vi "StreamEye_client_winX_v4.vi"() -> ()   [LabVIEW 2017]
uses:
  <vilib>/Analysis/NI_AALPro.lvlib
panel:
  in  "Start Scan":bool
  in  "Wavelength Step (nm)":dbl=100.0 min=0.0 max=100.0 step=0.01
  in  "Wavelength End (nm)":dbl=400.0 min=0.0 max=2000.0 step=0.01
  in  "Wavelength Start (nm)":dbl=400.0 min=0.0 max=2000.0 step=0.01
  in  "Fast continuous":bool caption="Focus mode"
  in  "standby stream":bool caption="Standby"
  out "time elapsed (s)":dbl caption="Time per scan (s)"
  out "Time Trace":dbl(graph)
  out "Intensity Sum":dbl
  in  "Stop measurement":bool
  out "XY Graph Spectrum":T1(graph)
  in  "Spectro Correct background":bool
  in  "Get Temp":bool
  in  "Misc Info/Variables":enum32{"Streaming", "OVA V"}(tab)
  out "reader endpoint":refnum<k21>
  out "error reader":errorcluster
  out "writer endpoint":refnum<k21>
  out "error writer":errorcluster
  out "MonoRef":refnum<k7>
  out "notifier out WinX Abort":refnum<notifier>
  out "notifier out WinX Start":refnum<notifier>
  in  "spectroObject reference":refnum<k7>
  in  "experiment reference_raw":refnum<k7>
  in  "file reference":refnum<k7>
  out "Wavelength Scale":dbl[](array[numeric])=[468.44882318557495, 468.4966768628263, 468.54452836446194, 468.59237769048184, 468.640224840886, 468.6880698156744, 468.73591261484705, 468.783753238404, 468.83159168634523, 468.8794279586707, 468.9272620553804, 468.9750939764744, 469.0229237219527, 469.07075129181516, 469.11857668606194, 469.16639990469304, 469.2142209477083, 469.2620398151079, 469.3098565068918, 469.3576710230599, 469.40548336361223, 469.45329352854884, 469.50110151786976, 469.5489073315749, 469.59671096966434, 469.644512432138, 469.69231171899594, 469.74010883023817, 469.78790376586466, 469.8356965258754, 469.8834871102704, 469.9312755190497, 469.97906175221317, 470.02684580976097, 470.074627691693, 470.12240739800933, 470.17018492870994, 470.2179602837948, 470.26573346326387, 470.31350446711724, 470.3612732953549, 470.4090399479768, 470.456804424983, 470.5045667263734, 470.5523268521481, 470.60008480230704, 470.6478405768503, 470.6955941757777, 470.7433455990895, 470.7910948467854, 470.83884191886574, 470.88658681533025, 470.93432953617906, 470.98207008141213, 471.02980845102945, 471.077544645031, 471.1252786634169, 471.17301050618704, 471.2207401733414, 471.26846766488006, 471.31619298080295, 471.36391612111015, 471.41163708580154, 471.45935587487725, 471.5070724883372, 471.55478692618146, 471.6024991884099, 471.6502092750227, 471.6979171860197, 471.745622921401, 471.79332648116656, 471.84102786531633, 471.8887270738504, 471.93642410676875, 471.98411896407134, 472.03181164575824, 472.07950215182933, 472.12719048228473, 472.1748766371244, 472.2225606163483, 472.27024241995645, 472.3179220479489, 472.36559950032563, 472.4132747770866, 472.4609478782318, 472.50861880376135, 472.5562875536751, 472.6039541279731, 472.6516185266554, 472.69928074972194, 472.7469407971728, 472.7945986690078, 472.8422543652272, 472.8899078858308, 472.93755923081864, 472.9852084001908, 473.0328553939472, 473.0805002120878, 473.1281428546128, 473.175783321522, 473.2234216128154, 473.27105772849313, 473.3186916685551, 473.36632343300136, 473.41395302183184, 473.46158043504664, 473.50920567264563, 473.55682873462894, 473.6044496209965, 473.65206833174835, 473.6996848668844, 473.7472992264048, 473.7949114103094, 473.84252141859827, 473.8901292512714, 473.9377349083288, 473.98533838977045, 474.0329396955964, 474.08053882580657, 474.12813578040107, 474.17573055937976, 474.22332316274276, 474.27091359049, 474.3185018426215, 474.36608791913727, 474.41367182003734, 474.46125354532165, 474.5088330949902, 474.55641046904304, 474.6039856674801, 474.6515586903015, 474.6991295375071, 474.74669820909696, 474.79426470507116, 474.84182902542955, 474.88939117017225, 474.93695113929914, 474.98450893281034, 475.0320645507058, 475.07961799298556, 475.1271692596495, 475.1747183506978, 475.2222652661303, 475.269810005947, 475.3173525701481, 475.3648929587334, 475.41243117170296, 475.4599672090568, 475.50750107079494, 475.5550327569173, 475.60256226742393, 475.6500896023148, 475.69761476158993, 475.7451377452494, 475.79265855329305, 475.840177185721, 475.88769364253324, 475.9352079237297, 475.9827200293104, 476.0302299592754, 476.0777377136247, 476.1252432923582, 476.172746695476, 476.22024792297805, 476.2677469748644, 476.31524385113494, 476.3627385517898, 476.4102310768289, 476.45772142625225, 476.5052096000599, 476.55269559825183, 476.600179420828, 476.6476610677884, 476.6951405391331, 476.742617834862, 476.79009295497525, 476.83756589947274, 476.8850366683545, 476.93250526162046, 476.97997167927076, 477.0274359213053, 477.0748979877241, 477.12235787852717, 477.1698155937145, 477.2172711332861, 477.2647244972419, 477.312175685582, 477.3596246983064, 477.40707153541507, 477.45451619690795, 477.50195868278513, 477.54939899304657, 477.59683712769225, 477.6442730867222, 477.69170687013644, 477.73913847793494, 477.7865679101177, 477.8339951666847, 477.88142024763596, 477.9288431529715, 477.97626388269134, 478.0236824367954, 478.07109881528373, 478.1185130181563, 478.1659250454132, 478.2133348970543, 478.2607425730797, 478.30814807348935, 478.35555139828324, 478.40295254746144, 478.4503515210239, 478.4977483189706, 478.54514294130155, 478.59253538801676, 478.6399256591163, 478.68731375460004, 478.73469967446806, 478.78208341872033, 478.82946498735686, 478.8768443803777, 478.9242215977828, 478.9715966395721, 479.0189695057457, 479.0663401963036, 479.1137087112457, 479.1610750505721, 479.20843921428275, 479.25580120237765, 479.30316101485687, 479.35051865172034, 479.397874112968, 479.4452273986, 479.49257850861625, 479.5399274430167, 479.5872742018015, 479.63461878497054, 479.68196119252383, 479.72930142446137, 479.7766394807832, 479.82397536148926, 479.8713090665796, 479.91864059605416, 479.9659699499131, 480.0132971281562, 480.0606221307836, 480.10794495779527, 480.1552656091912, 480.20258408497136, 480.24990038513585, 480.2972145096846, 480.34452645861757, 480.3918362319348, 480.4391438296363, 480.4864492517221, 480.5337524981921, 480.5810535690464, 480.62835246428494, 480.6756491839078, 480.72294372791487, 480.77023609630623, 480.81752628908185, 480.8648143062417, 480.9121001477859, 480.9593838137143, 481.00666530402697, 481.0539446187239, 481.1012217578051, 481.1484967212706, 481.1957695091203, 481.2430401213543, 481.29030855797254, 481.33757481897504, 481.3848389043618, 481.43210081413287, 481.4793605482882, 481.52661810682775, 481.5738734897516, 481.6211266970597, 481.66837772875203, 481.71562658482867, 481.76287326528956, 481.8101177701347, 481.85736009936414, 481.9046002529778, 481.95183823097574, 481.99907403335794, 482.0463076601244, 482.09353911127516, 482.1407683868102, 482.1879954867294, 482.2352204110329, 482.28244315972074, 482.32966373279277, 482.3768821302491, 482.4240983520897, 482.4713123983145, 482.5185242689236, 482.565733963917, 482.6129414832946, 482.6601468270565, 482.70734999520266, 482.7545509877331, 482.8017498046478, 482.84894644594675, 482.89614091162997, 482.94333320169744, 482.99052331614917, 483.0377112549852, 483.0848970182054, 483.13208060580996, 483.17926201779875, 483.22644125417185, 483.27361831492914, 483.32079320007074, 483.3679659095966, 483.4151364435067, 483.46230480180105, 483.5094709844797, 483.55663499154264, 483.6037968229898, 483.65095647882123, 483.6981139590369, 483.7452692636369, 483.79242239262106, 483.83957334598955, 483.8867221237423, 483.93386872587934, 483.9810131524006, 484.02815540330613, 484.07529547859593, 484.12243337827, 484.16956910232835, 484.2167026507709, 484.2638340235978, 484.31096322080884, 484.3580902424042, 484.4052150883839, 484.4523377587478, 484.49945825349596, 484.5465765726284, 484.5936927161451, 484.6408066840461, 484.6879184763313, 484.7350280930008, 484.78213553405453, 484.8292407994926, 484.87634388931485, 484.9234448035214, 484.9705435421122, 485.01764010508725, 485.06473449244663, 485.1118267041902, 485.1589167403181, 485.2060046008302, 485.2530902857266, 485.30017379500725, 485.34725512867215, 485.39433428672135, 485.4414112691548, 485.4884860759725, 485.53555870717446, 485.5826291627607, 485.62969744273124, 485.67676354708595, 485.723827475825, 485.7708892289483, 485.81794880645583, 485.86500620834767, 485.91206143462375, 485.9591144852841, 486.0061653603287, 486.0532140597576, 486.10026058357073, 486.1473049317681, 486.1943471043498, 486.2413871013157, 486.28842492266585, 486.3354605684003, 486.38249403851904, 486.429525333022, 486.4765544519093, 486.52358139518077, 486.57060616283655, 486.6176287548766, 486.6646491713009, 486.7116674121094, 486.75868347730227, 486.8056973668794, 486.8527090808407, 486.89971861918633, 486.9467259819162, 486.99373116903035, 487.0407341805287, 487.0877350164114, 487.13473367667837, 487.18173016132954, 487.228724470365, 487.2757166037847, 487.3227065615887, 487.369694343777, 487.4166799503495, 487.4636633813063, 487.51064463664727, 487.5576237163726, 487.6046006204822, 487.651575348976, 487.6985479018541, 487.7455182791164, 487.7924864807631, 487.839452506794, 487.8864163572091, 487.93337803200853, 487.9803375311922, 488.02729485476016, 488.07425000271235, 488.1212029750488, 488.16815377176954, 488.21510239287454, 488.2620488383638, 488.3089931082373, 488.3559352024951, 488.40287512113713, 488.44981286416345, 488.496748431574, 488.5436818233689, 488.590613039548, 488.63754208011136, 488.684468945059, 488.7313936343909, 488.778316148107, 488.8252364862074, 488.8721546486921, 488.919070635561, 488.9659844468142, 489.0128960824517, 489.05980554247344, 489.10671282687946, 489.15361793566973, 489.20052086884425, 489.247421626403, 489.2943202083461, 489.3412166146734, 489.388110845385, 489.4350029004808, 489.48189277996096, 489.5287804838253, 489.57566601207395, 489.62254936470686, 489.669430541724, 489.7163095431254, 489.76318636891114, 489.8100610190811, 489.8569334936353, 489.9038037925738, 489.9506719158965, 489.99753786360355, 490.04440163569484, 490.0912632321704, 490.13812265303017, 490.1849798982742, 490.23183496790256, 490.27868786191516, 490.325538580312, 490.3723871230931, 490.4192334902585, 490.46607768180814, 490.51291969774206, 490.55975953806023, 490.60659720276266, 490.65343269184933, 490.7002660053203, 490.74709714317555, 490.79392610541504, 490.8407528920388, 490.88757750304677, 490.93439993843907, 490.9812201982156, 491.02803828237643, 491.0748541909215, 491.12166792385085, 491.1684794811644, 491.2152888628623, 491.2620960689444, 491.3089010994108, 491.35570395426146, 491.4025046334964, 491.4493031371155, 491.49609946511896, 491.5428936175067, 491.58968559427865, 491.6364753954349, 491.6832630209754, 491.73004847090016, 491.77683174520917, 491.8236128439025, 491.87039176698, 491.9171685144418, 491.9639430862879, 492.01071548251826, 492.05748570313284, 492.1042537481317, 492.15101961751486, 492.19778331128225, 492.2445448294339, 492.29130417196984, 492.33806133889004, 492.38481633019444, 492.4315691458832, 492.47831978595616, 492.52506825041337, 492.5718145392549, 492.61855865248066, 492.6653005900907, 492.712040352085, 492.75877793846354, 492.8055133492264, 492.85224658437346, 492.8989776439048, 492.9457065278204, 492.9924332361203, 493.03915776880444, 493.08588012587285, 493.1326003073255, 493.1793183131624, 493.22603414338363, 493.2727477979891, 493.31945927697876, 493.36616858035273, 493.41287570811096, 493.4595806602535, 493.5062834367803, 493.5529840376913, 493.5996824629866, 493.64637871266615, 493.69307278673, 493.7397646851781, 493.78645440801046, 493.83314195522706, 493.879827326828, 493.9265105228131, 493.9731915431825, 494.0198703879362, 494.0665470570741, 494.11322155059634, 494.15989386850276, 494.2065640107935, 494.2532319774685, 494.2998977685278, 494.3465613839713, 494.3932228237991, 494.43988208801113, 494.48653917660744, 494.533194089588, 494.5798468269528, 494.6264973887019, 494.6731457748353, 494.7197919853529, 494.7664360202548, 494.81307787954097, 494.8597175632114, 494.90635507126603, 494.95299040370503, 494.9996235605282, 495.04625454173566, 495.0928833473274, 495.1395099773034, 495.1861344316637, 495.2327567104082, 495.279376813537, 495.32599474105007, 495.3726104929474, 495.41922406922896, 495.4658354698948, 495.5124446949449, 495.55905174437925, 495.6056566181979, 495.6522593164008, 495.69885983898797, 495.74545818595936, 495.79205435731507, 495.838648353055, 495.8852401731792, 495.93182981768774, 495.97841728658045, 496.02500257985747, 496.07158569751874, 496.11816663956427, 496.1647454059941, 496.2113219968081, 496.25789641200646, 496.30446865158905, 496.3510387155559, 496.397606603907, 496.4441723166424, 496.49073585376203, 496.53729721526594, 496.5838564011541, 496.63041341142656, 496.6769682460832, 496.7235209051242, 496.7700713885494, 496.8166196963589, 496.86316582855267, 496.90970978513064, 496.95625156609293, 497.00279117143947, 497.04932860117026, 497.09586385528536, 497.1423969337847, 497.18892783666826, 497.2354565639361, 497.2819831155883, 497.32850749162463, 497.3750296920453, 497.4215497168502, 497.4680675660394, 497.5145832396128, 497.56109673757055, 497.6076080599125, 497.6541172066387, 497.7006241777492, 497.74712897324395, 497.793631593123, 497.84013203738624, 497.8866303060338, 497.9331263990656, 497.97962031648166, 498.02611205828197, 498.0726016244666, 498.11908901503546, 498.1655742299886, 498.212057269326, 498.25853813304764, 498.3050168211536, 498.35149333364376, 498.3979676705182, 498.4444398317769, 498.4909098174199, 498.5373776274471, 498.5838432618586, 498.6303067206544, 498.6767680038344, 498.72322711139867, 498.76968404334724, 498.81613879968006, 498.86259138039713, 498.9090417854985, 498.9554900149841, 499.001936068854, 499.0483799471081, 499.0948216497465, 499.1412611767692, 499.1876985281761, 499.2341337039673, 499.28056670414276, 499.32699752870246, 499.3734261776465, 499.4198526509747, 499.4662769486872, 499.512699070784, 499.559119017265, 499.60553678813034, 499.65195238337986, 499.6983658030137, 499.7447770470318, 499.79118611543413, 499.8375930082208, 499.8839977253916, 499.9304002669468, 499.9768006328862, 500.0231988232099, 500.0695948379178, 500.11598867701, 500.16238034048644, 500.2087698283472, 500.2551571405922, 500.3015422772214, 500.34792523823495, 500.39430602363274, 500.4406846334148, 500.48706106758107, 500.53343532613167, 500.57980740906646, 500.62617731638557, 500.6725450480889, 500.7189106041766, 500.76527398464845, 500.8116351895046, 500.85799421874503, 500.9043510723697, 500.95070575037863, 500.99705825277186, 501.0434085795493, 501.08975673071103, 501.136102706257, 501.1824465061873, 501.2287881305018, 501.2751275792006, 501.32146485228367, 501.367799949751, 501.41413287160253, 501.4604636178384, 501.5067921884585, 501.5531185834629, 501.5994428028515, 501.6457648466244, 501.6920847147816, 501.73840240732295, 501.78471792424864, 501.8310312655586, 501.8773424312528, 501.9236514213313, 501.969958235794, 502.01626287464103, 502.0625653378723, 502.10886562548785, 502.1551637374876, 502.2014596738716, 502.24775343463995, 502.2940450197925, 502.3403344293294, 502.3866216632505, 502.43290672155587, 502.4791896042455, 502.5254703113194, 502.5717488427776, 502.61802519862, 502.6642993788467, 502.71057138345765, 502.75684121245285, 502.80310886583237, 502.8493743435961, 502.8956376457441, 502.9418987722764, 502.98815772319296, 503.03441449849373, 503.0806690981788, 503.12692152224815, 503.17317177070174, 503.2194198435396, 503.2656657407617, 503.3119094623681, 503.35815100835873, 503.40439037873364, 503.4506275734928, 503.49686259263626, 503.5430954361639, 503.5893261040759, 503.6355545963721, 503.68178091305265, 503.7280050541174, 503.7742270195664, 503.8204468093997, 503.86666442361724, 503.91287986221903, 503.95909312520513, 504.0053042125754, 504.05151312433003, 504.0977198604689, 504.14392442099205, 504.1901268058994, 504.2363270151911, 504.282525048867, 504.3287209069272, 504.3749145893716, 504.42110609620033, 504.4672954274133, 504.51348258301056, 504.55966756299205, 504.6058503673578, 504.65203099610784, 504.6982094492421, 504.74438572676064, 504.79055982866345, 504.83673175495056, 504.8829015056219, 504.9290690806775, 504.97523448011736, 505.0213977039415, 505.0675587521499, 505.11371762474255, 505.1598743217195, 505.2060288430807, 505.2521811888261, 505.29833135895586, 505.3444793534698, 505.39062517236806, 505.43676881565057, 505.4829102833173, 505.5290495753684, 505.57518669180365, 505.6213216326232, 505.66745439782704, 505.7135849874151, 505.7597134013875, 505.80583963974414, 505.85196370248497, 505.8980855896101, 505.94420530111955, 505.9903228370132, 506.03643819729115, 506.08255138195335, 506.1286623909998, 506.1747712244305, 506.2208778822455, 506.26698236444474, 506.31308467102826, 506.35918480199604, 506.40528275734806, 506.4513785370844, 506.4974721412049, 506.54356356970976, 506.58965282259885, 506.63573989987225, 506.6818248015298, 506.7279075275717, 506.77398807799784, 506.82006645280825, 506.8661426520029, 506.9122166755819, 506.95828852354504, 507.0043581958925, 507.05042569262423, 507.09649101374026, 507.1425541592405, 507.188615129125, 507.2346739233938, 507.28073054204685, 507.32678498508415, 507.37283725250575, 507.4188873443116, 507.4649352605017, 507.51098100107606, 507.55702456603467, 507.6030659553776, 507.6491051691047, 507.6951422072161, 507.74117706971185, 507.7872097565918, 507.83324026785596, 507.87926860350444, 507.9252947635372, 507.9713187479542, 508.01734055675547, 508.06336018994097, 508.10937764751077, 508.1553929294648, 508.20140603580313, 508.24741696652575, 508.29342572163256, 508.3394323011237, 508.38543670499905, 508.4314389332587, 508.4774389859026, 508.52343686293074, 508.5694325643432, 508.61542609013986, 508.6614174403208, 508.70740661488605, 508.7533936138355, 508.79937843716925, 508.84536108488726, 508.8913415569896, 508.9373198534761, 508.9832959743469, 509.029269919602, 509.0752416892413, 509.12121128326487, 509.1671787016727, 509.21314394446483, 509.2591070116412, 509.30506790320186, 509.35102661914675, 509.39698315947595, 509.44293752418935, 509.48888971328705, 509.534839726769, 509.5807875646353, 509.62673322688573, 509.6726767135205, 509.7186180245395, 509.7645571599428, 509.8104941197303, 509.85642890390216, 509.9023615124582, 509.9482919453985, 509.9942202027231, 510.040146284432, 510.0860701905251, 510.1319919210025, 510.17791147586416, 510.22382885511007, 510.26974405874023, 510.3156570867547, 510.3615679391534, 510.4074766159364, 510.4533831171036, 510.4992874426551, 510.5451895925909, 510.59108956691085, 510.63698736561514, 510.6828829887037, 510.72877643617653, 510.7746677080336, 510.82055680427493, 510.86644372490053, 510.9123284699104, 510.95821103930456, 511.00409143308286, 511.04996965124553, 511.09584569379246, 511.14171956072363, 511.1875912520391, 511.2334607677388, 511.2793281078228, 511.325193272291, 511.3710562611435, 511.4169170743803, 511.4627757120013, 511.5086321740066, 511.55448646039616, 511.60033857116997, 511.6461885063281, 511.6920362658704, 511.737881849797, 511.7837252581079, 511.8295664908031, 511.87540554788245, 511.92124242934614, 511.9670771351941, 512.0129096654263, 512.0587400200427, 512.1045681990435, 512.1503942024284, 512.1962180301977, 512.2420396823511, 512.287859158889, 512.3336764598109, 512.3794915851173, 512.4253045348079, 512.4711153088826, 512.5169239073417, 512.5627303301851, 512.6085345774127, 512.6543366490246, 512.7001365450208, 512.7459342654012, 512.7917298101659, 512.8375231793148, 512.883314372848, 512.9291033907655, 512.9748902330672, 513.0206748997532, 513.0664573908234, 513.1122377062779, 513.1580158461167, 513.2037918103398, 513.249565598947, 513.2953372119387, 513.3411066493145, 513.3868739110745, 513.432638997219, 513.4784019077475, 513.5241626426605, 513.5699212019576, 513.615677585639, 513.6614317937047, 513.7071838261546, 513.7529336829889, 513.7986813642074, 513.84442686981, 513.890170199797, 513.9359113541683, 513.9816503329239, 514.0273871360637, 514.0731217635877, 514.118854215496, 514.1645844917886, 514.2103125924655, 514.2560385175266, 514.3017622669719, 514.3474838408015, 514.3932032390154, 514.4389204616136, 514.484635508596, 514.5303483799627, 514.5760590757136, 514.6217675958488, 514.6674739403684, 514.7131781092721, 514.75888010256, 514.8045799202323, 514.8502775622889, 514.8959730287297, 514.9416663195548, 514.987357434764, 515.0330463743577, 515.0787331383355, 515.1244177266976, 515.170100139444, 515.2157803765747, 515.2614584380896, 515.3071343239887, 515.3528080342721, 515.3984795689398, 515.4441489279917, 515.489816111428, 515.5354811192485, 515.5811439514532, 515.6268046080422, 515.6724630890155, 515.718119394373, 515.7637735241149, 515.8094254782409, 515.8550752567513, 515.9007228596458, 515.9463682869247, 515.9920115385878, 516.0376526146352, 516.0832915150669, 516.1289282398827, 516.1745627890829, 516.2201951626673, 516.2658253606361, 516.311453382989, 516.3570792297262, 516.4027029008477, 516.4483243963535, 516.4939437162435, 516.5395608605178, 516.5851758291764, 516.6307886222193, 516.6763992396462, 516.7220076814576, 516.7676139476531, 516.8132180382331, 516.8588199531972, 516.9044196925456, 516.9500172562782, 516.9956126443952, 517.0412058568963, 517.0867968937818, 517.1323857550515, 517.1779724407054, 517.2235569507437, 517.2691392851661, 517.3147194439729, 517.3602974271639, 517.4058732347393, 517.4514468666988, 517.4970183230427, 517.5425876037707, 517.588154708883, 517.6337196383797, 517.6792823922606, 517.7248429705256, 517.7704013731751, 517.8159576002088, 517.8615116516266, 517.9070635274288, 517.9526132276153, 517.9981607521861, 518.043706101141, 518.0892492744803, 518.1347902722036, 518.1803290943116, 518.2258657408036, 518.2714002116799, 518.3169325069404, 518.3624626265853, 518.4079905706143, 518.4535163390277, 518.4990399318252, 518.5445613490073, 518.5900805905733, 518.6355976565237, 518.6811125468583, 518.7266252615774, 518.7721358006805, 518.817644164168, 518.8631503520397, 518.9086543642958, 518.9541562009359, 518.9996558619605, 519.0451533473693, 519.0906486571622, 519.1361417913396, 519.1816327499012, 519.2271215328469, 519.272608140177, 519.3180925718915, 519.3635748279901, 519.409054908473, 519.45453281334, 519.5000085425916, 519.5454820962271, 519.5909534742472, 519.6364226766513, 519.6818897034399, 519.7273545546126, 519.7728172301695, 519.8182777301107, 519.8637360544363, 519.9091922031461, 519.9546461762401, 520.0000979737184, 520.045547595581, 520.0909950418279, 520.136440312459, 520.1818834074743, 520.2273243268739, 520.2727630706579, 520.3181996388261, 520.3636340313784, 520.4090662483151, 520.4544962896362, 520.4999241553413, 520.5453498454308, 520.5907733599045, 520.6361946987626, 520.6816138620048, 520.7270308496313, 520.772445661642, 520.8178582980372, 520.8632687588165, 520.90867704398, 520.9540831535279, 520.99948708746, 521.0448888457764, 521.090288428477, 521.1356858355618, 521.1810810670311, 521.2264741228845, 521.2718650031222, 521.3172537077442, 521.3626402367503, 521.4080245901409, 521.4534067679156, 521.4987867700746, 521.5441645966179, 521.5895402475454, 521.6349137228573, 521.6802850225532, 521.7256541466336, 521.7710210950983, 521.8163858679471, 521.8617484651802, 521.9071088867976, 521.9524671327993, 521.9978232031851, 522.0431770979553, 522.0885288171097, 522.1338783606484, 522.1792257285714, 522.2245709208786, 522.2699139375701, 522.3152547786458, 522.3605934441059, 522.4059299339501, 522.4512642481786, 522.4965963867915, 522.5419263497886, 522.5872541371699, 522.6325797489355, 522.6779031850854, 522.7232244456195, 522.7685435305378, 522.8138604398405, 522.8591751735274, 522.9044877315987, 522.949798114054, 522.9951063208938, 523.0404123521178, 523.0857162077259, 523.1310178877185, 523.1763173920953, 523.2216147208562, 523.2669098740015, 523.3122028515311, 523.3574936534449, 523.402782279743, 523.4480687304252, 523.4933530054919, 523.5386351049428, 523.5839150287779, 523.6291927769973, 523.674468349601, 523.719741746589, 523.7650129679611, 523.8102820137175, 523.8555488838583, 523.9008135783832, 523.9460760972925, 523.991336440586, 524.0365946082637, 524.0818506003258, 524.1271044167721, 524.1723560576027, 524.2176055228174, 524.2628528124166, 524.3080979263999, 524.3533408647675, 524.3985816275193, 524.4438202146556, 524.489056626176, 524.5342908620805, 524.5795229223695, 524.6247528070428, 524.6699805161002, 524.7152060495418, 524.7604294073678, 524.8056505895781, 524.8508695961726, 524.8960864271514, 524.9413010825144, 524.9865135622617, 525.0317238663933, 525.0769319949092, 525.1221379478092, 525.1673417250936, 525.2125433267622, 525.2577427528151, 525.3029400032523, 525.3481350780736, 525.3933279772793, 525.4385187008693, 525.4837072488434, 525.5288936212019, 525.5740778179447, 525.6192598390717, 525.6644396845829, 525.7096173544784, 525.7547928487583, 525.7999661674223, 525.8451373104706, 525.8903062779032, 525.9354730697199, 525.9806376859211, 526.0258001265064, 526.0709603914761, 526.1161184808299, 526.1612743945682, 526.2064281326906, 526.2515796951972, 526.2967290820881, 526.3418762933634, 526.3870213290229, 526.4321641890666, 526.4773048734945, 526.5224433823068, 526.5675797155034, 526.6127138730842, 526.6578458550492, 526.7029756613986, 526.7481032921321, 526.7932287472499, 526.838352026752, 526.8834731306383, 526.9285920589091, 526.9737088115639, 527.0188233886031, 527.0639357900264, 527.1090460158342, 527.1541540660262, 527.1992599406024, 527.2443636395628, 527.2894651629076, 527.3345645106366, 527.3796616827499, 527.4247566792474, 527.4698495001293, 527.5149401453954, 527.5600286150457, 527.6051149090802, 527.6501990274991, 527.6952809703022, 527.7403607374896, 527.7854383290612, 527.830513745017, 527.8755869853574, 527.9206580500817, 527.9657269391904, 528.0107936526833, 528.0558581905606, 528.1009205528221, 528.1459807394677, 528.1910387504978, 528.2360945859122, 528.2811482457107, 528.3261997298935, 528.3712490384605, 528.4162961714119, 528.4613411287474, 528.5063839104673, 528.5514245165714, 528.5964629470599, 528.6414992019324, 528.6865332811893, 528.7315651848305, 528.7765949128559, 528.8216224652657, 528.8666478420597, 528.9116710432379, 528.9566920688003, 529.0017109187472, 529.0467275930782, 529.0917420917934, 529.136754414893, 529.1817645623769, 529.2267725342449, 529.2717783304972, 529.3167819511337, 529.3617833961547, 529.4067826655598, 529.4517797593492, 529.4967746775228, 529.5417674200809, 529.586757987023, 529.6317463783495, 529.6767325940601, 529.7217166341551, 529.7666984986344, 529.8116781874978, 529.8566557007456, 529.9016310383776, 529.946604200394, 529.9915751867945, 530.0365439975793, 530.0815106327484, 530.1264750923018, 530.1714373762394, 530.2163974845612, 530.2613554172673, 530.3063111743578, 530.3512647558324, 530.3962161616913, 530.4411653919345, 530.4861124465621, 530.5310573255738, 530.5760000289697]
  in  "FrameVariant":variant
  out "experiment reference":refnum<k7>
  out "frame array":i32[][](array[numeric])
  out "time start (ms)":i32
  in  "Set Temperature (°C)":i8 min=-125 max=25 step=1
  in  "Start Continuous":bool
  in  "Start Background":bool
  in  "Start Single Spectrum":bool
  in  "Start Stream":bool
  out "busy":bool
  out "Hosts Synchronized":bool
  in  "Synchronize Hosts":bool
  in  "Init Spectro":bool
  in  "Exit":bool
  out "OMA V temp":dbl(slide) caption="Sensor Temperature" scale=-125.0..25.0
  in  "OMA V exposure time":dbl=0.001 caption="Integration time (s)" min=0.001 max=3000.0 step=0.001
  in  "OMA V gain":u32(ring) caption="Gain" items=["low"=2, "high"=3]
  in  "Grating Number":i16(ring) items=["600g/mm, blz=1.6um"=1, "300g/mm, blz=1.0um"=2, "150g/mm, blz=3.0um"=3]
  in  "Output Port":bool
  in  "Wavelength (nm)":dbl=400.0 min=-100.0 max=2000.0 step=0.01
  out "Spectro ON":bool
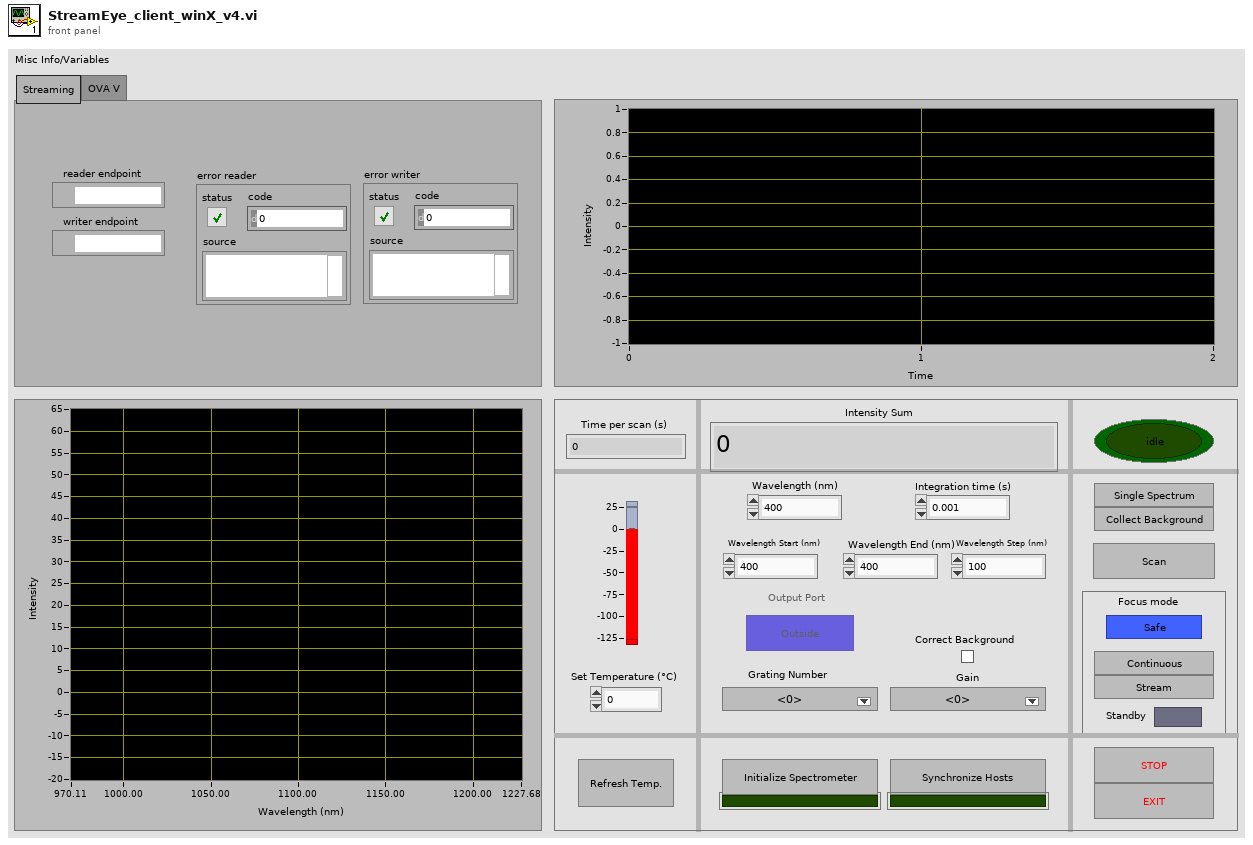
[diagram p1: front panel]
types:
  T1 = cluster{"Calibrated Array":dbl[], "Array F32":sgl[]}
  T2 = enum8{"Enabled", "Disabled", "Disabled and Grayed Out"}
  T3 = cluster{"Wavelength Scale":dbl[], "frame array":i32[]}
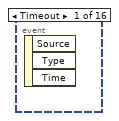
[diagram p2: hidden frame]
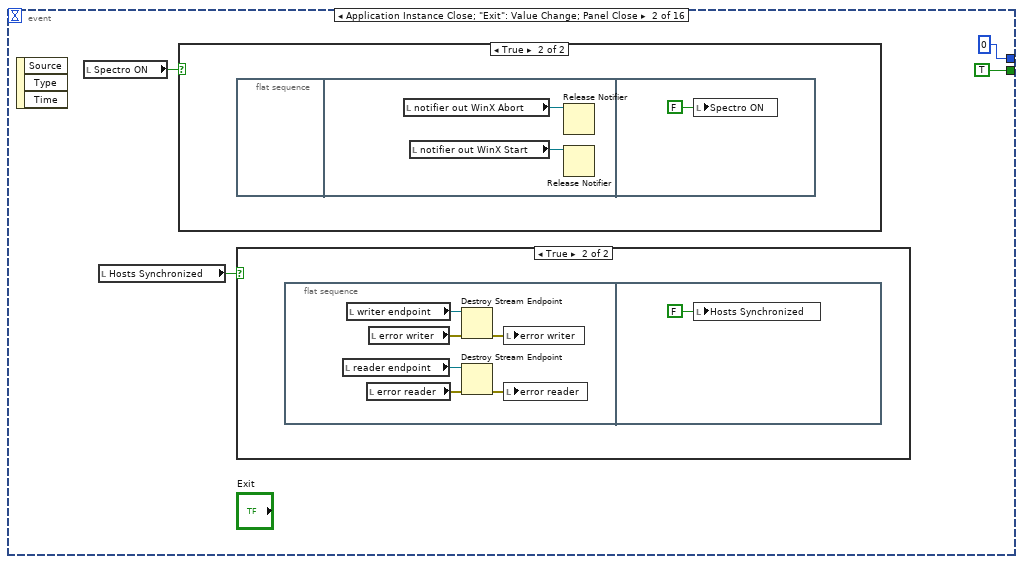
[diagram p3: hidden frame]
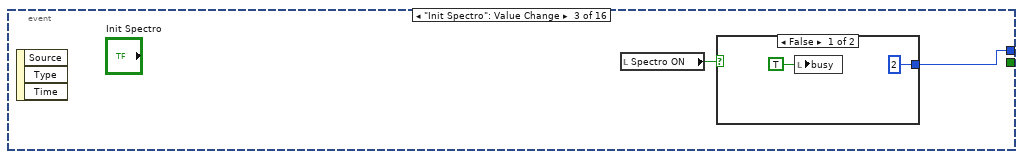
[diagram p6: hidden frame]
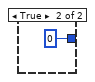
[diagram p7: hidden frame]
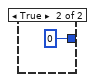
[diagram p8: hidden frame]
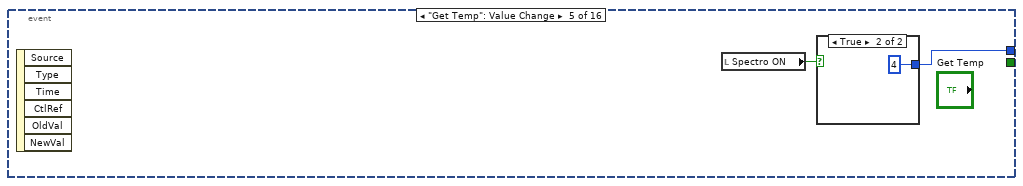
[diagram p9: hidden frame]
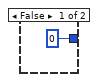
[diagram p10: hidden frame]
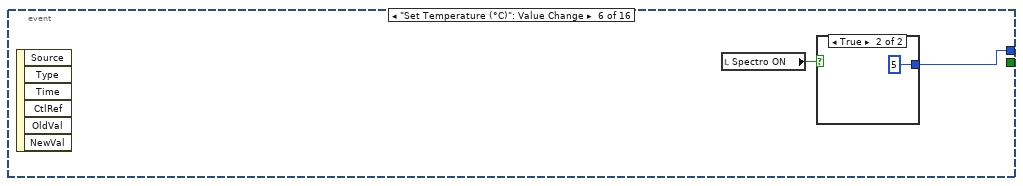
[diagram p11: hidden frame]
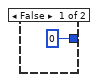
[diagram p12: hidden frame]
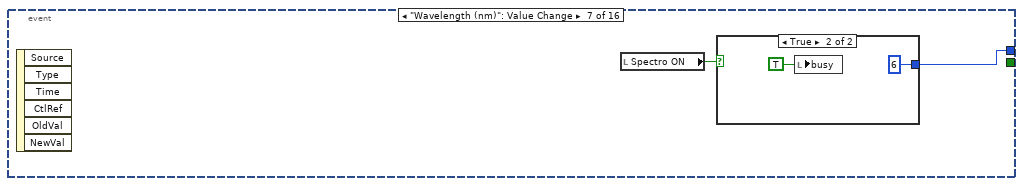
[diagram p13: hidden frame]
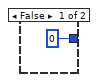
[diagram p14: hidden frame]
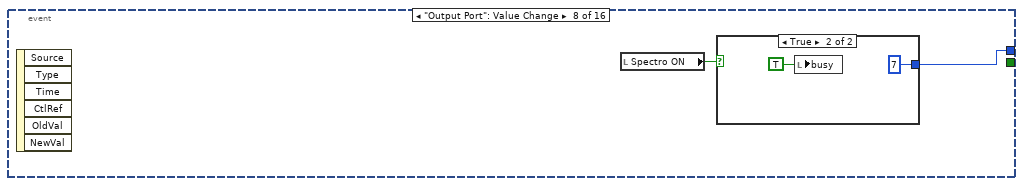
[diagram p15: hidden frame]
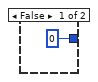
[diagram p16: hidden frame]
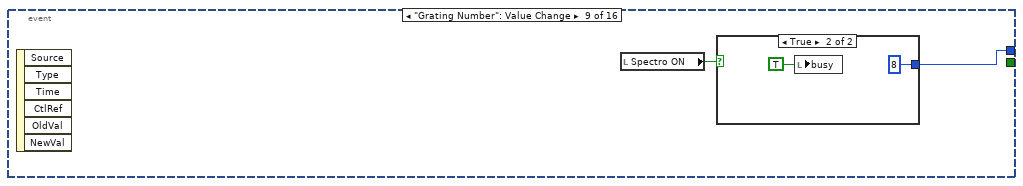
[diagram p17: hidden frame]
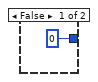
[diagram p18: hidden frame]
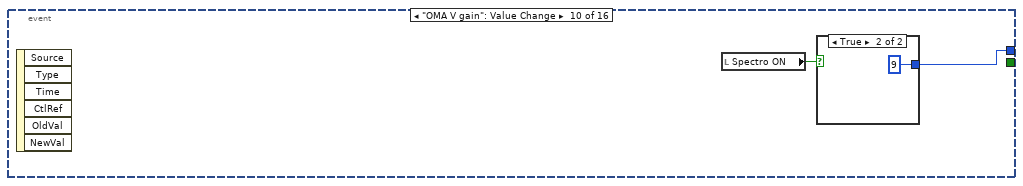
[diagram p19: hidden frame]
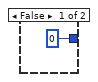
[diagram p20: hidden frame]
diagram:
  w8 = u32 2 items=["", "low", "high"] ("OMA V gain")
  w7 = FALSE ("Hosts Synchronized")
  n1 = while {
    stop <- w14 stop-if-true
    n2 = flat-sequence {
      tunnel: [w16] -> w14
      tunnel: [w15] -> w13
      tunnel: w13 -> [w108]
      frame #0 {
        # "Even catcher"
        n3 = event shown="[3] \"Synchronize Hosts\": Value Change" {
          selector: _ -> [_ _ _ _ _ _ _ _ _ _ _ _ _ _ _ _]
          dyn-events: _ -> [_ _ _ _ _ _ _ _ _ _ _ _ _ _ _ _]
          timeout: 1000 -> [_ _ _ _ _ _ _ _ _ _ _ _ _ _ _ _]
          tunnel: [_ TRUE _ _ _ _ _ _ _ _ _ _ _ _ _ _] -> w16
          tunnel: [_ 0 w33 w37 w42 w46 w50 w55 w61 w66 w69 w74 w79 w90 0 w103] -> w15
          event Timeout {
            n4 = event-data() -> ()  [unwired: 1 in, 3 out]
          }
          event Application Instance Close; "Exit": Value Change; Panel Close {
            n5 = event-data() -> ()  [unwired: 1 in, 3 out]
            n6 = local read "Spectro ON"() -> (w18:bool)
            n7 = local read "Hosts Synchronized"() -> (w19:bool)
            n8 = case shown="True" w18 {
              frame False {
              }
              frame True {
                n9 = flat-sequence {
                  frame #0 {
                  }
                  frame #1 {
                    n10 = local read "notifier out WinX Abort"() -> (w29:refnum<notifier>)
                    n11 = local read "notifier out WinX Start"() -> (w30:refnum<notifier>)
                    n12 = Release Notifier(notifier=w29) -> ()  [unwired: 2 in, 3 out]
                    n13 = Release Notifier(notifier=w30) -> ()  [unwired: 2 in, 3 out]
                  }
                  frame #2 {
                    n14 = local write "Spectro ON"(FALSE ("Spectro ON")) -> ()
                  }
                }
              }
            }
            n15 = case shown="True" w19 {
              frame False {
              }
              frame True {
                n16 = flat-sequence {
                  frame #0 {
                    n17 = local read "reader endpoint"() -> (w22:refnum<k21>)
                    n18 = local read "writer endpoint"() -> (w23:refnum<k21>)
                    n19 = local read "error reader"() -> (w27:errorcluster)
                    n20 = local read "error writer"() -> (w24:errorcluster)
                    n21 = Destroy Stream Endpoint(8:w24, 11:w23) -> (0:w25:errorcluster)
                    n22 = Destroy Stream Endpoint(8:w27, 11:w22) -> (0:w26:errorcluster)
                    n23 = local write "error writer"(w25) -> ()
                    n24 = local write "error reader"(w26) -> ()
                  }
                  frame #1 {
                    n25 = local write "Hosts Synchronized"(FALSE ("Hosts Synchronized")) -> ()
                  }
                }
              }
            }
          }
          event "Init Spectro": Value Change {
            n26 = event-data() -> ()  [unwired: 1 in, 3 out]
            n27 = local read "Spectro ON"() -> (w32:bool)
            n28 = case shown="False" w32 {
              tunnel: [2 0] -> w33
              frame False {
                n29 = local write "busy"(TRUE ("busy")) -> ()
              }
              frame True {
              }
            }
          }
          event "Synchronize Hosts": Value Change {
            n30 = event-data() -> ()  [unwired: 1 in, 3 out]
            n31 = local read "Hosts Synchronized"() -> (w38:bool)
            n32 = case shown="False" w38 {
              tunnel: [3 0] -> w37
              frame False {
                n33 = local write "busy"(TRUE ("busy")) -> ()
              }
              frame True {
              }
            }
          }
          event "Get Temp": Value Change {
            n34 = event-data() -> ()  [unwired: 1 in, 6 out]
            n35 = local read "Spectro ON"() -> (w43:bool)
            n36 = case shown="True" w43 {
              tunnel: [0 4] -> w42
              frame False {
              }
              frame True {
              }
            }
          }
          event "Set Temperature (°C)": Value Change {
            n37 = event-data() -> ()  [unwired: 1 in, 6 out]
            n38 = local read "Spectro ON"() -> (w47:bool)
            n39 = case shown="True" w47 {
              tunnel: [0 5] -> w46
              frame False {
              }
              frame True {
              }
            }
          }
          event "Wavelength (nm)": Value Change {
            n40 = event-data() -> ()  [unwired: 1 in, 6 out]
            n41 = local read "Spectro ON"() -> (w51:bool)
            n42 = case shown="True" w51 {
              tunnel: [0 6] -> w50
              frame False {
              }
              frame True {
                n43 = local write "busy"(TRUE ("busy")) -> ()
              }
            }
          }
          event "Output Port": Value Change {
            n44 = event-data() -> ()  [unwired: 1 in, 6 out]
            n45 = local read "Spectro ON"() -> (w56:bool)
            n46 = case shown="True" w56 {
              tunnel: [0 7] -> w55
              frame False {
              }
              frame True {
                n47 = local write "busy"(TRUE ("busy")) -> ()
              }
            }
          }
          event "Grating Number": Value Change {
            n48 = event-data() -> ()  [unwired: 1 in, 6 out]
            n49 = local read "Spectro ON"() -> (w60:bool)
            n50 = case shown="True" w60 {
              tunnel: [0 8] -> w61
              frame False {
              }
              frame True {
                n51 = local write "busy"(TRUE ("busy")) -> ()
              }
            }
          }
          event "OMA V gain": Value Change {
            n52 = event-data() -> ()  [unwired: 1 in, 6 out]
            n53 = local read "Spectro ON"() -> (w65:bool)
            n54 = case shown="True" w65 {
              tunnel: [0 9] -> w66
              frame False {
              }
              frame True {
              }
            }
          }
          event "Start Single Spectrum": Value Change {
            n55 = event-data() -> ()  [unwired: 1 in, 6 out]
            n56 = local read "Spectro ON"() -> (w70:bool)
            n57 = case shown="True" w70 {
              tunnel: [0 10] -> w69
              frame False {
              }
              frame True {
                n58 = local write "busy"(TRUE ("busy")) -> ()
              }
            }
          }
          event "Start Background": Value Change {
            n59 = event-data() -> ()  [unwired: 1 in, 6 out]
            n60 = local read "Spectro ON"() -> (w75:bool)
            n61 = case shown="True" w75 {
              tunnel: [0 11] -> w74
              frame False {
              }
              frame True {
                n62 = local write "busy"(TRUE) -> ()
              }
            }
          }
          event "Start Continuous": Value Change {
            n63 = event-data() -> ()  [unwired: 1 in, 6 out]
            n64 = local read "Spectro ON"() -> (w80:bool)
            n65 = case shown="True" w80 {
              tunnel: [0 w84] -> w79
              frame False {
              }
              frame True {
                n66 = local write "busy"(TRUE) -> ()
                n67 = local read "Fast continuous"() -> (w82:bool)
                n68 = Select(t=14, s=w82, f=12) -> (s? t:f=w84:i32)
              }
            }
          }
          event "Start Stream": Value Change {
            n69 = event-data() -> ()  [unwired: 1 in, 6 out]
            n70 = local read "Hosts Synchronized"() -> (w89:bool)
            n71 = local read "Spectro ON"() -> (w88:bool)
            n72 = And(x=w88, y=w89) -> (x .and. y?=w87:bool)
            n73 = case shown="True" w87 {
              tunnel: [0 w92] -> w90
              frame False {
              }
              frame True {
                n74 = local write "busy"(TRUE) -> ()
                n75 = local read "Fast continuous"() -> (w94:bool)
                n76 = Select(t=15, s=w94, f=13) -> (s? t:f=w92:i32)
              }
            }
          }
          event "Spectro Correct background": Value Change {
            n77 = event-data() -> ()  [unwired: 1 in, 6 out]
            n78 = local read "Spectro ON"() -> (w98:bool)
            n79 = case shown="True" w98 {
              frame False {
              }
              frame True {
                w102 = 828 items=["EXP_ETACTUAL"=1, "EXP_SEQUENTS"=2, "EXP_ERROR"=3, "EXP_GETCAPS"=4, "EXP_GETPLSR"=5, "EXP_DETECTOR_BIT"=16, "EXP_RUNNING_APP"=23, "EXP_VIDEO_TYPE"=24, "EXP_CUSTOM_VIDEO_X"=25, "EXP_CUSTOM_VIDEO_Y"=26, "EXP_CUSTOM_VIDEO_FSTWIDTH"=27, "EXP_CUSTOM_VIDEO_LSTWIDTH"=28, "EXP_VIDEO_XDIM"=29, "EXP_VIDEO_YDIM"=30, "EXP_VIDEO_MAX_ZOOM"=31, "EXP_VIDEO_HORZ_PAN"=32, "EXP_VIDEO_VERT_PAN"=33, "EXP_WORD_MULTIPLIER"=34, "EXP_TARGET_ID"=35, "EXP_ADAPTER_ID"=36, "EXP_NUMADAPTORS"=37, "EXP_FORCE_PP_INIT"=38, "EXP_NOP_ADC"=39, "EXP_ACTUAL_TEMP"=40, "EXP_FORCE_AUTOSTOP"=41, "EXP_DEFAULT_VTCLK"=42, "EXP_MIN_VTCLK"=43, "EXP_MAX_VTCLK"=44, "EXP_DEFAULT_HTCLK"=45, "EXP_MIN_HTCLK"=46, "EXP_MAX_HTCLK"=47, "EXP_TIMING_STYLE"=48, "EXP_HEADSELECT"=49, "EXP_HORZPHASE"=50, "EXP_VERTPHASE"=51, "EXP_SPECIAL_SPEED"=52, "EXP_PRE_STRIPS"=53, "EXP_POST_STRIPS"=54, "EXP_PRE_LINES"=55, "EXP_POST_LINES"=56, "EXP_ACTIVE_LINES"=57, "EXP_ACTIVE_STRIPS"=58, "EXP_XFER_EXTRA"=59, "EXP_MIN_BLOCK"=60, "EXP_NUM_MIN_BLOCK"=61, "EXP_LOGIC_OUTPUT"=66, "EXP_VIDEO_BLANK"=67, "EXP_ZOOM_MODE_VIDEO"=68, "EXP_LEVEL_SYNC"=69, "EXP_DISABLE_LASER"=70, "EXP_ACQBACK_SHUTTER"=71, "EXP_ACQFLAT_SHUTTER"=72, "EXP_SMALL_CCD_MINEXP"=73, "EXP_LARGE_CCD_MINEXP"=74, "EXP_GATING_MODE"=75, "EXP_ILME_B1X"=76, "EXP_ILME_B2X"=77, "EXP_ILME_D1X"=78, "EXP_ILME_D2X"=79, "EXP_ILME_D4X"=80, "EXP_INIT_HW_ACCUM"=81, "EXP_5X_GAIN_ENABLE"=82, "EXP_RET_SRCCMP"=83, "EXP_EVENT_HANDLE"=84, "EXP_READOUT_MODE"=85, "EXP_SHUTTER_TYPE"=86, "EXP_USER_DEFINED_CHIP"=87, "EXP_USER_DEFINED_TIMING"=88, "EXP_CONTROLLER_VERSION"=89, "EXP_GET_CONTROLLER_VER"=90, "EXP_TTL_LINES"=91, "EXP_BIT_ADJUST"=92, "EXP_RESOLUTION"=93, "EXP_GAIN"=94, "EXP_ADC_RATE"=95, "EXP_ADC_TYPE"=96, "EXP_NUMBER_OF_CLEANS"=97, "EXP_NUM_OF_STRIPS_PER_CLN"=98, "EXP_INTERFACE_CARD"=99, "EXP_INTERRUPT"=100, "EXP_IO_ADDRESS1"=101, "EXP_IO_ADDRESS2"=102, "EXP_IO_ADDRESS3"=103, "EXP_HW_ROI"=104, "EXP_HW_BINNING"=105, "EXP_EDGE_TRIGGER"=106, "EXP_SHUTTER_CONTROL"=107, "EXP_RS170"=108, "EXP_RS170_COMPLEX"=109, "EXP_HW_RS170_LUT"=110, "EXP_RS170_INTENSITY_SCALING"=111, "EXP_RS170_OFFSET"=112, "EXP_RS170_PAN"=113, "EXP_RS170_ZOOM2X"=114, "EXP_RS170_ZOOM4X"=115, "EXP_RS170_BINNING"=116, "EXP_RS170_DECIMATION"=117, "EXP_HW_ACCUM"=118, "EXP_SHT_PREOPEN"=119, "EXP_STORE_STROBE"=120, "EXP_CONT_CLNS"=121, "EXP_TIMING_MODE"=122, "EXP_EXT_TRIGGER"=123, "EXP_EVENT_COUNTER"=124, "EXP_SW_TRIGGER"=125, "EXP_KINETICS_WINDOWSIZE"=126, "EXP_EXPOSURE"=127, "EXP_CONTROLLER_NAME"=128, "EXP_CCD_CHIP_NAME"=129, "EXP_BSWBINNING"=297, "EXP_EDGEENHANCE"=130, "EXP_BOXVIDEOGAIN"=131, "EXP_HSHADING_VALUE"=132, "EXP_VSHADING_VALUE"=133, "EXP_EDGEENHANCE_FLAG"=134, "EXP_SHADING_FLAG"=135, "EXP_GRAYSCALE"=136, "EXP_OFFSET"=137, "EXP_CCDGAIN"=138, "EXP_TEMPERATURE"=139, "EXP_MCPVOLTAGE"=140, "EXP_BOXEXPOSURE"=141, "EXP_ABC_FLAG"=142, "EXP_GAMMA_FLAG"=143, "EXP_AUTOBLACK_FLAG"=144, "EXP_AGC_FLAG"=145, "EXP_ODD_FIELD"=146, "EXP_FIELD_SELECT"=147, "EXP_RESET"=148, "EXP_EXTERN_ENABLE"=149, "EXP_CONTROLLERS_SUPPORTED"=150, "EXP_VTCLK"=151, "EXP_HTCLK"=152, "EXP_GATE_VS_CW"=153, "EXP_COM_PORT"=154, "EXP_US_UNITS"=156, "EXP_MS_UNITS"=157, "EXP_SEC_UNITS"=158, "EXP_MIN_UNITS"=159, "EXP_HRS_UNITS"=160, "EXP_FRAME_UNITS"=161, "EXP_SYNC_ASYNC"=162, "EXP_FOCUS_NFRAME"=163, "EXP_TIMEOUT"=164, "EXP_TIMEOUT_DEFAULT"=165, "EXP_HW_AUTOSTOP"=166, "EXP_RS170_INTEN_OFFSET"=167, "EXP_CONTROLLER_ALIVE"=168, "EXP_FOCUS_TYPE"=169, "EXP_FOCUS_ZOOM"=170, "EXP_FOCUS_PAN"=171, "EXP_MULTI_TAP_ROI"=172, "EXP_USE_INTERUPTS"=173, "EXP_DATA_ACQ_STATE"=174, "EXP_VERIFY_GOOD_VALUES"=175, "EXP_WHITE_CLAMP"=176, "EXP_BLACK_CLAMP"=177, "EXP_DELAY_TIME"=178, "EXP_READOUT_TIME"=179, "EXP_SW_DIAG"=180, "EXP_DIAG1"=181, "EXP_DIAG2"=182, "EXP_DIAG3"=183, "EXP_DIAG4"=184, "EXP_DIAG5"=185, "EXP_AorB_GROUP"=186, "EXP_ABSORBANCE_FLAG"=187, "EXP_ABSORBANCE_METHOD"=188, "EXP_ABSORBANCE_STRIPNUM"=189, "EXP_DMASIZE_VIA_DRIVER"=190, "EXP_DRIVERVERSION"=191, "EXP_NUM_DEVICES"=192, "EXP_ECPDMA_CHANNEL"=193, "EXP_CUSTOM_SHUTTER"=194, "EXP_ADC_OFFSET"=195, "EXP_CURRENT_READOUT_MODE"=196, "EXP_BANK_ADD"=197, "EXP_LUT_BANK"=198, "EXP_SETUP_STATUS"=201, "EXP_XY_GROUPING"=239, "EXP_MESSAGES_FLAG"=240, "EXP_TTL_LINE_TO_WAIT"=253, "EXP_DATA_COLLECTION_MODE"=258, "EXP_DATA_COLLECTION_TYPE"=262, "EXP_SKIPFRAMES"=274, "EXP_CLR_INT_CNTR"=276, "EXP_ENABLE_INT_CNTR"=277, "EXP_INT_CNTR"=278, "EXP_INTERNAL_SYNC_SRC"=279, "EXP_SW_EXTSYNC"=280, "EXP_PTG_PRESENT"=281, "EXP_ELEC_SHT"=282, "EXP_BOARDS_WITH_NVRAM"=283, "EXP_ANLGMASTER_ST143"=284, "EXP_ANLGSLAVE_ST143"=285, "EXP_DISPLAY_ST143"=286, "EXP_INTRFACE_ST143"=287, "EXP_SCANCONTROL_ST143"=288, "EXP_NUMBERFRAMES_IRQ"=204, "EXP_COOL_TYPE"=214, "EXP_HD_TYPE"=215, "EXP_INTENSIFER_GAIN"=216, "EXP_SHT_GATE_MODE"=217, "EXP_HD_CHECK"=218, "EXP_AMP_MODE"=219, "EXP_AMP_DIALOG"=247, "EXP_ANALOG_GAIN"=220, "EXP_HW_FIXES"=221, "EXP_PCI_CARDS"=222, "EXP_NOT_REVERSE"=223, "EXP_LOAD_NVRAM_DEFAULTS"=234, "EXP_CNTR_BRD"=235, "EXP_XDIMHW"=237, "EXP_YDIMHW"=238, "EXP_SPECIAL_FAST_RDOUT"=254, "EXP_SPCL_FAST_Y_DIM"=255, "EXP_SPCL_FAST_X_DIM"=256, "EXP_SPCL_FAST_Y_INDEX"=257, "EXP_SHUTTER_COMP_TIME_MS"=266, "EXP_NVRAM_AVAIL"=267, "EXP_NUMBER_AGAIN_AVAIL"=269, "EXP_SENSOR_TYPE"=270, "EXP_EVENT_TYPE"=292, "EXP_ANTI_BLOOMING"=293, "EXP_FAST_PULSE_ENABLE"=233, "EXP_USE_HEADCALIB"=296, "EXP_TEMP_STATUS"=301, "EXP_MULTIPLE_READMODES_LIVE"=302, "EXP_FIRST_ACQUIRE_FLAG"=303, "EXP_ANTI_BLOOMING_CONTROL"=304, "EXP_PRE_HORZ_DELAY"=305, "EXP_NVRAM_TRIES"=306, "EXP_XASCEND"=307, "EXP_YASCEND"=308, "EXP_ALT_TIMING"=309, "EXP_SHUTTER_PRE_COMP"=310, "EXP_PVCAM_POSSIBLE"=311, "EXP_ADC_IN_NVRAM"=312, "EXP_PASSTHRU_MODE"=313, "EXP_FIRMWAREVERSION"=314, "EXP_IMMEDIATE_SHUTTER"=315, "EXP_STAGE2_TEMP"=316, "EXP_AVGAIN_ENABLED"=317, "EXP_AVGAIN_SETPOINT"=318, "EXP_AVGAIN"=319, "EXP_AVGAIN_CALIB_TEMP"=320, "EXP_AVGAIN_CALIB_COEFF1"=321, "EXP_AVGAIN_CALIB_COEFF2"=322, "EXP_AVGAIN_CALIB_COEFF3"=323, "EXP_AVGAIN_CALIB_COEFF4"=324, "EXP_AVGAIN_CALIB_COEFF5"=325, "EXP_FORCE_READOUT_MODE"=326, "EXP_RESET_DATACOLLECTION"=327, "EXP_ACTIVE_SUBFRAME"=328, "EXP_PV_READOUT_PORT"=514, "EXP_CLASSNAME"=775, "EXP_FLATFLDNAME"=776, "EXP_DARKNAME"=777, "EXP_SETUPNAME"=778, "EXP_ACCESSNAME"=779, "EXP_DATFILENAME"=780, "EXP_ABSORBFILENAME"=781, "EXP_BLEMISHFILENAME"=782, "EXP_COSMICFILENAME"=783, "EXP_FILEINCBASENAME"=784, "EXP_YTNAME"=785, "EXP_DEVNAME"=786, "EXP_USEROI"=787, "EXP_DOBLEMISH"=788, "EXP_DOABSORB"=789, "EXP_DOCOSMIC"=790, "EXP_COSMICSENS"=791, "EXP_ABSORBSTRIP"=792, "EXP_DATATYPE"=793, "EXP_OVERWRITECONFIRM"=794, "EXP_FILEINCENABLE"=795, "EXP_FILEINCCOUNT"=796, "EXP_RUNNING"=797, "EXP_SAVEROPT"=798, "EXP_TIME_UNITS"=799, "EXP_FILEACCESS"=800, "EXP_AUTOSAVE"=801, "EXP_NEWWINDOW"=802, "EXP_XDIM"=803, "EXP_YDIM"=804, "EXP_XDIMDET"=805, "EXP_YDIMDET"=806, "EXP_ROIMODE"=807, "EXP_NUMREPEATSEXP"=808, "EXP_NUMACCUMSEXP"=809, "EXP_THREADSTATE"=810, "EXP_USEMINTHRESHOLDING"=811, "EXP_MINTHRESHOLDVALUE"=812, "EXP_USEMAXTHRESHOLDING"=813, "EXP_MAXTHRESHOLDVALUE"=814, "EXP_RUNNING_EXPERIMENT"=815, "EXP_THRESHOLD_DEMAND_UPDATE"=816, "EXP_ROICOUNT"=817, "EXP_ACCUMS"=818, "EXP_CACCUMS"=819, "EXP_CSEQUENTS"=820, "EXP_PHOTON_ESTIMATION_ENABLE"=821, "EXP_PHOTON_MAXTIME"=822, "EXP_PHOTON_MAXTIMEUNIT"=823, "EXP_CUSTOMFILTER_ENABLE"=824, "EXP_CUSTOMFILTER_SIZE"=825, "EXP_LOOKUPTABLE_ENABLE"=826, "EXP_BSHOWWINDOW"=827, "EXP_BBACKSUBTRACT"=828, "EXP_BDOFLATFIELD"=829, "EXP_ASCIIOUTPUTFILE"=830, "EXP_ASCIIOUTPUT_DELIMITER"=831, "EXP_ASCIIOUTPUT_TERMINATOR"=832, "EXP_FFTYPE"=833, "EXP_BGTYPE"=834, "EXP_COSGRASS"=835, "EXP_RUNASCONFIRM"=836, "EXP_RUNASRUNACCESS"=837, "EXP_DATAFILETYPE"=838, "EXP_ROTATE"=839, "EXP_FLIP"=840, "EXP_REVERSE"=841, "EXP_SWBINNING"=842, "EXP_AUTOSTORE"=843, "EXP_XBINNED"=844, "EXP_YBINNED"=845, "EXP_NUMPATTERNS"=846, "EXP_EXPERIMENTTIME"=847, "EXP_ASYNCSEQUENTIALS"=848, "EXP_SEQUENTIALS"=849, "EXP_CSEQUENTIALS"=850, "EXP_AUTOD"=851, "EXP_EXPOSURETIME"=852, "EXP_EXPOSURETIME_UNITS"=853, "EXP_ACQMODE"=854, "EXP_DMASIZE_PVCAM"=855, "EXP_INITIALIZE"=856, "EXP_CELL_X_SIZE"=857, "EXP_CELL_Y_SIZE"=858, "EXP_X_GAP_SIZE"=859, "EXP_Y_GAP_SIZE"=860] ("Param")
                n80 = local read "experiment reference"() -> (w100:refnum<k7>)
                n81 = property on="Spectro Correct background" class="Bool (strict)"("DisabledEnum"=T2."Disabled" ("Disabled")) -> ()  [unwired: 2 in, 2 out]
                n82 = invoke class="IExpSetup2" method="SetParam"(reference=w100, "Param"=w102, "pSetVal"=0) -> ()  [unwired: 2 in, 5 out]
              }
            }
          }
          event "Start Scan": Value Change {
            n83 = event-data() -> ()  [unwired: 1 in, 6 out]
            n84 = local read "Spectro ON"() -> (w104:bool)
            n85 = case shown="True" w104 {
              tunnel: [0 16] -> w103
              frame False {
              }
              frame True {
                n86 = local write "busy"(TRUE ("busy")) -> ()
              }
            }
          }
        }
      }
      frame #1 {
        # "Event handler"
        n87 = case shown="16" w108 {
          frame 0, Default {
            # "idle"
          }
          frame 2 {
            # "InitSpectro"
            n88 = Obtain Notifier(name (unnamed)="Winx_Abort", notification data type=FALSE) -> (notifier out=→"notifier out WinX Abort":refnum<notifier>)  [unwired: 2 in, 2 out]
            n89 = Obtain Notifier(name (unnamed)="Winx_Start", notification data type=TRUE) -> (notifier out=→"notifier out WinX Start":refnum<notifier>)  [unwired: 2 in, 2 out]
            n90 = flat-sequence {
              tunnel: w111 -> [w156]
              frame #0 {
                # "monochromator"
                n91 = Automation Open(Automation Refnum="spectroObject reference") -> (Automation Refnum=w120:refnum<k7>)  [unwired: 3 in, 1 out]
                n92 = property class="ISpectroObjMgr"(reference=w120) -> ("Count"=w122:i16)  [unwired: 1 in, 2 out]
                n93 = property class="ISpectroObjMgr"(reference=w120) -> ("Current"=w118:refnum<k7>)  [unwired: 1 in, 2 out]
                "MonoRef" <- w118
                n94 = Greater Than 0?(x=w122) -> (x > 0?=w119:bool)
                n95 = case shown="True" w119 {
                  tunnel: w118 -> [_ w123]
                  frame False {
                  }
                  frame True {
                    w127 = 88 items=["SPT_NOCMD", "SPT_SPECTS_SUPPORTED", "SPT_TYPE", "SPT_CALIBUPDATE", "SPT_GRATINGWARNING", "SPT_LASERWARNING", "SPT_FORCEMOVE", "SPT_INSTNAME", "SPT_USERNAME", "SPT_INSTUSERNAME", "SPT_INSTCOMMNAME", "SPT_WAVE_ORIENTED", "SPT_NUMSTAGES", "SPT_GRATINGSPERTURRET", "SPT_CURRGRATING", "SPT_GRAT_BACKLASH_REQ", "SPT_GRATINGBACKLASHSTEPS", "SPT_NEEDINIT", "SPT_NEED_HWINIT", "SPT_MOTOR", "SPT_ARRAYSIZE", "SPT_ROI_CENTER", "SPT_ORDER", "SPT_CUR_GRATING", "SPT_NEW_GRATING", "SPT_SEQUENCER_STATE", "SPT_NUMTURRETS", "SPT_CURRTURRET", "SPT_DO_RESET", "SPT_SLAVE_CNT", "SPT_NUM_STEPS", "SPT_PIXEL_WIDTH", "SPT_GRAT_USERNAME", "SPT_GRAT_GROOVES", "SPT_GRAT_CENTERADJ", "SPT_GRAT_LINEAR_ADJ", "SPT_GRAT_SLOPE_ADJ", "SPT_GRAT_FOCAL_LEN", "SPT_GRAT_INCL_ANGLE", "SPT_GRAT_DETECT_ANGLE", "SPT_GRAT_MAG", "SPT_ACCESS_ALL_GRAT_SPEEDS", "SPT_SPEED_FOR_EACH_GRATING", "SPT_NUM_SETABLE_GRAT_SPEEDS", "SPT_GRATING_SPEED", "SPT_GRATING_SPEED_MIN", "SPT_GRATING_SPEED_MAX", "SPT_GRAT_REF_GRATING", "SPT_GRAT_STEPSPUNIT", "SPT_GRAT_OFFSET", "SPT_GRAT_ADJUST", "SPT_GRAT_LO_CAL_WAVE", "SPT_GRAT_HI_CAL_WAVE", "SPT_GRAT_LO_POS_WAVE", "SPT_GRAT_HI_POS_WAVE", "SPT_GRAT_REF_WAVE", "SPT_NUM_SLITS", "SPT_SLIT_ENABLED", "SPT_SLIT_LOCATION", "SPT_SLIT_CURPOSITION", "SPT_SLIT_NEWPOSITION", "SPT_SPEED_FOR_EACH_SLIT", "SPT_NUM_SETABLE_SLIT_SPEEDS", "SPT_SLIT_SPEED", "SPT_SLIT_SPEED_MIN", "SPT_SLIT_SPEED_MAX", "SPT_SLIT_STEPSPUNIT", "SPT_SLIT_BACKLASH_REQ", "SPT_SLIT_BACKLASH", "SPT_NUMMIRRORS", "SPT_MIRROR_ENABLED", "SPT_MIRROR_LOCATION", "SPT_MIRROR_CURPOSITION", "SPT_MIRROR_NEWPOSITION", "SPT_OFFSET_AVAIL", "SPT_ADJUST_AVAIL", "SPT_COUNTERSUPPORTED", "SPT_POSITIONSUPPORTED", "SPT_AUTOCALIBSUPPORTED", "SPT_POSITIONMEMORY", "SPT_NUMCOEFFS", "SPT_COEFF", "SPT_SERIAL_IO_SUPPORTED", "SPT_GPIB_IO_SUPPORTED", "SPT_OFFSETADJUSTSUPPORTED", "SPT_LINEARADJUSTSUPPORTED", "SPT_WL_PRECISION", "SPT_NEW_POSITION", "SPT_CUR_POSITION", "SPT_ROI_OFFSET", "SPT_MARK_EXCITATION", "SPT_EXCITATION", "SPT_STEP_SIZE", "SPT_STARTING_WAVELENGTH", "SPT_ENDING_WAVELENGTH", "SPT_MIN_OVERLAP", "SPT_GLUE_BIN_SIZE", "SPT_STARTING_CENTER_WAVE", "SPT_DFLT_BIN_FLAG", "SPT_REPOSITION_FLAG", "SPT_PORT_TYPE", "SPT_PORT_NAME", "SPT_PORT_ADDRESS", "SPT_CUSTOM_NAME", "SPT_GLUE_FILE_NAME", "SPT_DEF_GRATINGSPERTURRET", "SPT_DEF_FOCALLENGTH", "SPT_DEF_INCLUSIONANGLE", "SPT_DEF_DETECTORANGLE", "SPT_DEF_MAGNIFICATION", "SPT_DEF_PIXELWIDTH", "SPT_DEF_REFGRATING", "SPT_DEF_GROOVES", "SPT_DEF_GRAT_USERNAME", "SPT_DEF_GRAT_STEPSPERUNIT", "SPT_DEF_GRAT_SPEED", "SPT_DEF_GRAT_MAX_SPEED", "SPT_DEF_GRAT_MIN_SPEED", "SPT_DEF_GRAT_BACKLASH_REQ", "SPT_DEF_GRAT_BACKLASHSTEPS", "SPT_DEF_SLIT_STEPSPERUNIT", "SPT_DEF_SLIT_SPEED", "SPT_DEF_SLIT_MAX_SPEED", "SPT_DEF_SLIT_MIN_SPEED", "SPT_DEF_SLIT_BACKLASH_REQ", "SPT_DEF_SLIT_BACKLASHSTEPS", "SPT_MIN_SLIT_POS", "SPT_MAX_SLIT_POS", "SPT_SLIT_POS_UNITS", "SPT_DEF_PORTADDRESS", "SPT_DEF_PORTNAME", "SPT_DEF_PORTTYPE", "SPT_SETTINGSLOADED", "SPT_BAUDRATE", "SPT_DATABITS", "SPT_STOPBITS", "SPT_PARITY", "SPT_CTSFLOW", "SPT_MODELNAME", "SPT_SERIALNUMBER", "SPT_VALIDITYFLAG", "SPT_EXISTS", "SPT_CHANGED", "SPT_MANUFACTURE_NAME", "SPT_TRIMTOPRECISION", "SPT_GRAT_TYPE", "SPT_COMM_PORT", "SPT_RESET_WAIT_FLAG", "SPT_DEMOPORT_FLAG", "SPT_INST_NUMTURRETS", "SPT_INST_CURR_TURRET", "SPT_INST_GRAT_GROOVES", "SPT_INST_CUR_GRAT_NUM", "SPT_INST_GRAT_USERNAME", "SPT_INST_CUR_GRAT_POS", "SPT_INST_GRAT_SPEED", "SPT_INST_MODELNAME", "SPT_INST_SERIALNUMBER", "SPT_INST_NUM_SLITS", "SPT_INST_SLIT_LOCATION", "SPT_INST_SLIT_POSITION", "SPT_INST_SLIT_SPEED", "SPT_INST_NUM_MIRRORS", "SPT_INST_MIRROR_LOCATION", "SPT_INST_MIRROR_POSITION", "SPT_ACTIVE_MIRROR_LOC", "SPT_ACTIVE_MIRROR_POS", "SPT_GRAT_MOVE_MODE", "SPT_ACTIVE_GRAT_POS", "SPT_ACTIVE_GRATING_NUM", "SPT_ACTIVE_SLIT_LOC", "SPT_ACTIVE_SLIT_POS", "SPT_STEP_ERROR_CODE", "SPT_ERROR_CODE", "SPT_ACTIVE_TURRET_NUM", "SPT_DLL_INDEX", "SPT_NMTOSTEPS_WL", "SPT_NMTOSTEPS_STEPS", "SPT_NUM_SPECT_DLLS", "SPT_NUM_SPECT_AVAIL", "SPT_MESSAGE_WND_HNDL", "SPT_MUTEX", "SPT_CALC_WL_INCENTERWL", "SPT_CALC_WL_INDIST", "SPT_CALC_WL_OUTWL", "SPT_ARRAY_CENTER", "SPT_CURR_CALIB_PTR", "SPT_DLL_TYPE", "SPT_NEW_SLIT_INDEX", "SPT_NEW_MIRROR_INDEX", "SPT_CALCSLOPEADJ_WL", "SPT_CALCSLOPEADJ_SLOPE", "SPT_MAX_GRATINGS_PER_TURRET", "SPT_MAX_NUM_TURRETS", "SPT_MAX_NUM_MIRRORS", "SPT_MAX_NUM_SLITS", "SPT_GRATING_SPEED_INDEX", "SPT_SLIT_SPEED_INDEX", "SPT_GRATING_SPEED_UNITS", "SPT_GRATING_SPEED_NAME", "SPT_SLIT_SPEED_UNITS", "SPT_SLIT_SPEED_NAME", "SPT_NEED_GRATING_SPEED_SET", "SPT_NEED_SLIT_SPEED_SET", "SPT_GRAT_STEPSUNIT_UNIT", "SPT_SLIT_STEPSUNIT_UNIT", "SPT_PROCESS_MOVE_STATUS", "SPT_RESET", "SPT_RESET_TIMEOUT_MS", "SPT_GENERIC_DLG_MAIN_TITLE", "SPT_GENERIC_DLG_INDEX", "SPT_GENERIC_EDITBOX_TXT", "SPT_GENERIC_EDITBOX", "SPT_GENERIC_SPINBUTTON", "SPT_GENERIC_CHECKBOX_TXT", "SPT_GENERIC_CHECKBOX", "SPT_GENERIC_COMBOBOX_TXT", "SPT_GENERIC_COMBOBOX", "SPT_GENERIC_RADIOBUTTON_GRP", "SPT_GENERIC_RADIOBUTTON_TXT", "SPT_GENERIC_RADIOBUTTON", "SPT_DLL_PRODUCT_VERSION", "SPT_DLL_FILE_VERSION", "SPT_END_OF_LIST"] ("Param")
                    w132 = 23 items=["SPT_NOCMD", "SPT_SPECTS_SUPPORTED", "SPT_TYPE", "SPT_CALIBUPDATE", "SPT_GRATINGWARNING", "SPT_LASERWARNING", "SPT_FORCEMOVE", "SPT_INSTNAME", "SPT_USERNAME", "SPT_INSTUSERNAME", "SPT_INSTCOMMNAME", "SPT_WAVE_ORIENTED", "SPT_NUMSTAGES", "SPT_GRATINGSPERTURRET", "SPT_CURRGRATING", "SPT_GRAT_BACKLASH_REQ", "SPT_GRATINGBACKLASHSTEPS", "SPT_NEEDINIT", "SPT_NEED_HWINIT", "SPT_MOTOR", "SPT_ARRAYSIZE", "SPT_ROI_CENTER", "SPT_ORDER", "SPT_CUR_GRATING", "SPT_NEW_GRATING", "SPT_SEQUENCER_STATE", "SPT_NUMTURRETS", "SPT_CURRTURRET", "SPT_DO_RESET", "SPT_SLAVE_CNT", "SPT_NUM_STEPS", "SPT_PIXEL_WIDTH", "SPT_GRAT_USERNAME", "SPT_GRAT_GROOVES", "SPT_GRAT_CENTERADJ", "SPT_GRAT_LINEAR_ADJ", "SPT_GRAT_SLOPE_ADJ", "SPT_GRAT_FOCAL_LEN", "SPT_GRAT_INCL_ANGLE", "SPT_GRAT_DETECT_ANGLE", "SPT_GRAT_MAG", "SPT_ACCESS_ALL_GRAT_SPEEDS", "SPT_SPEED_FOR_EACH_GRATING", "SPT_NUM_SETABLE_GRAT_SPEEDS", "SPT_GRATING_SPEED", "SPT_GRATING_SPEED_MIN", "SPT_GRATING_SPEED_MAX", "SPT_GRAT_REF_GRATING", "SPT_GRAT_STEPSPUNIT", "SPT_GRAT_OFFSET", "SPT_GRAT_ADJUST", "SPT_GRAT_LO_CAL_WAVE", "SPT_GRAT_HI_CAL_WAVE", "SPT_GRAT_LO_POS_WAVE", "SPT_GRAT_HI_POS_WAVE", "SPT_GRAT_REF_WAVE", "SPT_NUM_SLITS", "SPT_SLIT_ENABLED", "SPT_SLIT_LOCATION", "SPT_SLIT_CURPOSITION", "SPT_SLIT_NEWPOSITION", "SPT_SPEED_FOR_EACH_SLIT", "SPT_NUM_SETABLE_SLIT_SPEEDS", "SPT_SLIT_SPEED", "SPT_SLIT_SPEED_MIN", "SPT_SLIT_SPEED_MAX", "SPT_SLIT_STEPSPUNIT", "SPT_SLIT_BACKLASH_REQ", "SPT_SLIT_BACKLASH", "SPT_NUMMIRRORS", "SPT_MIRROR_ENABLED", "SPT_MIRROR_LOCATION", "SPT_MIRROR_CURPOSITION", "SPT_MIRROR_NEWPOSITION", "SPT_OFFSET_AVAIL", "SPT_ADJUST_AVAIL", "SPT_COUNTERSUPPORTED", "SPT_POSITIONSUPPORTED", "SPT_AUTOCALIBSUPPORTED", "SPT_POSITIONMEMORY", "SPT_NUMCOEFFS", "SPT_COEFF", "SPT_SERIAL_IO_SUPPORTED", "SPT_GPIB_IO_SUPPORTED", "SPT_OFFSETADJUSTSUPPORTED", "SPT_LINEARADJUSTSUPPORTED", "SPT_WL_PRECISION", "SPT_NEW_POSITION", "SPT_CUR_POSITION", "SPT_ROI_OFFSET", "SPT_MARK_EXCITATION", "SPT_EXCITATION", "SPT_STEP_SIZE", "SPT_STARTING_WAVELENGTH", "SPT_ENDING_WAVELENGTH", "SPT_MIN_OVERLAP", "SPT_GLUE_BIN_SIZE", "SPT_STARTING_CENTER_WAVE", "SPT_DFLT_BIN_FLAG", "SPT_REPOSITION_FLAG", "SPT_PORT_TYPE", "SPT_PORT_NAME", "SPT_PORT_ADDRESS", "SPT_CUSTOM_NAME", "SPT_GLUE_FILE_NAME", "SPT_DEF_GRATINGSPERTURRET", "SPT_DEF_FOCALLENGTH", "SPT_DEF_INCLUSIONANGLE", "SPT_DEF_DETECTORANGLE", "SPT_DEF_MAGNIFICATION", "SPT_DEF_PIXELWIDTH", "SPT_DEF_REFGRATING", "SPT_DEF_GROOVES", "SPT_DEF_GRAT_USERNAME", "SPT_DEF_GRAT_STEPSPERUNIT", "SPT_DEF_GRAT_SPEED", "SPT_DEF_GRAT_MAX_SPEED", "SPT_DEF_GRAT_MIN_SPEED", "SPT_DEF_GRAT_BACKLASH_REQ", "SPT_DEF_GRAT_BACKLASHSTEPS", "SPT_DEF_SLIT_STEPSPERUNIT", "SPT_DEF_SLIT_SPEED", "SPT_DEF_SLIT_MAX_SPEED", "SPT_DEF_SLIT_MIN_SPEED", "SPT_DEF_SLIT_BACKLASH_REQ", "SPT_DEF_SLIT_BACKLASHSTEPS", "SPT_MIN_SLIT_POS", "SPT_MAX_SLIT_POS", "SPT_SLIT_POS_UNITS", "SPT_DEF_PORTADDRESS", "SPT_DEF_PORTNAME", "SPT_DEF_PORTTYPE", "SPT_SETTINGSLOADED", "SPT_BAUDRATE", "SPT_DATABITS", "SPT_STOPBITS", "SPT_PARITY", "SPT_CTSFLOW", "SPT_MODELNAME", "SPT_SERIALNUMBER", "SPT_VALIDITYFLAG", "SPT_EXISTS", "SPT_CHANGED", "SPT_MANUFACTURE_NAME", "SPT_TRIMTOPRECISION", "SPT_GRAT_TYPE", "SPT_COMM_PORT", "SPT_RESET_WAIT_FLAG", "SPT_DEMOPORT_FLAG", "SPT_INST_NUMTURRETS", "SPT_INST_CURR_TURRET", "SPT_INST_GRAT_GROOVES", "SPT_INST_CUR_GRAT_NUM", "SPT_INST_GRAT_USERNAME", "SPT_INST_CUR_GRAT_POS", "SPT_INST_GRAT_SPEED", "SPT_INST_MODELNAME", "SPT_INST_SERIALNUMBER", "SPT_INST_NUM_SLITS", "SPT_INST_SLIT_LOCATION", "SPT_INST_SLIT_POSITION", "SPT_INST_SLIT_SPEED", "SPT_INST_NUM_MIRRORS", "SPT_INST_MIRROR_LOCATION", "SPT_INST_MIRROR_POSITION", "SPT_ACTIVE_MIRROR_LOC", "SPT_ACTIVE_MIRROR_POS", "SPT_GRAT_MOVE_MODE", "SPT_ACTIVE_GRAT_POS", "SPT_ACTIVE_GRATING_NUM", "SPT_ACTIVE_SLIT_LOC", "SPT_ACTIVE_SLIT_POS", "SPT_STEP_ERROR_CODE", "SPT_ERROR_CODE", "SPT_ACTIVE_TURRET_NUM", "SPT_DLL_INDEX", "SPT_NMTOSTEPS_WL", "SPT_NMTOSTEPS_STEPS", "SPT_NUM_SPECT_DLLS", "SPT_NUM_SPECT_AVAIL", "SPT_MESSAGE_WND_HNDL", "SPT_MUTEX", "SPT_CALC_WL_INCENTERWL", "SPT_CALC_WL_INDIST", "SPT_CALC_WL_OUTWL", "SPT_ARRAY_CENTER", "SPT_CURR_CALIB_PTR", "SPT_DLL_TYPE", "SPT_NEW_SLIT_INDEX", "SPT_NEW_MIRROR_INDEX", "SPT_CALCSLOPEADJ_WL", "SPT_CALCSLOPEADJ_SLOPE", "SPT_MAX_GRATINGS_PER_TURRET", "SPT_MAX_NUM_TURRETS", "SPT_MAX_NUM_MIRRORS", "SPT_MAX_NUM_SLITS", "SPT_GRATING_SPEED_INDEX", "SPT_SLIT_SPEED_INDEX", "SPT_GRATING_SPEED_UNITS", "SPT_GRATING_SPEED_NAME", "SPT_SLIT_SPEED_UNITS", "SPT_SLIT_SPEED_NAME", "SPT_NEED_GRATING_SPEED_SET", "SPT_NEED_SLIT_SPEED_SET", "SPT_GRAT_STEPSUNIT_UNIT", "SPT_SLIT_STEPSUNIT_UNIT", "SPT_PROCESS_MOVE_STATUS", "SPT_RESET", "SPT_RESET_TIMEOUT_MS", "SPT_GENERIC_DLG_MAIN_TITLE", "SPT_GENERIC_DLG_INDEX", "SPT_GENERIC_EDITBOX_TXT", "SPT_GENERIC_EDITBOX", "SPT_GENERIC_SPINBUTTON", "SPT_GENERIC_CHECKBOX_TXT", "SPT_GENERIC_CHECKBOX", "SPT_GENERIC_COMBOBOX_TXT", "SPT_GENERIC_COMBOBOX", "SPT_GENERIC_RADIOBUTTON_GRP", "SPT_GENERIC_RADIOBUTTON_TXT", "SPT_GENERIC_RADIOBUTTON", "SPT_DLL_PRODUCT_VERSION", "SPT_DLL_FILE_VERSION", "SPT_END_OF_LIST"] ("Param")
                    n96 = invoke class="ISpectroObj" method="GetParam"(reference=w123, "Param"=w132) -> (reference out=w128:refnum<k7>, "GetParam"=w130:variant)  [unwired: 4 in, 4 out]
                    n97 = invoke class="ISpectroObj" method="GetParam"(reference=w128, "Param"=w127) -> ("GetParam"=w126:variant)  [unwired: 4 in, 5 out]
                    n98 = Variant To Data(type=0, Variant=w130) -> (data=w129:i32)  [unwired: 1 in, 1 out]
                    n99 = local write "Grating Number"(w129) -> ()
                    n100 = Variant To Data(type=0.0, Variant=w126) -> (data=w124:dbl)  [unwired: 1 in, 1 out]
                    n101 = local write "Wavelength (nm)"(w124) -> ()
                  }
                }
              }
              frame #1 {
                w138 = 828 items=["EXP_ETACTUAL"=1, "EXP_SEQUENTS"=2, "EXP_ERROR"=3, "EXP_GETCAPS"=4, "EXP_GETPLSR"=5, "EXP_DETECTOR_BIT"=16, "EXP_RUNNING_APP"=23, "EXP_VIDEO_TYPE"=24, "EXP_CUSTOM_VIDEO_X"=25, "EXP_CUSTOM_VIDEO_Y"=26, "EXP_CUSTOM_VIDEO_FSTWIDTH"=27, "EXP_CUSTOM_VIDEO_LSTWIDTH"=28, "EXP_VIDEO_XDIM"=29, "EXP_VIDEO_YDIM"=30, "EXP_VIDEO_MAX_ZOOM"=31, "EXP_VIDEO_HORZ_PAN"=32, "EXP_VIDEO_VERT_PAN"=33, "EXP_WORD_MULTIPLIER"=34, "EXP_TARGET_ID"=35, "EXP_ADAPTER_ID"=36, "EXP_NUMADAPTORS"=37, "EXP_FORCE_PP_INIT"=38, "EXP_NOP_ADC"=39, "EXP_ACTUAL_TEMP"=40, "EXP_FORCE_AUTOSTOP"=41, "EXP_DEFAULT_VTCLK"=42, "EXP_MIN_VTCLK"=43, "EXP_MAX_VTCLK"=44, "EXP_DEFAULT_HTCLK"=45, "EXP_MIN_HTCLK"=46, "EXP_MAX_HTCLK"=47, "EXP_TIMING_STYLE"=48, "EXP_HEADSELECT"=49, "EXP_HORZPHASE"=50, "EXP_VERTPHASE"=51, "EXP_SPECIAL_SPEED"=52, "EXP_PRE_STRIPS"=53, "EXP_POST_STRIPS"=54, "EXP_PRE_LINES"=55, "EXP_POST_LINES"=56, "EXP_ACTIVE_LINES"=57, "EXP_ACTIVE_STRIPS"=58, "EXP_XFER_EXTRA"=59, "EXP_MIN_BLOCK"=60, "EXP_NUM_MIN_BLOCK"=61, "EXP_LOGIC_OUTPUT"=66, "EXP_VIDEO_BLANK"=67, "EXP_ZOOM_MODE_VIDEO"=68, "EXP_LEVEL_SYNC"=69, "EXP_DISABLE_LASER"=70, "EXP_ACQBACK_SHUTTER"=71, "EXP_ACQFLAT_SHUTTER"=72, "EXP_SMALL_CCD_MINEXP"=73, "EXP_LARGE_CCD_MINEXP"=74, "EXP_GATING_MODE"=75, "EXP_ILME_B1X"=76, "EXP_ILME_B2X"=77, "EXP_ILME_D1X"=78, "EXP_ILME_D2X"=79, "EXP_ILME_D4X"=80, "EXP_INIT_HW_ACCUM"=81, "EXP_5X_GAIN_ENABLE"=82, "EXP_RET_SRCCMP"=83, "EXP_EVENT_HANDLE"=84, "EXP_READOUT_MODE"=85, "EXP_SHUTTER_TYPE"=86, "EXP_USER_DEFINED_CHIP"=87, "EXP_USER_DEFINED_TIMING"=88, "EXP_CONTROLLER_VERSION"=89, "EXP_GET_CONTROLLER_VER"=90, "EXP_TTL_LINES"=91, "EXP_BIT_ADJUST"=92, "EXP_RESOLUTION"=93, "EXP_GAIN"=94, "EXP_ADC_RATE"=95, "EXP_ADC_TYPE"=96, "EXP_NUMBER_OF_CLEANS"=97, "EXP_NUM_OF_STRIPS_PER_CLN"=98, "EXP_INTERFACE_CARD"=99, "EXP_INTERRUPT"=100, "EXP_IO_ADDRESS1"=101, "EXP_IO_ADDRESS2"=102, "EXP_IO_ADDRESS3"=103, "EXP_HW_ROI"=104, "EXP_HW_BINNING"=105, "EXP_EDGE_TRIGGER"=106, "EXP_SHUTTER_CONTROL"=107, "EXP_RS170"=108, "EXP_RS170_COMPLEX"=109, "EXP_HW_RS170_LUT"=110, "EXP_RS170_INTENSITY_SCALING"=111, "EXP_RS170_OFFSET"=112, "EXP_RS170_PAN"=113, "EXP_RS170_ZOOM2X"=114, "EXP_RS170_ZOOM4X"=115, "EXP_RS170_BINNING"=116, "EXP_RS170_DECIMATION"=117, "EXP_HW_ACCUM"=118, "EXP_SHT_PREOPEN"=119, "EXP_STORE_STROBE"=120, "EXP_CONT_CLNS"=121, "EXP_TIMING_MODE"=122, "EXP_EXT_TRIGGER"=123, "EXP_EVENT_COUNTER"=124, "EXP_SW_TRIGGER"=125, "EXP_KINETICS_WINDOWSIZE"=126, "EXP_EXPOSURE"=127, "EXP_CONTROLLER_NAME"=128, "EXP_CCD_CHIP_NAME"=129, "EXP_BSWBINNING"=297, "EXP_EDGEENHANCE"=130, "EXP_BOXVIDEOGAIN"=131, "EXP_HSHADING_VALUE"=132, "EXP_VSHADING_VALUE"=133, "EXP_EDGEENHANCE_FLAG"=134, "EXP_SHADING_FLAG"=135, "EXP_GRAYSCALE"=136, "EXP_OFFSET"=137, "EXP_CCDGAIN"=138, "EXP_TEMPERATURE"=139, "EXP_MCPVOLTAGE"=140, "EXP_BOXEXPOSURE"=141, "EXP_ABC_FLAG"=142, "EXP_GAMMA_FLAG"=143, "EXP_AUTOBLACK_FLAG"=144, "EXP_AGC_FLAG"=145, "EXP_ODD_FIELD"=146, "EXP_FIELD_SELECT"=147, "EXP_RESET"=148, "EXP_EXTERN_ENABLE"=149, "EXP_CONTROLLERS_SUPPORTED"=150, "EXP_VTCLK"=151, "EXP_HTCLK"=152, "EXP_GATE_VS_CW"=153, "EXP_COM_PORT"=154, "EXP_US_UNITS"=156, "EXP_MS_UNITS"=157, "EXP_SEC_UNITS"=158, "EXP_MIN_UNITS"=159, "EXP_HRS_UNITS"=160, "EXP_FRAME_UNITS"=161, "EXP_SYNC_ASYNC"=162, "EXP_FOCUS_NFRAME"=163, "EXP_TIMEOUT"=164, "EXP_TIMEOUT_DEFAULT"=165, "EXP_HW_AUTOSTOP"=166, "EXP_RS170_INTEN_OFFSET"=167, "EXP_CONTROLLER_ALIVE"=168, "EXP_FOCUS_TYPE"=169, "EXP_FOCUS_ZOOM"=170, "EXP_FOCUS_PAN"=171, "EXP_MULTI_TAP_ROI"=172, "EXP_USE_INTERUPTS"=173, "EXP_DATA_ACQ_STATE"=174, "EXP_VERIFY_GOOD_VALUES"=175, "EXP_WHITE_CLAMP"=176, "EXP_BLACK_CLAMP"=177, "EXP_DELAY_TIME"=178, "EXP_READOUT_TIME"=179, "EXP_SW_DIAG"=180, "EXP_DIAG1"=181, "EXP_DIAG2"=182, "EXP_DIAG3"=183, "EXP_DIAG4"=184, "EXP_DIAG5"=185, "EXP_AorB_GROUP"=186, "EXP_ABSORBANCE_FLAG"=187, "EXP_ABSORBANCE_METHOD"=188, "EXP_ABSORBANCE_STRIPNUM"=189, "EXP_DMASIZE_VIA_DRIVER"=190, "EXP_DRIVERVERSION"=191, "EXP_NUM_DEVICES"=192, "EXP_ECPDMA_CHANNEL"=193, "EXP_CUSTOM_SHUTTER"=194, "EXP_ADC_OFFSET"=195, "EXP_CURRENT_READOUT_MODE"=196, "EXP_BANK_ADD"=197, "EXP_LUT_BANK"=198, "EXP_SETUP_STATUS"=201, "EXP_XY_GROUPING"=239, "EXP_MESSAGES_FLAG"=240, "EXP_TTL_LINE_TO_WAIT"=253, "EXP_DATA_COLLECTION_MODE"=258, "EXP_DATA_COLLECTION_TYPE"=262, "EXP_SKIPFRAMES"=274, "EXP_CLR_INT_CNTR"=276, "EXP_ENABLE_INT_CNTR"=277, "EXP_INT_CNTR"=278, "EXP_INTERNAL_SYNC_SRC"=279, "EXP_SW_EXTSYNC"=280, "EXP_PTG_PRESENT"=281, "EXP_ELEC_SHT"=282, "EXP_BOARDS_WITH_NVRAM"=283, "EXP_ANLGMASTER_ST143"=284, "EXP_ANLGSLAVE_ST143"=285, "EXP_DISPLAY_ST143"=286, "EXP_INTRFACE_ST143"=287, "EXP_SCANCONTROL_ST143"=288, "EXP_NUMBERFRAMES_IRQ"=204, "EXP_COOL_TYPE"=214, "EXP_HD_TYPE"=215, "EXP_INTENSIFER_GAIN"=216, "EXP_SHT_GATE_MODE"=217, "EXP_HD_CHECK"=218, "EXP_AMP_MODE"=219, "EXP_AMP_DIALOG"=247, "EXP_ANALOG_GAIN"=220, "EXP_HW_FIXES"=221, "EXP_PCI_CARDS"=222, "EXP_NOT_REVERSE"=223, "EXP_LOAD_NVRAM_DEFAULTS"=234, "EXP_CNTR_BRD"=235, "EXP_XDIMHW"=237, "EXP_YDIMHW"=238, "EXP_SPECIAL_FAST_RDOUT"=254, "EXP_SPCL_FAST_Y_DIM"=255, "EXP_SPCL_FAST_X_DIM"=256, "EXP_SPCL_FAST_Y_INDEX"=257, "EXP_SHUTTER_COMP_TIME_MS"=266, "EXP_NVRAM_AVAIL"=267, "EXP_NUMBER_AGAIN_AVAIL"=269, "EXP_SENSOR_TYPE"=270, "EXP_EVENT_TYPE"=292, "EXP_ANTI_BLOOMING"=293, "EXP_FAST_PULSE_ENABLE"=233, "EXP_USE_HEADCALIB"=296, "EXP_TEMP_STATUS"=301, "EXP_MULTIPLE_READMODES_LIVE"=302, "EXP_FIRST_ACQUIRE_FLAG"=303, "EXP_ANTI_BLOOMING_CONTROL"=304, "EXP_PRE_HORZ_DELAY"=305, "EXP_NVRAM_TRIES"=306, "EXP_XASCEND"=307, "EXP_YASCEND"=308, "EXP_ALT_TIMING"=309, "EXP_SHUTTER_PRE_COMP"=310, "EXP_PVCAM_POSSIBLE"=311, "EXP_ADC_IN_NVRAM"=312, "EXP_PASSTHRU_MODE"=313, "EXP_FIRMWAREVERSION"=314, "EXP_IMMEDIATE_SHUTTER"=315, "EXP_STAGE2_TEMP"=316, "EXP_AVGAIN_ENABLED"=317, "EXP_AVGAIN_SETPOINT"=318, "EXP_AVGAIN"=319, "EXP_AVGAIN_CALIB_TEMP"=320, "EXP_AVGAIN_CALIB_COEFF1"=321, "EXP_AVGAIN_CALIB_COEFF2"=322, "EXP_AVGAIN_CALIB_COEFF3"=323, "EXP_AVGAIN_CALIB_COEFF4"=324, "EXP_AVGAIN_CALIB_COEFF5"=325, "EXP_FORCE_READOUT_MODE"=326, "EXP_RESET_DATACOLLECTION"=327, "EXP_ACTIVE_SUBFRAME"=328, "EXP_PV_READOUT_PORT"=514, "EXP_CLASSNAME"=775, "EXP_FLATFLDNAME"=776, "EXP_DARKNAME"=777, "EXP_SETUPNAME"=778, "EXP_ACCESSNAME"=779, "EXP_DATFILENAME"=780, "EXP_ABSORBFILENAME"=781, "EXP_BLEMISHFILENAME"=782, "EXP_COSMICFILENAME"=783, "EXP_FILEINCBASENAME"=784, "EXP_YTNAME"=785, "EXP_DEVNAME"=786, "EXP_USEROI"=787, "EXP_DOBLEMISH"=788, "EXP_DOABSORB"=789, "EXP_DOCOSMIC"=790, "EXP_COSMICSENS"=791, "EXP_ABSORBSTRIP"=792, "EXP_DATATYPE"=793, "EXP_OVERWRITECONFIRM"=794, "EXP_FILEINCENABLE"=795, "EXP_FILEINCCOUNT"=796, "EXP_RUNNING"=797, "EXP_SAVEROPT"=798, "EXP_TIME_UNITS"=799, "EXP_FILEACCESS"=800, "EXP_AUTOSAVE"=801, "EXP_NEWWINDOW"=802, "EXP_XDIM"=803, "EXP_YDIM"=804, "EXP_XDIMDET"=805, "EXP_YDIMDET"=806, "EXP_ROIMODE"=807, "EXP_NUMREPEATSEXP"=808, "EXP_NUMACCUMSEXP"=809, "EXP_THREADSTATE"=810, "EXP_USEMINTHRESHOLDING"=811, "EXP_MINTHRESHOLDVALUE"=812, "EXP_USEMAXTHRESHOLDING"=813, "EXP_MAXTHRESHOLDVALUE"=814, "EXP_RUNNING_EXPERIMENT"=815, "EXP_THRESHOLD_DEMAND_UPDATE"=816, "EXP_ROICOUNT"=817, "EXP_ACCUMS"=818, "EXP_CACCUMS"=819, "EXP_CSEQUENTS"=820, "EXP_PHOTON_ESTIMATION_ENABLE"=821, "EXP_PHOTON_MAXTIME"=822, "EXP_PHOTON_MAXTIMEUNIT"=823, "EXP_CUSTOMFILTER_ENABLE"=824, "EXP_CUSTOMFILTER_SIZE"=825, "EXP_LOOKUPTABLE_ENABLE"=826, "EXP_BSHOWWINDOW"=827, "EXP_BBACKSUBTRACT"=828, "EXP_BDOFLATFIELD"=829, "EXP_ASCIIOUTPUTFILE"=830, "EXP_ASCIIOUTPUT_DELIMITER"=831, "EXP_ASCIIOUTPUT_TERMINATOR"=832, "EXP_FFTYPE"=833, "EXP_BGTYPE"=834, "EXP_COSGRASS"=835, "EXP_RUNASCONFIRM"=836, "EXP_RUNASRUNACCESS"=837, "EXP_DATAFILETYPE"=838, "EXP_ROTATE"=839, "EXP_FLIP"=840, "EXP_REVERSE"=841, "EXP_SWBINNING"=842, "EXP_AUTOSTORE"=843, "EXP_XBINNED"=844, "EXP_YBINNED"=845, "EXP_NUMPATTERNS"=846, "EXP_EXPERIMENTTIME"=847, "EXP_ASYNCSEQUENTIALS"=848, "EXP_SEQUENTIALS"=849, "EXP_CSEQUENTIALS"=850, "EXP_AUTOD"=851, "EXP_EXPOSURETIME"=852, "EXP_EXPOSURETIME_UNITS"=853, "EXP_ACQMODE"=854, "EXP_DMASIZE_PVCAM"=855, "EXP_INITIALIZE"=856, "EXP_CELL_X_SIZE"=857, "EXP_CELL_Y_SIZE"=858, "EXP_X_GAP_SIZE"=859, "EXP_Y_GAP_SIZE"=860] ("Param")
                w141 = 795 items=["EXP_ETACTUAL"=1, "EXP_SEQUENTS"=2, "EXP_ERROR"=3, "EXP_GETCAPS"=4, "EXP_GETPLSR"=5, "EXP_DETECTOR_BIT"=16, "EXP_RUNNING_APP"=23, "EXP_VIDEO_TYPE"=24, "EXP_CUSTOM_VIDEO_X"=25, "EXP_CUSTOM_VIDEO_Y"=26, "EXP_CUSTOM_VIDEO_FSTWIDTH"=27, "EXP_CUSTOM_VIDEO_LSTWIDTH"=28, "EXP_VIDEO_XDIM"=29, "EXP_VIDEO_YDIM"=30, "EXP_VIDEO_MAX_ZOOM"=31, "EXP_VIDEO_HORZ_PAN"=32, "EXP_VIDEO_VERT_PAN"=33, "EXP_WORD_MULTIPLIER"=34, "EXP_TARGET_ID"=35, "EXP_ADAPTER_ID"=36, "EXP_NUMADAPTORS"=37, "EXP_FORCE_PP_INIT"=38, "EXP_NOP_ADC"=39, "EXP_ACTUAL_TEMP"=40, "EXP_FORCE_AUTOSTOP"=41, "EXP_DEFAULT_VTCLK"=42, "EXP_MIN_VTCLK"=43, "EXP_MAX_VTCLK"=44, "EXP_DEFAULT_HTCLK"=45, "EXP_MIN_HTCLK"=46, "EXP_MAX_HTCLK"=47, "EXP_TIMING_STYLE"=48, "EXP_HEADSELECT"=49, "EXP_HORZPHASE"=50, "EXP_VERTPHASE"=51, "EXP_SPECIAL_SPEED"=52, "EXP_PRE_STRIPS"=53, "EXP_POST_STRIPS"=54, "EXP_PRE_LINES"=55, "EXP_POST_LINES"=56, "EXP_ACTIVE_LINES"=57, "EXP_ACTIVE_STRIPS"=58, "EXP_XFER_EXTRA"=59, "EXP_MIN_BLOCK"=60, "EXP_NUM_MIN_BLOCK"=61, "EXP_LOGIC_OUTPUT"=66, "EXP_VIDEO_BLANK"=67, "EXP_ZOOM_MODE_VIDEO"=68, "EXP_LEVEL_SYNC"=69, "EXP_DISABLE_LASER"=70, "EXP_ACQBACK_SHUTTER"=71, "EXP_ACQFLAT_SHUTTER"=72, "EXP_SMALL_CCD_MINEXP"=73, "EXP_LARGE_CCD_MINEXP"=74, "EXP_GATING_MODE"=75, "EXP_ILME_B1X"=76, "EXP_ILME_B2X"=77, "EXP_ILME_D1X"=78, "EXP_ILME_D2X"=79, "EXP_ILME_D4X"=80, "EXP_INIT_HW_ACCUM"=81, "EXP_5X_GAIN_ENABLE"=82, "EXP_RET_SRCCMP"=83, "EXP_EVENT_HANDLE"=84, "EXP_READOUT_MODE"=85, "EXP_SHUTTER_TYPE"=86, "EXP_USER_DEFINED_CHIP"=87, "EXP_USER_DEFINED_TIMING"=88, "EXP_CONTROLLER_VERSION"=89, "EXP_GET_CONTROLLER_VER"=90, "EXP_TTL_LINES"=91, "EXP_BIT_ADJUST"=92, "EXP_RESOLUTION"=93, "EXP_GAIN"=94, "EXP_ADC_RATE"=95, "EXP_ADC_TYPE"=96, "EXP_NUMBER_OF_CLEANS"=97, "EXP_NUM_OF_STRIPS_PER_CLN"=98, "EXP_INTERFACE_CARD"=99, "EXP_INTERRUPT"=100, "EXP_IO_ADDRESS1"=101, "EXP_IO_ADDRESS2"=102, "EXP_IO_ADDRESS3"=103, "EXP_HW_ROI"=104, "EXP_HW_BINNING"=105, "EXP_EDGE_TRIGGER"=106, "EXP_SHUTTER_CONTROL"=107, "EXP_RS170"=108, "EXP_RS170_COMPLEX"=109, "EXP_HW_RS170_LUT"=110, "EXP_RS170_INTENSITY_SCALING"=111, "EXP_RS170_OFFSET"=112, "EXP_RS170_PAN"=113, "EXP_RS170_ZOOM2X"=114, "EXP_RS170_ZOOM4X"=115, "EXP_RS170_BINNING"=116, "EXP_RS170_DECIMATION"=117, "EXP_HW_ACCUM"=118, "EXP_SHT_PREOPEN"=119, "EXP_STORE_STROBE"=120, "EXP_CONT_CLNS"=121, "EXP_TIMING_MODE"=122, "EXP_EXT_TRIGGER"=123, "EXP_EVENT_COUNTER"=124, "EXP_SW_TRIGGER"=125, "EXP_KINETICS_WINDOWSIZE"=126, "EXP_EXPOSURE"=127, "EXP_CONTROLLER_NAME"=128, "EXP_CCD_CHIP_NAME"=129, "EXP_BSWBINNING"=297, "EXP_EDGEENHANCE"=130, "EXP_BOXVIDEOGAIN"=131, "EXP_HSHADING_VALUE"=132, "EXP_VSHADING_VALUE"=133, "EXP_EDGEENHANCE_FLAG"=134, "EXP_SHADING_FLAG"=135, "EXP_GRAYSCALE"=136, "EXP_OFFSET"=137, "EXP_CCDGAIN"=138, "EXP_TEMPERATURE"=139, "EXP_MCPVOLTAGE"=140, "EXP_BOXEXPOSURE"=141, "EXP_ABC_FLAG"=142, "EXP_GAMMA_FLAG"=143, "EXP_AUTOBLACK_FLAG"=144, "EXP_AGC_FLAG"=145, "EXP_ODD_FIELD"=146, "EXP_FIELD_SELECT"=147, "EXP_RESET"=148, "EXP_EXTERN_ENABLE"=149, "EXP_CONTROLLERS_SUPPORTED"=150, "EXP_VTCLK"=151, "EXP_HTCLK"=152, "EXP_GATE_VS_CW"=153, "EXP_COM_PORT"=154, "EXP_US_UNITS"=156, "EXP_MS_UNITS"=157, "EXP_SEC_UNITS"=158, "EXP_MIN_UNITS"=159, "EXP_HRS_UNITS"=160, "EXP_FRAME_UNITS"=161, "EXP_SYNC_ASYNC"=162, "EXP_FOCUS_NFRAME"=163, "EXP_TIMEOUT"=164, "EXP_TIMEOUT_DEFAULT"=165, "EXP_HW_AUTOSTOP"=166, "EXP_RS170_INTEN_OFFSET"=167, "EXP_CONTROLLER_ALIVE"=168, "EXP_FOCUS_TYPE"=169, "EXP_FOCUS_ZOOM"=170, "EXP_FOCUS_PAN"=171, "EXP_MULTI_TAP_ROI"=172, "EXP_USE_INTERUPTS"=173, "EXP_DATA_ACQ_STATE"=174, "EXP_VERIFY_GOOD_VALUES"=175, "EXP_WHITE_CLAMP"=176, "EXP_BLACK_CLAMP"=177, "EXP_DELAY_TIME"=178, "EXP_READOUT_TIME"=179, "EXP_SW_DIAG"=180, "EXP_DIAG1"=181, "EXP_DIAG2"=182, "EXP_DIAG3"=183, "EXP_DIAG4"=184, "EXP_DIAG5"=185, "EXP_AorB_GROUP"=186, "EXP_ABSORBANCE_FLAG"=187, "EXP_ABSORBANCE_METHOD"=188, "EXP_ABSORBANCE_STRIPNUM"=189, "EXP_DMASIZE_VIA_DRIVER"=190, "EXP_DRIVERVERSION"=191, "EXP_NUM_DEVICES"=192, "EXP_ECPDMA_CHANNEL"=193, "EXP_CUSTOM_SHUTTER"=194, "EXP_ADC_OFFSET"=195, "EXP_CURRENT_READOUT_MODE"=196, "EXP_BANK_ADD"=197, "EXP_LUT_BANK"=198, "EXP_SETUP_STATUS"=201, "EXP_XY_GROUPING"=239, "EXP_MESSAGES_FLAG"=240, "EXP_TTL_LINE_TO_WAIT"=253, "EXP_DATA_COLLECTION_MODE"=258, "EXP_DATA_COLLECTION_TYPE"=262, "EXP_SKIPFRAMES"=274, "EXP_CLR_INT_CNTR"=276, "EXP_ENABLE_INT_CNTR"=277, "EXP_INT_CNTR"=278, "EXP_INTERNAL_SYNC_SRC"=279, "EXP_SW_EXTSYNC"=280, "EXP_PTG_PRESENT"=281, "EXP_ELEC_SHT"=282, "EXP_BOARDS_WITH_NVRAM"=283, "EXP_ANLGMASTER_ST143"=284, "EXP_ANLGSLAVE_ST143"=285, "EXP_DISPLAY_ST143"=286, "EXP_INTRFACE_ST143"=287, "EXP_SCANCONTROL_ST143"=288, "EXP_NUMBERFRAMES_IRQ"=204, "EXP_COOL_TYPE"=214, "EXP_HD_TYPE"=215, "EXP_INTENSIFER_GAIN"=216, "EXP_SHT_GATE_MODE"=217, "EXP_HD_CHECK"=218, "EXP_AMP_MODE"=219, "EXP_AMP_DIALOG"=247, "EXP_ANALOG_GAIN"=220, "EXP_HW_FIXES"=221, "EXP_PCI_CARDS"=222, "EXP_NOT_REVERSE"=223, "EXP_LOAD_NVRAM_DEFAULTS"=234, "EXP_CNTR_BRD"=235, "EXP_XDIMHW"=237, "EXP_YDIMHW"=238, "EXP_SPECIAL_FAST_RDOUT"=254, "EXP_SPCL_FAST_Y_DIM"=255, "EXP_SPCL_FAST_X_DIM"=256, "EXP_SPCL_FAST_Y_INDEX"=257, "EXP_SHUTTER_COMP_TIME_MS"=266, "EXP_NVRAM_AVAIL"=267, "EXP_NUMBER_AGAIN_AVAIL"=269, "EXP_SENSOR_TYPE"=270, "EXP_EVENT_TYPE"=292, "EXP_ANTI_BLOOMING"=293, "EXP_FAST_PULSE_ENABLE"=233, "EXP_USE_HEADCALIB"=296, "EXP_TEMP_STATUS"=301, "EXP_MULTIPLE_READMODES_LIVE"=302, "EXP_FIRST_ACQUIRE_FLAG"=303, "EXP_ANTI_BLOOMING_CONTROL"=304, "EXP_PRE_HORZ_DELAY"=305, "EXP_NVRAM_TRIES"=306, "EXP_XASCEND"=307, "EXP_YASCEND"=308, "EXP_ALT_TIMING"=309, "EXP_SHUTTER_PRE_COMP"=310, "EXP_PVCAM_POSSIBLE"=311, "EXP_ADC_IN_NVRAM"=312, "EXP_PASSTHRU_MODE"=313, "EXP_FIRMWAREVERSION"=314, "EXP_IMMEDIATE_SHUTTER"=315, "EXP_STAGE2_TEMP"=316, "EXP_AVGAIN_ENABLED"=317, "EXP_AVGAIN_SETPOINT"=318, "EXP_AVGAIN"=319, "EXP_AVGAIN_CALIB_TEMP"=320, "EXP_AVGAIN_CALIB_COEFF1"=321, "EXP_AVGAIN_CALIB_COEFF2"=322, "EXP_AVGAIN_CALIB_COEFF3"=323, "EXP_AVGAIN_CALIB_COEFF4"=324, "EXP_AVGAIN_CALIB_COEFF5"=325, "EXP_FORCE_READOUT_MODE"=326, "EXP_RESET_DATACOLLECTION"=327, "EXP_ACTIVE_SUBFRAME"=328, "EXP_PV_READOUT_PORT"=514, "EXP_COOLING_FAN_CTRL"=339, "EXP_SHTR_RES"=343, "EXP_PBC"=351, "EXP_PREEXP_CLEANS"=354, "EXP_TTL_CTRL"=355, "EXP_PAR_SHIFT_INDEX"=547, "EXP_LOGIC_OUTPUT_INVERT"=548, "EXP_CLASSNAME"=775, "EXP_FLATFLDNAME"=776, "EXP_DARKNAME"=777, "EXP_SETUPNAME"=778, "EXP_ACCESSNAME"=779, "EXP_DATFILENAME"=780, "EXP_ABSORBFILENAME"=781, "EXP_BLEMISHFILENAME"=782, "EXP_COSMICFILENAME"=783, "EXP_FILEINCBASENAME"=784, "EXP_YTNAME"=785, "EXP_DEVNAME"=786, "EXP_USEROI"=787, "EXP_DOBLEMISH"=788, "EXP_DOABSORB"=789, "EXP_DOCOSMIC"=790, "EXP_COSMICSENS"=791, "EXP_ABSORBSTRIP"=792, "EXP_DATATYPE"=793, "EXP_OVERWRITECONFIRM"=794, "EXP_FILEINCENABLE"=795, "EXP_FILEINCCOUNT"=796, "EXP_RUNNING"=797, "EXP_SAVEROPT"=798, "EXP_TIME_UNITS"=799, "EXP_FILEACCESS"=800, "EXP_AUTOSAVE"=801, "EXP_NEWWINDOW"=802, "EXP_XDIM"=803, "EXP_YDIM"=804, "EXP_XDIMDET"=805, "EXP_YDIMDET"=806, "EXP_ROIMODE"=807, "EXP_NUMREPEATSEXP"=808, "EXP_NUMACCUMSEXP"=809, "EXP_THREADSTATE"=810, "EXP_USEMINTHRESHOLDING"=811, "EXP_MINTHRESHOLDVALUE"=812, "EXP_USEMAXTHRESHOLDING"=813, "EXP_MAXTHRESHOLDVALUE"=814, "EXP_RUNNING_EXPERIMENT"=815, "EXP_THRESHOLD_DEMAND_UPDATE"=816, "EXP_ROICOUNT"=817, "EXP_ACCUMS"=818, "EXP_CACCUMS"=819, "EXP_CSEQUENTS"=820, "EXP_PHOTON_ESTIMATION_ENABLE"=821, "EXP_PHOTON_MAXTIME"=822, "EXP_PHOTON_MAXTIMEUNIT"=823, "EXP_CUSTOMFILTER_ENABLE"=824, "EXP_CUSTOMFILTER_SIZE"=825, "EXP_LOOKUPTABLE_ENABLE"=826, "EXP_BSHOWWINDOW"=827, "EXP_BBACKSUBTRACT"=828, "EXP_BDOFLATFIELD"=829, "EXP_ASCIIOUTPUTFILE"=830, "EXP_ASCIIOUTPUT_DELIMITER"=831, "EXP_ASCIIOUTPUT_TERMINATOR"=832, "EXP_FFTYPE"=833, "EXP_BGTYPE"=834, "EXP_COSGRASS"=835, "EXP_RUNASCONFIRM"=836, "EXP_RUNASRUNACCESS"=837, "EXP_DATAFILETYPE"=838, "EXP_ROTATE"=839, "EXP_FLIP"=840, "EXP_REVERSE"=841, "EXP_SWBINNING"=842, "EXP_AUTOSTORE"=843, "EXP_XBINNED"=844, "EXP_YBINNED"=845, "EXP_NUMPATTERNS"=846, "EXP_EXPERIMENTTIME"=847, "EXP_ASYNCSEQUENTIALS"=848, "EXP_SEQUENTIALS"=849, "EXP_CSEQUENTIALS"=850, "EXP_AUTOD"=851, "EXP_EXPOSURETIME"=852, "EXP_EXPOSURETIME_UNITS"=853, "EXP_ACQMODE"=854, "EXP_DMASIZE_PVCAM"=855, "EXP_INITIALIZE"=856, "EXP_CELL_X_SIZE"=857, "EXP_CELL_Y_SIZE"=858, "EXP_X_GAP_SIZE"=859, "EXP_Y_GAP_SIZE"=860] ("Param")
                w147 = 40 items=["EXP_ETACTUAL"=1, "EXP_SEQUENTS"=2, "EXP_ERROR"=3, "EXP_GETCAPS"=4, "EXP_GETPLSR"=5, "EXP_DETECTOR_BIT"=16, "EXP_RUNNING_APP"=23, "EXP_VIDEO_TYPE"=24, "EXP_CUSTOM_VIDEO_X"=25, "EXP_CUSTOM_VIDEO_Y"=26, "EXP_CUSTOM_VIDEO_FSTWIDTH"=27, "EXP_CUSTOM_VIDEO_LSTWIDTH"=28, "EXP_VIDEO_XDIM"=29, "EXP_VIDEO_YDIM"=30, "EXP_VIDEO_MAX_ZOOM"=31, "EXP_VIDEO_HORZ_PAN"=32, "EXP_VIDEO_VERT_PAN"=33, "EXP_WORD_MULTIPLIER"=34, "EXP_TARGET_ID"=35, "EXP_ADAPTER_ID"=36, "EXP_NUMADAPTORS"=37, "EXP_FORCE_PP_INIT"=38, "EXP_NOP_ADC"=39, "EXP_ACTUAL_TEMP"=40, "EXP_FORCE_AUTOSTOP"=41, "EXP_DEFAULT_VTCLK"=42, "EXP_MIN_VTCLK"=43, "EXP_MAX_VTCLK"=44, "EXP_DEFAULT_HTCLK"=45, "EXP_MIN_HTCLK"=46, "EXP_MAX_HTCLK"=47, "EXP_TIMING_STYLE"=48, "EXP_HEADSELECT"=49, "EXP_HORZPHASE"=50, "EXP_VERTPHASE"=51, "EXP_SPECIAL_SPEED"=52, "EXP_PRE_STRIPS"=53, "EXP_POST_STRIPS"=54, "EXP_PRE_LINES"=55, "EXP_POST_LINES"=56, "EXP_ACTIVE_LINES"=57, "EXP_ACTIVE_STRIPS"=58, "EXP_XFER_EXTRA"=59, "EXP_MIN_BLOCK"=60, "EXP_NUM_MIN_BLOCK"=61, "EXP_LOGIC_OUTPUT"=66, "EXP_VIDEO_BLANK"=67, "EXP_ZOOM_MODE_VIDEO"=68, "EXP_LEVEL_SYNC"=69, "EXP_DISABLE_LASER"=70, "EXP_ACQBACK_SHUTTER"=71, "EXP_ACQFLAT_SHUTTER"=72, "EXP_SMALL_CCD_MINEXP"=73, "EXP_LARGE_CCD_MINEXP"=74, "EXP_GATING_MODE"=75, "EXP_ILME_B1X"=76, "EXP_ILME_B2X"=77, "EXP_ILME_D1X"=78, "EXP_ILME_D2X"=79, "EXP_ILME_D4X"=80, "EXP_INIT_HW_ACCUM"=81, "EXP_5X_GAIN_ENABLE"=82, "EXP_RET_SRCCMP"=83, "EXP_EVENT_HANDLE"=84, "EXP_READOUT_MODE"=85, "EXP_SHUTTER_TYPE"=86, "EXP_USER_DEFINED_CHIP"=87, "EXP_USER_DEFINED_TIMING"=88, "EXP_CONTROLLER_VERSION"=89, "EXP_GET_CONTROLLER_VER"=90, "EXP_TTL_LINES"=91, "EXP_BIT_ADJUST"=92, "EXP_RESOLUTION"=93, "EXP_GAIN"=94, "EXP_ADC_RATE"=95, "EXP_ADC_TYPE"=96, "EXP_NUMBER_OF_CLEANS"=97, "EXP_NUM_OF_STRIPS_PER_CLN"=98, "EXP_INTERFACE_CARD"=99, "EXP_INTERRUPT"=100, "EXP_IO_ADDRESS1"=101, "EXP_IO_ADDRESS2"=102, "EXP_IO_ADDRESS3"=103, "EXP_HW_ROI"=104, "EXP_HW_BINNING"=105, "EXP_EDGE_TRIGGER"=106, "EXP_SHUTTER_CONTROL"=107, "EXP_RS170"=108, "EXP_RS170_COMPLEX"=109, "EXP_HW_RS170_LUT"=110, "EXP_RS170_INTENSITY_SCALING"=111, "EXP_RS170_OFFSET"=112, "EXP_RS170_PAN"=113, "EXP_RS170_ZOOM2X"=114, "EXP_RS170_ZOOM4X"=115, "EXP_RS170_BINNING"=116, "EXP_RS170_DECIMATION"=117, "EXP_HW_ACCUM"=118, "EXP_SHT_PREOPEN"=119, "EXP_STORE_STROBE"=120, "EXP_CONT_CLNS"=121, "EXP_TIMING_MODE"=122, "EXP_EXT_TRIGGER"=123, "EXP_EVENT_COUNTER"=124, "EXP_SW_TRIGGER"=125, "EXP_KINETICS_WINDOWSIZE"=126, "EXP_EXPOSURE"=127, "EXP_CONTROLLER_NAME"=128, "EXP_CCD_CHIP_NAME"=129, "EXP_BSWBINNING"=297, "EXP_EDGEENHANCE"=130, "EXP_BOXVIDEOGAIN"=131, "EXP_HSHADING_VALUE"=132, "EXP_VSHADING_VALUE"=133, "EXP_EDGEENHANCE_FLAG"=134, "EXP_SHADING_FLAG"=135, "EXP_GRAYSCALE"=136, "EXP_OFFSET"=137, "EXP_CCDGAIN"=138, "EXP_TEMPERATURE"=139, "EXP_MCPVOLTAGE"=140, "EXP_BOXEXPOSURE"=141, "EXP_ABC_FLAG"=142, "EXP_GAMMA_FLAG"=143, "EXP_AUTOBLACK_FLAG"=144, "EXP_AGC_FLAG"=145, "EXP_ODD_FIELD"=146, "EXP_FIELD_SELECT"=147, "EXP_RESET"=148, "EXP_EXTERN_ENABLE"=149, "EXP_CONTROLLERS_SUPPORTED"=150, "EXP_VTCLK"=151, "EXP_HTCLK"=152, "EXP_GATE_VS_CW"=153, "EXP_COM_PORT"=154, "EXP_US_UNITS"=156, "EXP_MS_UNITS"=157, "EXP_SEC_UNITS"=158, "EXP_MIN_UNITS"=159, "EXP_HRS_UNITS"=160, "EXP_FRAME_UNITS"=161, "EXP_SYNC_ASYNC"=162, "EXP_FOCUS_NFRAME"=163, "EXP_TIMEOUT"=164, "EXP_TIMEOUT_DEFAULT"=165, "EXP_HW_AUTOSTOP"=166, "EXP_RS170_INTEN_OFFSET"=167, "EXP_CONTROLLER_ALIVE"=168, "EXP_FOCUS_TYPE"=169, "EXP_FOCUS_ZOOM"=170, "EXP_FOCUS_PAN"=171, "EXP_MULTI_TAP_ROI"=172, "EXP_USE_INTERUPTS"=173, "EXP_DATA_ACQ_STATE"=174, "EXP_VERIFY_GOOD_VALUES"=175, "EXP_WHITE_CLAMP"=176, "EXP_BLACK_CLAMP"=177, "EXP_DELAY_TIME"=178, "EXP_READOUT_TIME"=179, "EXP_SW_DIAG"=180, "EXP_DIAG1"=181, "EXP_DIAG2"=182, "EXP_DIAG3"=183, "EXP_DIAG4"=184, "EXP_DIAG5"=185, "EXP_AorB_GROUP"=186, "EXP_ABSORBANCE_FLAG"=187, "EXP_ABSORBANCE_METHOD"=188, "EXP_ABSORBANCE_STRIPNUM"=189, "EXP_DMASIZE_VIA_DRIVER"=190, "EXP_DRIVERVERSION"=191, "EXP_NUM_DEVICES"=192, "EXP_ECPDMA_CHANNEL"=193, "EXP_CUSTOM_SHUTTER"=194, "EXP_ADC_OFFSET"=195, "EXP_CURRENT_READOUT_MODE"=196, "EXP_BANK_ADD"=197, "EXP_LUT_BANK"=198, "EXP_SETUP_STATUS"=201, "EXP_XY_GROUPING"=239, "EXP_MESSAGES_FLAG"=240, "EXP_TTL_LINE_TO_WAIT"=253, "EXP_DATA_COLLECTION_MODE"=258, "EXP_DATA_COLLECTION_TYPE"=262, "EXP_SKIPFRAMES"=274, "EXP_CLR_INT_CNTR"=276, "EXP_ENABLE_INT_CNTR"=277, "EXP_INT_CNTR"=278, "EXP_INTERNAL_SYNC_SRC"=279, "EXP_SW_EXTSYNC"=280, "EXP_PTG_PRESENT"=281, "EXP_ELEC_SHT"=282, "EXP_BOARDS_WITH_NVRAM"=283, "EXP_ANLGMASTER_ST143"=284, "EXP_ANLGSLAVE_ST143"=285, "EXP_DISPLAY_ST143"=286, "EXP_INTRFACE_ST143"=287, "EXP_SCANCONTROL_ST143"=288, "EXP_NUMBERFRAMES_IRQ"=204, "EXP_COOL_TYPE"=214, "EXP_HD_TYPE"=215, "EXP_INTENSIFER_GAIN"=216, "EXP_SHT_GATE_MODE"=217, "EXP_HD_CHECK"=218, "EXP_AMP_MODE"=219, "EXP_AMP_DIALOG"=247, "EXP_ANALOG_GAIN"=220, "EXP_HW_FIXES"=221, "EXP_PCI_CARDS"=222, "EXP_NOT_REVERSE"=223, "EXP_LOAD_NVRAM_DEFAULTS"=234, "EXP_CNTR_BRD"=235, "EXP_XDIMHW"=237, "EXP_YDIMHW"=238, "EXP_SPECIAL_FAST_RDOUT"=254, "EXP_SPCL_FAST_Y_DIM"=255, "EXP_SPCL_FAST_X_DIM"=256, "EXP_SPCL_FAST_Y_INDEX"=257, "EXP_SHUTTER_COMP_TIME_MS"=266, "EXP_NVRAM_AVAIL"=267, "EXP_NUMBER_AGAIN_AVAIL"=269, "EXP_SENSOR_TYPE"=270, "EXP_EVENT_TYPE"=292, "EXP_ANTI_BLOOMING"=293, "EXP_FAST_PULSE_ENABLE"=233, "EXP_USE_HEADCALIB"=296, "EXP_TEMP_STATUS"=301, "EXP_MULTIPLE_READMODES_LIVE"=302, "EXP_FIRST_ACQUIRE_FLAG"=303, "EXP_ANTI_BLOOMING_CONTROL"=304, "EXP_PRE_HORZ_DELAY"=305, "EXP_NVRAM_TRIES"=306, "EXP_XASCEND"=307, "EXP_YASCEND"=308, "EXP_ALT_TIMING"=309, "EXP_SHUTTER_PRE_COMP"=310, "EXP_PVCAM_POSSIBLE"=311, "EXP_ADC_IN_NVRAM"=312, "EXP_PASSTHRU_MODE"=313, "EXP_FIRMWAREVERSION"=314, "EXP_IMMEDIATE_SHUTTER"=315, "EXP_STAGE2_TEMP"=316, "EXP_AVGAIN_ENABLED"=317, "EXP_AVGAIN_SETPOINT"=318, "EXP_AVGAIN"=319, "EXP_AVGAIN_CALIB_TEMP"=320, "EXP_AVGAIN_CALIB_COEFF1"=321, "EXP_AVGAIN_CALIB_COEFF2"=322, "EXP_AVGAIN_CALIB_COEFF3"=323, "EXP_AVGAIN_CALIB_COEFF4"=324, "EXP_AVGAIN_CALIB_COEFF5"=325, "EXP_FORCE_READOUT_MODE"=326, "EXP_RESET_DATACOLLECTION"=327, "EXP_ACTIVE_SUBFRAME"=328, "EXP_PV_READOUT_PORT"=514, "EXP_COOLING_FAN_CTRL"=339, "EXP_SHTR_RES"=343, "EXP_PBC"=351, "EXP_PREEXP_CLEANS"=354, "EXP_TTL_CTRL"=355, "EXP_PAR_SHIFT_INDEX"=547, "EXP_LOGIC_OUTPUT_INVERT"=548, "EXP_CLASSNAME"=775, "EXP_FLATFLDNAME"=776, "EXP_DARKNAME"=777, "EXP_SETUPNAME"=778, "EXP_ACCESSNAME"=779, "EXP_DATFILENAME"=780, "EXP_ABSORBFILENAME"=781, "EXP_BLEMISHFILENAME"=782, "EXP_COSMICFILENAME"=783, "EXP_FILEINCBASENAME"=784, "EXP_YTNAME"=785, "EXP_DEVNAME"=786, "EXP_USEROI"=787, "EXP_DOBLEMISH"=788, "EXP_DOABSORB"=789, "EXP_DOCOSMIC"=790, "EXP_COSMICSENS"=791, "EXP_ABSORBSTRIP"=792, "EXP_DATATYPE"=793, "EXP_OVERWRITECONFIRM"=794, "EXP_FILEINCENABLE"=795, "EXP_FILEINCCOUNT"=796, "EXP_RUNNING"=797, "EXP_SAVEROPT"=798, "EXP_TIME_UNITS"=799, "EXP_FILEACCESS"=800, "EXP_AUTOSAVE"=801, "EXP_NEWWINDOW"=802, "EXP_XDIM"=803, "EXP_YDIM"=804, "EXP_XDIMDET"=805, "EXP_YDIMDET"=806, "EXP_ROIMODE"=807, "EXP_NUMREPEATSEXP"=808, "EXP_NUMACCUMSEXP"=809, "EXP_THREADSTATE"=810, "EXP_USEMINTHRESHOLDING"=811, "EXP_MINTHRESHOLDVALUE"=812, "EXP_USEMAXTHRESHOLDING"=813, "EXP_MAXTHRESHOLDVALUE"=814, "EXP_RUNNING_EXPERIMENT"=815, "EXP_THRESHOLD_DEMAND_UPDATE"=816, "EXP_ROICOUNT"=817, "EXP_ACCUMS"=818, "EXP_CACCUMS"=819, "EXP_CSEQUENTS"=820, "EXP_PHOTON_ESTIMATION_ENABLE"=821, "EXP_PHOTON_MAXTIME"=822, "EXP_PHOTON_MAXTIMEUNIT"=823, "EXP_CUSTOMFILTER_ENABLE"=824, "EXP_CUSTOMFILTER_SIZE"=825, "EXP_LOOKUPTABLE_ENABLE"=826, "EXP_BSHOWWINDOW"=827, "EXP_BBACKSUBTRACT"=828, "EXP_BDOFLATFIELD"=829, "EXP_ASCIIOUTPUTFILE"=830, "EXP_ASCIIOUTPUT_DELIMITER"=831, "EXP_ASCIIOUTPUT_TERMINATOR"=832, "EXP_FFTYPE"=833, "EXP_BGTYPE"=834, "EXP_COSGRASS"=835, "EXP_RUNASCONFIRM"=836, "EXP_RUNASRUNACCESS"=837, "EXP_DATAFILETYPE"=838, "EXP_ROTATE"=839, "EXP_FLIP"=840, "EXP_REVERSE"=841, "EXP_SWBINNING"=842, "EXP_AUTOSTORE"=843, "EXP_XBINNED"=844, "EXP_YBINNED"=845, "EXP_NUMPATTERNS"=846, "EXP_EXPERIMENTTIME"=847, "EXP_ASYNCSEQUENTIALS"=848, "EXP_SEQUENTIALS"=849, "EXP_CSEQUENTIALS"=850, "EXP_AUTOD"=851, "EXP_EXPOSURETIME"=852, "EXP_EXPOSURETIME_UNITS"=853, "EXP_ACQMODE"=854, "EXP_DMASIZE_PVCAM"=855, "EXP_INITIALIZE"=856, "EXP_CELL_X_SIZE"=857, "EXP_CELL_Y_SIZE"=858, "EXP_X_GAP_SIZE"=859, "EXP_Y_GAP_SIZE"=860] ("Param")
                w149 = 139 items=["EXP_ETACTUAL"=1, "EXP_SEQUENTS"=2, "EXP_ERROR"=3, "EXP_GETCAPS"=4, "EXP_GETPLSR"=5, "EXP_DETECTOR_BIT"=16, "EXP_RUNNING_APP"=23, "EXP_VIDEO_TYPE"=24, "EXP_CUSTOM_VIDEO_X"=25, "EXP_CUSTOM_VIDEO_Y"=26, "EXP_CUSTOM_VIDEO_FSTWIDTH"=27, "EXP_CUSTOM_VIDEO_LSTWIDTH"=28, "EXP_VIDEO_XDIM"=29, "EXP_VIDEO_YDIM"=30, "EXP_VIDEO_MAX_ZOOM"=31, "EXP_VIDEO_HORZ_PAN"=32, "EXP_VIDEO_VERT_PAN"=33, "EXP_WORD_MULTIPLIER"=34, "EXP_TARGET_ID"=35, "EXP_ADAPTER_ID"=36, "EXP_NUMADAPTORS"=37, "EXP_FORCE_PP_INIT"=38, "EXP_NOP_ADC"=39, "EXP_ACTUAL_TEMP"=40, "EXP_FORCE_AUTOSTOP"=41, "EXP_DEFAULT_VTCLK"=42, "EXP_MIN_VTCLK"=43, "EXP_MAX_VTCLK"=44, "EXP_DEFAULT_HTCLK"=45, "EXP_MIN_HTCLK"=46, "EXP_MAX_HTCLK"=47, "EXP_TIMING_STYLE"=48, "EXP_HEADSELECT"=49, "EXP_HORZPHASE"=50, "EXP_VERTPHASE"=51, "EXP_SPECIAL_SPEED"=52, "EXP_PRE_STRIPS"=53, "EXP_POST_STRIPS"=54, "EXP_PRE_LINES"=55, "EXP_POST_LINES"=56, "EXP_ACTIVE_LINES"=57, "EXP_ACTIVE_STRIPS"=58, "EXP_XFER_EXTRA"=59, "EXP_MIN_BLOCK"=60, "EXP_NUM_MIN_BLOCK"=61, "EXP_LOGIC_OUTPUT"=66, "EXP_VIDEO_BLANK"=67, "EXP_ZOOM_MODE_VIDEO"=68, "EXP_LEVEL_SYNC"=69, "EXP_DISABLE_LASER"=70, "EXP_ACQBACK_SHUTTER"=71, "EXP_ACQFLAT_SHUTTER"=72, "EXP_SMALL_CCD_MINEXP"=73, "EXP_LARGE_CCD_MINEXP"=74, "EXP_GATING_MODE"=75, "EXP_ILME_B1X"=76, "EXP_ILME_B2X"=77, "EXP_ILME_D1X"=78, "EXP_ILME_D2X"=79, "EXP_ILME_D4X"=80, "EXP_INIT_HW_ACCUM"=81, "EXP_5X_GAIN_ENABLE"=82, "EXP_RET_SRCCMP"=83, "EXP_EVENT_HANDLE"=84, "EXP_READOUT_MODE"=85, "EXP_SHUTTER_TYPE"=86, "EXP_USER_DEFINED_CHIP"=87, "EXP_USER_DEFINED_TIMING"=88, "EXP_CONTROLLER_VERSION"=89, "EXP_GET_CONTROLLER_VER"=90, "EXP_TTL_LINES"=91, "EXP_BIT_ADJUST"=92, "EXP_RESOLUTION"=93, "EXP_GAIN"=94, "EXP_ADC_RATE"=95, "EXP_ADC_TYPE"=96, "EXP_NUMBER_OF_CLEANS"=97, "EXP_NUM_OF_STRIPS_PER_CLN"=98, "EXP_INTERFACE_CARD"=99, "EXP_INTERRUPT"=100, "EXP_IO_ADDRESS1"=101, "EXP_IO_ADDRESS2"=102, "EXP_IO_ADDRESS3"=103, "EXP_HW_ROI"=104, "EXP_HW_BINNING"=105, "EXP_EDGE_TRIGGER"=106, "EXP_SHUTTER_CONTROL"=107, "EXP_RS170"=108, "EXP_RS170_COMPLEX"=109, "EXP_HW_RS170_LUT"=110, "EXP_RS170_INTENSITY_SCALING"=111, "EXP_RS170_OFFSET"=112, "EXP_RS170_PAN"=113, "EXP_RS170_ZOOM2X"=114, "EXP_RS170_ZOOM4X"=115, "EXP_RS170_BINNING"=116, "EXP_RS170_DECIMATION"=117, "EXP_HW_ACCUM"=118, "EXP_SHT_PREOPEN"=119, "EXP_STORE_STROBE"=120, "EXP_CONT_CLNS"=121, "EXP_TIMING_MODE"=122, "EXP_EXT_TRIGGER"=123, "EXP_EVENT_COUNTER"=124, "EXP_SW_TRIGGER"=125, "EXP_KINETICS_WINDOWSIZE"=126, "EXP_EXPOSURE"=127, "EXP_CONTROLLER_NAME"=128, "EXP_CCD_CHIP_NAME"=129, "EXP_BSWBINNING"=297, "EXP_EDGEENHANCE"=130, "EXP_BOXVIDEOGAIN"=131, "EXP_HSHADING_VALUE"=132, "EXP_VSHADING_VALUE"=133, "EXP_EDGEENHANCE_FLAG"=134, "EXP_SHADING_FLAG"=135, "EXP_GRAYSCALE"=136, "EXP_OFFSET"=137, "EXP_CCDGAIN"=138, "EXP_TEMPERATURE"=139, "EXP_MCPVOLTAGE"=140, "EXP_BOXEXPOSURE"=141, "EXP_ABC_FLAG"=142, "EXP_GAMMA_FLAG"=143, "EXP_AUTOBLACK_FLAG"=144, "EXP_AGC_FLAG"=145, "EXP_ODD_FIELD"=146, "EXP_FIELD_SELECT"=147, "EXP_RESET"=148, "EXP_EXTERN_ENABLE"=149, "EXP_CONTROLLERS_SUPPORTED"=150, "EXP_VTCLK"=151, "EXP_HTCLK"=152, "EXP_GATE_VS_CW"=153, "EXP_COM_PORT"=154, "EXP_US_UNITS"=156, "EXP_MS_UNITS"=157, "EXP_SEC_UNITS"=158, "EXP_MIN_UNITS"=159, "EXP_HRS_UNITS"=160, "EXP_FRAME_UNITS"=161, "EXP_SYNC_ASYNC"=162, "EXP_FOCUS_NFRAME"=163, "EXP_TIMEOUT"=164, "EXP_TIMEOUT_DEFAULT"=165, "EXP_HW_AUTOSTOP"=166, "EXP_RS170_INTEN_OFFSET"=167, "EXP_CONTROLLER_ALIVE"=168, "EXP_FOCUS_TYPE"=169, "EXP_FOCUS_ZOOM"=170, "EXP_FOCUS_PAN"=171, "EXP_MULTI_TAP_ROI"=172, "EXP_USE_INTERUPTS"=173, "EXP_DATA_ACQ_STATE"=174, "EXP_VERIFY_GOOD_VALUES"=175, "EXP_WHITE_CLAMP"=176, "EXP_BLACK_CLAMP"=177, "EXP_DELAY_TIME"=178, "EXP_READOUT_TIME"=179, "EXP_SW_DIAG"=180, "EXP_DIAG1"=181, "EXP_DIAG2"=182, "EXP_DIAG3"=183, "EXP_DIAG4"=184, "EXP_DIAG5"=185, "EXP_AorB_GROUP"=186, "EXP_ABSORBANCE_FLAG"=187, "EXP_ABSORBANCE_METHOD"=188, "EXP_ABSORBANCE_STRIPNUM"=189, "EXP_DMASIZE_VIA_DRIVER"=190, "EXP_DRIVERVERSION"=191, "EXP_NUM_DEVICES"=192, "EXP_ECPDMA_CHANNEL"=193, "EXP_CUSTOM_SHUTTER"=194, "EXP_ADC_OFFSET"=195, "EXP_CURRENT_READOUT_MODE"=196, "EXP_BANK_ADD"=197, "EXP_LUT_BANK"=198, "EXP_SETUP_STATUS"=201, "EXP_XY_GROUPING"=239, "EXP_MESSAGES_FLAG"=240, "EXP_TTL_LINE_TO_WAIT"=253, "EXP_DATA_COLLECTION_MODE"=258, "EXP_DATA_COLLECTION_TYPE"=262, "EXP_SKIPFRAMES"=274, "EXP_CLR_INT_CNTR"=276, "EXP_ENABLE_INT_CNTR"=277, "EXP_INT_CNTR"=278, "EXP_INTERNAL_SYNC_SRC"=279, "EXP_SW_EXTSYNC"=280, "EXP_PTG_PRESENT"=281, "EXP_ELEC_SHT"=282, "EXP_BOARDS_WITH_NVRAM"=283, "EXP_ANLGMASTER_ST143"=284, "EXP_ANLGSLAVE_ST143"=285, "EXP_DISPLAY_ST143"=286, "EXP_INTRFACE_ST143"=287, "EXP_SCANCONTROL_ST143"=288, "EXP_NUMBERFRAMES_IRQ"=204, "EXP_COOL_TYPE"=214, "EXP_HD_TYPE"=215, "EXP_INTENSIFER_GAIN"=216, "EXP_SHT_GATE_MODE"=217, "EXP_HD_CHECK"=218, "EXP_AMP_MODE"=219, "EXP_AMP_DIALOG"=247, "EXP_ANALOG_GAIN"=220, "EXP_HW_FIXES"=221, "EXP_PCI_CARDS"=222, "EXP_NOT_REVERSE"=223, "EXP_LOAD_NVRAM_DEFAULTS"=234, "EXP_CNTR_BRD"=235, "EXP_XDIMHW"=237, "EXP_YDIMHW"=238, "EXP_SPECIAL_FAST_RDOUT"=254, "EXP_SPCL_FAST_Y_DIM"=255, "EXP_SPCL_FAST_X_DIM"=256, "EXP_SPCL_FAST_Y_INDEX"=257, "EXP_SHUTTER_COMP_TIME_MS"=266, "EXP_NVRAM_AVAIL"=267, "EXP_NUMBER_AGAIN_AVAIL"=269, "EXP_SENSOR_TYPE"=270, "EXP_EVENT_TYPE"=292, "EXP_ANTI_BLOOMING"=293, "EXP_FAST_PULSE_ENABLE"=233, "EXP_USE_HEADCALIB"=296, "EXP_TEMP_STATUS"=301, "EXP_MULTIPLE_READMODES_LIVE"=302, "EXP_FIRST_ACQUIRE_FLAG"=303, "EXP_ANTI_BLOOMING_CONTROL"=304, "EXP_PRE_HORZ_DELAY"=305, "EXP_NVRAM_TRIES"=306, "EXP_XASCEND"=307, "EXP_YASCEND"=308, "EXP_ALT_TIMING"=309, "EXP_SHUTTER_PRE_COMP"=310, "EXP_PVCAM_POSSIBLE"=311, "EXP_ADC_IN_NVRAM"=312, "EXP_PASSTHRU_MODE"=313, "EXP_FIRMWAREVERSION"=314, "EXP_IMMEDIATE_SHUTTER"=315, "EXP_STAGE2_TEMP"=316, "EXP_AVGAIN_ENABLED"=317, "EXP_AVGAIN_SETPOINT"=318, "EXP_AVGAIN"=319, "EXP_AVGAIN_CALIB_TEMP"=320, "EXP_AVGAIN_CALIB_COEFF1"=321, "EXP_AVGAIN_CALIB_COEFF2"=322, "EXP_AVGAIN_CALIB_COEFF3"=323, "EXP_AVGAIN_CALIB_COEFF4"=324, "EXP_AVGAIN_CALIB_COEFF5"=325, "EXP_FORCE_READOUT_MODE"=326, "EXP_RESET_DATACOLLECTION"=327, "EXP_ACTIVE_SUBFRAME"=328, "EXP_PV_READOUT_PORT"=514, "EXP_COOLING_FAN_CTRL"=339, "EXP_SHTR_RES"=343, "EXP_PBC"=351, "EXP_PREEXP_CLEANS"=354, "EXP_TTL_CTRL"=355, "EXP_PAR_SHIFT_INDEX"=547, "EXP_LOGIC_OUTPUT_INVERT"=548, "EXP_CLASSNAME"=775, "EXP_FLATFLDNAME"=776, "EXP_DARKNAME"=777, "EXP_SETUPNAME"=778, "EXP_ACCESSNAME"=779, "EXP_DATFILENAME"=780, "EXP_ABSORBFILENAME"=781, "EXP_BLEMISHFILENAME"=782, "EXP_COSMICFILENAME"=783, "EXP_FILEINCBASENAME"=784, "EXP_YTNAME"=785, "EXP_DEVNAME"=786, "EXP_USEROI"=787, "EXP_DOBLEMISH"=788, "EXP_DOABSORB"=789, "EXP_DOCOSMIC"=790, "EXP_COSMICSENS"=791, "EXP_ABSORBSTRIP"=792, "EXP_DATATYPE"=793, "EXP_OVERWRITECONFIRM"=794, "EXP_FILEINCENABLE"=795, "EXP_FILEINCCOUNT"=796, "EXP_RUNNING"=797, "EXP_SAVEROPT"=798, "EXP_TIME_UNITS"=799, "EXP_FILEACCESS"=800, "EXP_AUTOSAVE"=801, "EXP_NEWWINDOW"=802, "EXP_XDIM"=803, "EXP_YDIM"=804, "EXP_XDIMDET"=805, "EXP_YDIMDET"=806, "EXP_ROIMODE"=807, "EXP_NUMREPEATSEXP"=808, "EXP_NUMACCUMSEXP"=809, "EXP_THREADSTATE"=810, "EXP_USEMINTHRESHOLDING"=811, "EXP_MINTHRESHOLDVALUE"=812, "EXP_USEMAXTHRESHOLDING"=813, "EXP_MAXTHRESHOLDVALUE"=814, "EXP_RUNNING_EXPERIMENT"=815, "EXP_THRESHOLD_DEMAND_UPDATE"=816, "EXP_ROICOUNT"=817, "EXP_ACCUMS"=818, "EXP_CACCUMS"=819, "EXP_CSEQUENTS"=820, "EXP_PHOTON_ESTIMATION_ENABLE"=821, "EXP_PHOTON_MAXTIME"=822, "EXP_PHOTON_MAXTIMEUNIT"=823, "EXP_CUSTOMFILTER_ENABLE"=824, "EXP_CUSTOMFILTER_SIZE"=825, "EXP_LOOKUPTABLE_ENABLE"=826, "EXP_BSHOWWINDOW"=827, "EXP_BBACKSUBTRACT"=828, "EXP_BDOFLATFIELD"=829, "EXP_ASCIIOUTPUTFILE"=830, "EXP_ASCIIOUTPUT_DELIMITER"=831, "EXP_ASCIIOUTPUT_TERMINATOR"=832, "EXP_FFTYPE"=833, "EXP_BGTYPE"=834, "EXP_COSGRASS"=835, "EXP_RUNASCONFIRM"=836, "EXP_RUNASRUNACCESS"=837, "EXP_DATAFILETYPE"=838, "EXP_ROTATE"=839, "EXP_FLIP"=840, "EXP_REVERSE"=841, "EXP_SWBINNING"=842, "EXP_AUTOSTORE"=843, "EXP_XBINNED"=844, "EXP_YBINNED"=845, "EXP_NUMPATTERNS"=846, "EXP_EXPERIMENTTIME"=847, "EXP_ASYNCSEQUENTIALS"=848, "EXP_SEQUENTIALS"=849, "EXP_CSEQUENTIALS"=850, "EXP_AUTOD"=851, "EXP_EXPOSURETIME"=852, "EXP_EXPOSURETIME_UNITS"=853, "EXP_ACQMODE"=854, "EXP_DMASIZE_PVCAM"=855, "EXP_INITIALIZE"=856, "EXP_CELL_X_SIZE"=857, "EXP_CELL_Y_SIZE"=858, "EXP_X_GAP_SIZE"=859, "EXP_Y_GAP_SIZE"=860] ("Param")
                w152 = 94 items=["EXP_ETACTUAL"=1, "EXP_SEQUENTS"=2, "EXP_ERROR"=3, "EXP_GETCAPS"=4, "EXP_GETPLSR"=5, "EXP_DETECTOR_BIT"=16, "EXP_RUNNING_APP"=23, "EXP_VIDEO_TYPE"=24, "EXP_CUSTOM_VIDEO_X"=25, "EXP_CUSTOM_VIDEO_Y"=26, "EXP_CUSTOM_VIDEO_FSTWIDTH"=27, "EXP_CUSTOM_VIDEO_LSTWIDTH"=28, "EXP_VIDEO_XDIM"=29, "EXP_VIDEO_YDIM"=30, "EXP_VIDEO_MAX_ZOOM"=31, "EXP_VIDEO_HORZ_PAN"=32, "EXP_VIDEO_VERT_PAN"=33, "EXP_WORD_MULTIPLIER"=34, "EXP_TARGET_ID"=35, "EXP_ADAPTER_ID"=36, "EXP_NUMADAPTORS"=37, "EXP_FORCE_PP_INIT"=38, "EXP_NOP_ADC"=39, "EXP_ACTUAL_TEMP"=40, "EXP_FORCE_AUTOSTOP"=41, "EXP_DEFAULT_VTCLK"=42, "EXP_MIN_VTCLK"=43, "EXP_MAX_VTCLK"=44, "EXP_DEFAULT_HTCLK"=45, "EXP_MIN_HTCLK"=46, "EXP_MAX_HTCLK"=47, "EXP_TIMING_STYLE"=48, "EXP_HEADSELECT"=49, "EXP_HORZPHASE"=50, "EXP_VERTPHASE"=51, "EXP_SPECIAL_SPEED"=52, "EXP_PRE_STRIPS"=53, "EXP_POST_STRIPS"=54, "EXP_PRE_LINES"=55, "EXP_POST_LINES"=56, "EXP_ACTIVE_LINES"=57, "EXP_ACTIVE_STRIPS"=58, "EXP_XFER_EXTRA"=59, "EXP_MIN_BLOCK"=60, "EXP_NUM_MIN_BLOCK"=61, "EXP_LOGIC_OUTPUT"=66, "EXP_VIDEO_BLANK"=67, "EXP_ZOOM_MODE_VIDEO"=68, "EXP_LEVEL_SYNC"=69, "EXP_DISABLE_LASER"=70, "EXP_ACQBACK_SHUTTER"=71, "EXP_ACQFLAT_SHUTTER"=72, "EXP_SMALL_CCD_MINEXP"=73, "EXP_LARGE_CCD_MINEXP"=74, "EXP_GATING_MODE"=75, "EXP_ILME_B1X"=76, "EXP_ILME_B2X"=77, "EXP_ILME_D1X"=78, "EXP_ILME_D2X"=79, "EXP_ILME_D4X"=80, "EXP_INIT_HW_ACCUM"=81, "EXP_5X_GAIN_ENABLE"=82, "EXP_RET_SRCCMP"=83, "EXP_EVENT_HANDLE"=84, "EXP_READOUT_MODE"=85, "EXP_SHUTTER_TYPE"=86, "EXP_USER_DEFINED_CHIP"=87, "EXP_USER_DEFINED_TIMING"=88, "EXP_CONTROLLER_VERSION"=89, "EXP_GET_CONTROLLER_VER"=90, "EXP_TTL_LINES"=91, "EXP_BIT_ADJUST"=92, "EXP_RESOLUTION"=93, "EXP_GAIN"=94, "EXP_ADC_RATE"=95, "EXP_ADC_TYPE"=96, "EXP_NUMBER_OF_CLEANS"=97, "EXP_NUM_OF_STRIPS_PER_CLN"=98, "EXP_INTERFACE_CARD"=99, "EXP_INTERRUPT"=100, "EXP_IO_ADDRESS1"=101, "EXP_IO_ADDRESS2"=102, "EXP_IO_ADDRESS3"=103, "EXP_HW_ROI"=104, "EXP_HW_BINNING"=105, "EXP_EDGE_TRIGGER"=106, "EXP_SHUTTER_CONTROL"=107, "EXP_RS170"=108, "EXP_RS170_COMPLEX"=109, "EXP_HW_RS170_LUT"=110, "EXP_RS170_INTENSITY_SCALING"=111, "EXP_RS170_OFFSET"=112, "EXP_RS170_PAN"=113, "EXP_RS170_ZOOM2X"=114, "EXP_RS170_ZOOM4X"=115, "EXP_RS170_BINNING"=116, "EXP_RS170_DECIMATION"=117, "EXP_HW_ACCUM"=118, "EXP_SHT_PREOPEN"=119, "EXP_STORE_STROBE"=120, "EXP_CONT_CLNS"=121, "EXP_TIMING_MODE"=122, "EXP_EXT_TRIGGER"=123, "EXP_EVENT_COUNTER"=124, "EXP_SW_TRIGGER"=125, "EXP_KINETICS_WINDOWSIZE"=126, "EXP_EXPOSURE"=127, "EXP_CONTROLLER_NAME"=128, "EXP_CCD_CHIP_NAME"=129, "EXP_BSWBINNING"=297, "EXP_EDGEENHANCE"=130, "EXP_BOXVIDEOGAIN"=131, "EXP_HSHADING_VALUE"=132, "EXP_VSHADING_VALUE"=133, "EXP_EDGEENHANCE_FLAG"=134, "EXP_SHADING_FLAG"=135, "EXP_GRAYSCALE"=136, "EXP_OFFSET"=137, "EXP_CCDGAIN"=138, "EXP_TEMPERATURE"=139, "EXP_MCPVOLTAGE"=140, "EXP_BOXEXPOSURE"=141, "EXP_ABC_FLAG"=142, "EXP_GAMMA_FLAG"=143, "EXP_AUTOBLACK_FLAG"=144, "EXP_AGC_FLAG"=145, "EXP_ODD_FIELD"=146, "EXP_FIELD_SELECT"=147, "EXP_RESET"=148, "EXP_EXTERN_ENABLE"=149, "EXP_CONTROLLERS_SUPPORTED"=150, "EXP_VTCLK"=151, "EXP_HTCLK"=152, "EXP_GATE_VS_CW"=153, "EXP_COM_PORT"=154, "EXP_US_UNITS"=156, "EXP_MS_UNITS"=157, "EXP_SEC_UNITS"=158, "EXP_MIN_UNITS"=159, "EXP_HRS_UNITS"=160, "EXP_FRAME_UNITS"=161, "EXP_SYNC_ASYNC"=162, "EXP_FOCUS_NFRAME"=163, "EXP_TIMEOUT"=164, "EXP_TIMEOUT_DEFAULT"=165, "EXP_HW_AUTOSTOP"=166, "EXP_RS170_INTEN_OFFSET"=167, "EXP_CONTROLLER_ALIVE"=168, "EXP_FOCUS_TYPE"=169, "EXP_FOCUS_ZOOM"=170, "EXP_FOCUS_PAN"=171, "EXP_MULTI_TAP_ROI"=172, "EXP_USE_INTERUPTS"=173, "EXP_DATA_ACQ_STATE"=174, "EXP_VERIFY_GOOD_VALUES"=175, "EXP_WHITE_CLAMP"=176, "EXP_BLACK_CLAMP"=177, "EXP_DELAY_TIME"=178, "EXP_READOUT_TIME"=179, "EXP_SW_DIAG"=180, "EXP_DIAG1"=181, "EXP_DIAG2"=182, "EXP_DIAG3"=183, "EXP_DIAG4"=184, "EXP_DIAG5"=185, "EXP_AorB_GROUP"=186, "EXP_ABSORBANCE_FLAG"=187, "EXP_ABSORBANCE_METHOD"=188, "EXP_ABSORBANCE_STRIPNUM"=189, "EXP_DMASIZE_VIA_DRIVER"=190, "EXP_DRIVERVERSION"=191, "EXP_NUM_DEVICES"=192, "EXP_ECPDMA_CHANNEL"=193, "EXP_CUSTOM_SHUTTER"=194, "EXP_ADC_OFFSET"=195, "EXP_CURRENT_READOUT_MODE"=196, "EXP_BANK_ADD"=197, "EXP_LUT_BANK"=198, "EXP_SETUP_STATUS"=201, "EXP_XY_GROUPING"=239, "EXP_MESSAGES_FLAG"=240, "EXP_TTL_LINE_TO_WAIT"=253, "EXP_DATA_COLLECTION_MODE"=258, "EXP_DATA_COLLECTION_TYPE"=262, "EXP_SKIPFRAMES"=274, "EXP_CLR_INT_CNTR"=276, "EXP_ENABLE_INT_CNTR"=277, "EXP_INT_CNTR"=278, "EXP_INTERNAL_SYNC_SRC"=279, "EXP_SW_EXTSYNC"=280, "EXP_PTG_PRESENT"=281, "EXP_ELEC_SHT"=282, "EXP_BOARDS_WITH_NVRAM"=283, "EXP_ANLGMASTER_ST143"=284, "EXP_ANLGSLAVE_ST143"=285, "EXP_DISPLAY_ST143"=286, "EXP_INTRFACE_ST143"=287, "EXP_SCANCONTROL_ST143"=288, "EXP_NUMBERFRAMES_IRQ"=204, "EXP_COOL_TYPE"=214, "EXP_HD_TYPE"=215, "EXP_INTENSIFER_GAIN"=216, "EXP_SHT_GATE_MODE"=217, "EXP_HD_CHECK"=218, "EXP_AMP_MODE"=219, "EXP_AMP_DIALOG"=247, "EXP_ANALOG_GAIN"=220, "EXP_HW_FIXES"=221, "EXP_PCI_CARDS"=222, "EXP_NOT_REVERSE"=223, "EXP_LOAD_NVRAM_DEFAULTS"=234, "EXP_CNTR_BRD"=235, "EXP_XDIMHW"=237, "EXP_YDIMHW"=238, "EXP_SPECIAL_FAST_RDOUT"=254, "EXP_SPCL_FAST_Y_DIM"=255, "EXP_SPCL_FAST_X_DIM"=256, "EXP_SPCL_FAST_Y_INDEX"=257, "EXP_SHUTTER_COMP_TIME_MS"=266, "EXP_NVRAM_AVAIL"=267, "EXP_NUMBER_AGAIN_AVAIL"=269, "EXP_SENSOR_TYPE"=270, "EXP_EVENT_TYPE"=292, "EXP_ANTI_BLOOMING"=293, "EXP_FAST_PULSE_ENABLE"=233, "EXP_USE_HEADCALIB"=296, "EXP_TEMP_STATUS"=301, "EXP_MULTIPLE_READMODES_LIVE"=302, "EXP_FIRST_ACQUIRE_FLAG"=303, "EXP_ANTI_BLOOMING_CONTROL"=304, "EXP_PRE_HORZ_DELAY"=305, "EXP_NVRAM_TRIES"=306, "EXP_XASCEND"=307, "EXP_YASCEND"=308, "EXP_ALT_TIMING"=309, "EXP_SHUTTER_PRE_COMP"=310, "EXP_PVCAM_POSSIBLE"=311, "EXP_ADC_IN_NVRAM"=312, "EXP_PASSTHRU_MODE"=313, "EXP_FIRMWAREVERSION"=314, "EXP_IMMEDIATE_SHUTTER"=315, "EXP_STAGE2_TEMP"=316, "EXP_AVGAIN_ENABLED"=317, "EXP_AVGAIN_SETPOINT"=318, "EXP_AVGAIN"=319, "EXP_AVGAIN_CALIB_TEMP"=320, "EXP_AVGAIN_CALIB_COEFF1"=321, "EXP_AVGAIN_CALIB_COEFF2"=322, "EXP_AVGAIN_CALIB_COEFF3"=323, "EXP_AVGAIN_CALIB_COEFF4"=324, "EXP_AVGAIN_CALIB_COEFF5"=325, "EXP_FORCE_READOUT_MODE"=326, "EXP_RESET_DATACOLLECTION"=327, "EXP_ACTIVE_SUBFRAME"=328, "EXP_PV_READOUT_PORT"=514, "EXP_COOLING_FAN_CTRL"=339, "EXP_SHTR_RES"=343, "EXP_PBC"=351, "EXP_PREEXP_CLEANS"=354, "EXP_TTL_CTRL"=355, "EXP_PAR_SHIFT_INDEX"=547, "EXP_LOGIC_OUTPUT_INVERT"=548, "EXP_CLASSNAME"=775, "EXP_FLATFLDNAME"=776, "EXP_DARKNAME"=777, "EXP_SETUPNAME"=778, "EXP_ACCESSNAME"=779, "EXP_DATFILENAME"=780, "EXP_ABSORBFILENAME"=781, "EXP_BLEMISHFILENAME"=782, "EXP_COSMICFILENAME"=783, "EXP_FILEINCBASENAME"=784, "EXP_YTNAME"=785, "EXP_DEVNAME"=786, "EXP_USEROI"=787, "EXP_DOBLEMISH"=788, "EXP_DOABSORB"=789, "EXP_DOCOSMIC"=790, "EXP_COSMICSENS"=791, "EXP_ABSORBSTRIP"=792, "EXP_DATATYPE"=793, "EXP_OVERWRITECONFIRM"=794, "EXP_FILEINCENABLE"=795, "EXP_FILEINCCOUNT"=796, "EXP_RUNNING"=797, "EXP_SAVEROPT"=798, "EXP_TIME_UNITS"=799, "EXP_FILEACCESS"=800, "EXP_AUTOSAVE"=801, "EXP_NEWWINDOW"=802, "EXP_XDIM"=803, "EXP_YDIM"=804, "EXP_XDIMDET"=805, "EXP_YDIMDET"=806, "EXP_ROIMODE"=807, "EXP_NUMREPEATSEXP"=808, "EXP_NUMACCUMSEXP"=809, "EXP_THREADSTATE"=810, "EXP_USEMINTHRESHOLDING"=811, "EXP_MINTHRESHOLDVALUE"=812, "EXP_USEMAXTHRESHOLDING"=813, "EXP_MAXTHRESHOLDVALUE"=814, "EXP_RUNNING_EXPERIMENT"=815, "EXP_THRESHOLD_DEMAND_UPDATE"=816, "EXP_ROICOUNT"=817, "EXP_ACCUMS"=818, "EXP_CACCUMS"=819, "EXP_CSEQUENTS"=820, "EXP_PHOTON_ESTIMATION_ENABLE"=821, "EXP_PHOTON_MAXTIME"=822, "EXP_PHOTON_MAXTIMEUNIT"=823, "EXP_CUSTOMFILTER_ENABLE"=824, "EXP_CUSTOMFILTER_SIZE"=825, "EXP_LOOKUPTABLE_ENABLE"=826, "EXP_BSHOWWINDOW"=827, "EXP_BBACKSUBTRACT"=828, "EXP_BDOFLATFIELD"=829, "EXP_ASCIIOUTPUTFILE"=830, "EXP_ASCIIOUTPUT_DELIMITER"=831, "EXP_ASCIIOUTPUT_TERMINATOR"=832, "EXP_FFTYPE"=833, "EXP_BGTYPE"=834, "EXP_COSGRASS"=835, "EXP_RUNASCONFIRM"=836, "EXP_RUNASRUNACCESS"=837, "EXP_DATAFILETYPE"=838, "EXP_ROTATE"=839, "EXP_FLIP"=840, "EXP_REVERSE"=841, "EXP_SWBINNING"=842, "EXP_AUTOSTORE"=843, "EXP_XBINNED"=844, "EXP_YBINNED"=845, "EXP_NUMPATTERNS"=846, "EXP_EXPERIMENTTIME"=847, "EXP_ASYNCSEQUENTIALS"=848, "EXP_SEQUENTIALS"=849, "EXP_CSEQUENTIALS"=850, "EXP_AUTOD"=851, "EXP_EXPOSURETIME"=852, "EXP_EXPOSURETIME_UNITS"=853, "EXP_ACQMODE"=854, "EXP_DMASIZE_PVCAM"=855, "EXP_INITIALIZE"=856, "EXP_CELL_X_SIZE"=857, "EXP_CELL_Y_SIZE"=858, "EXP_X_GAP_SIZE"=859, "EXP_Y_GAP_SIZE"=860] ("Param")
                w154 = 1
                w160 = 780 items=["EXP_ETACTUAL"=1, "EXP_SEQUENTS"=2, "EXP_ERROR"=3, "EXP_GETCAPS"=4, "EXP_GETPLSR"=5, "EXP_DETECTOR_BIT"=16, "EXP_RUNNING_APP"=23, "EXP_VIDEO_TYPE"=24, "EXP_CUSTOM_VIDEO_X"=25, "EXP_CUSTOM_VIDEO_Y"=26, "EXP_CUSTOM_VIDEO_FSTWIDTH"=27, "EXP_CUSTOM_VIDEO_LSTWIDTH"=28, "EXP_VIDEO_XDIM"=29, "EXP_VIDEO_YDIM"=30, "EXP_VIDEO_MAX_ZOOM"=31, "EXP_VIDEO_HORZ_PAN"=32, "EXP_VIDEO_VERT_PAN"=33, "EXP_WORD_MULTIPLIER"=34, "EXP_TARGET_ID"=35, "EXP_ADAPTER_ID"=36, "EXP_NUMADAPTORS"=37, "EXP_FORCE_PP_INIT"=38, "EXP_NOP_ADC"=39, "EXP_ACTUAL_TEMP"=40, "EXP_FORCE_AUTOSTOP"=41, "EXP_DEFAULT_VTCLK"=42, "EXP_MIN_VTCLK"=43, "EXP_MAX_VTCLK"=44, "EXP_DEFAULT_HTCLK"=45, "EXP_MIN_HTCLK"=46, "EXP_MAX_HTCLK"=47, "EXP_TIMING_STYLE"=48, "EXP_HEADSELECT"=49, "EXP_HORZPHASE"=50, "EXP_VERTPHASE"=51, "EXP_SPECIAL_SPEED"=52, "EXP_PRE_STRIPS"=53, "EXP_POST_STRIPS"=54, "EXP_PRE_LINES"=55, "EXP_POST_LINES"=56, "EXP_ACTIVE_LINES"=57, "EXP_ACTIVE_STRIPS"=58, "EXP_XFER_EXTRA"=59, "EXP_MIN_BLOCK"=60, "EXP_NUM_MIN_BLOCK"=61, "EXP_LOGIC_OUTPUT"=66, "EXP_VIDEO_BLANK"=67, "EXP_ZOOM_MODE_VIDEO"=68, "EXP_LEVEL_SYNC"=69, "EXP_DISABLE_LASER"=70, "EXP_ACQBACK_SHUTTER"=71, "EXP_ACQFLAT_SHUTTER"=72, "EXP_SMALL_CCD_MINEXP"=73, "EXP_LARGE_CCD_MINEXP"=74, "EXP_GATING_MODE"=75, "EXP_ILME_B1X"=76, "EXP_ILME_B2X"=77, "EXP_ILME_D1X"=78, "EXP_ILME_D2X"=79, "EXP_ILME_D4X"=80, "EXP_INIT_HW_ACCUM"=81, "EXP_5X_GAIN_ENABLE"=82, "EXP_RET_SRCCMP"=83, "EXP_EVENT_HANDLE"=84, "EXP_READOUT_MODE"=85, "EXP_SHUTTER_TYPE"=86, "EXP_USER_DEFINED_CHIP"=87, "EXP_USER_DEFINED_TIMING"=88, "EXP_CONTROLLER_VERSION"=89, "EXP_GET_CONTROLLER_VER"=90, "EXP_TTL_LINES"=91, "EXP_BIT_ADJUST"=92, "EXP_RESOLUTION"=93, "EXP_GAIN"=94, "EXP_ADC_RATE"=95, "EXP_ADC_TYPE"=96, "EXP_NUMBER_OF_CLEANS"=97, "EXP_NUM_OF_STRIPS_PER_CLN"=98, "EXP_INTERFACE_CARD"=99, "EXP_INTERRUPT"=100, "EXP_IO_ADDRESS1"=101, "EXP_IO_ADDRESS2"=102, "EXP_IO_ADDRESS3"=103, "EXP_HW_ROI"=104, "EXP_HW_BINNING"=105, "EXP_EDGE_TRIGGER"=106, "EXP_SHUTTER_CONTROL"=107, "EXP_RS170"=108, "EXP_RS170_COMPLEX"=109, "EXP_HW_RS170_LUT"=110, "EXP_RS170_INTENSITY_SCALING"=111, "EXP_RS170_OFFSET"=112, "EXP_RS170_PAN"=113, "EXP_RS170_ZOOM2X"=114, "EXP_RS170_ZOOM4X"=115, "EXP_RS170_BINNING"=116, "EXP_RS170_DECIMATION"=117, "EXP_HW_ACCUM"=118, "EXP_SHT_PREOPEN"=119, "EXP_STORE_STROBE"=120, "EXP_CONT_CLNS"=121, "EXP_TIMING_MODE"=122, "EXP_EXT_TRIGGER"=123, "EXP_EVENT_COUNTER"=124, "EXP_SW_TRIGGER"=125, "EXP_KINETICS_WINDOWSIZE"=126, "EXP_EXPOSURE"=127, "EXP_CONTROLLER_NAME"=128, "EXP_CCD_CHIP_NAME"=129, "EXP_BSWBINNING"=297, "EXP_EDGEENHANCE"=130, "EXP_BOXVIDEOGAIN"=131, "EXP_HSHADING_VALUE"=132, "EXP_VSHADING_VALUE"=133, "EXP_EDGEENHANCE_FLAG"=134, "EXP_SHADING_FLAG"=135, "EXP_GRAYSCALE"=136, "EXP_OFFSET"=137, "EXP_CCDGAIN"=138, "EXP_TEMPERATURE"=139, "EXP_MCPVOLTAGE"=140, "EXP_BOXEXPOSURE"=141, "EXP_ABC_FLAG"=142, "EXP_GAMMA_FLAG"=143, "EXP_AUTOBLACK_FLAG"=144, "EXP_AGC_FLAG"=145, "EXP_ODD_FIELD"=146, "EXP_FIELD_SELECT"=147, "EXP_RESET"=148, "EXP_EXTERN_ENABLE"=149, "EXP_CONTROLLERS_SUPPORTED"=150, "EXP_VTCLK"=151, "EXP_HTCLK"=152, "EXP_GATE_VS_CW"=153, "EXP_COM_PORT"=154, "EXP_US_UNITS"=156, "EXP_MS_UNITS"=157, "EXP_SEC_UNITS"=158, "EXP_MIN_UNITS"=159, "EXP_HRS_UNITS"=160, "EXP_FRAME_UNITS"=161, "EXP_SYNC_ASYNC"=162, "EXP_FOCUS_NFRAME"=163, "EXP_TIMEOUT"=164, "EXP_TIMEOUT_DEFAULT"=165, "EXP_HW_AUTOSTOP"=166, "EXP_RS170_INTEN_OFFSET"=167, "EXP_CONTROLLER_ALIVE"=168, "EXP_FOCUS_TYPE"=169, "EXP_FOCUS_ZOOM"=170, "EXP_FOCUS_PAN"=171, "EXP_MULTI_TAP_ROI"=172, "EXP_USE_INTERUPTS"=173, "EXP_DATA_ACQ_STATE"=174, "EXP_VERIFY_GOOD_VALUES"=175, "EXP_WHITE_CLAMP"=176, "EXP_BLACK_CLAMP"=177, "EXP_DELAY_TIME"=178, "EXP_READOUT_TIME"=179, "EXP_SW_DIAG"=180, "EXP_DIAG1"=181, "EXP_DIAG2"=182, "EXP_DIAG3"=183, "EXP_DIAG4"=184, "EXP_DIAG5"=185, "EXP_AorB_GROUP"=186, "EXP_ABSORBANCE_FLAG"=187, "EXP_ABSORBANCE_METHOD"=188, "EXP_ABSORBANCE_STRIPNUM"=189, "EXP_DMASIZE_VIA_DRIVER"=190, "EXP_DRIVERVERSION"=191, "EXP_NUM_DEVICES"=192, "EXP_ECPDMA_CHANNEL"=193, "EXP_CUSTOM_SHUTTER"=194, "EXP_ADC_OFFSET"=195, "EXP_CURRENT_READOUT_MODE"=196, "EXP_BANK_ADD"=197, "EXP_LUT_BANK"=198, "EXP_SETUP_STATUS"=201, "EXP_XY_GROUPING"=239, "EXP_MESSAGES_FLAG"=240, "EXP_TTL_LINE_TO_WAIT"=253, "EXP_DATA_COLLECTION_MODE"=258, "EXP_DATA_COLLECTION_TYPE"=262, "EXP_SKIPFRAMES"=274, "EXP_CLR_INT_CNTR"=276, "EXP_ENABLE_INT_CNTR"=277, "EXP_INT_CNTR"=278, "EXP_INTERNAL_SYNC_SRC"=279, "EXP_SW_EXTSYNC"=280, "EXP_PTG_PRESENT"=281, "EXP_ELEC_SHT"=282, "EXP_BOARDS_WITH_NVRAM"=283, "EXP_ANLGMASTER_ST143"=284, "EXP_ANLGSLAVE_ST143"=285, "EXP_DISPLAY_ST143"=286, "EXP_INTRFACE_ST143"=287, "EXP_SCANCONTROL_ST143"=288, "EXP_NUMBERFRAMES_IRQ"=204, "EXP_COOL_TYPE"=214, "EXP_HD_TYPE"=215, "EXP_INTENSIFER_GAIN"=216, "EXP_SHT_GATE_MODE"=217, "EXP_HD_CHECK"=218, "EXP_AMP_MODE"=219, "EXP_AMP_DIALOG"=247, "EXP_ANALOG_GAIN"=220, "EXP_HW_FIXES"=221, "EXP_PCI_CARDS"=222, "EXP_NOT_REVERSE"=223, "EXP_LOAD_NVRAM_DEFAULTS"=234, "EXP_CNTR_BRD"=235, "EXP_XDIMHW"=237, "EXP_YDIMHW"=238, "EXP_SPECIAL_FAST_RDOUT"=254, "EXP_SPCL_FAST_Y_DIM"=255, "EXP_SPCL_FAST_X_DIM"=256, "EXP_SPCL_FAST_Y_INDEX"=257, "EXP_SHUTTER_COMP_TIME_MS"=266, "EXP_NVRAM_AVAIL"=267, "EXP_NUMBER_AGAIN_AVAIL"=269, "EXP_SENSOR_TYPE"=270, "EXP_EVENT_TYPE"=292, "EXP_ANTI_BLOOMING"=293, "EXP_FAST_PULSE_ENABLE"=233, "EXP_USE_HEADCALIB"=296, "EXP_TEMP_STATUS"=301, "EXP_MULTIPLE_READMODES_LIVE"=302, "EXP_FIRST_ACQUIRE_FLAG"=303, "EXP_ANTI_BLOOMING_CONTROL"=304, "EXP_PRE_HORZ_DELAY"=305, "EXP_NVRAM_TRIES"=306, "EXP_XASCEND"=307, "EXP_YASCEND"=308, "EXP_ALT_TIMING"=309, "EXP_SHUTTER_PRE_COMP"=310, "EXP_PVCAM_POSSIBLE"=311, "EXP_ADC_IN_NVRAM"=312, "EXP_PASSTHRU_MODE"=313, "EXP_FIRMWAREVERSION"=314, "EXP_IMMEDIATE_SHUTTER"=315, "EXP_STAGE2_TEMP"=316, "EXP_AVGAIN_ENABLED"=317, "EXP_AVGAIN_SETPOINT"=318, "EXP_AVGAIN"=319, "EXP_AVGAIN_CALIB_TEMP"=320, "EXP_AVGAIN_CALIB_COEFF1"=321, "EXP_AVGAIN_CALIB_COEFF2"=322, "EXP_AVGAIN_CALIB_COEFF3"=323, "EXP_AVGAIN_CALIB_COEFF4"=324, "EXP_AVGAIN_CALIB_COEFF5"=325, "EXP_FORCE_READOUT_MODE"=326, "EXP_RESET_DATACOLLECTION"=327, "EXP_ACTIVE_SUBFRAME"=328, "EXP_PV_READOUT_PORT"=514, "EXP_CLASSNAME"=775, "EXP_FLATFLDNAME"=776, "EXP_DARKNAME"=777, "EXP_SETUPNAME"=778, "EXP_ACCESSNAME"=779, "EXP_DATFILENAME"=780, "EXP_ABSORBFILENAME"=781, "EXP_BLEMISHFILENAME"=782, "EXP_COSMICFILENAME"=783, "EXP_FILEINCBASENAME"=784, "EXP_YTNAME"=785, "EXP_DEVNAME"=786, "EXP_USEROI"=787, "EXP_DOBLEMISH"=788, "EXP_DOABSORB"=789, "EXP_DOCOSMIC"=790, "EXP_COSMICSENS"=791, "EXP_ABSORBSTRIP"=792, "EXP_DATATYPE"=793, "EXP_OVERWRITECONFIRM"=794, "EXP_FILEINCENABLE"=795, "EXP_FILEINCCOUNT"=796, "EXP_RUNNING"=797, "EXP_SAVEROPT"=798, "EXP_TIME_UNITS"=799, "EXP_FILEACCESS"=800, "EXP_AUTOSAVE"=801, "EXP_NEWWINDOW"=802, "EXP_XDIM"=803, "EXP_YDIM"=804, "EXP_XDIMDET"=805, "EXP_YDIMDET"=806, "EXP_ROIMODE"=807, "EXP_NUMREPEATSEXP"=808, "EXP_NUMACCUMSEXP"=809, "EXP_THREADSTATE"=810, "EXP_USEMINTHRESHOLDING"=811, "EXP_MINTHRESHOLDVALUE"=812, "EXP_USEMAXTHRESHOLDING"=813, "EXP_MAXTHRESHOLDVALUE"=814, "EXP_RUNNING_EXPERIMENT"=815, "EXP_THRESHOLD_DEMAND_UPDATE"=816, "EXP_ROICOUNT"=817, "EXP_ACCUMS"=818, "EXP_CACCUMS"=819, "EXP_CSEQUENTS"=820, "EXP_PHOTON_ESTIMATION_ENABLE"=821, "EXP_PHOTON_MAXTIME"=822, "EXP_PHOTON_MAXTIMEUNIT"=823, "EXP_CUSTOMFILTER_ENABLE"=824, "EXP_CUSTOMFILTER_SIZE"=825, "EXP_LOOKUPTABLE_ENABLE"=826, "EXP_BSHOWWINDOW"=827, "EXP_BBACKSUBTRACT"=828, "EXP_BDOFLATFIELD"=829, "EXP_ASCIIOUTPUTFILE"=830, "EXP_ASCIIOUTPUT_DELIMITER"=831, "EXP_ASCIIOUTPUT_TERMINATOR"=832, "EXP_FFTYPE"=833, "EXP_BGTYPE"=834, "EXP_COSGRASS"=835, "EXP_RUNASCONFIRM"=836, "EXP_RUNASRUNACCESS"=837, "EXP_DATAFILETYPE"=838, "EXP_ROTATE"=839, "EXP_FLIP"=840, "EXP_REVERSE"=841, "EXP_SWBINNING"=842, "EXP_AUTOSTORE"=843, "EXP_XBINNED"=844, "EXP_YBINNED"=845, "EXP_NUMPATTERNS"=846, "EXP_EXPERIMENTTIME"=847, "EXP_ASYNCSEQUENTIALS"=848, "EXP_SEQUENTIALS"=849, "EXP_CSEQUENTIALS"=850, "EXP_AUTOD"=851, "EXP_EXPOSURETIME"=852, "EXP_EXPOSURETIME_UNITS"=853, "EXP_ACQMODE"=854, "EXP_DMASIZE_PVCAM"=855, "EXP_INITIALIZE"=856, "EXP_CELL_X_SIZE"=857, "EXP_CELL_Y_SIZE"=858, "EXP_X_GAP_SIZE"=859, "EXP_Y_GAP_SIZE"=860] ("Param")
                w161 = 818 items=["EXP_ETACTUAL"=1, "EXP_SEQUENTS"=2, "EXP_ERROR"=3, "EXP_GETCAPS"=4, "EXP_GETPLSR"=5, "EXP_DETECTOR_BIT"=16, "EXP_RUNNING_APP"=23, "EXP_VIDEO_TYPE"=24, "EXP_CUSTOM_VIDEO_X"=25, "EXP_CUSTOM_VIDEO_Y"=26, "EXP_CUSTOM_VIDEO_FSTWIDTH"=27, "EXP_CUSTOM_VIDEO_LSTWIDTH"=28, "EXP_VIDEO_XDIM"=29, "EXP_VIDEO_YDIM"=30, "EXP_VIDEO_MAX_ZOOM"=31, "EXP_VIDEO_HORZ_PAN"=32, "EXP_VIDEO_VERT_PAN"=33, "EXP_WORD_MULTIPLIER"=34, "EXP_TARGET_ID"=35, "EXP_ADAPTER_ID"=36, "EXP_NUMADAPTORS"=37, "EXP_FORCE_PP_INIT"=38, "EXP_NOP_ADC"=39, "EXP_ACTUAL_TEMP"=40, "EXP_FORCE_AUTOSTOP"=41, "EXP_DEFAULT_VTCLK"=42, "EXP_MIN_VTCLK"=43, "EXP_MAX_VTCLK"=44, "EXP_DEFAULT_HTCLK"=45, "EXP_MIN_HTCLK"=46, "EXP_MAX_HTCLK"=47, "EXP_TIMING_STYLE"=48, "EXP_HEADSELECT"=49, "EXP_HORZPHASE"=50, "EXP_VERTPHASE"=51, "EXP_SPECIAL_SPEED"=52, "EXP_PRE_STRIPS"=53, "EXP_POST_STRIPS"=54, "EXP_PRE_LINES"=55, "EXP_POST_LINES"=56, "EXP_ACTIVE_LINES"=57, "EXP_ACTIVE_STRIPS"=58, "EXP_XFER_EXTRA"=59, "EXP_MIN_BLOCK"=60, "EXP_NUM_MIN_BLOCK"=61, "EXP_LOGIC_OUTPUT"=66, "EXP_VIDEO_BLANK"=67, "EXP_ZOOM_MODE_VIDEO"=68, "EXP_LEVEL_SYNC"=69, "EXP_DISABLE_LASER"=70, "EXP_ACQBACK_SHUTTER"=71, "EXP_ACQFLAT_SHUTTER"=72, "EXP_SMALL_CCD_MINEXP"=73, "EXP_LARGE_CCD_MINEXP"=74, "EXP_GATING_MODE"=75, "EXP_ILME_B1X"=76, "EXP_ILME_B2X"=77, "EXP_ILME_D1X"=78, "EXP_ILME_D2X"=79, "EXP_ILME_D4X"=80, "EXP_INIT_HW_ACCUM"=81, "EXP_5X_GAIN_ENABLE"=82, "EXP_RET_SRCCMP"=83, "EXP_EVENT_HANDLE"=84, "EXP_READOUT_MODE"=85, "EXP_SHUTTER_TYPE"=86, "EXP_USER_DEFINED_CHIP"=87, "EXP_USER_DEFINED_TIMING"=88, "EXP_CONTROLLER_VERSION"=89, "EXP_GET_CONTROLLER_VER"=90, "EXP_TTL_LINES"=91, "EXP_BIT_ADJUST"=92, "EXP_RESOLUTION"=93, "EXP_GAIN"=94, "EXP_ADC_RATE"=95, "EXP_ADC_TYPE"=96, "EXP_NUMBER_OF_CLEANS"=97, "EXP_NUM_OF_STRIPS_PER_CLN"=98, "EXP_INTERFACE_CARD"=99, "EXP_INTERRUPT"=100, "EXP_IO_ADDRESS1"=101, "EXP_IO_ADDRESS2"=102, "EXP_IO_ADDRESS3"=103, "EXP_HW_ROI"=104, "EXP_HW_BINNING"=105, "EXP_EDGE_TRIGGER"=106, "EXP_SHUTTER_CONTROL"=107, "EXP_RS170"=108, "EXP_RS170_COMPLEX"=109, "EXP_HW_RS170_LUT"=110, "EXP_RS170_INTENSITY_SCALING"=111, "EXP_RS170_OFFSET"=112, "EXP_RS170_PAN"=113, "EXP_RS170_ZOOM2X"=114, "EXP_RS170_ZOOM4X"=115, "EXP_RS170_BINNING"=116, "EXP_RS170_DECIMATION"=117, "EXP_HW_ACCUM"=118, "EXP_SHT_PREOPEN"=119, "EXP_STORE_STROBE"=120, "EXP_CONT_CLNS"=121, "EXP_TIMING_MODE"=122, "EXP_EXT_TRIGGER"=123, "EXP_EVENT_COUNTER"=124, "EXP_SW_TRIGGER"=125, "EXP_KINETICS_WINDOWSIZE"=126, "EXP_EXPOSURE"=127, "EXP_CONTROLLER_NAME"=128, "EXP_CCD_CHIP_NAME"=129, "EXP_BSWBINNING"=297, "EXP_EDGEENHANCE"=130, "EXP_BOXVIDEOGAIN"=131, "EXP_HSHADING_VALUE"=132, "EXP_VSHADING_VALUE"=133, "EXP_EDGEENHANCE_FLAG"=134, "EXP_SHADING_FLAG"=135, "EXP_GRAYSCALE"=136, "EXP_OFFSET"=137, "EXP_CCDGAIN"=138, "EXP_TEMPERATURE"=139, "EXP_MCPVOLTAGE"=140, "EXP_BOXEXPOSURE"=141, "EXP_ABC_FLAG"=142, "EXP_GAMMA_FLAG"=143, "EXP_AUTOBLACK_FLAG"=144, "EXP_AGC_FLAG"=145, "EXP_ODD_FIELD"=146, "EXP_FIELD_SELECT"=147, "EXP_RESET"=148, "EXP_EXTERN_ENABLE"=149, "EXP_CONTROLLERS_SUPPORTED"=150, "EXP_VTCLK"=151, "EXP_HTCLK"=152, "EXP_GATE_VS_CW"=153, "EXP_COM_PORT"=154, "EXP_US_UNITS"=156, "EXP_MS_UNITS"=157, "EXP_SEC_UNITS"=158, "EXP_MIN_UNITS"=159, "EXP_HRS_UNITS"=160, "EXP_FRAME_UNITS"=161, "EXP_SYNC_ASYNC"=162, "EXP_FOCUS_NFRAME"=163, "EXP_TIMEOUT"=164, "EXP_TIMEOUT_DEFAULT"=165, "EXP_HW_AUTOSTOP"=166, "EXP_RS170_INTEN_OFFSET"=167, "EXP_CONTROLLER_ALIVE"=168, "EXP_FOCUS_TYPE"=169, "EXP_FOCUS_ZOOM"=170, "EXP_FOCUS_PAN"=171, "EXP_MULTI_TAP_ROI"=172, "EXP_USE_INTERUPTS"=173, "EXP_DATA_ACQ_STATE"=174, "EXP_VERIFY_GOOD_VALUES"=175, "EXP_WHITE_CLAMP"=176, "EXP_BLACK_CLAMP"=177, "EXP_DELAY_TIME"=178, "EXP_READOUT_TIME"=179, "EXP_SW_DIAG"=180, "EXP_DIAG1"=181, "EXP_DIAG2"=182, "EXP_DIAG3"=183, "EXP_DIAG4"=184, "EXP_DIAG5"=185, "EXP_AorB_GROUP"=186, "EXP_ABSORBANCE_FLAG"=187, "EXP_ABSORBANCE_METHOD"=188, "EXP_ABSORBANCE_STRIPNUM"=189, "EXP_DMASIZE_VIA_DRIVER"=190, "EXP_DRIVERVERSION"=191, "EXP_NUM_DEVICES"=192, "EXP_ECPDMA_CHANNEL"=193, "EXP_CUSTOM_SHUTTER"=194, "EXP_ADC_OFFSET"=195, "EXP_CURRENT_READOUT_MODE"=196, "EXP_BANK_ADD"=197, "EXP_LUT_BANK"=198, "EXP_SETUP_STATUS"=201, "EXP_XY_GROUPING"=239, "EXP_MESSAGES_FLAG"=240, "EXP_TTL_LINE_TO_WAIT"=253, "EXP_DATA_COLLECTION_MODE"=258, "EXP_DATA_COLLECTION_TYPE"=262, "EXP_SKIPFRAMES"=274, "EXP_CLR_INT_CNTR"=276, "EXP_ENABLE_INT_CNTR"=277, "EXP_INT_CNTR"=278, "EXP_INTERNAL_SYNC_SRC"=279, "EXP_SW_EXTSYNC"=280, "EXP_PTG_PRESENT"=281, "EXP_ELEC_SHT"=282, "EXP_BOARDS_WITH_NVRAM"=283, "EXP_ANLGMASTER_ST143"=284, "EXP_ANLGSLAVE_ST143"=285, "EXP_DISPLAY_ST143"=286, "EXP_INTRFACE_ST143"=287, "EXP_SCANCONTROL_ST143"=288, "EXP_NUMBERFRAMES_IRQ"=204, "EXP_COOL_TYPE"=214, "EXP_HD_TYPE"=215, "EXP_INTENSIFER_GAIN"=216, "EXP_SHT_GATE_MODE"=217, "EXP_HD_CHECK"=218, "EXP_AMP_MODE"=219, "EXP_AMP_DIALOG"=247, "EXP_ANALOG_GAIN"=220, "EXP_HW_FIXES"=221, "EXP_PCI_CARDS"=222, "EXP_NOT_REVERSE"=223, "EXP_LOAD_NVRAM_DEFAULTS"=234, "EXP_CNTR_BRD"=235, "EXP_XDIMHW"=237, "EXP_YDIMHW"=238, "EXP_SPECIAL_FAST_RDOUT"=254, "EXP_SPCL_FAST_Y_DIM"=255, "EXP_SPCL_FAST_X_DIM"=256, "EXP_SPCL_FAST_Y_INDEX"=257, "EXP_SHUTTER_COMP_TIME_MS"=266, "EXP_NVRAM_AVAIL"=267, "EXP_NUMBER_AGAIN_AVAIL"=269, "EXP_SENSOR_TYPE"=270, "EXP_EVENT_TYPE"=292, "EXP_ANTI_BLOOMING"=293, "EXP_FAST_PULSE_ENABLE"=233, "EXP_USE_HEADCALIB"=296, "EXP_TEMP_STATUS"=301, "EXP_MULTIPLE_READMODES_LIVE"=302, "EXP_FIRST_ACQUIRE_FLAG"=303, "EXP_ANTI_BLOOMING_CONTROL"=304, "EXP_PRE_HORZ_DELAY"=305, "EXP_NVRAM_TRIES"=306, "EXP_XASCEND"=307, "EXP_YASCEND"=308, "EXP_ALT_TIMING"=309, "EXP_SHUTTER_PRE_COMP"=310, "EXP_PVCAM_POSSIBLE"=311, "EXP_ADC_IN_NVRAM"=312, "EXP_PASSTHRU_MODE"=313, "EXP_FIRMWAREVERSION"=314, "EXP_IMMEDIATE_SHUTTER"=315, "EXP_STAGE2_TEMP"=316, "EXP_AVGAIN_ENABLED"=317, "EXP_AVGAIN_SETPOINT"=318, "EXP_AVGAIN"=319, "EXP_AVGAIN_CALIB_TEMP"=320, "EXP_AVGAIN_CALIB_COEFF1"=321, "EXP_AVGAIN_CALIB_COEFF2"=322, "EXP_AVGAIN_CALIB_COEFF3"=323, "EXP_AVGAIN_CALIB_COEFF4"=324, "EXP_AVGAIN_CALIB_COEFF5"=325, "EXP_FORCE_READOUT_MODE"=326, "EXP_RESET_DATACOLLECTION"=327, "EXP_ACTIVE_SUBFRAME"=328, "EXP_PV_READOUT_PORT"=514, "EXP_CLASSNAME"=775, "EXP_FLATFLDNAME"=776, "EXP_DARKNAME"=777, "EXP_SETUPNAME"=778, "EXP_ACCESSNAME"=779, "EXP_DATFILENAME"=780, "EXP_ABSORBFILENAME"=781, "EXP_BLEMISHFILENAME"=782, "EXP_COSMICFILENAME"=783, "EXP_FILEINCBASENAME"=784, "EXP_YTNAME"=785, "EXP_DEVNAME"=786, "EXP_USEROI"=787, "EXP_DOBLEMISH"=788, "EXP_DOABSORB"=789, "EXP_DOCOSMIC"=790, "EXP_COSMICSENS"=791, "EXP_ABSORBSTRIP"=792, "EXP_DATATYPE"=793, "EXP_OVERWRITECONFIRM"=794, "EXP_FILEINCENABLE"=795, "EXP_FILEINCCOUNT"=796, "EXP_RUNNING"=797, "EXP_SAVEROPT"=798, "EXP_TIME_UNITS"=799, "EXP_FILEACCESS"=800, "EXP_AUTOSAVE"=801, "EXP_NEWWINDOW"=802, "EXP_XDIM"=803, "EXP_YDIM"=804, "EXP_XDIMDET"=805, "EXP_YDIMDET"=806, "EXP_ROIMODE"=807, "EXP_NUMREPEATSEXP"=808, "EXP_NUMACCUMSEXP"=809, "EXP_THREADSTATE"=810, "EXP_USEMINTHRESHOLDING"=811, "EXP_MINTHRESHOLDVALUE"=812, "EXP_USEMAXTHRESHOLDING"=813, "EXP_MAXTHRESHOLDVALUE"=814, "EXP_RUNNING_EXPERIMENT"=815, "EXP_THRESHOLD_DEMAND_UPDATE"=816, "EXP_ROICOUNT"=817, "EXP_ACCUMS"=818, "EXP_CACCUMS"=819, "EXP_CSEQUENTS"=820, "EXP_PHOTON_ESTIMATION_ENABLE"=821, "EXP_PHOTON_MAXTIME"=822, "EXP_PHOTON_MAXTIMEUNIT"=823, "EXP_CUSTOMFILTER_ENABLE"=824, "EXP_CUSTOMFILTER_SIZE"=825, "EXP_LOOKUPTABLE_ENABLE"=826, "EXP_BSHOWWINDOW"=827, "EXP_BBACKSUBTRACT"=828, "EXP_BDOFLATFIELD"=829, "EXP_ASCIIOUTPUTFILE"=830, "EXP_ASCIIOUTPUT_DELIMITER"=831, "EXP_ASCIIOUTPUT_TERMINATOR"=832, "EXP_FFTYPE"=833, "EXP_BGTYPE"=834, "EXP_COSGRASS"=835, "EXP_RUNASCONFIRM"=836, "EXP_RUNASRUNACCESS"=837, "EXP_DATAFILETYPE"=838, "EXP_ROTATE"=839, "EXP_FLIP"=840, "EXP_REVERSE"=841, "EXP_SWBINNING"=842, "EXP_AUTOSTORE"=843, "EXP_XBINNED"=844, "EXP_YBINNED"=845, "EXP_NUMPATTERNS"=846, "EXP_EXPERIMENTTIME"=847, "EXP_ASYNCSEQUENTIALS"=848, "EXP_SEQUENTIALS"=849, "EXP_CSEQUENTIALS"=850, "EXP_AUTOD"=851, "EXP_EXPOSURETIME"=852, "EXP_EXPOSURETIME_UNITS"=853, "EXP_ACQMODE"=854, "EXP_DMASIZE_PVCAM"=855, "EXP_INITIALIZE"=856, "EXP_CELL_X_SIZE"=857, "EXP_CELL_Y_SIZE"=858, "EXP_X_GAP_SIZE"=859, "EXP_Y_GAP_SIZE"=860] ("Param")
                w162 = 2 items=["EXP_ETACTUAL"=1, "EXP_SEQUENTS"=2, "EXP_ERROR"=3, "EXP_GETCAPS"=4, "EXP_GETPLSR"=5, "EXP_DETECTOR_BIT"=16, "EXP_RUNNING_APP"=23, "EXP_VIDEO_TYPE"=24, "EXP_CUSTOM_VIDEO_X"=25, "EXP_CUSTOM_VIDEO_Y"=26, "EXP_CUSTOM_VIDEO_FSTWIDTH"=27, "EXP_CUSTOM_VIDEO_LSTWIDTH"=28, "EXP_VIDEO_XDIM"=29, "EXP_VIDEO_YDIM"=30, "EXP_VIDEO_MAX_ZOOM"=31, "EXP_VIDEO_HORZ_PAN"=32, "EXP_VIDEO_VERT_PAN"=33, "EXP_WORD_MULTIPLIER"=34, "EXP_TARGET_ID"=35, "EXP_ADAPTER_ID"=36, "EXP_NUMADAPTORS"=37, "EXP_FORCE_PP_INIT"=38, "EXP_NOP_ADC"=39, "EXP_ACTUAL_TEMP"=40, "EXP_FORCE_AUTOSTOP"=41, "EXP_DEFAULT_VTCLK"=42, "EXP_MIN_VTCLK"=43, "EXP_MAX_VTCLK"=44, "EXP_DEFAULT_HTCLK"=45, "EXP_MIN_HTCLK"=46, "EXP_MAX_HTCLK"=47, "EXP_TIMING_STYLE"=48, "EXP_HEADSELECT"=49, "EXP_HORZPHASE"=50, "EXP_VERTPHASE"=51, "EXP_SPECIAL_SPEED"=52, "EXP_PRE_STRIPS"=53, "EXP_POST_STRIPS"=54, "EXP_PRE_LINES"=55, "EXP_POST_LINES"=56, "EXP_ACTIVE_LINES"=57, "EXP_ACTIVE_STRIPS"=58, "EXP_XFER_EXTRA"=59, "EXP_MIN_BLOCK"=60, "EXP_NUM_MIN_BLOCK"=61, "EXP_LOGIC_OUTPUT"=66, "EXP_VIDEO_BLANK"=67, "EXP_ZOOM_MODE_VIDEO"=68, "EXP_LEVEL_SYNC"=69, "EXP_DISABLE_LASER"=70, "EXP_ACQBACK_SHUTTER"=71, "EXP_ACQFLAT_SHUTTER"=72, "EXP_SMALL_CCD_MINEXP"=73, "EXP_LARGE_CCD_MINEXP"=74, "EXP_GATING_MODE"=75, "EXP_ILME_B1X"=76, "EXP_ILME_B2X"=77, "EXP_ILME_D1X"=78, "EXP_ILME_D2X"=79, "EXP_ILME_D4X"=80, "EXP_INIT_HW_ACCUM"=81, "EXP_5X_GAIN_ENABLE"=82, "EXP_RET_SRCCMP"=83, "EXP_EVENT_HANDLE"=84, "EXP_READOUT_MODE"=85, "EXP_SHUTTER_TYPE"=86, "EXP_USER_DEFINED_CHIP"=87, "EXP_USER_DEFINED_TIMING"=88, "EXP_CONTROLLER_VERSION"=89, "EXP_GET_CONTROLLER_VER"=90, "EXP_TTL_LINES"=91, "EXP_BIT_ADJUST"=92, "EXP_RESOLUTION"=93, "EXP_GAIN"=94, "EXP_ADC_RATE"=95, "EXP_ADC_TYPE"=96, "EXP_NUMBER_OF_CLEANS"=97, "EXP_NUM_OF_STRIPS_PER_CLN"=98, "EXP_INTERFACE_CARD"=99, "EXP_INTERRUPT"=100, "EXP_IO_ADDRESS1"=101, "EXP_IO_ADDRESS2"=102, "EXP_IO_ADDRESS3"=103, "EXP_HW_ROI"=104, "EXP_HW_BINNING"=105, "EXP_EDGE_TRIGGER"=106, "EXP_SHUTTER_CONTROL"=107, "EXP_RS170"=108, "EXP_RS170_COMPLEX"=109, "EXP_HW_RS170_LUT"=110, "EXP_RS170_INTENSITY_SCALING"=111, "EXP_RS170_OFFSET"=112, "EXP_RS170_PAN"=113, "EXP_RS170_ZOOM2X"=114, "EXP_RS170_ZOOM4X"=115, "EXP_RS170_BINNING"=116, "EXP_RS170_DECIMATION"=117, "EXP_HW_ACCUM"=118, "EXP_SHT_PREOPEN"=119, "EXP_STORE_STROBE"=120, "EXP_CONT_CLNS"=121, "EXP_TIMING_MODE"=122, "EXP_EXT_TRIGGER"=123, "EXP_EVENT_COUNTER"=124, "EXP_SW_TRIGGER"=125, "EXP_KINETICS_WINDOWSIZE"=126, "EXP_EXPOSURE"=127, "EXP_CONTROLLER_NAME"=128, "EXP_CCD_CHIP_NAME"=129, "EXP_BSWBINNING"=297, "EXP_EDGEENHANCE"=130, "EXP_BOXVIDEOGAIN"=131, "EXP_HSHADING_VALUE"=132, "EXP_VSHADING_VALUE"=133, "EXP_EDGEENHANCE_FLAG"=134, "EXP_SHADING_FLAG"=135, "EXP_GRAYSCALE"=136, "EXP_OFFSET"=137, "EXP_CCDGAIN"=138, "EXP_TEMPERATURE"=139, "EXP_MCPVOLTAGE"=140, "EXP_BOXEXPOSURE"=141, "EXP_ABC_FLAG"=142, "EXP_GAMMA_FLAG"=143, "EXP_AUTOBLACK_FLAG"=144, "EXP_AGC_FLAG"=145, "EXP_ODD_FIELD"=146, "EXP_FIELD_SELECT"=147, "EXP_RESET"=148, "EXP_EXTERN_ENABLE"=149, "EXP_CONTROLLERS_SUPPORTED"=150, "EXP_VTCLK"=151, "EXP_HTCLK"=152, "EXP_GATE_VS_CW"=153, "EXP_COM_PORT"=154, "EXP_US_UNITS"=156, "EXP_MS_UNITS"=157, "EXP_SEC_UNITS"=158, "EXP_MIN_UNITS"=159, "EXP_HRS_UNITS"=160, "EXP_FRAME_UNITS"=161, "EXP_SYNC_ASYNC"=162, "EXP_FOCUS_NFRAME"=163, "EXP_TIMEOUT"=164, "EXP_TIMEOUT_DEFAULT"=165, "EXP_HW_AUTOSTOP"=166, "EXP_RS170_INTEN_OFFSET"=167, "EXP_CONTROLLER_ALIVE"=168, "EXP_FOCUS_TYPE"=169, "EXP_FOCUS_ZOOM"=170, "EXP_FOCUS_PAN"=171, "EXP_MULTI_TAP_ROI"=172, "EXP_USE_INTERUPTS"=173, "EXP_DATA_ACQ_STATE"=174, "EXP_VERIFY_GOOD_VALUES"=175, "EXP_WHITE_CLAMP"=176, "EXP_BLACK_CLAMP"=177, "EXP_DELAY_TIME"=178, "EXP_READOUT_TIME"=179, "EXP_SW_DIAG"=180, "EXP_DIAG1"=181, "EXP_DIAG2"=182, "EXP_DIAG3"=183, "EXP_DIAG4"=184, "EXP_DIAG5"=185, "EXP_AorB_GROUP"=186, "EXP_ABSORBANCE_FLAG"=187, "EXP_ABSORBANCE_METHOD"=188, "EXP_ABSORBANCE_STRIPNUM"=189, "EXP_DMASIZE_VIA_DRIVER"=190, "EXP_DRIVERVERSION"=191, "EXP_NUM_DEVICES"=192, "EXP_ECPDMA_CHANNEL"=193, "EXP_CUSTOM_SHUTTER"=194, "EXP_ADC_OFFSET"=195, "EXP_CURRENT_READOUT_MODE"=196, "EXP_BANK_ADD"=197, "EXP_LUT_BANK"=198, "EXP_SETUP_STATUS"=201, "EXP_XY_GROUPING"=239, "EXP_MESSAGES_FLAG"=240, "EXP_TTL_LINE_TO_WAIT"=253, "EXP_DATA_COLLECTION_MODE"=258, "EXP_DATA_COLLECTION_TYPE"=262, "EXP_SKIPFRAMES"=274, "EXP_CLR_INT_CNTR"=276, "EXP_ENABLE_INT_CNTR"=277, "EXP_INT_CNTR"=278, "EXP_INTERNAL_SYNC_SRC"=279, "EXP_SW_EXTSYNC"=280, "EXP_PTG_PRESENT"=281, "EXP_ELEC_SHT"=282, "EXP_BOARDS_WITH_NVRAM"=283, "EXP_ANLGMASTER_ST143"=284, "EXP_ANLGSLAVE_ST143"=285, "EXP_DISPLAY_ST143"=286, "EXP_INTRFACE_ST143"=287, "EXP_SCANCONTROL_ST143"=288, "EXP_NUMBERFRAMES_IRQ"=204, "EXP_COOL_TYPE"=214, "EXP_HD_TYPE"=215, "EXP_INTENSIFER_GAIN"=216, "EXP_SHT_GATE_MODE"=217, "EXP_HD_CHECK"=218, "EXP_AMP_MODE"=219, "EXP_AMP_DIALOG"=247, "EXP_ANALOG_GAIN"=220, "EXP_HW_FIXES"=221, "EXP_PCI_CARDS"=222, "EXP_NOT_REVERSE"=223, "EXP_LOAD_NVRAM_DEFAULTS"=234, "EXP_CNTR_BRD"=235, "EXP_XDIMHW"=237, "EXP_YDIMHW"=238, "EXP_SPECIAL_FAST_RDOUT"=254, "EXP_SPCL_FAST_Y_DIM"=255, "EXP_SPCL_FAST_X_DIM"=256, "EXP_SPCL_FAST_Y_INDEX"=257, "EXP_SHUTTER_COMP_TIME_MS"=266, "EXP_NVRAM_AVAIL"=267, "EXP_NUMBER_AGAIN_AVAIL"=269, "EXP_SENSOR_TYPE"=270, "EXP_EVENT_TYPE"=292, "EXP_ANTI_BLOOMING"=293, "EXP_FAST_PULSE_ENABLE"=233, "EXP_USE_HEADCALIB"=296, "EXP_TEMP_STATUS"=301, "EXP_MULTIPLE_READMODES_LIVE"=302, "EXP_FIRST_ACQUIRE_FLAG"=303, "EXP_ANTI_BLOOMING_CONTROL"=304, "EXP_PRE_HORZ_DELAY"=305, "EXP_NVRAM_TRIES"=306, "EXP_XASCEND"=307, "EXP_YASCEND"=308, "EXP_ALT_TIMING"=309, "EXP_SHUTTER_PRE_COMP"=310, "EXP_PVCAM_POSSIBLE"=311, "EXP_ADC_IN_NVRAM"=312, "EXP_PASSTHRU_MODE"=313, "EXP_FIRMWAREVERSION"=314, "EXP_IMMEDIATE_SHUTTER"=315, "EXP_STAGE2_TEMP"=316, "EXP_AVGAIN_ENABLED"=317, "EXP_AVGAIN_SETPOINT"=318, "EXP_AVGAIN"=319, "EXP_AVGAIN_CALIB_TEMP"=320, "EXP_AVGAIN_CALIB_COEFF1"=321, "EXP_AVGAIN_CALIB_COEFF2"=322, "EXP_AVGAIN_CALIB_COEFF3"=323, "EXP_AVGAIN_CALIB_COEFF4"=324, "EXP_AVGAIN_CALIB_COEFF5"=325, "EXP_FORCE_READOUT_MODE"=326, "EXP_RESET_DATACOLLECTION"=327, "EXP_ACTIVE_SUBFRAME"=328, "EXP_PV_READOUT_PORT"=514, "EXP_CLASSNAME"=775, "EXP_FLATFLDNAME"=776, "EXP_DARKNAME"=777, "EXP_SETUPNAME"=778, "EXP_ACCESSNAME"=779, "EXP_DATFILENAME"=780, "EXP_ABSORBFILENAME"=781, "EXP_BLEMISHFILENAME"=782, "EXP_COSMICFILENAME"=783, "EXP_FILEINCBASENAME"=784, "EXP_YTNAME"=785, "EXP_DEVNAME"=786, "EXP_USEROI"=787, "EXP_DOBLEMISH"=788, "EXP_DOABSORB"=789, "EXP_DOCOSMIC"=790, "EXP_COSMICSENS"=791, "EXP_ABSORBSTRIP"=792, "EXP_DATATYPE"=793, "EXP_OVERWRITECONFIRM"=794, "EXP_FILEINCENABLE"=795, "EXP_FILEINCCOUNT"=796, "EXP_RUNNING"=797, "EXP_SAVEROPT"=798, "EXP_TIME_UNITS"=799, "EXP_FILEACCESS"=800, "EXP_AUTOSAVE"=801, "EXP_NEWWINDOW"=802, "EXP_XDIM"=803, "EXP_YDIM"=804, "EXP_XDIMDET"=805, "EXP_YDIMDET"=806, "EXP_ROIMODE"=807, "EXP_NUMREPEATSEXP"=808, "EXP_NUMACCUMSEXP"=809, "EXP_THREADSTATE"=810, "EXP_USEMINTHRESHOLDING"=811, "EXP_MINTHRESHOLDVALUE"=812, "EXP_USEMAXTHRESHOLDING"=813, "EXP_MAXTHRESHOLDVALUE"=814, "EXP_RUNNING_EXPERIMENT"=815, "EXP_THRESHOLD_DEMAND_UPDATE"=816, "EXP_ROICOUNT"=817, "EXP_ACCUMS"=818, "EXP_CACCUMS"=819, "EXP_CSEQUENTS"=820, "EXP_PHOTON_ESTIMATION_ENABLE"=821, "EXP_PHOTON_MAXTIME"=822, "EXP_PHOTON_MAXTIMEUNIT"=823, "EXP_CUSTOMFILTER_ENABLE"=824, "EXP_CUSTOMFILTER_SIZE"=825, "EXP_LOOKUPTABLE_ENABLE"=826, "EXP_BSHOWWINDOW"=827, "EXP_BBACKSUBTRACT"=828, "EXP_BDOFLATFIELD"=829, "EXP_ASCIIOUTPUTFILE"=830, "EXP_ASCIIOUTPUT_DELIMITER"=831, "EXP_ASCIIOUTPUT_TERMINATOR"=832, "EXP_FFTYPE"=833, "EXP_BGTYPE"=834, "EXP_COSGRASS"=835, "EXP_RUNASCONFIRM"=836, "EXP_RUNASRUNACCESS"=837, "EXP_DATAFILETYPE"=838, "EXP_ROTATE"=839, "EXP_FLIP"=840, "EXP_REVERSE"=841, "EXP_SWBINNING"=842, "EXP_AUTOSTORE"=843, "EXP_XBINNED"=844, "EXP_YBINNED"=845, "EXP_NUMPATTERNS"=846, "EXP_EXPERIMENTTIME"=847, "EXP_ASYNCSEQUENTIALS"=848, "EXP_SEQUENTIALS"=849, "EXP_CSEQUENTIALS"=850, "EXP_AUTOD"=851, "EXP_EXPOSURETIME"=852, "EXP_EXPOSURETIME_UNITS"=853, "EXP_ACQMODE"=854, "EXP_DMASIZE_PVCAM"=855, "EXP_INITIALIZE"=856, "EXP_CELL_X_SIZE"=857, "EXP_CELL_Y_SIZE"=858, "EXP_X_GAP_SIZE"=859, "EXP_Y_GAP_SIZE"=860] ("Param")
                w159 = 127 items=["EXP_ETACTUAL"=1, "EXP_SEQUENTS"=2, "EXP_ERROR"=3, "EXP_GETCAPS"=4, "EXP_GETPLSR"=5, "EXP_DETECTOR_BIT"=16, "EXP_RUNNING_APP"=23, "EXP_VIDEO_TYPE"=24, "EXP_CUSTOM_VIDEO_X"=25, "EXP_CUSTOM_VIDEO_Y"=26, "EXP_CUSTOM_VIDEO_FSTWIDTH"=27, "EXP_CUSTOM_VIDEO_LSTWIDTH"=28, "EXP_VIDEO_XDIM"=29, "EXP_VIDEO_YDIM"=30, "EXP_VIDEO_MAX_ZOOM"=31, "EXP_VIDEO_HORZ_PAN"=32, "EXP_VIDEO_VERT_PAN"=33, "EXP_WORD_MULTIPLIER"=34, "EXP_TARGET_ID"=35, "EXP_ADAPTER_ID"=36, "EXP_NUMADAPTORS"=37, "EXP_FORCE_PP_INIT"=38, "EXP_NOP_ADC"=39, "EXP_ACTUAL_TEMP"=40, "EXP_FORCE_AUTOSTOP"=41, "EXP_DEFAULT_VTCLK"=42, "EXP_MIN_VTCLK"=43, "EXP_MAX_VTCLK"=44, "EXP_DEFAULT_HTCLK"=45, "EXP_MIN_HTCLK"=46, "EXP_MAX_HTCLK"=47, "EXP_TIMING_STYLE"=48, "EXP_HEADSELECT"=49, "EXP_HORZPHASE"=50, "EXP_VERTPHASE"=51, "EXP_SPECIAL_SPEED"=52, "EXP_PRE_STRIPS"=53, "EXP_POST_STRIPS"=54, "EXP_PRE_LINES"=55, "EXP_POST_LINES"=56, "EXP_ACTIVE_LINES"=57, "EXP_ACTIVE_STRIPS"=58, "EXP_XFER_EXTRA"=59, "EXP_MIN_BLOCK"=60, "EXP_NUM_MIN_BLOCK"=61, "EXP_LOGIC_OUTPUT"=66, "EXP_VIDEO_BLANK"=67, "EXP_ZOOM_MODE_VIDEO"=68, "EXP_LEVEL_SYNC"=69, "EXP_DISABLE_LASER"=70, "EXP_ACQBACK_SHUTTER"=71, "EXP_ACQFLAT_SHUTTER"=72, "EXP_SMALL_CCD_MINEXP"=73, "EXP_LARGE_CCD_MINEXP"=74, "EXP_GATING_MODE"=75, "EXP_ILME_B1X"=76, "EXP_ILME_B2X"=77, "EXP_ILME_D1X"=78, "EXP_ILME_D2X"=79, "EXP_ILME_D4X"=80, "EXP_INIT_HW_ACCUM"=81, "EXP_5X_GAIN_ENABLE"=82, "EXP_RET_SRCCMP"=83, "EXP_EVENT_HANDLE"=84, "EXP_READOUT_MODE"=85, "EXP_SHUTTER_TYPE"=86, "EXP_USER_DEFINED_CHIP"=87, "EXP_USER_DEFINED_TIMING"=88, "EXP_CONTROLLER_VERSION"=89, "EXP_GET_CONTROLLER_VER"=90, "EXP_TTL_LINES"=91, "EXP_BIT_ADJUST"=92, "EXP_RESOLUTION"=93, "EXP_GAIN"=94, "EXP_ADC_RATE"=95, "EXP_ADC_TYPE"=96, "EXP_NUMBER_OF_CLEANS"=97, "EXP_NUM_OF_STRIPS_PER_CLN"=98, "EXP_INTERFACE_CARD"=99, "EXP_INTERRUPT"=100, "EXP_IO_ADDRESS1"=101, "EXP_IO_ADDRESS2"=102, "EXP_IO_ADDRESS3"=103, "EXP_HW_ROI"=104, "EXP_HW_BINNING"=105, "EXP_EDGE_TRIGGER"=106, "EXP_SHUTTER_CONTROL"=107, "EXP_RS170"=108, "EXP_RS170_COMPLEX"=109, "EXP_HW_RS170_LUT"=110, "EXP_RS170_INTENSITY_SCALING"=111, "EXP_RS170_OFFSET"=112, "EXP_RS170_PAN"=113, "EXP_RS170_ZOOM2X"=114, "EXP_RS170_ZOOM4X"=115, "EXP_RS170_BINNING"=116, "EXP_RS170_DECIMATION"=117, "EXP_HW_ACCUM"=118, "EXP_SHT_PREOPEN"=119, "EXP_STORE_STROBE"=120, "EXP_CONT_CLNS"=121, "EXP_TIMING_MODE"=122, "EXP_EXT_TRIGGER"=123, "EXP_EVENT_COUNTER"=124, "EXP_SW_TRIGGER"=125, "EXP_KINETICS_WINDOWSIZE"=126, "EXP_EXPOSURE"=127, "EXP_CONTROLLER_NAME"=128, "EXP_CCD_CHIP_NAME"=129, "EXP_BSWBINNING"=297, "EXP_EDGEENHANCE"=130, "EXP_BOXVIDEOGAIN"=131, "EXP_HSHADING_VALUE"=132, "EXP_VSHADING_VALUE"=133, "EXP_EDGEENHANCE_FLAG"=134, "EXP_SHADING_FLAG"=135, "EXP_GRAYSCALE"=136, "EXP_OFFSET"=137, "EXP_CCDGAIN"=138, "EXP_TEMPERATURE"=139, "EXP_MCPVOLTAGE"=140, "EXP_BOXEXPOSURE"=141, "EXP_ABC_FLAG"=142, "EXP_GAMMA_FLAG"=143, "EXP_AUTOBLACK_FLAG"=144, "EXP_AGC_FLAG"=145, "EXP_ODD_FIELD"=146, "EXP_FIELD_SELECT"=147, "EXP_RESET"=148, "EXP_EXTERN_ENABLE"=149, "EXP_CONTROLLERS_SUPPORTED"=150, "EXP_VTCLK"=151, "EXP_HTCLK"=152, "EXP_GATE_VS_CW"=153, "EXP_COM_PORT"=154, "EXP_US_UNITS"=156, "EXP_MS_UNITS"=157, "EXP_SEC_UNITS"=158, "EXP_MIN_UNITS"=159, "EXP_HRS_UNITS"=160, "EXP_FRAME_UNITS"=161, "EXP_SYNC_ASYNC"=162, "EXP_FOCUS_NFRAME"=163, "EXP_TIMEOUT"=164, "EXP_TIMEOUT_DEFAULT"=165, "EXP_HW_AUTOSTOP"=166, "EXP_RS170_INTEN_OFFSET"=167, "EXP_CONTROLLER_ALIVE"=168, "EXP_FOCUS_TYPE"=169, "EXP_FOCUS_ZOOM"=170, "EXP_FOCUS_PAN"=171, "EXP_MULTI_TAP_ROI"=172, "EXP_USE_INTERUPTS"=173, "EXP_DATA_ACQ_STATE"=174, "EXP_VERIFY_GOOD_VALUES"=175, "EXP_WHITE_CLAMP"=176, "EXP_BLACK_CLAMP"=177, "EXP_DELAY_TIME"=178, "EXP_READOUT_TIME"=179, "EXP_SW_DIAG"=180, "EXP_DIAG1"=181, "EXP_DIAG2"=182, "EXP_DIAG3"=183, "EXP_DIAG4"=184, "EXP_DIAG5"=185, "EXP_AorB_GROUP"=186, "EXP_ABSORBANCE_FLAG"=187, "EXP_ABSORBANCE_METHOD"=188, "EXP_ABSORBANCE_STRIPNUM"=189, "EXP_DMASIZE_VIA_DRIVER"=190, "EXP_DRIVERVERSION"=191, "EXP_NUM_DEVICES"=192, "EXP_ECPDMA_CHANNEL"=193, "EXP_CUSTOM_SHUTTER"=194, "EXP_ADC_OFFSET"=195, "EXP_CURRENT_READOUT_MODE"=196, "EXP_BANK_ADD"=197, "EXP_LUT_BANK"=198, "EXP_SETUP_STATUS"=201, "EXP_XY_GROUPING"=239, "EXP_MESSAGES_FLAG"=240, "EXP_TTL_LINE_TO_WAIT"=253, "EXP_DATA_COLLECTION_MODE"=258, "EXP_DATA_COLLECTION_TYPE"=262, "EXP_SKIPFRAMES"=274, "EXP_CLR_INT_CNTR"=276, "EXP_ENABLE_INT_CNTR"=277, "EXP_INT_CNTR"=278, "EXP_INTERNAL_SYNC_SRC"=279, "EXP_SW_EXTSYNC"=280, "EXP_PTG_PRESENT"=281, "EXP_ELEC_SHT"=282, "EXP_BOARDS_WITH_NVRAM"=283, "EXP_ANLGMASTER_ST143"=284, "EXP_ANLGSLAVE_ST143"=285, "EXP_DISPLAY_ST143"=286, "EXP_INTRFACE_ST143"=287, "EXP_SCANCONTROL_ST143"=288, "EXP_NUMBERFRAMES_IRQ"=204, "EXP_COOL_TYPE"=214, "EXP_HD_TYPE"=215, "EXP_INTENSIFER_GAIN"=216, "EXP_SHT_GATE_MODE"=217, "EXP_HD_CHECK"=218, "EXP_AMP_MODE"=219, "EXP_AMP_DIALOG"=247, "EXP_ANALOG_GAIN"=220, "EXP_HW_FIXES"=221, "EXP_PCI_CARDS"=222, "EXP_NOT_REVERSE"=223, "EXP_LOAD_NVRAM_DEFAULTS"=234, "EXP_CNTR_BRD"=235, "EXP_XDIMHW"=237, "EXP_YDIMHW"=238, "EXP_SPECIAL_FAST_RDOUT"=254, "EXP_SPCL_FAST_Y_DIM"=255, "EXP_SPCL_FAST_X_DIM"=256, "EXP_SPCL_FAST_Y_INDEX"=257, "EXP_SHUTTER_COMP_TIME_MS"=266, "EXP_NVRAM_AVAIL"=267, "EXP_NUMBER_AGAIN_AVAIL"=269, "EXP_SENSOR_TYPE"=270, "EXP_EVENT_TYPE"=292, "EXP_ANTI_BLOOMING"=293, "EXP_FAST_PULSE_ENABLE"=233, "EXP_USE_HEADCALIB"=296, "EXP_TEMP_STATUS"=301, "EXP_MULTIPLE_READMODES_LIVE"=302, "EXP_FIRST_ACQUIRE_FLAG"=303, "EXP_ANTI_BLOOMING_CONTROL"=304, "EXP_PRE_HORZ_DELAY"=305, "EXP_NVRAM_TRIES"=306, "EXP_XASCEND"=307, "EXP_YASCEND"=308, "EXP_ALT_TIMING"=309, "EXP_SHUTTER_PRE_COMP"=310, "EXP_PVCAM_POSSIBLE"=311, "EXP_ADC_IN_NVRAM"=312, "EXP_PASSTHRU_MODE"=313, "EXP_FIRMWAREVERSION"=314, "EXP_IMMEDIATE_SHUTTER"=315, "EXP_STAGE2_TEMP"=316, "EXP_AVGAIN_ENABLED"=317, "EXP_AVGAIN_SETPOINT"=318, "EXP_AVGAIN"=319, "EXP_AVGAIN_CALIB_TEMP"=320, "EXP_AVGAIN_CALIB_COEFF1"=321, "EXP_AVGAIN_CALIB_COEFF2"=322, "EXP_AVGAIN_CALIB_COEFF3"=323, "EXP_AVGAIN_CALIB_COEFF4"=324, "EXP_AVGAIN_CALIB_COEFF5"=325, "EXP_FORCE_READOUT_MODE"=326, "EXP_RESET_DATACOLLECTION"=327, "EXP_ACTIVE_SUBFRAME"=328, "EXP_PV_READOUT_PORT"=514, "EXP_CLASSNAME"=775, "EXP_FLATFLDNAME"=776, "EXP_DARKNAME"=777, "EXP_SETUPNAME"=778, "EXP_ACCESSNAME"=779, "EXP_DATFILENAME"=780, "EXP_ABSORBFILENAME"=781, "EXP_BLEMISHFILENAME"=782, "EXP_COSMICFILENAME"=783, "EXP_FILEINCBASENAME"=784, "EXP_YTNAME"=785, "EXP_DEVNAME"=786, "EXP_USEROI"=787, "EXP_DOBLEMISH"=788, "EXP_DOABSORB"=789, "EXP_DOCOSMIC"=790, "EXP_COSMICSENS"=791, "EXP_ABSORBSTRIP"=792, "EXP_DATATYPE"=793, "EXP_OVERWRITECONFIRM"=794, "EXP_FILEINCENABLE"=795, "EXP_FILEINCCOUNT"=796, "EXP_RUNNING"=797, "EXP_SAVEROPT"=798, "EXP_TIME_UNITS"=799, "EXP_FILEACCESS"=800, "EXP_AUTOSAVE"=801, "EXP_NEWWINDOW"=802, "EXP_XDIM"=803, "EXP_YDIM"=804, "EXP_XDIMDET"=805, "EXP_YDIMDET"=806, "EXP_ROIMODE"=807, "EXP_NUMREPEATSEXP"=808, "EXP_NUMACCUMSEXP"=809, "EXP_THREADSTATE"=810, "EXP_USEMINTHRESHOLDING"=811, "EXP_MINTHRESHOLDVALUE"=812, "EXP_USEMAXTHRESHOLDING"=813, "EXP_MAXTHRESHOLDVALUE"=814, "EXP_RUNNING_EXPERIMENT"=815, "EXP_THRESHOLD_DEMAND_UPDATE"=816, "EXP_ROICOUNT"=817, "EXP_ACCUMS"=818, "EXP_CACCUMS"=819, "EXP_CSEQUENTS"=820, "EXP_PHOTON_ESTIMATION_ENABLE"=821, "EXP_PHOTON_MAXTIME"=822, "EXP_PHOTON_MAXTIMEUNIT"=823, "EXP_CUSTOMFILTER_ENABLE"=824, "EXP_CUSTOMFILTER_SIZE"=825, "EXP_LOOKUPTABLE_ENABLE"=826, "EXP_BSHOWWINDOW"=827, "EXP_BBACKSUBTRACT"=828, "EXP_BDOFLATFIELD"=829, "EXP_ASCIIOUTPUTFILE"=830, "EXP_ASCIIOUTPUT_DELIMITER"=831, "EXP_ASCIIOUTPUT_TERMINATOR"=832, "EXP_FFTYPE"=833, "EXP_BGTYPE"=834, "EXP_COSGRASS"=835, "EXP_RUNASCONFIRM"=836, "EXP_RUNASRUNACCESS"=837, "EXP_DATAFILETYPE"=838, "EXP_ROTATE"=839, "EXP_FLIP"=840, "EXP_REVERSE"=841, "EXP_SWBINNING"=842, "EXP_AUTOSTORE"=843, "EXP_XBINNED"=844, "EXP_YBINNED"=845, "EXP_NUMPATTERNS"=846, "EXP_EXPERIMENTTIME"=847, "EXP_ASYNCSEQUENTIALS"=848, "EXP_SEQUENTIALS"=849, "EXP_CSEQUENTIALS"=850, "EXP_AUTOD"=851, "EXP_EXPOSURETIME"=852, "EXP_EXPOSURETIME_UNITS"=853, "EXP_ACQMODE"=854, "EXP_DMASIZE_PVCAM"=855, "EXP_INITIALIZE"=856, "EXP_CELL_X_SIZE"=857, "EXP_CELL_Y_SIZE"=858, "EXP_X_GAP_SIZE"=859, "EXP_Y_GAP_SIZE"=860] ("Param")
                # "camera"
                n102 = invoke class="IExpSetup2" method="SetParam"(reference=w156, "Param"=w162, "pSetVal"=w154) -> (reference out=w157:refnum<k7>)  [unwired: 2 in, 4 out]
                n103 = invoke class="IExpSetup2" method="SetParam"(reference=w157, "Param"=w161, "pSetVal"=w154) -> (reference out=w140:refnum<k7>)  [unwired: 2 in, 4 out]
                n104 = invoke class="IExpSetup2" method="SetParam"(reference=w140, "Param"=w141, "pSetVal"=FALSE) -> (reference out=w137:refnum<k7>)  [unwired: 2 in, 4 out]
                n105 = local read "OMA V exposure time"() -> (w158:dbl)
                n106 = invoke class="IExpSetup2" method="GetParam"(reference=w137, "Param"=w138) -> (reference out=w136:refnum<k7>, "GetParam"=w135:variant)  [unwired: 3 in, 3 out]
                n107 = invoke class="IExpSetup2" method="SetParam"(reference=w136, "Param"=w159, "pSetVal"=w158) -> (reference out=w143:refnum<k7>)  [unwired: 2 in, 4 out]
                n108 = Variant To Data(type=TRUE, Variant=w135) -> (data=w133:bool)  [unwired: 1 in, 1 out]
                n109 = case shown="True" w133 {
                  frame False {
                  }
                  frame True {
                    n110 = property on="Spectro Correct background" class="Bool (strict)"("DisabledEnum"=T2."Enabled" ("Disabled")) -> ()  [unwired: 2 in, 2 out]
                  }
                }
                n111 = local write "Spectro Correct background"(w133) -> ()
                n112 = invoke class="IExpSetup2" method="SetParam"(reference=w143, "Param"=w160, "pSetVal"=path "C:/Users/Yuriy/OMAV" ("Full File Name\nfor Acqure")) -> (reference out=w153:refnum<k7>)  [unwired: 2 in, 4 out]
                n113 = local read "OMA V gain"() -> (w142:u32)
                n114 = local read "Set Temperature (°C)"() -> (w150:i8)
                n115 = invoke class="IExpSetup2" method="SetParam"(reference=w153, "Param"=w152, "pSetVal"=w142) -> (reference out=w151:refnum<k7>)  [unwired: 2 in, 4 out]
                n116 = invoke class="IExpSetup2" method="SetParam"(reference=w151, "Param"=w149, "pSetVal"=w150) -> (reference out=w148:refnum<k7>)  [unwired: 2 in, 4 out]
                n117 = invoke class="IExpSetup2" method="GetParam"(reference=w148, "Param"=w147) -> ("GetParam"=w145:variant)  [unwired: 3 in, 4 out]
                n118 = Variant To Data(type=0.0, Variant=w145) -> (data=w144:dbl)  [unwired: 1 in, 1 out]
                n119 = local write "OMA V temp"(w144) -> ()
              }
              frame #2 {
              }
              frame #3 {
                n120 = local write "busy"(FALSE ("busy")) -> ()
                n121 = local write "Spectro ON"(TRUE ("Spectro ON")) -> ()
              }
            }
            n122 = Automation Open(Automation Refnum="experiment reference_raw") -> (Automation Refnum=w112:refnum<k7>)  [unwired: 3 in, 1 out]
            "experiment reference" <- w112
            n123 = invoke class="IExpSetup2" method="WaitForExperiment"(reference=w112) -> (reference out=w111:refnum<k7>)  [unwired: 2 in, 2 out]
          }
          frame 3 {
            # "Synchronize hosts"
            n124 = flat-sequence {
              frame #0 {
                n125 = Create Network Stream Writer Endpoint(7:1 ("writer buffer size"), 9:cluster{dbl[], dbl[]} {array[512 elements], array[512 elements]} ("XY Graph OMA V"), 10:"//140.78.89.185/R_master" ("reader url"), 11:"W_slave" ("writer name")) -> (0:w168:errorcluster, 3:→"writer endpoint":refnum<k21>)  [unwired: 3 in]
                "error writer" <- w168
                n126 = Create Network Stream Reader Endpoint(7:1 ("reader buffer size"), 9:TRUE, 10:"//140.78.89.185/W_master" ("writer url"), 11:"R_slave" ("reader name")) -> (0:w167:errorcluster, 3:→"reader endpoint":refnum<k21>)  [unwired: 3 in]
                "error reader" <- w167
                n127 = Not(x=w168) -> (.not. x?=w170:bool)
                n128 = Not(x=w167) -> (.not. x?=w169:bool)
                n129 = And(x=w170, y=w169) -> (x .and. y?=w166:bool)
                n130 = local write "Hosts Synchronized"(w166) -> ()
              }
              frame #1 {
                n131 = local write "busy"(FALSE ("busy")) -> ()
              }
            }
          }
          frame 4 {
            w184 = 40 items=["EXP_ETACTUAL"=1, "EXP_SEQUENTS"=2, "EXP_ERROR"=3, "EXP_GETCAPS"=4, "EXP_GETPLSR"=5, "EXP_DETECTOR_BIT"=16, "EXP_RUNNING_APP"=23, "EXP_VIDEO_TYPE"=24, "EXP_CUSTOM_VIDEO_X"=25, "EXP_CUSTOM_VIDEO_Y"=26, "EXP_CUSTOM_VIDEO_FSTWIDTH"=27, "EXP_CUSTOM_VIDEO_LSTWIDTH"=28, "EXP_VIDEO_XDIM"=29, "EXP_VIDEO_YDIM"=30, "EXP_VIDEO_MAX_ZOOM"=31, "EXP_VIDEO_HORZ_PAN"=32, "EXP_VIDEO_VERT_PAN"=33, "EXP_WORD_MULTIPLIER"=34, "EXP_TARGET_ID"=35, "EXP_ADAPTER_ID"=36, "EXP_NUMADAPTORS"=37, "EXP_FORCE_PP_INIT"=38, "EXP_NOP_ADC"=39, "EXP_ACTUAL_TEMP"=40, "EXP_FORCE_AUTOSTOP"=41, "EXP_DEFAULT_VTCLK"=42, "EXP_MIN_VTCLK"=43, "EXP_MAX_VTCLK"=44, "EXP_DEFAULT_HTCLK"=45, "EXP_MIN_HTCLK"=46, "EXP_MAX_HTCLK"=47, "EXP_TIMING_STYLE"=48, "EXP_HEADSELECT"=49, "EXP_HORZPHASE"=50, "EXP_VERTPHASE"=51, "EXP_SPECIAL_SPEED"=52, "EXP_PRE_STRIPS"=53, "EXP_POST_STRIPS"=54, "EXP_PRE_LINES"=55, "EXP_POST_LINES"=56, "EXP_ACTIVE_LINES"=57, "EXP_ACTIVE_STRIPS"=58, "EXP_XFER_EXTRA"=59, "EXP_MIN_BLOCK"=60, "EXP_NUM_MIN_BLOCK"=61, "EXP_LOGIC_OUTPUT"=66, "EXP_VIDEO_BLANK"=67, "EXP_ZOOM_MODE_VIDEO"=68, "EXP_LEVEL_SYNC"=69, "EXP_DISABLE_LASER"=70, "EXP_ACQBACK_SHUTTER"=71, "EXP_ACQFLAT_SHUTTER"=72, "EXP_SMALL_CCD_MINEXP"=73, "EXP_LARGE_CCD_MINEXP"=74, "EXP_GATING_MODE"=75, "EXP_ILME_B1X"=76, "EXP_ILME_B2X"=77, "EXP_ILME_D1X"=78, "EXP_ILME_D2X"=79, "EXP_ILME_D4X"=80, "EXP_INIT_HW_ACCUM"=81, "EXP_5X_GAIN_ENABLE"=82, "EXP_RET_SRCCMP"=83, "EXP_EVENT_HANDLE"=84, "EXP_READOUT_MODE"=85, "EXP_SHUTTER_TYPE"=86, "EXP_USER_DEFINED_CHIP"=87, "EXP_USER_DEFINED_TIMING"=88, "EXP_CONTROLLER_VERSION"=89, "EXP_GET_CONTROLLER_VER"=90, "EXP_TTL_LINES"=91, "EXP_BIT_ADJUST"=92, "EXP_RESOLUTION"=93, "EXP_GAIN"=94, "EXP_ADC_RATE"=95, "EXP_ADC_TYPE"=96, "EXP_NUMBER_OF_CLEANS"=97, "EXP_NUM_OF_STRIPS_PER_CLN"=98, "EXP_INTERFACE_CARD"=99, "EXP_INTERRUPT"=100, "EXP_IO_ADDRESS1"=101, "EXP_IO_ADDRESS2"=102, "EXP_IO_ADDRESS3"=103, "EXP_HW_ROI"=104, "EXP_HW_BINNING"=105, "EXP_EDGE_TRIGGER"=106, "EXP_SHUTTER_CONTROL"=107, "EXP_RS170"=108, "EXP_RS170_COMPLEX"=109, "EXP_HW_RS170_LUT"=110, "EXP_RS170_INTENSITY_SCALING"=111, "EXP_RS170_OFFSET"=112, "EXP_RS170_PAN"=113, "EXP_RS170_ZOOM2X"=114, "EXP_RS170_ZOOM4X"=115, "EXP_RS170_BINNING"=116, "EXP_RS170_DECIMATION"=117, "EXP_HW_ACCUM"=118, "EXP_SHT_PREOPEN"=119, "EXP_STORE_STROBE"=120, "EXP_CONT_CLNS"=121, "EXP_TIMING_MODE"=122, "EXP_EXT_TRIGGER"=123, "EXP_EVENT_COUNTER"=124, "EXP_SW_TRIGGER"=125, "EXP_KINETICS_WINDOWSIZE"=126, "EXP_EXPOSURE"=127, "EXP_CONTROLLER_NAME"=128, "EXP_CCD_CHIP_NAME"=129, "EXP_BSWBINNING"=297, "EXP_EDGEENHANCE"=130, "EXP_BOXVIDEOGAIN"=131, "EXP_HSHADING_VALUE"=132, "EXP_VSHADING_VALUE"=133, "EXP_EDGEENHANCE_FLAG"=134, "EXP_SHADING_FLAG"=135, "EXP_GRAYSCALE"=136, "EXP_OFFSET"=137, "EXP_CCDGAIN"=138, "EXP_TEMPERATURE"=139, "EXP_MCPVOLTAGE"=140, "EXP_BOXEXPOSURE"=141, "EXP_ABC_FLAG"=142, "EXP_GAMMA_FLAG"=143, "EXP_AUTOBLACK_FLAG"=144, "EXP_AGC_FLAG"=145, "EXP_ODD_FIELD"=146, "EXP_FIELD_SELECT"=147, "EXP_RESET"=148, "EXP_EXTERN_ENABLE"=149, "EXP_CONTROLLERS_SUPPORTED"=150, "EXP_VTCLK"=151, "EXP_HTCLK"=152, "EXP_GATE_VS_CW"=153, "EXP_COM_PORT"=154, "EXP_US_UNITS"=156, "EXP_MS_UNITS"=157, "EXP_SEC_UNITS"=158, "EXP_MIN_UNITS"=159, "EXP_HRS_UNITS"=160, "EXP_FRAME_UNITS"=161, "EXP_SYNC_ASYNC"=162, "EXP_FOCUS_NFRAME"=163, "EXP_TIMEOUT"=164, "EXP_TIMEOUT_DEFAULT"=165, "EXP_HW_AUTOSTOP"=166, "EXP_RS170_INTEN_OFFSET"=167, "EXP_CONTROLLER_ALIVE"=168, "EXP_FOCUS_TYPE"=169, "EXP_FOCUS_ZOOM"=170, "EXP_FOCUS_PAN"=171, "EXP_MULTI_TAP_ROI"=172, "EXP_USE_INTERUPTS"=173, "EXP_DATA_ACQ_STATE"=174, "EXP_VERIFY_GOOD_VALUES"=175, "EXP_WHITE_CLAMP"=176, "EXP_BLACK_CLAMP"=177, "EXP_DELAY_TIME"=178, "EXP_READOUT_TIME"=179, "EXP_SW_DIAG"=180, "EXP_DIAG1"=181, "EXP_DIAG2"=182, "EXP_DIAG3"=183, "EXP_DIAG4"=184, "EXP_DIAG5"=185, "EXP_AorB_GROUP"=186, "EXP_ABSORBANCE_FLAG"=187, "EXP_ABSORBANCE_METHOD"=188, "EXP_ABSORBANCE_STRIPNUM"=189, "EXP_DMASIZE_VIA_DRIVER"=190, "EXP_DRIVERVERSION"=191, "EXP_NUM_DEVICES"=192, "EXP_ECPDMA_CHANNEL"=193, "EXP_CUSTOM_SHUTTER"=194, "EXP_ADC_OFFSET"=195, "EXP_CURRENT_READOUT_MODE"=196, "EXP_BANK_ADD"=197, "EXP_LUT_BANK"=198, "EXP_SETUP_STATUS"=201, "EXP_XY_GROUPING"=239, "EXP_MESSAGES_FLAG"=240, "EXP_TTL_LINE_TO_WAIT"=253, "EXP_DATA_COLLECTION_MODE"=258, "EXP_DATA_COLLECTION_TYPE"=262, "EXP_SKIPFRAMES"=274, "EXP_CLR_INT_CNTR"=276, "EXP_ENABLE_INT_CNTR"=277, "EXP_INT_CNTR"=278, "EXP_INTERNAL_SYNC_SRC"=279, "EXP_SW_EXTSYNC"=280, "EXP_PTG_PRESENT"=281, "EXP_ELEC_SHT"=282, "EXP_BOARDS_WITH_NVRAM"=283, "EXP_ANLGMASTER_ST143"=284, "EXP_ANLGSLAVE_ST143"=285, "EXP_DISPLAY_ST143"=286, "EXP_INTRFACE_ST143"=287, "EXP_SCANCONTROL_ST143"=288, "EXP_NUMBERFRAMES_IRQ"=204, "EXP_COOL_TYPE"=214, "EXP_HD_TYPE"=215, "EXP_INTENSIFER_GAIN"=216, "EXP_SHT_GATE_MODE"=217, "EXP_HD_CHECK"=218, "EXP_AMP_MODE"=219, "EXP_AMP_DIALOG"=247, "EXP_ANALOG_GAIN"=220, "EXP_HW_FIXES"=221, "EXP_PCI_CARDS"=222, "EXP_NOT_REVERSE"=223, "EXP_LOAD_NVRAM_DEFAULTS"=234, "EXP_CNTR_BRD"=235, "EXP_XDIMHW"=237, "EXP_YDIMHW"=238, "EXP_SPECIAL_FAST_RDOUT"=254, "EXP_SPCL_FAST_Y_DIM"=255, "EXP_SPCL_FAST_X_DIM"=256, "EXP_SPCL_FAST_Y_INDEX"=257, "EXP_SHUTTER_COMP_TIME_MS"=266, "EXP_NVRAM_AVAIL"=267, "EXP_NUMBER_AGAIN_AVAIL"=269, "EXP_SENSOR_TYPE"=270, "EXP_EVENT_TYPE"=292, "EXP_ANTI_BLOOMING"=293, "EXP_FAST_PULSE_ENABLE"=233, "EXP_USE_HEADCALIB"=296, "EXP_TEMP_STATUS"=301, "EXP_MULTIPLE_READMODES_LIVE"=302, "EXP_FIRST_ACQUIRE_FLAG"=303, "EXP_ANTI_BLOOMING_CONTROL"=304, "EXP_PRE_HORZ_DELAY"=305, "EXP_NVRAM_TRIES"=306, "EXP_XASCEND"=307, "EXP_YASCEND"=308, "EXP_ALT_TIMING"=309, "EXP_SHUTTER_PRE_COMP"=310, "EXP_PVCAM_POSSIBLE"=311, "EXP_ADC_IN_NVRAM"=312, "EXP_PASSTHRU_MODE"=313, "EXP_FIRMWAREVERSION"=314, "EXP_IMMEDIATE_SHUTTER"=315, "EXP_STAGE2_TEMP"=316, "EXP_AVGAIN_ENABLED"=317, "EXP_AVGAIN_SETPOINT"=318, "EXP_AVGAIN"=319, "EXP_AVGAIN_CALIB_TEMP"=320, "EXP_AVGAIN_CALIB_COEFF1"=321, "EXP_AVGAIN_CALIB_COEFF2"=322, "EXP_AVGAIN_CALIB_COEFF3"=323, "EXP_AVGAIN_CALIB_COEFF4"=324, "EXP_AVGAIN_CALIB_COEFF5"=325, "EXP_FORCE_READOUT_MODE"=326, "EXP_RESET_DATACOLLECTION"=327, "EXP_ACTIVE_SUBFRAME"=328, "EXP_PV_READOUT_PORT"=514, "EXP_COOLING_FAN_CTRL"=339, "EXP_SHTR_RES"=343, "EXP_PBC"=351, "EXP_PREEXP_CLEANS"=354, "EXP_TTL_CTRL"=355, "EXP_PAR_SHIFT_INDEX"=547, "EXP_LOGIC_OUTPUT_INVERT"=548, "EXP_CLASSNAME"=775, "EXP_FLATFLDNAME"=776, "EXP_DARKNAME"=777, "EXP_SETUPNAME"=778, "EXP_ACCESSNAME"=779, "EXP_DATFILENAME"=780, "EXP_ABSORBFILENAME"=781, "EXP_BLEMISHFILENAME"=782, "EXP_COSMICFILENAME"=783, "EXP_FILEINCBASENAME"=784, "EXP_YTNAME"=785, "EXP_DEVNAME"=786, "EXP_USEROI"=787, "EXP_DOBLEMISH"=788, "EXP_DOABSORB"=789, "EXP_DOCOSMIC"=790, "EXP_COSMICSENS"=791, "EXP_ABSORBSTRIP"=792, "EXP_DATATYPE"=793, "EXP_OVERWRITECONFIRM"=794, "EXP_FILEINCENABLE"=795, "EXP_FILEINCCOUNT"=796, "EXP_RUNNING"=797, "EXP_SAVEROPT"=798, "EXP_TIME_UNITS"=799, "EXP_FILEACCESS"=800, "EXP_AUTOSAVE"=801, "EXP_NEWWINDOW"=802, "EXP_XDIM"=803, "EXP_YDIM"=804, "EXP_XDIMDET"=805, "EXP_YDIMDET"=806, "EXP_ROIMODE"=807, "EXP_NUMREPEATSEXP"=808, "EXP_NUMACCUMSEXP"=809, "EXP_THREADSTATE"=810, "EXP_USEMINTHRESHOLDING"=811, "EXP_MINTHRESHOLDVALUE"=812, "EXP_USEMAXTHRESHOLDING"=813, "EXP_MAXTHRESHOLDVALUE"=814, "EXP_RUNNING_EXPERIMENT"=815, "EXP_THRESHOLD_DEMAND_UPDATE"=816, "EXP_ROICOUNT"=817, "EXP_ACCUMS"=818, "EXP_CACCUMS"=819, "EXP_CSEQUENTS"=820, "EXP_PHOTON_ESTIMATION_ENABLE"=821, "EXP_PHOTON_MAXTIME"=822, "EXP_PHOTON_MAXTIMEUNIT"=823, "EXP_CUSTOMFILTER_ENABLE"=824, "EXP_CUSTOMFILTER_SIZE"=825, "EXP_LOOKUPTABLE_ENABLE"=826, "EXP_BSHOWWINDOW"=827, "EXP_BBACKSUBTRACT"=828, "EXP_BDOFLATFIELD"=829, "EXP_ASCIIOUTPUTFILE"=830, "EXP_ASCIIOUTPUT_DELIMITER"=831, "EXP_ASCIIOUTPUT_TERMINATOR"=832, "EXP_FFTYPE"=833, "EXP_BGTYPE"=834, "EXP_COSGRASS"=835, "EXP_RUNASCONFIRM"=836, "EXP_RUNASRUNACCESS"=837, "EXP_DATAFILETYPE"=838, "EXP_ROTATE"=839, "EXP_FLIP"=840, "EXP_REVERSE"=841, "EXP_SWBINNING"=842, "EXP_AUTOSTORE"=843, "EXP_XBINNED"=844, "EXP_YBINNED"=845, "EXP_NUMPATTERNS"=846, "EXP_EXPERIMENTTIME"=847, "EXP_ASYNCSEQUENTIALS"=848, "EXP_SEQUENTIALS"=849, "EXP_CSEQUENTIALS"=850, "EXP_AUTOD"=851, "EXP_EXPOSURETIME"=852, "EXP_EXPOSURETIME_UNITS"=853, "EXP_ACQMODE"=854, "EXP_DMASIZE_PVCAM"=855, "EXP_INITIALIZE"=856, "EXP_CELL_X_SIZE"=857, "EXP_CELL_Y_SIZE"=858, "EXP_X_GAP_SIZE"=859, "EXP_Y_GAP_SIZE"=860] ("Param")
            # "get current temperature"
            n132 = local read "experiment reference"() -> (w183:refnum<k7>)
            n133 = invoke class="IExpSetup2" method="GetParam"(reference=w183, "Param"=w184) -> ("GetParam"=w186:variant)  [unwired: 3 in, 4 out]
            n134 = Variant To Data(type=0.0, Variant=w186) -> (data=w182:dbl)  [unwired: 1 in, 1 out]
            n135 = local write "OMA V temp"(w182) -> ()
          }
          frame 5 {
            w188 = 139 items=["EXP_ETACTUAL"=1, "EXP_SEQUENTS"=2, "EXP_ERROR"=3, "EXP_GETCAPS"=4, "EXP_GETPLSR"=5, "EXP_DETECTOR_BIT"=16, "EXP_RUNNING_APP"=23, "EXP_VIDEO_TYPE"=24, "EXP_CUSTOM_VIDEO_X"=25, "EXP_CUSTOM_VIDEO_Y"=26, "EXP_CUSTOM_VIDEO_FSTWIDTH"=27, "EXP_CUSTOM_VIDEO_LSTWIDTH"=28, "EXP_VIDEO_XDIM"=29, "EXP_VIDEO_YDIM"=30, "EXP_VIDEO_MAX_ZOOM"=31, "EXP_VIDEO_HORZ_PAN"=32, "EXP_VIDEO_VERT_PAN"=33, "EXP_WORD_MULTIPLIER"=34, "EXP_TARGET_ID"=35, "EXP_ADAPTER_ID"=36, "EXP_NUMADAPTORS"=37, "EXP_FORCE_PP_INIT"=38, "EXP_NOP_ADC"=39, "EXP_ACTUAL_TEMP"=40, "EXP_FORCE_AUTOSTOP"=41, "EXP_DEFAULT_VTCLK"=42, "EXP_MIN_VTCLK"=43, "EXP_MAX_VTCLK"=44, "EXP_DEFAULT_HTCLK"=45, "EXP_MIN_HTCLK"=46, "EXP_MAX_HTCLK"=47, "EXP_TIMING_STYLE"=48, "EXP_HEADSELECT"=49, "EXP_HORZPHASE"=50, "EXP_VERTPHASE"=51, "EXP_SPECIAL_SPEED"=52, "EXP_PRE_STRIPS"=53, "EXP_POST_STRIPS"=54, "EXP_PRE_LINES"=55, "EXP_POST_LINES"=56, "EXP_ACTIVE_LINES"=57, "EXP_ACTIVE_STRIPS"=58, "EXP_XFER_EXTRA"=59, "EXP_MIN_BLOCK"=60, "EXP_NUM_MIN_BLOCK"=61, "EXP_LOGIC_OUTPUT"=66, "EXP_VIDEO_BLANK"=67, "EXP_ZOOM_MODE_VIDEO"=68, "EXP_LEVEL_SYNC"=69, "EXP_DISABLE_LASER"=70, "EXP_ACQBACK_SHUTTER"=71, "EXP_ACQFLAT_SHUTTER"=72, "EXP_SMALL_CCD_MINEXP"=73, "EXP_LARGE_CCD_MINEXP"=74, "EXP_GATING_MODE"=75, "EXP_ILME_B1X"=76, "EXP_ILME_B2X"=77, "EXP_ILME_D1X"=78, "EXP_ILME_D2X"=79, "EXP_ILME_D4X"=80, "EXP_INIT_HW_ACCUM"=81, "EXP_5X_GAIN_ENABLE"=82, "EXP_RET_SRCCMP"=83, "EXP_EVENT_HANDLE"=84, "EXP_READOUT_MODE"=85, "EXP_SHUTTER_TYPE"=86, "EXP_USER_DEFINED_CHIP"=87, "EXP_USER_DEFINED_TIMING"=88, "EXP_CONTROLLER_VERSION"=89, "EXP_GET_CONTROLLER_VER"=90, "EXP_TTL_LINES"=91, "EXP_BIT_ADJUST"=92, "EXP_RESOLUTION"=93, "EXP_GAIN"=94, "EXP_ADC_RATE"=95, "EXP_ADC_TYPE"=96, "EXP_NUMBER_OF_CLEANS"=97, "EXP_NUM_OF_STRIPS_PER_CLN"=98, "EXP_INTERFACE_CARD"=99, "EXP_INTERRUPT"=100, "EXP_IO_ADDRESS1"=101, "EXP_IO_ADDRESS2"=102, "EXP_IO_ADDRESS3"=103, "EXP_HW_ROI"=104, "EXP_HW_BINNING"=105, "EXP_EDGE_TRIGGER"=106, "EXP_SHUTTER_CONTROL"=107, "EXP_RS170"=108, "EXP_RS170_COMPLEX"=109, "EXP_HW_RS170_LUT"=110, "EXP_RS170_INTENSITY_SCALING"=111, "EXP_RS170_OFFSET"=112, "EXP_RS170_PAN"=113, "EXP_RS170_ZOOM2X"=114, "EXP_RS170_ZOOM4X"=115, "EXP_RS170_BINNING"=116, "EXP_RS170_DECIMATION"=117, "EXP_HW_ACCUM"=118, "EXP_SHT_PREOPEN"=119, "EXP_STORE_STROBE"=120, "EXP_CONT_CLNS"=121, "EXP_TIMING_MODE"=122, "EXP_EXT_TRIGGER"=123, "EXP_EVENT_COUNTER"=124, "EXP_SW_TRIGGER"=125, "EXP_KINETICS_WINDOWSIZE"=126, "EXP_EXPOSURE"=127, "EXP_CONTROLLER_NAME"=128, "EXP_CCD_CHIP_NAME"=129, "EXP_BSWBINNING"=297, "EXP_EDGEENHANCE"=130, "EXP_BOXVIDEOGAIN"=131, "EXP_HSHADING_VALUE"=132, "EXP_VSHADING_VALUE"=133, "EXP_EDGEENHANCE_FLAG"=134, "EXP_SHADING_FLAG"=135, "EXP_GRAYSCALE"=136, "EXP_OFFSET"=137, "EXP_CCDGAIN"=138, "EXP_TEMPERATURE"=139, "EXP_MCPVOLTAGE"=140, "EXP_BOXEXPOSURE"=141, "EXP_ABC_FLAG"=142, "EXP_GAMMA_FLAG"=143, "EXP_AUTOBLACK_FLAG"=144, "EXP_AGC_FLAG"=145, "EXP_ODD_FIELD"=146, "EXP_FIELD_SELECT"=147, "EXP_RESET"=148, "EXP_EXTERN_ENABLE"=149, "EXP_CONTROLLERS_SUPPORTED"=150, "EXP_VTCLK"=151, "EXP_HTCLK"=152, "EXP_GATE_VS_CW"=153, "EXP_COM_PORT"=154, "EXP_US_UNITS"=156, "EXP_MS_UNITS"=157, "EXP_SEC_UNITS"=158, "EXP_MIN_UNITS"=159, "EXP_HRS_UNITS"=160, "EXP_FRAME_UNITS"=161, "EXP_SYNC_ASYNC"=162, "EXP_FOCUS_NFRAME"=163, "EXP_TIMEOUT"=164, "EXP_TIMEOUT_DEFAULT"=165, "EXP_HW_AUTOSTOP"=166, "EXP_RS170_INTEN_OFFSET"=167, "EXP_CONTROLLER_ALIVE"=168, "EXP_FOCUS_TYPE"=169, "EXP_FOCUS_ZOOM"=170, "EXP_FOCUS_PAN"=171, "EXP_MULTI_TAP_ROI"=172, "EXP_USE_INTERUPTS"=173, "EXP_DATA_ACQ_STATE"=174, "EXP_VERIFY_GOOD_VALUES"=175, "EXP_WHITE_CLAMP"=176, "EXP_BLACK_CLAMP"=177, "EXP_DELAY_TIME"=178, "EXP_READOUT_TIME"=179, "EXP_SW_DIAG"=180, "EXP_DIAG1"=181, "EXP_DIAG2"=182, "EXP_DIAG3"=183, "EXP_DIAG4"=184, "EXP_DIAG5"=185, "EXP_AorB_GROUP"=186, "EXP_ABSORBANCE_FLAG"=187, "EXP_ABSORBANCE_METHOD"=188, "EXP_ABSORBANCE_STRIPNUM"=189, "EXP_DMASIZE_VIA_DRIVER"=190, "EXP_DRIVERVERSION"=191, "EXP_NUM_DEVICES"=192, "EXP_ECPDMA_CHANNEL"=193, "EXP_CUSTOM_SHUTTER"=194, "EXP_ADC_OFFSET"=195, "EXP_CURRENT_READOUT_MODE"=196, "EXP_BANK_ADD"=197, "EXP_LUT_BANK"=198, "EXP_SETUP_STATUS"=201, "EXP_XY_GROUPING"=239, "EXP_MESSAGES_FLAG"=240, "EXP_TTL_LINE_TO_WAIT"=253, "EXP_DATA_COLLECTION_MODE"=258, "EXP_DATA_COLLECTION_TYPE"=262, "EXP_SKIPFRAMES"=274, "EXP_CLR_INT_CNTR"=276, "EXP_ENABLE_INT_CNTR"=277, "EXP_INT_CNTR"=278, "EXP_INTERNAL_SYNC_SRC"=279, "EXP_SW_EXTSYNC"=280, "EXP_PTG_PRESENT"=281, "EXP_ELEC_SHT"=282, "EXP_BOARDS_WITH_NVRAM"=283, "EXP_ANLGMASTER_ST143"=284, "EXP_ANLGSLAVE_ST143"=285, "EXP_DISPLAY_ST143"=286, "EXP_INTRFACE_ST143"=287, "EXP_SCANCONTROL_ST143"=288, "EXP_NUMBERFRAMES_IRQ"=204, "EXP_COOL_TYPE"=214, "EXP_HD_TYPE"=215, "EXP_INTENSIFER_GAIN"=216, "EXP_SHT_GATE_MODE"=217, "EXP_HD_CHECK"=218, "EXP_AMP_MODE"=219, "EXP_AMP_DIALOG"=247, "EXP_ANALOG_GAIN"=220, "EXP_HW_FIXES"=221, "EXP_PCI_CARDS"=222, "EXP_NOT_REVERSE"=223, "EXP_LOAD_NVRAM_DEFAULTS"=234, "EXP_CNTR_BRD"=235, "EXP_XDIMHW"=237, "EXP_YDIMHW"=238, "EXP_SPECIAL_FAST_RDOUT"=254, "EXP_SPCL_FAST_Y_DIM"=255, "EXP_SPCL_FAST_X_DIM"=256, "EXP_SPCL_FAST_Y_INDEX"=257, "EXP_SHUTTER_COMP_TIME_MS"=266, "EXP_NVRAM_AVAIL"=267, "EXP_NUMBER_AGAIN_AVAIL"=269, "EXP_SENSOR_TYPE"=270, "EXP_EVENT_TYPE"=292, "EXP_ANTI_BLOOMING"=293, "EXP_FAST_PULSE_ENABLE"=233, "EXP_USE_HEADCALIB"=296, "EXP_TEMP_STATUS"=301, "EXP_MULTIPLE_READMODES_LIVE"=302, "EXP_FIRST_ACQUIRE_FLAG"=303, "EXP_ANTI_BLOOMING_CONTROL"=304, "EXP_PRE_HORZ_DELAY"=305, "EXP_NVRAM_TRIES"=306, "EXP_XASCEND"=307, "EXP_YASCEND"=308, "EXP_ALT_TIMING"=309, "EXP_SHUTTER_PRE_COMP"=310, "EXP_PVCAM_POSSIBLE"=311, "EXP_ADC_IN_NVRAM"=312, "EXP_PASSTHRU_MODE"=313, "EXP_FIRMWAREVERSION"=314, "EXP_IMMEDIATE_SHUTTER"=315, "EXP_STAGE2_TEMP"=316, "EXP_AVGAIN_ENABLED"=317, "EXP_AVGAIN_SETPOINT"=318, "EXP_AVGAIN"=319, "EXP_AVGAIN_CALIB_TEMP"=320, "EXP_AVGAIN_CALIB_COEFF1"=321, "EXP_AVGAIN_CALIB_COEFF2"=322, "EXP_AVGAIN_CALIB_COEFF3"=323, "EXP_AVGAIN_CALIB_COEFF4"=324, "EXP_AVGAIN_CALIB_COEFF5"=325, "EXP_FORCE_READOUT_MODE"=326, "EXP_RESET_DATACOLLECTION"=327, "EXP_ACTIVE_SUBFRAME"=328, "EXP_PV_READOUT_PORT"=514, "EXP_COOLING_FAN_CTRL"=339, "EXP_SHTR_RES"=343, "EXP_PBC"=351, "EXP_PREEXP_CLEANS"=354, "EXP_TTL_CTRL"=355, "EXP_PAR_SHIFT_INDEX"=547, "EXP_LOGIC_OUTPUT_INVERT"=548, "EXP_CLASSNAME"=775, "EXP_FLATFLDNAME"=776, "EXP_DARKNAME"=777, "EXP_SETUPNAME"=778, "EXP_ACCESSNAME"=779, "EXP_DATFILENAME"=780, "EXP_ABSORBFILENAME"=781, "EXP_BLEMISHFILENAME"=782, "EXP_COSMICFILENAME"=783, "EXP_FILEINCBASENAME"=784, "EXP_YTNAME"=785, "EXP_DEVNAME"=786, "EXP_USEROI"=787, "EXP_DOBLEMISH"=788, "EXP_DOABSORB"=789, "EXP_DOCOSMIC"=790, "EXP_COSMICSENS"=791, "EXP_ABSORBSTRIP"=792, "EXP_DATATYPE"=793, "EXP_OVERWRITECONFIRM"=794, "EXP_FILEINCENABLE"=795, "EXP_FILEINCCOUNT"=796, "EXP_RUNNING"=797, "EXP_SAVEROPT"=798, "EXP_TIME_UNITS"=799, "EXP_FILEACCESS"=800, "EXP_AUTOSAVE"=801, "EXP_NEWWINDOW"=802, "EXP_XDIM"=803, "EXP_YDIM"=804, "EXP_XDIMDET"=805, "EXP_YDIMDET"=806, "EXP_ROIMODE"=807, "EXP_NUMREPEATSEXP"=808, "EXP_NUMACCUMSEXP"=809, "EXP_THREADSTATE"=810, "EXP_USEMINTHRESHOLDING"=811, "EXP_MINTHRESHOLDVALUE"=812, "EXP_USEMAXTHRESHOLDING"=813, "EXP_MAXTHRESHOLDVALUE"=814, "EXP_RUNNING_EXPERIMENT"=815, "EXP_THRESHOLD_DEMAND_UPDATE"=816, "EXP_ROICOUNT"=817, "EXP_ACCUMS"=818, "EXP_CACCUMS"=819, "EXP_CSEQUENTS"=820, "EXP_PHOTON_ESTIMATION_ENABLE"=821, "EXP_PHOTON_MAXTIME"=822, "EXP_PHOTON_MAXTIMEUNIT"=823, "EXP_CUSTOMFILTER_ENABLE"=824, "EXP_CUSTOMFILTER_SIZE"=825, "EXP_LOOKUPTABLE_ENABLE"=826, "EXP_BSHOWWINDOW"=827, "EXP_BBACKSUBTRACT"=828, "EXP_BDOFLATFIELD"=829, "EXP_ASCIIOUTPUTFILE"=830, "EXP_ASCIIOUTPUT_DELIMITER"=831, "EXP_ASCIIOUTPUT_TERMINATOR"=832, "EXP_FFTYPE"=833, "EXP_BGTYPE"=834, "EXP_COSGRASS"=835, "EXP_RUNASCONFIRM"=836, "EXP_RUNASRUNACCESS"=837, "EXP_DATAFILETYPE"=838, "EXP_ROTATE"=839, "EXP_FLIP"=840, "EXP_REVERSE"=841, "EXP_SWBINNING"=842, "EXP_AUTOSTORE"=843, "EXP_XBINNED"=844, "EXP_YBINNED"=845, "EXP_NUMPATTERNS"=846, "EXP_EXPERIMENTTIME"=847, "EXP_ASYNCSEQUENTIALS"=848, "EXP_SEQUENTIALS"=849, "EXP_CSEQUENTIALS"=850, "EXP_AUTOD"=851, "EXP_EXPOSURETIME"=852, "EXP_EXPOSURETIME_UNITS"=853, "EXP_ACQMODE"=854, "EXP_DMASIZE_PVCAM"=855, "EXP_INITIALIZE"=856, "EXP_CELL_X_SIZE"=857, "EXP_CELL_Y_SIZE"=858, "EXP_X_GAP_SIZE"=859, "EXP_Y_GAP_SIZE"=860] ("Param")
            # "set OMA V temperature"
            n136 = local read "experiment reference"() -> (w187:refnum<k7>)
            n137 = local read "Set Temperature (°C)"() -> (w189:i8)
            n138 = invoke class="IExpSetup2" method="SetParam"(reference=w187, "Param"=w188, "pSetVal"=w189) -> ()  [unwired: 2 in, 5 out]
          }
          frame 6 {
            # "Change spectro wavelength"
            n139 = flat-sequence {
              frame #0 {
                w193 = 87 items=["SPT_NOCMD", "SPT_SPECTS_SUPPORTED", "SPT_TYPE", "SPT_CALIBUPDATE", "SPT_GRATINGWARNING", "SPT_LASERWARNING", "SPT_FORCEMOVE", "SPT_INSTNAME", "SPT_USERNAME", "SPT_INSTUSERNAME", "SPT_INSTCOMMNAME", "SPT_WAVE_ORIENTED", "SPT_NUMSTAGES", "SPT_GRATINGSPERTURRET", "SPT_CURRGRATING", "SPT_GRAT_BACKLASH_REQ", "SPT_GRATINGBACKLASHSTEPS", "SPT_NEEDINIT", "SPT_NEED_HWINIT", "SPT_MOTOR", "SPT_ARRAYSIZE", "SPT_ROI_CENTER", "SPT_ORDER", "SPT_CUR_GRATING", "SPT_NEW_GRATING", "SPT_SEQUENCER_STATE", "SPT_NUMTURRETS", "SPT_CURRTURRET", "SPT_DO_RESET", "SPT_SLAVE_CNT", "SPT_NUM_STEPS", "SPT_PIXEL_WIDTH", "SPT_GRAT_USERNAME", "SPT_GRAT_GROOVES", "SPT_GRAT_CENTERADJ", "SPT_GRAT_LINEAR_ADJ", "SPT_GRAT_SLOPE_ADJ", "SPT_GRAT_FOCAL_LEN", "SPT_GRAT_INCL_ANGLE", "SPT_GRAT_DETECT_ANGLE", "SPT_GRAT_MAG", "SPT_ACCESS_ALL_GRAT_SPEEDS", "SPT_SPEED_FOR_EACH_GRATING", "SPT_NUM_SETABLE_GRAT_SPEEDS", "SPT_GRATING_SPEED", "SPT_GRATING_SPEED_MIN", "SPT_GRATING_SPEED_MAX", "SPT_GRAT_REF_GRATING", "SPT_GRAT_STEPSPUNIT", "SPT_GRAT_OFFSET", "SPT_GRAT_ADJUST", "SPT_GRAT_LO_CAL_WAVE", "SPT_GRAT_HI_CAL_WAVE", "SPT_GRAT_LO_POS_WAVE", "SPT_GRAT_HI_POS_WAVE", "SPT_GRAT_REF_WAVE", "SPT_NUM_SLITS", "SPT_SLIT_ENABLED", "SPT_SLIT_LOCATION", "SPT_SLIT_CURPOSITION", "SPT_SLIT_NEWPOSITION", "SPT_SPEED_FOR_EACH_SLIT", "SPT_NUM_SETABLE_SLIT_SPEEDS", "SPT_SLIT_SPEED", "SPT_SLIT_SPEED_MIN", "SPT_SLIT_SPEED_MAX", "SPT_SLIT_STEPSPUNIT", "SPT_SLIT_BACKLASH_REQ", "SPT_SLIT_BACKLASH", "SPT_NUMMIRRORS", "SPT_MIRROR_ENABLED", "SPT_MIRROR_LOCATION", "SPT_MIRROR_CURPOSITION", "SPT_MIRROR_NEWPOSITION", "SPT_OFFSET_AVAIL", "SPT_ADJUST_AVAIL", "SPT_COUNTERSUPPORTED", "SPT_POSITIONSUPPORTED", "SPT_AUTOCALIBSUPPORTED", "SPT_POSITIONMEMORY", "SPT_NUMCOEFFS", "SPT_COEFF", "SPT_SERIAL_IO_SUPPORTED", "SPT_GPIB_IO_SUPPORTED", "SPT_OFFSETADJUSTSUPPORTED", "SPT_LINEARADJUSTSUPPORTED", "SPT_WL_PRECISION", "SPT_NEW_POSITION", "SPT_CUR_POSITION", "SPT_ROI_OFFSET", "SPT_MARK_EXCITATION", "SPT_EXCITATION", "SPT_STEP_SIZE", "SPT_STARTING_WAVELENGTH", "SPT_ENDING_WAVELENGTH", "SPT_MIN_OVERLAP", "SPT_GLUE_BIN_SIZE", "SPT_STARTING_CENTER_WAVE", "SPT_DFLT_BIN_FLAG", "SPT_REPOSITION_FLAG", "SPT_PORT_TYPE", "SPT_PORT_NAME", "SPT_PORT_ADDRESS", "SPT_CUSTOM_NAME", "SPT_GLUE_FILE_NAME", "SPT_DEF_GRATINGSPERTURRET", "SPT_DEF_FOCALLENGTH", "SPT_DEF_INCLUSIONANGLE", "SPT_DEF_DETECTORANGLE", "SPT_DEF_MAGNIFICATION", "SPT_DEF_PIXELWIDTH", "SPT_DEF_REFGRATING", "SPT_DEF_GROOVES", "SPT_DEF_GRAT_USERNAME", "SPT_DEF_GRAT_STEPSPERUNIT", "SPT_DEF_GRAT_SPEED", "SPT_DEF_GRAT_MAX_SPEED", "SPT_DEF_GRAT_MIN_SPEED", "SPT_DEF_GRAT_BACKLASH_REQ", "SPT_DEF_GRAT_BACKLASHSTEPS", "SPT_DEF_SLIT_STEPSPERUNIT", "SPT_DEF_SLIT_SPEED", "SPT_DEF_SLIT_MAX_SPEED", "SPT_DEF_SLIT_MIN_SPEED", "SPT_DEF_SLIT_BACKLASH_REQ", "SPT_DEF_SLIT_BACKLASHSTEPS", "SPT_MIN_SLIT_POS", "SPT_MAX_SLIT_POS", "SPT_SLIT_POS_UNITS", "SPT_DEF_PORTADDRESS", "SPT_DEF_PORTNAME", "SPT_DEF_PORTTYPE", "SPT_SETTINGSLOADED", "SPT_BAUDRATE", "SPT_DATABITS", "SPT_STOPBITS", "SPT_PARITY", "SPT_CTSFLOW", "SPT_MODELNAME", "SPT_SERIALNUMBER", "SPT_VALIDITYFLAG", "SPT_EXISTS", "SPT_CHANGED", "SPT_MANUFACTURE_NAME", "SPT_TRIMTOPRECISION", "SPT_GRAT_TYPE", "SPT_COMM_PORT", "SPT_RESET_WAIT_FLAG", "SPT_DEMOPORT_FLAG", "SPT_INST_NUMTURRETS", "SPT_INST_CURR_TURRET", "SPT_INST_GRAT_GROOVES", "SPT_INST_CUR_GRAT_NUM", "SPT_INST_GRAT_USERNAME", "SPT_INST_CUR_GRAT_POS", "SPT_INST_GRAT_SPEED", "SPT_INST_MODELNAME", "SPT_INST_SERIALNUMBER", "SPT_INST_NUM_SLITS", "SPT_INST_SLIT_LOCATION", "SPT_INST_SLIT_POSITION", "SPT_INST_SLIT_SPEED", "SPT_INST_NUM_MIRRORS", "SPT_INST_MIRROR_LOCATION", "SPT_INST_MIRROR_POSITION", "SPT_ACTIVE_MIRROR_LOC", "SPT_ACTIVE_MIRROR_POS", "SPT_GRAT_MOVE_MODE", "SPT_ACTIVE_GRAT_POS", "SPT_ACTIVE_GRATING_NUM", "SPT_ACTIVE_SLIT_LOC", "SPT_ACTIVE_SLIT_POS", "SPT_STEP_ERROR_CODE", "SPT_ERROR_CODE", "SPT_ACTIVE_TURRET_NUM", "SPT_DLL_INDEX", "SPT_NMTOSTEPS_WL", "SPT_NMTOSTEPS_STEPS", "SPT_NUM_SPECT_DLLS", "SPT_NUM_SPECT_AVAIL", "SPT_MESSAGE_WND_HNDL", "SPT_MUTEX", "SPT_CALC_WL_INCENTERWL", "SPT_CALC_WL_INDIST", "SPT_CALC_WL_OUTWL", "SPT_ARRAY_CENTER", "SPT_CURR_CALIB_PTR", "SPT_DLL_TYPE", "SPT_NEW_SLIT_INDEX", "SPT_NEW_MIRROR_INDEX", "SPT_CALCSLOPEADJ_WL", "SPT_CALCSLOPEADJ_SLOPE", "SPT_MAX_GRATINGS_PER_TURRET", "SPT_MAX_NUM_TURRETS", "SPT_MAX_NUM_MIRRORS", "SPT_MAX_NUM_SLITS", "SPT_GRATING_SPEED_INDEX", "SPT_SLIT_SPEED_INDEX", "SPT_GRATING_SPEED_UNITS", "SPT_GRATING_SPEED_NAME", "SPT_SLIT_SPEED_UNITS", "SPT_SLIT_SPEED_NAME", "SPT_NEED_GRATING_SPEED_SET", "SPT_NEED_SLIT_SPEED_SET", "SPT_GRAT_STEPSUNIT_UNIT", "SPT_SLIT_STEPSUNIT_UNIT", "SPT_PROCESS_MOVE_STATUS", "SPT_RESET", "SPT_RESET_TIMEOUT_MS", "SPT_GENERIC_DLG_MAIN_TITLE", "SPT_GENERIC_DLG_INDEX", "SPT_GENERIC_EDITBOX_TXT", "SPT_GENERIC_EDITBOX", "SPT_GENERIC_SPINBUTTON", "SPT_GENERIC_CHECKBOX_TXT", "SPT_GENERIC_CHECKBOX", "SPT_GENERIC_COMBOBOX_TXT", "SPT_GENERIC_COMBOBOX", "SPT_GENERIC_RADIOBUTTON_GRP", "SPT_GENERIC_RADIOBUTTON_TXT", "SPT_GENERIC_RADIOBUTTON", "SPT_DLL_PRODUCT_VERSION", "SPT_DLL_FILE_VERSION", "SPT_END_OF_LIST"] ("Param")
                n140 = local read "Wavelength (nm)"() -> (w191:dbl)
                n141 = local read "MonoRef"() -> (w192:refnum<k7>)
                n142 = invoke class="ISpectroObj" method="SetParam"(reference=w192, "Param"=w193, "pSetVal"=w191) -> (reference out=w190:refnum<k7>)  [unwired: 3 in, 5 out]
                n143 = invoke class="ISpectroObj" method="Move"(reference=w190) -> ()  [unwired: 2 in, 3 out]
              }
              frame #1 {
                n144 = local write "busy"(FALSE ("busy")) -> ()
              }
            }
          }
          frame 7 {
            # "change output port"
          }
          frame 8 {
            # "change grating"
            n145 = flat-sequence {
              frame #0 {
                w201 = 24 items=["SPT_NOCMD", "SPT_SPECTS_SUPPORTED", "SPT_TYPE", "SPT_CALIBUPDATE", "SPT_GRATINGWARNING", "SPT_LASERWARNING", "SPT_FORCEMOVE", "SPT_INSTNAME", "SPT_USERNAME", "SPT_INSTUSERNAME", "SPT_INSTCOMMNAME", "SPT_WAVE_ORIENTED", "SPT_NUMSTAGES", "SPT_GRATINGSPERTURRET", "SPT_CURRGRATING", "SPT_GRAT_BACKLASH_REQ", "SPT_GRATINGBACKLASHSTEPS", "SPT_NEEDINIT", "SPT_NEED_HWINIT", "SPT_MOTOR", "SPT_ARRAYSIZE", "SPT_ROI_CENTER", "SPT_ORDER", "SPT_CUR_GRATING", "SPT_NEW_GRATING", "SPT_SEQUENCER_STATE", "SPT_NUMTURRETS", "SPT_CURRTURRET", "SPT_DO_RESET", "SPT_SLAVE_CNT", "SPT_NUM_STEPS", "SPT_PIXEL_WIDTH", "SPT_GRAT_USERNAME", "SPT_GRAT_GROOVES", "SPT_GRAT_CENTERADJ", "SPT_GRAT_LINEAR_ADJ", "SPT_GRAT_SLOPE_ADJ", "SPT_GRAT_FOCAL_LEN", "SPT_GRAT_INCL_ANGLE", "SPT_GRAT_DETECT_ANGLE", "SPT_GRAT_MAG", "SPT_ACCESS_ALL_GRAT_SPEEDS", "SPT_SPEED_FOR_EACH_GRATING", "SPT_NUM_SETABLE_GRAT_SPEEDS", "SPT_GRATING_SPEED", "SPT_GRATING_SPEED_MIN", "SPT_GRATING_SPEED_MAX", "SPT_GRAT_REF_GRATING", "SPT_GRAT_STEPSPUNIT", "SPT_GRAT_OFFSET", "SPT_GRAT_ADJUST", "SPT_GRAT_LO_CAL_WAVE", "SPT_GRAT_HI_CAL_WAVE", "SPT_GRAT_LO_POS_WAVE", "SPT_GRAT_HI_POS_WAVE", "SPT_GRAT_REF_WAVE", "SPT_NUM_SLITS", "SPT_SLIT_ENABLED", "SPT_SLIT_LOCATION", "SPT_SLIT_CURPOSITION", "SPT_SLIT_NEWPOSITION", "SPT_SPEED_FOR_EACH_SLIT", "SPT_NUM_SETABLE_SLIT_SPEEDS", "SPT_SLIT_SPEED", "SPT_SLIT_SPEED_MIN", "SPT_SLIT_SPEED_MAX", "SPT_SLIT_STEPSPUNIT", "SPT_SLIT_BACKLASH_REQ", "SPT_SLIT_BACKLASH", "SPT_NUMMIRRORS", "SPT_MIRROR_ENABLED", "SPT_MIRROR_LOCATION", "SPT_MIRROR_CURPOSITION", "SPT_MIRROR_NEWPOSITION", "SPT_OFFSET_AVAIL", "SPT_ADJUST_AVAIL", "SPT_COUNTERSUPPORTED", "SPT_POSITIONSUPPORTED", "SPT_AUTOCALIBSUPPORTED", "SPT_POSITIONMEMORY", "SPT_NUMCOEFFS", "SPT_COEFF", "SPT_SERIAL_IO_SUPPORTED", "SPT_GPIB_IO_SUPPORTED", "SPT_OFFSETADJUSTSUPPORTED", "SPT_LINEARADJUSTSUPPORTED", "SPT_WL_PRECISION", "SPT_NEW_POSITION", "SPT_CUR_POSITION", "SPT_ROI_OFFSET", "SPT_MARK_EXCITATION", "SPT_EXCITATION", "SPT_STEP_SIZE", "SPT_STARTING_WAVELENGTH", "SPT_ENDING_WAVELENGTH", "SPT_MIN_OVERLAP", "SPT_GLUE_BIN_SIZE", "SPT_STARTING_CENTER_WAVE", "SPT_DFLT_BIN_FLAG", "SPT_REPOSITION_FLAG", "SPT_PORT_TYPE", "SPT_PORT_NAME", "SPT_PORT_ADDRESS", "SPT_CUSTOM_NAME", "SPT_GLUE_FILE_NAME", "SPT_DEF_GRATINGSPERTURRET", "SPT_DEF_FOCALLENGTH", "SPT_DEF_INCLUSIONANGLE", "SPT_DEF_DETECTORANGLE", "SPT_DEF_MAGNIFICATION", "SPT_DEF_PIXELWIDTH", "SPT_DEF_REFGRATING", "SPT_DEF_GROOVES", "SPT_DEF_GRAT_USERNAME", "SPT_DEF_GRAT_STEPSPERUNIT", "SPT_DEF_GRAT_SPEED", "SPT_DEF_GRAT_MAX_SPEED", "SPT_DEF_GRAT_MIN_SPEED", "SPT_DEF_GRAT_BACKLASH_REQ", "SPT_DEF_GRAT_BACKLASHSTEPS", "SPT_DEF_SLIT_STEPSPERUNIT", "SPT_DEF_SLIT_SPEED", "SPT_DEF_SLIT_MAX_SPEED", "SPT_DEF_SLIT_MIN_SPEED", "SPT_DEF_SLIT_BACKLASH_REQ", "SPT_DEF_SLIT_BACKLASHSTEPS", "SPT_MIN_SLIT_POS", "SPT_MAX_SLIT_POS", "SPT_SLIT_POS_UNITS", "SPT_DEF_PORTADDRESS", "SPT_DEF_PORTNAME", "SPT_DEF_PORTTYPE", "SPT_SETTINGSLOADED", "SPT_BAUDRATE", "SPT_DATABITS", "SPT_STOPBITS", "SPT_PARITY", "SPT_CTSFLOW", "SPT_MODELNAME", "SPT_SERIALNUMBER", "SPT_VALIDITYFLAG", "SPT_EXISTS", "SPT_CHANGED", "SPT_MANUFACTURE_NAME", "SPT_TRIMTOPRECISION", "SPT_GRAT_TYPE", "SPT_COMM_PORT", "SPT_RESET_WAIT_FLAG", "SPT_DEMOPORT_FLAG", "SPT_INST_NUMTURRETS", "SPT_INST_CURR_TURRET", "SPT_INST_GRAT_GROOVES", "SPT_INST_CUR_GRAT_NUM", "SPT_INST_GRAT_USERNAME", "SPT_INST_CUR_GRAT_POS", "SPT_INST_GRAT_SPEED", "SPT_INST_MODELNAME", "SPT_INST_SERIALNUMBER", "SPT_INST_NUM_SLITS", "SPT_INST_SLIT_LOCATION", "SPT_INST_SLIT_POSITION", "SPT_INST_SLIT_SPEED", "SPT_INST_NUM_MIRRORS", "SPT_INST_MIRROR_LOCATION", "SPT_INST_MIRROR_POSITION", "SPT_ACTIVE_MIRROR_LOC", "SPT_ACTIVE_MIRROR_POS", "SPT_GRAT_MOVE_MODE", "SPT_ACTIVE_GRAT_POS", "SPT_ACTIVE_GRATING_NUM", "SPT_ACTIVE_SLIT_LOC", "SPT_ACTIVE_SLIT_POS", "SPT_STEP_ERROR_CODE", "SPT_ERROR_CODE", "SPT_ACTIVE_TURRET_NUM", "SPT_DLL_INDEX", "SPT_NMTOSTEPS_WL", "SPT_NMTOSTEPS_STEPS", "SPT_NUM_SPECT_DLLS", "SPT_NUM_SPECT_AVAIL", "SPT_MESSAGE_WND_HNDL", "SPT_MUTEX", "SPT_CALC_WL_INCENTERWL", "SPT_CALC_WL_INDIST", "SPT_CALC_WL_OUTWL", "SPT_ARRAY_CENTER", "SPT_CURR_CALIB_PTR", "SPT_DLL_TYPE", "SPT_NEW_SLIT_INDEX", "SPT_NEW_MIRROR_INDEX", "SPT_CALCSLOPEADJ_WL", "SPT_CALCSLOPEADJ_SLOPE", "SPT_MAX_GRATINGS_PER_TURRET", "SPT_MAX_NUM_TURRETS", "SPT_MAX_NUM_MIRRORS", "SPT_MAX_NUM_SLITS", "SPT_GRATING_SPEED_INDEX", "SPT_SLIT_SPEED_INDEX", "SPT_GRATING_SPEED_UNITS", "SPT_GRATING_SPEED_NAME", "SPT_SLIT_SPEED_UNITS", "SPT_SLIT_SPEED_NAME", "SPT_NEED_GRATING_SPEED_SET", "SPT_NEED_SLIT_SPEED_SET", "SPT_GRAT_STEPSUNIT_UNIT", "SPT_SLIT_STEPSUNIT_UNIT", "SPT_PROCESS_MOVE_STATUS", "SPT_RESET", "SPT_RESET_TIMEOUT_MS", "SPT_GENERIC_DLG_MAIN_TITLE", "SPT_GENERIC_DLG_INDEX", "SPT_GENERIC_EDITBOX_TXT", "SPT_GENERIC_EDITBOX", "SPT_GENERIC_SPINBUTTON", "SPT_GENERIC_CHECKBOX_TXT", "SPT_GENERIC_CHECKBOX", "SPT_GENERIC_COMBOBOX_TXT", "SPT_GENERIC_COMBOBOX", "SPT_GENERIC_RADIOBUTTON_GRP", "SPT_GENERIC_RADIOBUTTON_TXT", "SPT_GENERIC_RADIOBUTTON", "SPT_DLL_PRODUCT_VERSION", "SPT_DLL_FILE_VERSION", "SPT_END_OF_LIST"] ("Param")
                w198 = 87 items=["SPT_NOCMD", "SPT_SPECTS_SUPPORTED", "SPT_TYPE", "SPT_CALIBUPDATE", "SPT_GRATINGWARNING", "SPT_LASERWARNING", "SPT_FORCEMOVE", "SPT_INSTNAME", "SPT_USERNAME", "SPT_INSTUSERNAME", "SPT_INSTCOMMNAME", "SPT_WAVE_ORIENTED", "SPT_NUMSTAGES", "SPT_GRATINGSPERTURRET", "SPT_CURRGRATING", "SPT_GRAT_BACKLASH_REQ", "SPT_GRATINGBACKLASHSTEPS", "SPT_NEEDINIT", "SPT_NEED_HWINIT", "SPT_MOTOR", "SPT_ARRAYSIZE", "SPT_ROI_CENTER", "SPT_ORDER", "SPT_CUR_GRATING", "SPT_NEW_GRATING", "SPT_SEQUENCER_STATE", "SPT_NUMTURRETS", "SPT_CURRTURRET", "SPT_DO_RESET", "SPT_SLAVE_CNT", "SPT_NUM_STEPS", "SPT_PIXEL_WIDTH", "SPT_GRAT_USERNAME", "SPT_GRAT_GROOVES", "SPT_GRAT_CENTERADJ", "SPT_GRAT_LINEAR_ADJ", "SPT_GRAT_SLOPE_ADJ", "SPT_GRAT_FOCAL_LEN", "SPT_GRAT_INCL_ANGLE", "SPT_GRAT_DETECT_ANGLE", "SPT_GRAT_MAG", "SPT_ACCESS_ALL_GRAT_SPEEDS", "SPT_SPEED_FOR_EACH_GRATING", "SPT_NUM_SETABLE_GRAT_SPEEDS", "SPT_GRATING_SPEED", "SPT_GRATING_SPEED_MIN", "SPT_GRATING_SPEED_MAX", "SPT_GRAT_REF_GRATING", "SPT_GRAT_STEPSPUNIT", "SPT_GRAT_OFFSET", "SPT_GRAT_ADJUST", "SPT_GRAT_LO_CAL_WAVE", "SPT_GRAT_HI_CAL_WAVE", "SPT_GRAT_LO_POS_WAVE", "SPT_GRAT_HI_POS_WAVE", "SPT_GRAT_REF_WAVE", "SPT_NUM_SLITS", "SPT_SLIT_ENABLED", "SPT_SLIT_LOCATION", "SPT_SLIT_CURPOSITION", "SPT_SLIT_NEWPOSITION", "SPT_SPEED_FOR_EACH_SLIT", "SPT_NUM_SETABLE_SLIT_SPEEDS", "SPT_SLIT_SPEED", "SPT_SLIT_SPEED_MIN", "SPT_SLIT_SPEED_MAX", "SPT_SLIT_STEPSPUNIT", "SPT_SLIT_BACKLASH_REQ", "SPT_SLIT_BACKLASH", "SPT_NUMMIRRORS", "SPT_MIRROR_ENABLED", "SPT_MIRROR_LOCATION", "SPT_MIRROR_CURPOSITION", "SPT_MIRROR_NEWPOSITION", "SPT_OFFSET_AVAIL", "SPT_ADJUST_AVAIL", "SPT_COUNTERSUPPORTED", "SPT_POSITIONSUPPORTED", "SPT_AUTOCALIBSUPPORTED", "SPT_POSITIONMEMORY", "SPT_NUMCOEFFS", "SPT_COEFF", "SPT_SERIAL_IO_SUPPORTED", "SPT_GPIB_IO_SUPPORTED", "SPT_OFFSETADJUSTSUPPORTED", "SPT_LINEARADJUSTSUPPORTED", "SPT_WL_PRECISION", "SPT_NEW_POSITION", "SPT_CUR_POSITION", "SPT_ROI_OFFSET", "SPT_MARK_EXCITATION", "SPT_EXCITATION", "SPT_STEP_SIZE", "SPT_STARTING_WAVELENGTH", "SPT_ENDING_WAVELENGTH", "SPT_MIN_OVERLAP", "SPT_GLUE_BIN_SIZE", "SPT_STARTING_CENTER_WAVE", "SPT_DFLT_BIN_FLAG", "SPT_REPOSITION_FLAG", "SPT_PORT_TYPE", "SPT_PORT_NAME", "SPT_PORT_ADDRESS", "SPT_CUSTOM_NAME", "SPT_GLUE_FILE_NAME", "SPT_DEF_GRATINGSPERTURRET", "SPT_DEF_FOCALLENGTH", "SPT_DEF_INCLUSIONANGLE", "SPT_DEF_DETECTORANGLE", "SPT_DEF_MAGNIFICATION", "SPT_DEF_PIXELWIDTH", "SPT_DEF_REFGRATING", "SPT_DEF_GROOVES", "SPT_DEF_GRAT_USERNAME", "SPT_DEF_GRAT_STEPSPERUNIT", "SPT_DEF_GRAT_SPEED", "SPT_DEF_GRAT_MAX_SPEED", "SPT_DEF_GRAT_MIN_SPEED", "SPT_DEF_GRAT_BACKLASH_REQ", "SPT_DEF_GRAT_BACKLASHSTEPS", "SPT_DEF_SLIT_STEPSPERUNIT", "SPT_DEF_SLIT_SPEED", "SPT_DEF_SLIT_MAX_SPEED", "SPT_DEF_SLIT_MIN_SPEED", "SPT_DEF_SLIT_BACKLASH_REQ", "SPT_DEF_SLIT_BACKLASHSTEPS", "SPT_MIN_SLIT_POS", "SPT_MAX_SLIT_POS", "SPT_SLIT_POS_UNITS", "SPT_DEF_PORTADDRESS", "SPT_DEF_PORTNAME", "SPT_DEF_PORTTYPE", "SPT_SETTINGSLOADED", "SPT_BAUDRATE", "SPT_DATABITS", "SPT_STOPBITS", "SPT_PARITY", "SPT_CTSFLOW", "SPT_MODELNAME", "SPT_SERIALNUMBER", "SPT_VALIDITYFLAG", "SPT_EXISTS", "SPT_CHANGED", "SPT_MANUFACTURE_NAME", "SPT_TRIMTOPRECISION", "SPT_GRAT_TYPE", "SPT_COMM_PORT", "SPT_RESET_WAIT_FLAG", "SPT_DEMOPORT_FLAG", "SPT_INST_NUMTURRETS", "SPT_INST_CURR_TURRET", "SPT_INST_GRAT_GROOVES", "SPT_INST_CUR_GRAT_NUM", "SPT_INST_GRAT_USERNAME", "SPT_INST_CUR_GRAT_POS", "SPT_INST_GRAT_SPEED", "SPT_INST_MODELNAME", "SPT_INST_SERIALNUMBER", "SPT_INST_NUM_SLITS", "SPT_INST_SLIT_LOCATION", "SPT_INST_SLIT_POSITION", "SPT_INST_SLIT_SPEED", "SPT_INST_NUM_MIRRORS", "SPT_INST_MIRROR_LOCATION", "SPT_INST_MIRROR_POSITION", "SPT_ACTIVE_MIRROR_LOC", "SPT_ACTIVE_MIRROR_POS", "SPT_GRAT_MOVE_MODE", "SPT_ACTIVE_GRAT_POS", "SPT_ACTIVE_GRATING_NUM", "SPT_ACTIVE_SLIT_LOC", "SPT_ACTIVE_SLIT_POS", "SPT_STEP_ERROR_CODE", "SPT_ERROR_CODE", "SPT_ACTIVE_TURRET_NUM", "SPT_DLL_INDEX", "SPT_NMTOSTEPS_WL", "SPT_NMTOSTEPS_STEPS", "SPT_NUM_SPECT_DLLS", "SPT_NUM_SPECT_AVAIL", "SPT_MESSAGE_WND_HNDL", "SPT_MUTEX", "SPT_CALC_WL_INCENTERWL", "SPT_CALC_WL_INDIST", "SPT_CALC_WL_OUTWL", "SPT_ARRAY_CENTER", "SPT_CURR_CALIB_PTR", "SPT_DLL_TYPE", "SPT_NEW_SLIT_INDEX", "SPT_NEW_MIRROR_INDEX", "SPT_CALCSLOPEADJ_WL", "SPT_CALCSLOPEADJ_SLOPE", "SPT_MAX_GRATINGS_PER_TURRET", "SPT_MAX_NUM_TURRETS", "SPT_MAX_NUM_MIRRORS", "SPT_MAX_NUM_SLITS", "SPT_GRATING_SPEED_INDEX", "SPT_SLIT_SPEED_INDEX", "SPT_GRATING_SPEED_UNITS", "SPT_GRATING_SPEED_NAME", "SPT_SLIT_SPEED_UNITS", "SPT_SLIT_SPEED_NAME", "SPT_NEED_GRATING_SPEED_SET", "SPT_NEED_SLIT_SPEED_SET", "SPT_GRAT_STEPSUNIT_UNIT", "SPT_SLIT_STEPSUNIT_UNIT", "SPT_PROCESS_MOVE_STATUS", "SPT_RESET", "SPT_RESET_TIMEOUT_MS", "SPT_GENERIC_DLG_MAIN_TITLE", "SPT_GENERIC_DLG_INDEX", "SPT_GENERIC_EDITBOX_TXT", "SPT_GENERIC_EDITBOX", "SPT_GENERIC_SPINBUTTON", "SPT_GENERIC_CHECKBOX_TXT", "SPT_GENERIC_CHECKBOX", "SPT_GENERIC_COMBOBOX_TXT", "SPT_GENERIC_COMBOBOX", "SPT_GENERIC_RADIOBUTTON_GRP", "SPT_GENERIC_RADIOBUTTON_TXT", "SPT_GENERIC_RADIOBUTTON", "SPT_DLL_PRODUCT_VERSION", "SPT_DLL_FILE_VERSION", "SPT_END_OF_LIST"] ("Param")
                n146 = local read "Wavelength (nm)"() -> (w196:dbl)
                n147 = local read "MonoRef"() -> (w197:refnum<k7>)
                n148 = local read "Grating Number"() -> (w195:i16)
                n149 = invoke class="ISpectroObj" method="SetParam"(reference=w197, "Param"=w198, "pSetVal"=w196) -> (reference out=w200:refnum<k7>)  [unwired: 3 in, 5 out]
                n150 = invoke class="ISpectroObj" method="SetParam"(reference=w200, "Param"=w201, "pSetVal"=w195) -> (reference out=w199:refnum<k7>)  [unwired: 3 in, 5 out]
                n151 = invoke class="ISpectroObj" method="Move"(reference=w199) -> ()  [unwired: 2 in, 3 out]
              }
              frame #1 {
                n152 = local write "busy"(FALSE ("busy")) -> ()
              }
            }
          }
          frame 9 {
            w205 = 94 items=["EXP_ETACTUAL"=1, "EXP_SEQUENTS"=2, "EXP_ERROR"=3, "EXP_GETCAPS"=4, "EXP_GETPLSR"=5, "EXP_DETECTOR_BIT"=16, "EXP_RUNNING_APP"=23, "EXP_VIDEO_TYPE"=24, "EXP_CUSTOM_VIDEO_X"=25, "EXP_CUSTOM_VIDEO_Y"=26, "EXP_CUSTOM_VIDEO_FSTWIDTH"=27, "EXP_CUSTOM_VIDEO_LSTWIDTH"=28, "EXP_VIDEO_XDIM"=29, "EXP_VIDEO_YDIM"=30, "EXP_VIDEO_MAX_ZOOM"=31, "EXP_VIDEO_HORZ_PAN"=32, "EXP_VIDEO_VERT_PAN"=33, "EXP_WORD_MULTIPLIER"=34, "EXP_TARGET_ID"=35, "EXP_ADAPTER_ID"=36, "EXP_NUMADAPTORS"=37, "EXP_FORCE_PP_INIT"=38, "EXP_NOP_ADC"=39, "EXP_ACTUAL_TEMP"=40, "EXP_FORCE_AUTOSTOP"=41, "EXP_DEFAULT_VTCLK"=42, "EXP_MIN_VTCLK"=43, "EXP_MAX_VTCLK"=44, "EXP_DEFAULT_HTCLK"=45, "EXP_MIN_HTCLK"=46, "EXP_MAX_HTCLK"=47, "EXP_TIMING_STYLE"=48, "EXP_HEADSELECT"=49, "EXP_HORZPHASE"=50, "EXP_VERTPHASE"=51, "EXP_SPECIAL_SPEED"=52, "EXP_PRE_STRIPS"=53, "EXP_POST_STRIPS"=54, "EXP_PRE_LINES"=55, "EXP_POST_LINES"=56, "EXP_ACTIVE_LINES"=57, "EXP_ACTIVE_STRIPS"=58, "EXP_XFER_EXTRA"=59, "EXP_MIN_BLOCK"=60, "EXP_NUM_MIN_BLOCK"=61, "EXP_LOGIC_OUTPUT"=66, "EXP_VIDEO_BLANK"=67, "EXP_ZOOM_MODE_VIDEO"=68, "EXP_LEVEL_SYNC"=69, "EXP_DISABLE_LASER"=70, "EXP_ACQBACK_SHUTTER"=71, "EXP_ACQFLAT_SHUTTER"=72, "EXP_SMALL_CCD_MINEXP"=73, "EXP_LARGE_CCD_MINEXP"=74, "EXP_GATING_MODE"=75, "EXP_ILME_B1X"=76, "EXP_ILME_B2X"=77, "EXP_ILME_D1X"=78, "EXP_ILME_D2X"=79, "EXP_ILME_D4X"=80, "EXP_INIT_HW_ACCUM"=81, "EXP_5X_GAIN_ENABLE"=82, "EXP_RET_SRCCMP"=83, "EXP_EVENT_HANDLE"=84, "EXP_READOUT_MODE"=85, "EXP_SHUTTER_TYPE"=86, "EXP_USER_DEFINED_CHIP"=87, "EXP_USER_DEFINED_TIMING"=88, "EXP_CONTROLLER_VERSION"=89, "EXP_GET_CONTROLLER_VER"=90, "EXP_TTL_LINES"=91, "EXP_BIT_ADJUST"=92, "EXP_RESOLUTION"=93, "EXP_GAIN"=94, "EXP_ADC_RATE"=95, "EXP_ADC_TYPE"=96, "EXP_NUMBER_OF_CLEANS"=97, "EXP_NUM_OF_STRIPS_PER_CLN"=98, "EXP_INTERFACE_CARD"=99, "EXP_INTERRUPT"=100, "EXP_IO_ADDRESS1"=101, "EXP_IO_ADDRESS2"=102, "EXP_IO_ADDRESS3"=103, "EXP_HW_ROI"=104, "EXP_HW_BINNING"=105, "EXP_EDGE_TRIGGER"=106, "EXP_SHUTTER_CONTROL"=107, "EXP_RS170"=108, "EXP_RS170_COMPLEX"=109, "EXP_HW_RS170_LUT"=110, "EXP_RS170_INTENSITY_SCALING"=111, "EXP_RS170_OFFSET"=112, "EXP_RS170_PAN"=113, "EXP_RS170_ZOOM2X"=114, "EXP_RS170_ZOOM4X"=115, "EXP_RS170_BINNING"=116, "EXP_RS170_DECIMATION"=117, "EXP_HW_ACCUM"=118, "EXP_SHT_PREOPEN"=119, "EXP_STORE_STROBE"=120, "EXP_CONT_CLNS"=121, "EXP_TIMING_MODE"=122, "EXP_EXT_TRIGGER"=123, "EXP_EVENT_COUNTER"=124, "EXP_SW_TRIGGER"=125, "EXP_KINETICS_WINDOWSIZE"=126, "EXP_EXPOSURE"=127, "EXP_CONTROLLER_NAME"=128, "EXP_CCD_CHIP_NAME"=129, "EXP_BSWBINNING"=297, "EXP_EDGEENHANCE"=130, "EXP_BOXVIDEOGAIN"=131, "EXP_HSHADING_VALUE"=132, "EXP_VSHADING_VALUE"=133, "EXP_EDGEENHANCE_FLAG"=134, "EXP_SHADING_FLAG"=135, "EXP_GRAYSCALE"=136, "EXP_OFFSET"=137, "EXP_CCDGAIN"=138, "EXP_TEMPERATURE"=139, "EXP_MCPVOLTAGE"=140, "EXP_BOXEXPOSURE"=141, "EXP_ABC_FLAG"=142, "EXP_GAMMA_FLAG"=143, "EXP_AUTOBLACK_FLAG"=144, "EXP_AGC_FLAG"=145, "EXP_ODD_FIELD"=146, "EXP_FIELD_SELECT"=147, "EXP_RESET"=148, "EXP_EXTERN_ENABLE"=149, "EXP_CONTROLLERS_SUPPORTED"=150, "EXP_VTCLK"=151, "EXP_HTCLK"=152, "EXP_GATE_VS_CW"=153, "EXP_COM_PORT"=154, "EXP_US_UNITS"=156, "EXP_MS_UNITS"=157, "EXP_SEC_UNITS"=158, "EXP_MIN_UNITS"=159, "EXP_HRS_UNITS"=160, "EXP_FRAME_UNITS"=161, "EXP_SYNC_ASYNC"=162, "EXP_FOCUS_NFRAME"=163, "EXP_TIMEOUT"=164, "EXP_TIMEOUT_DEFAULT"=165, "EXP_HW_AUTOSTOP"=166, "EXP_RS170_INTEN_OFFSET"=167, "EXP_CONTROLLER_ALIVE"=168, "EXP_FOCUS_TYPE"=169, "EXP_FOCUS_ZOOM"=170, "EXP_FOCUS_PAN"=171, "EXP_MULTI_TAP_ROI"=172, "EXP_USE_INTERUPTS"=173, "EXP_DATA_ACQ_STATE"=174, "EXP_VERIFY_GOOD_VALUES"=175, "EXP_WHITE_CLAMP"=176, "EXP_BLACK_CLAMP"=177, "EXP_DELAY_TIME"=178, "EXP_READOUT_TIME"=179, "EXP_SW_DIAG"=180, "EXP_DIAG1"=181, "EXP_DIAG2"=182, "EXP_DIAG3"=183, "EXP_DIAG4"=184, "EXP_DIAG5"=185, "EXP_AorB_GROUP"=186, "EXP_ABSORBANCE_FLAG"=187, "EXP_ABSORBANCE_METHOD"=188, "EXP_ABSORBANCE_STRIPNUM"=189, "EXP_DMASIZE_VIA_DRIVER"=190, "EXP_DRIVERVERSION"=191, "EXP_NUM_DEVICES"=192, "EXP_ECPDMA_CHANNEL"=193, "EXP_CUSTOM_SHUTTER"=194, "EXP_ADC_OFFSET"=195, "EXP_CURRENT_READOUT_MODE"=196, "EXP_BANK_ADD"=197, "EXP_LUT_BANK"=198, "EXP_SETUP_STATUS"=201, "EXP_XY_GROUPING"=239, "EXP_MESSAGES_FLAG"=240, "EXP_TTL_LINE_TO_WAIT"=253, "EXP_DATA_COLLECTION_MODE"=258, "EXP_DATA_COLLECTION_TYPE"=262, "EXP_SKIPFRAMES"=274, "EXP_CLR_INT_CNTR"=276, "EXP_ENABLE_INT_CNTR"=277, "EXP_INT_CNTR"=278, "EXP_INTERNAL_SYNC_SRC"=279, "EXP_SW_EXTSYNC"=280, "EXP_PTG_PRESENT"=281, "EXP_ELEC_SHT"=282, "EXP_BOARDS_WITH_NVRAM"=283, "EXP_ANLGMASTER_ST143"=284, "EXP_ANLGSLAVE_ST143"=285, "EXP_DISPLAY_ST143"=286, "EXP_INTRFACE_ST143"=287, "EXP_SCANCONTROL_ST143"=288, "EXP_NUMBERFRAMES_IRQ"=204, "EXP_COOL_TYPE"=214, "EXP_HD_TYPE"=215, "EXP_INTENSIFER_GAIN"=216, "EXP_SHT_GATE_MODE"=217, "EXP_HD_CHECK"=218, "EXP_AMP_MODE"=219, "EXP_AMP_DIALOG"=247, "EXP_ANALOG_GAIN"=220, "EXP_HW_FIXES"=221, "EXP_PCI_CARDS"=222, "EXP_NOT_REVERSE"=223, "EXP_LOAD_NVRAM_DEFAULTS"=234, "EXP_CNTR_BRD"=235, "EXP_XDIMHW"=237, "EXP_YDIMHW"=238, "EXP_SPECIAL_FAST_RDOUT"=254, "EXP_SPCL_FAST_Y_DIM"=255, "EXP_SPCL_FAST_X_DIM"=256, "EXP_SPCL_FAST_Y_INDEX"=257, "EXP_SHUTTER_COMP_TIME_MS"=266, "EXP_NVRAM_AVAIL"=267, "EXP_NUMBER_AGAIN_AVAIL"=269, "EXP_SENSOR_TYPE"=270, "EXP_EVENT_TYPE"=292, "EXP_ANTI_BLOOMING"=293, "EXP_FAST_PULSE_ENABLE"=233, "EXP_USE_HEADCALIB"=296, "EXP_TEMP_STATUS"=301, "EXP_MULTIPLE_READMODES_LIVE"=302, "EXP_FIRST_ACQUIRE_FLAG"=303, "EXP_ANTI_BLOOMING_CONTROL"=304, "EXP_PRE_HORZ_DELAY"=305, "EXP_NVRAM_TRIES"=306, "EXP_XASCEND"=307, "EXP_YASCEND"=308, "EXP_ALT_TIMING"=309, "EXP_SHUTTER_PRE_COMP"=310, "EXP_PVCAM_POSSIBLE"=311, "EXP_ADC_IN_NVRAM"=312, "EXP_PASSTHRU_MODE"=313, "EXP_FIRMWAREVERSION"=314, "EXP_IMMEDIATE_SHUTTER"=315, "EXP_STAGE2_TEMP"=316, "EXP_AVGAIN_ENABLED"=317, "EXP_AVGAIN_SETPOINT"=318, "EXP_AVGAIN"=319, "EXP_AVGAIN_CALIB_TEMP"=320, "EXP_AVGAIN_CALIB_COEFF1"=321, "EXP_AVGAIN_CALIB_COEFF2"=322, "EXP_AVGAIN_CALIB_COEFF3"=323, "EXP_AVGAIN_CALIB_COEFF4"=324, "EXP_AVGAIN_CALIB_COEFF5"=325, "EXP_FORCE_READOUT_MODE"=326, "EXP_RESET_DATACOLLECTION"=327, "EXP_ACTIVE_SUBFRAME"=328, "EXP_PV_READOUT_PORT"=514, "EXP_COOLING_FAN_CTRL"=339, "EXP_SHTR_RES"=343, "EXP_PBC"=351, "EXP_PREEXP_CLEANS"=354, "EXP_TTL_CTRL"=355, "EXP_PAR_SHIFT_INDEX"=547, "EXP_LOGIC_OUTPUT_INVERT"=548, "EXP_CLASSNAME"=775, "EXP_FLATFLDNAME"=776, "EXP_DARKNAME"=777, "EXP_SETUPNAME"=778, "EXP_ACCESSNAME"=779, "EXP_DATFILENAME"=780, "EXP_ABSORBFILENAME"=781, "EXP_BLEMISHFILENAME"=782, "EXP_COSMICFILENAME"=783, "EXP_FILEINCBASENAME"=784, "EXP_YTNAME"=785, "EXP_DEVNAME"=786, "EXP_USEROI"=787, "EXP_DOBLEMISH"=788, "EXP_DOABSORB"=789, "EXP_DOCOSMIC"=790, "EXP_COSMICSENS"=791, "EXP_ABSORBSTRIP"=792, "EXP_DATATYPE"=793, "EXP_OVERWRITECONFIRM"=794, "EXP_FILEINCENABLE"=795, "EXP_FILEINCCOUNT"=796, "EXP_RUNNING"=797, "EXP_SAVEROPT"=798, "EXP_TIME_UNITS"=799, "EXP_FILEACCESS"=800, "EXP_AUTOSAVE"=801, "EXP_NEWWINDOW"=802, "EXP_XDIM"=803, "EXP_YDIM"=804, "EXP_XDIMDET"=805, "EXP_YDIMDET"=806, "EXP_ROIMODE"=807, "EXP_NUMREPEATSEXP"=808, "EXP_NUMACCUMSEXP"=809, "EXP_THREADSTATE"=810, "EXP_USEMINTHRESHOLDING"=811, "EXP_MINTHRESHOLDVALUE"=812, "EXP_USEMAXTHRESHOLDING"=813, "EXP_MAXTHRESHOLDVALUE"=814, "EXP_RUNNING_EXPERIMENT"=815, "EXP_THRESHOLD_DEMAND_UPDATE"=816, "EXP_ROICOUNT"=817, "EXP_ACCUMS"=818, "EXP_CACCUMS"=819, "EXP_CSEQUENTS"=820, "EXP_PHOTON_ESTIMATION_ENABLE"=821, "EXP_PHOTON_MAXTIME"=822, "EXP_PHOTON_MAXTIMEUNIT"=823, "EXP_CUSTOMFILTER_ENABLE"=824, "EXP_CUSTOMFILTER_SIZE"=825, "EXP_LOOKUPTABLE_ENABLE"=826, "EXP_BSHOWWINDOW"=827, "EXP_BBACKSUBTRACT"=828, "EXP_BDOFLATFIELD"=829, "EXP_ASCIIOUTPUTFILE"=830, "EXP_ASCIIOUTPUT_DELIMITER"=831, "EXP_ASCIIOUTPUT_TERMINATOR"=832, "EXP_FFTYPE"=833, "EXP_BGTYPE"=834, "EXP_COSGRASS"=835, "EXP_RUNASCONFIRM"=836, "EXP_RUNASRUNACCESS"=837, "EXP_DATAFILETYPE"=838, "EXP_ROTATE"=839, "EXP_FLIP"=840, "EXP_REVERSE"=841, "EXP_SWBINNING"=842, "EXP_AUTOSTORE"=843, "EXP_XBINNED"=844, "EXP_YBINNED"=845, "EXP_NUMPATTERNS"=846, "EXP_EXPERIMENTTIME"=847, "EXP_ASYNCSEQUENTIALS"=848, "EXP_SEQUENTIALS"=849, "EXP_CSEQUENTIALS"=850, "EXP_AUTOD"=851, "EXP_EXPOSURETIME"=852, "EXP_EXPOSURETIME_UNITS"=853, "EXP_ACQMODE"=854, "EXP_DMASIZE_PVCAM"=855, "EXP_INITIALIZE"=856, "EXP_CELL_X_SIZE"=857, "EXP_CELL_Y_SIZE"=858, "EXP_X_GAP_SIZE"=859, "EXP_Y_GAP_SIZE"=860] ("Param")
            # "change OMA V gain"
            n153 = local read "experiment reference"() -> (w203:refnum<k7>)
            n154 = local read "OMA V gain"() -> (w204:u32)
            n155 = invoke class="IExpSetup2" method="SetParam"(reference=w203, "Param"=w205, "pSetVal"=w204) -> ()  [unwired: 2 in, 5 out]
          }
          frame 10 {
            # "Start single spectrum"
            n156 = flat-sequence {
              tunnel: [w212] -> w208
              tunnel: [w211] -> w207
              tunnel: [w210] -> w206
              tunnel: w208 -> [w236]
              tunnel: w207 -> [w230]
              tunnel: w206 -> [w229]
              frame #0 {
                n157 = Tick Count (ms)() -> (millisecond timer value=w209:u32)
                n158 = local write "time start (ms)"(w209) -> ()
              }
              frame #1 {
                w217 = 127 items=["EXP_ETACTUAL"=1, "EXP_SEQUENTS"=2, "EXP_ERROR"=3, "EXP_GETCAPS"=4, "EXP_GETPLSR"=5, "EXP_DETECTOR_BIT"=16, "EXP_RUNNING_APP"=23, "EXP_VIDEO_TYPE"=24, "EXP_CUSTOM_VIDEO_X"=25, "EXP_CUSTOM_VIDEO_Y"=26, "EXP_CUSTOM_VIDEO_FSTWIDTH"=27, "EXP_CUSTOM_VIDEO_LSTWIDTH"=28, "EXP_VIDEO_XDIM"=29, "EXP_VIDEO_YDIM"=30, "EXP_VIDEO_MAX_ZOOM"=31, "EXP_VIDEO_HORZ_PAN"=32, "EXP_VIDEO_VERT_PAN"=33, "EXP_WORD_MULTIPLIER"=34, "EXP_TARGET_ID"=35, "EXP_ADAPTER_ID"=36, "EXP_NUMADAPTORS"=37, "EXP_FORCE_PP_INIT"=38, "EXP_NOP_ADC"=39, "EXP_ACTUAL_TEMP"=40, "EXP_FORCE_AUTOSTOP"=41, "EXP_DEFAULT_VTCLK"=42, "EXP_MIN_VTCLK"=43, "EXP_MAX_VTCLK"=44, "EXP_DEFAULT_HTCLK"=45, "EXP_MIN_HTCLK"=46, "EXP_MAX_HTCLK"=47, "EXP_TIMING_STYLE"=48, "EXP_HEADSELECT"=49, "EXP_HORZPHASE"=50, "EXP_VERTPHASE"=51, "EXP_SPECIAL_SPEED"=52, "EXP_PRE_STRIPS"=53, "EXP_POST_STRIPS"=54, "EXP_PRE_LINES"=55, "EXP_POST_LINES"=56, "EXP_ACTIVE_LINES"=57, "EXP_ACTIVE_STRIPS"=58, "EXP_XFER_EXTRA"=59, "EXP_MIN_BLOCK"=60, "EXP_NUM_MIN_BLOCK"=61, "EXP_LOGIC_OUTPUT"=66, "EXP_VIDEO_BLANK"=67, "EXP_ZOOM_MODE_VIDEO"=68, "EXP_LEVEL_SYNC"=69, "EXP_DISABLE_LASER"=70, "EXP_ACQBACK_SHUTTER"=71, "EXP_ACQFLAT_SHUTTER"=72, "EXP_SMALL_CCD_MINEXP"=73, "EXP_LARGE_CCD_MINEXP"=74, "EXP_GATING_MODE"=75, "EXP_ILME_B1X"=76, "EXP_ILME_B2X"=77, "EXP_ILME_D1X"=78, "EXP_ILME_D2X"=79, "EXP_ILME_D4X"=80, "EXP_INIT_HW_ACCUM"=81, "EXP_5X_GAIN_ENABLE"=82, "EXP_RET_SRCCMP"=83, "EXP_EVENT_HANDLE"=84, "EXP_READOUT_MODE"=85, "EXP_SHUTTER_TYPE"=86, "EXP_USER_DEFINED_CHIP"=87, "EXP_USER_DEFINED_TIMING"=88, "EXP_CONTROLLER_VERSION"=89, "EXP_GET_CONTROLLER_VER"=90, "EXP_TTL_LINES"=91, "EXP_BIT_ADJUST"=92, "EXP_RESOLUTION"=93, "EXP_GAIN"=94, "EXP_ADC_RATE"=95, "EXP_ADC_TYPE"=96, "EXP_NUMBER_OF_CLEANS"=97, "EXP_NUM_OF_STRIPS_PER_CLN"=98, "EXP_INTERFACE_CARD"=99, "EXP_INTERRUPT"=100, "EXP_IO_ADDRESS1"=101, "EXP_IO_ADDRESS2"=102, "EXP_IO_ADDRESS3"=103, "EXP_HW_ROI"=104, "EXP_HW_BINNING"=105, "EXP_EDGE_TRIGGER"=106, "EXP_SHUTTER_CONTROL"=107, "EXP_RS170"=108, "EXP_RS170_COMPLEX"=109, "EXP_HW_RS170_LUT"=110, "EXP_RS170_INTENSITY_SCALING"=111, "EXP_RS170_OFFSET"=112, "EXP_RS170_PAN"=113, "EXP_RS170_ZOOM2X"=114, "EXP_RS170_ZOOM4X"=115, "EXP_RS170_BINNING"=116, "EXP_RS170_DECIMATION"=117, "EXP_HW_ACCUM"=118, "EXP_SHT_PREOPEN"=119, "EXP_STORE_STROBE"=120, "EXP_CONT_CLNS"=121, "EXP_TIMING_MODE"=122, "EXP_EXT_TRIGGER"=123, "EXP_EVENT_COUNTER"=124, "EXP_SW_TRIGGER"=125, "EXP_KINETICS_WINDOWSIZE"=126, "EXP_EXPOSURE"=127, "EXP_CONTROLLER_NAME"=128, "EXP_CCD_CHIP_NAME"=129, "EXP_BSWBINNING"=297, "EXP_EDGEENHANCE"=130, "EXP_BOXVIDEOGAIN"=131, "EXP_HSHADING_VALUE"=132, "EXP_VSHADING_VALUE"=133, "EXP_EDGEENHANCE_FLAG"=134, "EXP_SHADING_FLAG"=135, "EXP_GRAYSCALE"=136, "EXP_OFFSET"=137, "EXP_CCDGAIN"=138, "EXP_TEMPERATURE"=139, "EXP_MCPVOLTAGE"=140, "EXP_BOXEXPOSURE"=141, "EXP_ABC_FLAG"=142, "EXP_GAMMA_FLAG"=143, "EXP_AUTOBLACK_FLAG"=144, "EXP_AGC_FLAG"=145, "EXP_ODD_FIELD"=146, "EXP_FIELD_SELECT"=147, "EXP_RESET"=148, "EXP_EXTERN_ENABLE"=149, "EXP_CONTROLLERS_SUPPORTED"=150, "EXP_VTCLK"=151, "EXP_HTCLK"=152, "EXP_GATE_VS_CW"=153, "EXP_COM_PORT"=154, "EXP_US_UNITS"=156, "EXP_MS_UNITS"=157, "EXP_SEC_UNITS"=158, "EXP_MIN_UNITS"=159, "EXP_HRS_UNITS"=160, "EXP_FRAME_UNITS"=161, "EXP_SYNC_ASYNC"=162, "EXP_FOCUS_NFRAME"=163, "EXP_TIMEOUT"=164, "EXP_TIMEOUT_DEFAULT"=165, "EXP_HW_AUTOSTOP"=166, "EXP_RS170_INTEN_OFFSET"=167, "EXP_CONTROLLER_ALIVE"=168, "EXP_FOCUS_TYPE"=169, "EXP_FOCUS_ZOOM"=170, "EXP_FOCUS_PAN"=171, "EXP_MULTI_TAP_ROI"=172, "EXP_USE_INTERUPTS"=173, "EXP_DATA_ACQ_STATE"=174, "EXP_VERIFY_GOOD_VALUES"=175, "EXP_WHITE_CLAMP"=176, "EXP_BLACK_CLAMP"=177, "EXP_DELAY_TIME"=178, "EXP_READOUT_TIME"=179, "EXP_SW_DIAG"=180, "EXP_DIAG1"=181, "EXP_DIAG2"=182, "EXP_DIAG3"=183, "EXP_DIAG4"=184, "EXP_DIAG5"=185, "EXP_AorB_GROUP"=186, "EXP_ABSORBANCE_FLAG"=187, "EXP_ABSORBANCE_METHOD"=188, "EXP_ABSORBANCE_STRIPNUM"=189, "EXP_DMASIZE_VIA_DRIVER"=190, "EXP_DRIVERVERSION"=191, "EXP_NUM_DEVICES"=192, "EXP_ECPDMA_CHANNEL"=193, "EXP_CUSTOM_SHUTTER"=194, "EXP_ADC_OFFSET"=195, "EXP_CURRENT_READOUT_MODE"=196, "EXP_BANK_ADD"=197, "EXP_LUT_BANK"=198, "EXP_SETUP_STATUS"=201, "EXP_XY_GROUPING"=239, "EXP_MESSAGES_FLAG"=240, "EXP_TTL_LINE_TO_WAIT"=253, "EXP_DATA_COLLECTION_MODE"=258, "EXP_DATA_COLLECTION_TYPE"=262, "EXP_SKIPFRAMES"=274, "EXP_CLR_INT_CNTR"=276, "EXP_ENABLE_INT_CNTR"=277, "EXP_INT_CNTR"=278, "EXP_INTERNAL_SYNC_SRC"=279, "EXP_SW_EXTSYNC"=280, "EXP_PTG_PRESENT"=281, "EXP_ELEC_SHT"=282, "EXP_BOARDS_WITH_NVRAM"=283, "EXP_ANLGMASTER_ST143"=284, "EXP_ANLGSLAVE_ST143"=285, "EXP_DISPLAY_ST143"=286, "EXP_INTRFACE_ST143"=287, "EXP_SCANCONTROL_ST143"=288, "EXP_NUMBERFRAMES_IRQ"=204, "EXP_COOL_TYPE"=214, "EXP_HD_TYPE"=215, "EXP_INTENSIFER_GAIN"=216, "EXP_SHT_GATE_MODE"=217, "EXP_HD_CHECK"=218, "EXP_AMP_MODE"=219, "EXP_AMP_DIALOG"=247, "EXP_ANALOG_GAIN"=220, "EXP_HW_FIXES"=221, "EXP_PCI_CARDS"=222, "EXP_NOT_REVERSE"=223, "EXP_LOAD_NVRAM_DEFAULTS"=234, "EXP_CNTR_BRD"=235, "EXP_XDIMHW"=237, "EXP_YDIMHW"=238, "EXP_SPECIAL_FAST_RDOUT"=254, "EXP_SPCL_FAST_Y_DIM"=255, "EXP_SPCL_FAST_X_DIM"=256, "EXP_SPCL_FAST_Y_INDEX"=257, "EXP_SHUTTER_COMP_TIME_MS"=266, "EXP_NVRAM_AVAIL"=267, "EXP_NUMBER_AGAIN_AVAIL"=269, "EXP_SENSOR_TYPE"=270, "EXP_EVENT_TYPE"=292, "EXP_ANTI_BLOOMING"=293, "EXP_FAST_PULSE_ENABLE"=233, "EXP_USE_HEADCALIB"=296, "EXP_TEMP_STATUS"=301, "EXP_MULTIPLE_READMODES_LIVE"=302, "EXP_FIRST_ACQUIRE_FLAG"=303, "EXP_ANTI_BLOOMING_CONTROL"=304, "EXP_PRE_HORZ_DELAY"=305, "EXP_NVRAM_TRIES"=306, "EXP_XASCEND"=307, "EXP_YASCEND"=308, "EXP_ALT_TIMING"=309, "EXP_SHUTTER_PRE_COMP"=310, "EXP_PVCAM_POSSIBLE"=311, "EXP_ADC_IN_NVRAM"=312, "EXP_PASSTHRU_MODE"=313, "EXP_FIRMWAREVERSION"=314, "EXP_IMMEDIATE_SHUTTER"=315, "EXP_STAGE2_TEMP"=316, "EXP_AVGAIN_ENABLED"=317, "EXP_AVGAIN_SETPOINT"=318, "EXP_AVGAIN"=319, "EXP_AVGAIN_CALIB_TEMP"=320, "EXP_AVGAIN_CALIB_COEFF1"=321, "EXP_AVGAIN_CALIB_COEFF2"=322, "EXP_AVGAIN_CALIB_COEFF3"=323, "EXP_AVGAIN_CALIB_COEFF4"=324, "EXP_AVGAIN_CALIB_COEFF5"=325, "EXP_FORCE_READOUT_MODE"=326, "EXP_RESET_DATACOLLECTION"=327, "EXP_ACTIVE_SUBFRAME"=328, "EXP_PV_READOUT_PORT"=514, "EXP_CLASSNAME"=775, "EXP_FLATFLDNAME"=776, "EXP_DARKNAME"=777, "EXP_SETUPNAME"=778, "EXP_ACCESSNAME"=779, "EXP_DATFILENAME"=780, "EXP_ABSORBFILENAME"=781, "EXP_BLEMISHFILENAME"=782, "EXP_COSMICFILENAME"=783, "EXP_FILEINCBASENAME"=784, "EXP_YTNAME"=785, "EXP_DEVNAME"=786, "EXP_USEROI"=787, "EXP_DOBLEMISH"=788, "EXP_DOABSORB"=789, "EXP_DOCOSMIC"=790, "EXP_COSMICSENS"=791, "EXP_ABSORBSTRIP"=792, "EXP_DATATYPE"=793, "EXP_OVERWRITECONFIRM"=794, "EXP_FILEINCENABLE"=795, "EXP_FILEINCCOUNT"=796, "EXP_RUNNING"=797, "EXP_SAVEROPT"=798, "EXP_TIME_UNITS"=799, "EXP_FILEACCESS"=800, "EXP_AUTOSAVE"=801, "EXP_NEWWINDOW"=802, "EXP_XDIM"=803, "EXP_YDIM"=804, "EXP_XDIMDET"=805, "EXP_YDIMDET"=806, "EXP_ROIMODE"=807, "EXP_NUMREPEATSEXP"=808, "EXP_NUMACCUMSEXP"=809, "EXP_THREADSTATE"=810, "EXP_USEMINTHRESHOLDING"=811, "EXP_MINTHRESHOLDVALUE"=812, "EXP_USEMAXTHRESHOLDING"=813, "EXP_MAXTHRESHOLDVALUE"=814, "EXP_RUNNING_EXPERIMENT"=815, "EXP_THRESHOLD_DEMAND_UPDATE"=816, "EXP_ROICOUNT"=817, "EXP_ACCUMS"=818, "EXP_CACCUMS"=819, "EXP_CSEQUENTS"=820, "EXP_PHOTON_ESTIMATION_ENABLE"=821, "EXP_PHOTON_MAXTIME"=822, "EXP_PHOTON_MAXTIMEUNIT"=823, "EXP_CUSTOMFILTER_ENABLE"=824, "EXP_CUSTOMFILTER_SIZE"=825, "EXP_LOOKUPTABLE_ENABLE"=826, "EXP_BSHOWWINDOW"=827, "EXP_BBACKSUBTRACT"=828, "EXP_BDOFLATFIELD"=829, "EXP_ASCIIOUTPUTFILE"=830, "EXP_ASCIIOUTPUT_DELIMITER"=831, "EXP_ASCIIOUTPUT_TERMINATOR"=832, "EXP_FFTYPE"=833, "EXP_BGTYPE"=834, "EXP_COSGRASS"=835, "EXP_RUNASCONFIRM"=836, "EXP_RUNASRUNACCESS"=837, "EXP_DATAFILETYPE"=838, "EXP_ROTATE"=839, "EXP_FLIP"=840, "EXP_REVERSE"=841, "EXP_SWBINNING"=842, "EXP_AUTOSTORE"=843, "EXP_XBINNED"=844, "EXP_YBINNED"=845, "EXP_NUMPATTERNS"=846, "EXP_EXPERIMENTTIME"=847, "EXP_ASYNCSEQUENTIALS"=848, "EXP_SEQUENTIALS"=849, "EXP_CSEQUENTIALS"=850, "EXP_AUTOD"=851, "EXP_EXPOSURETIME"=852, "EXP_EXPOSURETIME_UNITS"=853, "EXP_ACQMODE"=854, "EXP_DMASIZE_PVCAM"=855, "EXP_INITIALIZE"=856, "EXP_CELL_X_SIZE"=857, "EXP_CELL_Y_SIZE"=858, "EXP_X_GAP_SIZE"=859, "EXP_Y_GAP_SIZE"=860] ("Param")
                n159 = local read "OMA V exposure time"() -> (w218:dbl)
                n160 = local read "experiment reference"() -> (w216:refnum<k7>)
                n161 = invoke class="IExpSetup2" method="SetParam"(reference=w216, "Param"=w217, "pSetVal"=w218) -> (reference out=w215:refnum<k7>)  [unwired: 2 in, 4 out]
                n162 = local read "file reference"() -> (w214:refnum<k7>)
                n163 = invoke class="IExpSetup2" method="Start"(reference=w215, "pFile"=w214) -> (reference out=w213:refnum<k7>, "pFile"=w212:refnum<k7>)  [unwired: 2 in, 2 out]
                n164 = while {
                  tunnel: w213 -> [w221]
                  tunnel: [w220] -> w211
                  tunnel: [w219] -> w210
                  stop <- w227 stop-if-true
                  w224 = 797 items=["EXP_ETACTUAL"=1, "EXP_SEQUENTS"=2, "EXP_ERROR"=3, "EXP_GETCAPS"=4, "EXP_GETPLSR"=5, "EXP_DETECTOR_BIT"=16, "EXP_RUNNING_APP"=23, "EXP_VIDEO_TYPE"=24, "EXP_CUSTOM_VIDEO_X"=25, "EXP_CUSTOM_VIDEO_Y"=26, "EXP_CUSTOM_VIDEO_FSTWIDTH"=27, "EXP_CUSTOM_VIDEO_LSTWIDTH"=28, "EXP_VIDEO_XDIM"=29, "EXP_VIDEO_YDIM"=30, "EXP_VIDEO_MAX_ZOOM"=31, "EXP_VIDEO_HORZ_PAN"=32, "EXP_VIDEO_VERT_PAN"=33, "EXP_WORD_MULTIPLIER"=34, "EXP_TARGET_ID"=35, "EXP_ADAPTER_ID"=36, "EXP_NUMADAPTORS"=37, "EXP_FORCE_PP_INIT"=38, "EXP_NOP_ADC"=39, "EXP_ACTUAL_TEMP"=40, "EXP_FORCE_AUTOSTOP"=41, "EXP_DEFAULT_VTCLK"=42, "EXP_MIN_VTCLK"=43, "EXP_MAX_VTCLK"=44, "EXP_DEFAULT_HTCLK"=45, "EXP_MIN_HTCLK"=46, "EXP_MAX_HTCLK"=47, "EXP_TIMING_STYLE"=48, "EXP_HEADSELECT"=49, "EXP_HORZPHASE"=50, "EXP_VERTPHASE"=51, "EXP_SPECIAL_SPEED"=52, "EXP_PRE_STRIPS"=53, "EXP_POST_STRIPS"=54, "EXP_PRE_LINES"=55, "EXP_POST_LINES"=56, "EXP_ACTIVE_LINES"=57, "EXP_ACTIVE_STRIPS"=58, "EXP_XFER_EXTRA"=59, "EXP_MIN_BLOCK"=60, "EXP_NUM_MIN_BLOCK"=61, "EXP_LOGIC_OUTPUT"=66, "EXP_VIDEO_BLANK"=67, "EXP_ZOOM_MODE_VIDEO"=68, "EXP_LEVEL_SYNC"=69, "EXP_DISABLE_LASER"=70, "EXP_ACQBACK_SHUTTER"=71, "EXP_ACQFLAT_SHUTTER"=72, "EXP_SMALL_CCD_MINEXP"=73, "EXP_LARGE_CCD_MINEXP"=74, "EXP_GATING_MODE"=75, "EXP_ILME_B1X"=76, "EXP_ILME_B2X"=77, "EXP_ILME_D1X"=78, "EXP_ILME_D2X"=79, "EXP_ILME_D4X"=80, "EXP_INIT_HW_ACCUM"=81, "EXP_5X_GAIN_ENABLE"=82, "EXP_RET_SRCCMP"=83, "EXP_EVENT_HANDLE"=84, "EXP_READOUT_MODE"=85, "EXP_SHUTTER_TYPE"=86, "EXP_USER_DEFINED_CHIP"=87, "EXP_USER_DEFINED_TIMING"=88, "EXP_CONTROLLER_VERSION"=89, "EXP_GET_CONTROLLER_VER"=90, "EXP_TTL_LINES"=91, "EXP_BIT_ADJUST"=92, "EXP_RESOLUTION"=93, "EXP_GAIN"=94, "EXP_ADC_RATE"=95, "EXP_ADC_TYPE"=96, "EXP_NUMBER_OF_CLEANS"=97, "EXP_NUM_OF_STRIPS_PER_CLN"=98, "EXP_INTERFACE_CARD"=99, "EXP_INTERRUPT"=100, "EXP_IO_ADDRESS1"=101, "EXP_IO_ADDRESS2"=102, "EXP_IO_ADDRESS3"=103, "EXP_HW_ROI"=104, "EXP_HW_BINNING"=105, "EXP_EDGE_TRIGGER"=106, "EXP_SHUTTER_CONTROL"=107, "EXP_RS170"=108, "EXP_RS170_COMPLEX"=109, "EXP_HW_RS170_LUT"=110, "EXP_RS170_INTENSITY_SCALING"=111, "EXP_RS170_OFFSET"=112, "EXP_RS170_PAN"=113, "EXP_RS170_ZOOM2X"=114, "EXP_RS170_ZOOM4X"=115, "EXP_RS170_BINNING"=116, "EXP_RS170_DECIMATION"=117, "EXP_HW_ACCUM"=118, "EXP_SHT_PREOPEN"=119, "EXP_STORE_STROBE"=120, "EXP_CONT_CLNS"=121, "EXP_TIMING_MODE"=122, "EXP_EXT_TRIGGER"=123, "EXP_EVENT_COUNTER"=124, "EXP_SW_TRIGGER"=125, "EXP_KINETICS_WINDOWSIZE"=126, "EXP_EXPOSURE"=127, "EXP_CONTROLLER_NAME"=128, "EXP_CCD_CHIP_NAME"=129, "EXP_BSWBINNING"=297, "EXP_EDGEENHANCE"=130, "EXP_BOXVIDEOGAIN"=131, "EXP_HSHADING_VALUE"=132, "EXP_VSHADING_VALUE"=133, "EXP_EDGEENHANCE_FLAG"=134, "EXP_SHADING_FLAG"=135, "EXP_GRAYSCALE"=136, "EXP_OFFSET"=137, "EXP_CCDGAIN"=138, "EXP_TEMPERATURE"=139, "EXP_MCPVOLTAGE"=140, "EXP_BOXEXPOSURE"=141, "EXP_ABC_FLAG"=142, "EXP_GAMMA_FLAG"=143, "EXP_AUTOBLACK_FLAG"=144, "EXP_AGC_FLAG"=145, "EXP_ODD_FIELD"=146, "EXP_FIELD_SELECT"=147, "EXP_RESET"=148, "EXP_EXTERN_ENABLE"=149, "EXP_CONTROLLERS_SUPPORTED"=150, "EXP_VTCLK"=151, "EXP_HTCLK"=152, "EXP_GATE_VS_CW"=153, "EXP_COM_PORT"=154, "EXP_US_UNITS"=156, "EXP_MS_UNITS"=157, "EXP_SEC_UNITS"=158, "EXP_MIN_UNITS"=159, "EXP_HRS_UNITS"=160, "EXP_FRAME_UNITS"=161, "EXP_SYNC_ASYNC"=162, "EXP_FOCUS_NFRAME"=163, "EXP_TIMEOUT"=164, "EXP_TIMEOUT_DEFAULT"=165, "EXP_HW_AUTOSTOP"=166, "EXP_RS170_INTEN_OFFSET"=167, "EXP_CONTROLLER_ALIVE"=168, "EXP_FOCUS_TYPE"=169, "EXP_FOCUS_ZOOM"=170, "EXP_FOCUS_PAN"=171, "EXP_MULTI_TAP_ROI"=172, "EXP_USE_INTERUPTS"=173, "EXP_DATA_ACQ_STATE"=174, "EXP_VERIFY_GOOD_VALUES"=175, "EXP_WHITE_CLAMP"=176, "EXP_BLACK_CLAMP"=177, "EXP_DELAY_TIME"=178, "EXP_READOUT_TIME"=179, "EXP_SW_DIAG"=180, "EXP_DIAG1"=181, "EXP_DIAG2"=182, "EXP_DIAG3"=183, "EXP_DIAG4"=184, "EXP_DIAG5"=185, "EXP_AorB_GROUP"=186, "EXP_ABSORBANCE_FLAG"=187, "EXP_ABSORBANCE_METHOD"=188, "EXP_ABSORBANCE_STRIPNUM"=189, "EXP_DMASIZE_VIA_DRIVER"=190, "EXP_DRIVERVERSION"=191, "EXP_NUM_DEVICES"=192, "EXP_ECPDMA_CHANNEL"=193, "EXP_CUSTOM_SHUTTER"=194, "EXP_ADC_OFFSET"=195, "EXP_CURRENT_READOUT_MODE"=196, "EXP_BANK_ADD"=197, "EXP_LUT_BANK"=198, "EXP_SETUP_STATUS"=201, "EXP_XY_GROUPING"=239, "EXP_MESSAGES_FLAG"=240, "EXP_TTL_LINE_TO_WAIT"=253, "EXP_DATA_COLLECTION_MODE"=258, "EXP_DATA_COLLECTION_TYPE"=262, "EXP_SKIPFRAMES"=274, "EXP_CLR_INT_CNTR"=276, "EXP_ENABLE_INT_CNTR"=277, "EXP_INT_CNTR"=278, "EXP_INTERNAL_SYNC_SRC"=279, "EXP_SW_EXTSYNC"=280, "EXP_PTG_PRESENT"=281, "EXP_ELEC_SHT"=282, "EXP_BOARDS_WITH_NVRAM"=283, "EXP_ANLGMASTER_ST143"=284, "EXP_ANLGSLAVE_ST143"=285, "EXP_DISPLAY_ST143"=286, "EXP_INTRFACE_ST143"=287, "EXP_SCANCONTROL_ST143"=288, "EXP_NUMBERFRAMES_IRQ"=204, "EXP_COOL_TYPE"=214, "EXP_HD_TYPE"=215, "EXP_INTENSIFER_GAIN"=216, "EXP_SHT_GATE_MODE"=217, "EXP_HD_CHECK"=218, "EXP_AMP_MODE"=219, "EXP_AMP_DIALOG"=247, "EXP_ANALOG_GAIN"=220, "EXP_HW_FIXES"=221, "EXP_PCI_CARDS"=222, "EXP_NOT_REVERSE"=223, "EXP_LOAD_NVRAM_DEFAULTS"=234, "EXP_CNTR_BRD"=235, "EXP_XDIMHW"=237, "EXP_YDIMHW"=238, "EXP_SPECIAL_FAST_RDOUT"=254, "EXP_SPCL_FAST_Y_DIM"=255, "EXP_SPCL_FAST_X_DIM"=256, "EXP_SPCL_FAST_Y_INDEX"=257, "EXP_SHUTTER_COMP_TIME_MS"=266, "EXP_NVRAM_AVAIL"=267, "EXP_NUMBER_AGAIN_AVAIL"=269, "EXP_SENSOR_TYPE"=270, "EXP_EVENT_TYPE"=292, "EXP_ANTI_BLOOMING"=293, "EXP_FAST_PULSE_ENABLE"=233, "EXP_USE_HEADCALIB"=296, "EXP_TEMP_STATUS"=301, "EXP_MULTIPLE_READMODES_LIVE"=302, "EXP_FIRST_ACQUIRE_FLAG"=303, "EXP_ANTI_BLOOMING_CONTROL"=304, "EXP_PRE_HORZ_DELAY"=305, "EXP_NVRAM_TRIES"=306, "EXP_XASCEND"=307, "EXP_YASCEND"=308, "EXP_ALT_TIMING"=309, "EXP_SHUTTER_PRE_COMP"=310, "EXP_PVCAM_POSSIBLE"=311, "EXP_ADC_IN_NVRAM"=312, "EXP_PASSTHRU_MODE"=313, "EXP_FIRMWAREVERSION"=314, "EXP_IMMEDIATE_SHUTTER"=315, "EXP_STAGE2_TEMP"=316, "EXP_AVGAIN_ENABLED"=317, "EXP_AVGAIN_SETPOINT"=318, "EXP_AVGAIN"=319, "EXP_AVGAIN_CALIB_TEMP"=320, "EXP_AVGAIN_CALIB_COEFF1"=321, "EXP_AVGAIN_CALIB_COEFF2"=322, "EXP_AVGAIN_CALIB_COEFF3"=323, "EXP_AVGAIN_CALIB_COEFF4"=324, "EXP_AVGAIN_CALIB_COEFF5"=325, "EXP_FORCE_READOUT_MODE"=326, "EXP_RESET_DATACOLLECTION"=327, "EXP_ACTIVE_SUBFRAME"=328, "EXP_PV_READOUT_PORT"=514, "EXP_CLASSNAME"=775, "EXP_FLATFLDNAME"=776, "EXP_DARKNAME"=777, "EXP_SETUPNAME"=778, "EXP_ACCESSNAME"=779, "EXP_DATFILENAME"=780, "EXP_ABSORBFILENAME"=781, "EXP_BLEMISHFILENAME"=782, "EXP_COSMICFILENAME"=783, "EXP_FILEINCBASENAME"=784, "EXP_YTNAME"=785, "EXP_DEVNAME"=786, "EXP_USEROI"=787, "EXP_DOBLEMISH"=788, "EXP_DOABSORB"=789, "EXP_DOCOSMIC"=790, "EXP_COSMICSENS"=791, "EXP_ABSORBSTRIP"=792, "EXP_DATATYPE"=793, "EXP_OVERWRITECONFIRM"=794, "EXP_FILEINCENABLE"=795, "EXP_FILEINCCOUNT"=796, "EXP_RUNNING"=797, "EXP_SAVEROPT"=798, "EXP_TIME_UNITS"=799, "EXP_FILEACCESS"=800, "EXP_AUTOSAVE"=801, "EXP_NEWWINDOW"=802, "EXP_XDIM"=803, "EXP_YDIM"=804, "EXP_XDIMDET"=805, "EXP_YDIMDET"=806, "EXP_ROIMODE"=807, "EXP_NUMREPEATSEXP"=808, "EXP_NUMACCUMSEXP"=809, "EXP_THREADSTATE"=810, "EXP_USEMINTHRESHOLDING"=811, "EXP_MINTHRESHOLDVALUE"=812, "EXP_USEMAXTHRESHOLDING"=813, "EXP_MAXTHRESHOLDVALUE"=814, "EXP_RUNNING_EXPERIMENT"=815, "EXP_THRESHOLD_DEMAND_UPDATE"=816, "EXP_ROICOUNT"=817, "EXP_ACCUMS"=818, "EXP_CACCUMS"=819, "EXP_CSEQUENTS"=820, "EXP_PHOTON_ESTIMATION_ENABLE"=821, "EXP_PHOTON_MAXTIME"=822, "EXP_PHOTON_MAXTIMEUNIT"=823, "EXP_CUSTOMFILTER_ENABLE"=824, "EXP_CUSTOMFILTER_SIZE"=825, "EXP_LOOKUPTABLE_ENABLE"=826, "EXP_BSHOWWINDOW"=827, "EXP_BBACKSUBTRACT"=828, "EXP_BDOFLATFIELD"=829, "EXP_ASCIIOUTPUTFILE"=830, "EXP_ASCIIOUTPUT_DELIMITER"=831, "EXP_ASCIIOUTPUT_TERMINATOR"=832, "EXP_FFTYPE"=833, "EXP_BGTYPE"=834, "EXP_COSGRASS"=835, "EXP_RUNASCONFIRM"=836, "EXP_RUNASRUNACCESS"=837, "EXP_DATAFILETYPE"=838, "EXP_ROTATE"=839, "EXP_FLIP"=840, "EXP_REVERSE"=841, "EXP_SWBINNING"=842, "EXP_AUTOSTORE"=843, "EXP_XBINNED"=844, "EXP_YBINNED"=845, "EXP_NUMPATTERNS"=846, "EXP_EXPERIMENTTIME"=847, "EXP_ASYNCSEQUENTIALS"=848, "EXP_SEQUENTIALS"=849, "EXP_CSEQUENTIALS"=850, "EXP_AUTOD"=851, "EXP_EXPOSURETIME"=852, "EXP_EXPOSURETIME_UNITS"=853, "EXP_ACQMODE"=854, "EXP_DMASIZE_PVCAM"=855, "EXP_INITIALIZE"=856, "EXP_CELL_X_SIZE"=857, "EXP_CELL_Y_SIZE"=858, "EXP_X_GAP_SIZE"=859, "EXP_Y_GAP_SIZE"=860] ("Param")
                  # "acquire"
                  n165 = invoke class="IExpSetup2" method="GetParam"(reference=w221, "Param"=w224) -> (reference out=w219:refnum<k7>, "GetParam"=w225:variant)  [unwired: 3 in, 3 out]
                  n166 = local read "Stop measurement"() -> (w220:bool)
                  n167 = Variant To Data(type=FALSE, Variant=w225) -> (data=w226:bool)  [unwired: 1 in, 1 out]
                  n168 = Not(x=w226) -> (.not. x?=w222:bool)
                  n169 = Or(x=w222, y=w220) -> (x .or. y?=w227:bool)
                  n170 = Wait (ms)(milliseconds to wait=u32 5) -> ()  [unwired: 1 out]
                }
              }
              frame #2 {
                n171 = case shown="True" w230 {
                  tunnel: w229 -> [_ w249]
                  frame False {
                  }
                  frame True {
                    n172 = invoke class="IExpSetup2" method="Stop"(reference=w249) -> ()  [unwired: 2 in, 3 out]
                  }
                }
                n173 = local read "FrameVariant"() -> (w237:variant)
                n174 = invoke class="IDocFile" method="GetFrame"(reference=w236, "frame"=i16 1, "FrameVariant"=w237) -> (reference out=w246:refnum<k7>, "FrameVariant"=w248:variant)  [unwired: 2 in, 3 out]
                n175 = invoke class="IDocFile" method="GetCalibration"(reference=w246) -> ("GetCalibration"=w245:refnum<k7>)  [unwired: 2 in, 2 out]
                n176 = property class="ICalibObj"(reference=w245) -> (reference out=w243:refnum<k7>, "PairCount"=w244:u8)  [unwired: 1 in, 1 out]
                n177 = for {
                  N: w244 -> [_]
                  tunnel: w243 -> [w264]
                  tunnel: [w265] -> w240 mode=indexing
                  tunnel: [w262] -> w241 mode=indexing
                  i -> [w263]
                  n178 = invoke class="ICalibObj" method="CalibVal"(reference=w264, "index"=w263) -> ("CalibVal"=w265:dbl)  [unwired: 2 in, 3 out]
                  n179 = invoke class="ICalibObj" method="PixelLoc"(reference=w264, "index"=w263) -> ("PixelLoc"=w262:dbl)  [unwired: 2 in, 3 out]
                }
                n180 = local read "frame array"() -> (w235:i32[][])
                n181 = Variant To Data(type=w235, Variant=w248) -> (data=w232:i32[][])  [unwired: 1 in, 1 out]
                n182 = Index Array(array=w232, index (col)=0 ("disabled index (col)")) -> (element=w231:i32[])  [unwired: 1 in]
                n183 = Array Size(array=w231) -> (size(s)=w234:i32)
                n184 = for {
                  N: w234 -> [_]
                  tunnel: w240 -> [w261]
                  tunnel: [w260] -> w238 mode=indexing
                  tunnel: [w259] -> _ mode=indexing
                  tunnel: w241 -> [w258]
                  tunnel: 1 ("index") -> [w250]
                  i -> [w257]
                  n185 = Divide(x=w250, y=2) -> (x/y=w254:dbl)
                  n186 = Round To Nearest(number=w254) -> (nearest integer value=w252:dbl)
                  n187 = Multiply(x=w257, y=w250) -> (x*y=w253:i32)
                  n188 = Increment(x=w252) -> (x+1=w251:dbl)
                  n189 = Add(x=w253, y=w251) -> (x+y=w256:dbl)
                  n190 = call <vilib>:"Polynomial Interpolation.vi"("x value"=w256, "X"=w258, "Y"=w261) -> ("interpolation error"=w259:dbl, "interpolation value"=w260:dbl)  [unwired: 1 out]
                }
                n191 = local write "Wavelength Scale"(w238) -> ()
                n192 = Bundle(w238, "frame array"=w231) -> (w239:cluster{dbl[], "frame array":i32[]})  [unwired: 1 in]
                n193 = local write "XY Graph Spectrum"(w239) -> ()
              }
              frame #3 {
                n194 = local write "busy"(FALSE ("busy")) -> ()
                n195 = local write "Stop measurement"(FALSE ("Stop measurement")) -> ()
                n196 = local read "time start (ms)"() -> (w269:i32)
                n197 = Tick Count (ms)() -> (millisecond timer value=w270:u32)
                n198 = Subtract(x=w270, y=w269) -> (x-y=w268:u32)
                n199 = Divide(x=w268, y=u32 1000) -> (x/y=w266:dbl)
                n200 = local write "time elapsed (s)"(w266) -> ()
              }
            }
          }
          frame 11 {
            # "collect background spectrum"
            n201 = flat-sequence {
              frame #0 {
                w276 = 127 items=["EXP_ETACTUAL"=1, "EXP_SEQUENTS"=2, "EXP_ERROR"=3, "EXP_GETCAPS"=4, "EXP_GETPLSR"=5, "EXP_DETECTOR_BIT"=16, "EXP_RUNNING_APP"=23, "EXP_VIDEO_TYPE"=24, "EXP_CUSTOM_VIDEO_X"=25, "EXP_CUSTOM_VIDEO_Y"=26, "EXP_CUSTOM_VIDEO_FSTWIDTH"=27, "EXP_CUSTOM_VIDEO_LSTWIDTH"=28, "EXP_VIDEO_XDIM"=29, "EXP_VIDEO_YDIM"=30, "EXP_VIDEO_MAX_ZOOM"=31, "EXP_VIDEO_HORZ_PAN"=32, "EXP_VIDEO_VERT_PAN"=33, "EXP_WORD_MULTIPLIER"=34, "EXP_TARGET_ID"=35, "EXP_ADAPTER_ID"=36, "EXP_NUMADAPTORS"=37, "EXP_FORCE_PP_INIT"=38, "EXP_NOP_ADC"=39, "EXP_ACTUAL_TEMP"=40, "EXP_FORCE_AUTOSTOP"=41, "EXP_DEFAULT_VTCLK"=42, "EXP_MIN_VTCLK"=43, "EXP_MAX_VTCLK"=44, "EXP_DEFAULT_HTCLK"=45, "EXP_MIN_HTCLK"=46, "EXP_MAX_HTCLK"=47, "EXP_TIMING_STYLE"=48, "EXP_HEADSELECT"=49, "EXP_HORZPHASE"=50, "EXP_VERTPHASE"=51, "EXP_SPECIAL_SPEED"=52, "EXP_PRE_STRIPS"=53, "EXP_POST_STRIPS"=54, "EXP_PRE_LINES"=55, "EXP_POST_LINES"=56, "EXP_ACTIVE_LINES"=57, "EXP_ACTIVE_STRIPS"=58, "EXP_XFER_EXTRA"=59, "EXP_MIN_BLOCK"=60, "EXP_NUM_MIN_BLOCK"=61, "EXP_LOGIC_OUTPUT"=66, "EXP_VIDEO_BLANK"=67, "EXP_ZOOM_MODE_VIDEO"=68, "EXP_LEVEL_SYNC"=69, "EXP_DISABLE_LASER"=70, "EXP_ACQBACK_SHUTTER"=71, "EXP_ACQFLAT_SHUTTER"=72, "EXP_SMALL_CCD_MINEXP"=73, "EXP_LARGE_CCD_MINEXP"=74, "EXP_GATING_MODE"=75, "EXP_ILME_B1X"=76, "EXP_ILME_B2X"=77, "EXP_ILME_D1X"=78, "EXP_ILME_D2X"=79, "EXP_ILME_D4X"=80, "EXP_INIT_HW_ACCUM"=81, "EXP_5X_GAIN_ENABLE"=82, "EXP_RET_SRCCMP"=83, "EXP_EVENT_HANDLE"=84, "EXP_READOUT_MODE"=85, "EXP_SHUTTER_TYPE"=86, "EXP_USER_DEFINED_CHIP"=87, "EXP_USER_DEFINED_TIMING"=88, "EXP_CONTROLLER_VERSION"=89, "EXP_GET_CONTROLLER_VER"=90, "EXP_TTL_LINES"=91, "EXP_BIT_ADJUST"=92, "EXP_RESOLUTION"=93, "EXP_GAIN"=94, "EXP_ADC_RATE"=95, "EXP_ADC_TYPE"=96, "EXP_NUMBER_OF_CLEANS"=97, "EXP_NUM_OF_STRIPS_PER_CLN"=98, "EXP_INTERFACE_CARD"=99, "EXP_INTERRUPT"=100, "EXP_IO_ADDRESS1"=101, "EXP_IO_ADDRESS2"=102, "EXP_IO_ADDRESS3"=103, "EXP_HW_ROI"=104, "EXP_HW_BINNING"=105, "EXP_EDGE_TRIGGER"=106, "EXP_SHUTTER_CONTROL"=107, "EXP_RS170"=108, "EXP_RS170_COMPLEX"=109, "EXP_HW_RS170_LUT"=110, "EXP_RS170_INTENSITY_SCALING"=111, "EXP_RS170_OFFSET"=112, "EXP_RS170_PAN"=113, "EXP_RS170_ZOOM2X"=114, "EXP_RS170_ZOOM4X"=115, "EXP_RS170_BINNING"=116, "EXP_RS170_DECIMATION"=117, "EXP_HW_ACCUM"=118, "EXP_SHT_PREOPEN"=119, "EXP_STORE_STROBE"=120, "EXP_CONT_CLNS"=121, "EXP_TIMING_MODE"=122, "EXP_EXT_TRIGGER"=123, "EXP_EVENT_COUNTER"=124, "EXP_SW_TRIGGER"=125, "EXP_KINETICS_WINDOWSIZE"=126, "EXP_EXPOSURE"=127, "EXP_CONTROLLER_NAME"=128, "EXP_CCD_CHIP_NAME"=129, "EXP_BSWBINNING"=297, "EXP_EDGEENHANCE"=130, "EXP_BOXVIDEOGAIN"=131, "EXP_HSHADING_VALUE"=132, "EXP_VSHADING_VALUE"=133, "EXP_EDGEENHANCE_FLAG"=134, "EXP_SHADING_FLAG"=135, "EXP_GRAYSCALE"=136, "EXP_OFFSET"=137, "EXP_CCDGAIN"=138, "EXP_TEMPERATURE"=139, "EXP_MCPVOLTAGE"=140, "EXP_BOXEXPOSURE"=141, "EXP_ABC_FLAG"=142, "EXP_GAMMA_FLAG"=143, "EXP_AUTOBLACK_FLAG"=144, "EXP_AGC_FLAG"=145, "EXP_ODD_FIELD"=146, "EXP_FIELD_SELECT"=147, "EXP_RESET"=148, "EXP_EXTERN_ENABLE"=149, "EXP_CONTROLLERS_SUPPORTED"=150, "EXP_VTCLK"=151, "EXP_HTCLK"=152, "EXP_GATE_VS_CW"=153, "EXP_COM_PORT"=154, "EXP_US_UNITS"=156, "EXP_MS_UNITS"=157, "EXP_SEC_UNITS"=158, "EXP_MIN_UNITS"=159, "EXP_HRS_UNITS"=160, "EXP_FRAME_UNITS"=161, "EXP_SYNC_ASYNC"=162, "EXP_FOCUS_NFRAME"=163, "EXP_TIMEOUT"=164, "EXP_TIMEOUT_DEFAULT"=165, "EXP_HW_AUTOSTOP"=166, "EXP_RS170_INTEN_OFFSET"=167, "EXP_CONTROLLER_ALIVE"=168, "EXP_FOCUS_TYPE"=169, "EXP_FOCUS_ZOOM"=170, "EXP_FOCUS_PAN"=171, "EXP_MULTI_TAP_ROI"=172, "EXP_USE_INTERUPTS"=173, "EXP_DATA_ACQ_STATE"=174, "EXP_VERIFY_GOOD_VALUES"=175, "EXP_WHITE_CLAMP"=176, "EXP_BLACK_CLAMP"=177, "EXP_DELAY_TIME"=178, "EXP_READOUT_TIME"=179, "EXP_SW_DIAG"=180, "EXP_DIAG1"=181, "EXP_DIAG2"=182, "EXP_DIAG3"=183, "EXP_DIAG4"=184, "EXP_DIAG5"=185, "EXP_AorB_GROUP"=186, "EXP_ABSORBANCE_FLAG"=187, "EXP_ABSORBANCE_METHOD"=188, "EXP_ABSORBANCE_STRIPNUM"=189, "EXP_DMASIZE_VIA_DRIVER"=190, "EXP_DRIVERVERSION"=191, "EXP_NUM_DEVICES"=192, "EXP_ECPDMA_CHANNEL"=193, "EXP_CUSTOM_SHUTTER"=194, "EXP_ADC_OFFSET"=195, "EXP_CURRENT_READOUT_MODE"=196, "EXP_BANK_ADD"=197, "EXP_LUT_BANK"=198, "EXP_SETUP_STATUS"=201, "EXP_XY_GROUPING"=239, "EXP_MESSAGES_FLAG"=240, "EXP_TTL_LINE_TO_WAIT"=253, "EXP_DATA_COLLECTION_MODE"=258, "EXP_DATA_COLLECTION_TYPE"=262, "EXP_SKIPFRAMES"=274, "EXP_CLR_INT_CNTR"=276, "EXP_ENABLE_INT_CNTR"=277, "EXP_INT_CNTR"=278, "EXP_INTERNAL_SYNC_SRC"=279, "EXP_SW_EXTSYNC"=280, "EXP_PTG_PRESENT"=281, "EXP_ELEC_SHT"=282, "EXP_BOARDS_WITH_NVRAM"=283, "EXP_ANLGMASTER_ST143"=284, "EXP_ANLGSLAVE_ST143"=285, "EXP_DISPLAY_ST143"=286, "EXP_INTRFACE_ST143"=287, "EXP_SCANCONTROL_ST143"=288, "EXP_NUMBERFRAMES_IRQ"=204, "EXP_COOL_TYPE"=214, "EXP_HD_TYPE"=215, "EXP_INTENSIFER_GAIN"=216, "EXP_SHT_GATE_MODE"=217, "EXP_HD_CHECK"=218, "EXP_AMP_MODE"=219, "EXP_AMP_DIALOG"=247, "EXP_ANALOG_GAIN"=220, "EXP_HW_FIXES"=221, "EXP_PCI_CARDS"=222, "EXP_NOT_REVERSE"=223, "EXP_LOAD_NVRAM_DEFAULTS"=234, "EXP_CNTR_BRD"=235, "EXP_XDIMHW"=237, "EXP_YDIMHW"=238, "EXP_SPECIAL_FAST_RDOUT"=254, "EXP_SPCL_FAST_Y_DIM"=255, "EXP_SPCL_FAST_X_DIM"=256, "EXP_SPCL_FAST_Y_INDEX"=257, "EXP_SHUTTER_COMP_TIME_MS"=266, "EXP_NVRAM_AVAIL"=267, "EXP_NUMBER_AGAIN_AVAIL"=269, "EXP_SENSOR_TYPE"=270, "EXP_EVENT_TYPE"=292, "EXP_ANTI_BLOOMING"=293, "EXP_FAST_PULSE_ENABLE"=233, "EXP_USE_HEADCALIB"=296, "EXP_TEMP_STATUS"=301, "EXP_MULTIPLE_READMODES_LIVE"=302, "EXP_FIRST_ACQUIRE_FLAG"=303, "EXP_ANTI_BLOOMING_CONTROL"=304, "EXP_PRE_HORZ_DELAY"=305, "EXP_NVRAM_TRIES"=306, "EXP_XASCEND"=307, "EXP_YASCEND"=308, "EXP_ALT_TIMING"=309, "EXP_SHUTTER_PRE_COMP"=310, "EXP_PVCAM_POSSIBLE"=311, "EXP_ADC_IN_NVRAM"=312, "EXP_PASSTHRU_MODE"=313, "EXP_FIRMWAREVERSION"=314, "EXP_IMMEDIATE_SHUTTER"=315, "EXP_STAGE2_TEMP"=316, "EXP_AVGAIN_ENABLED"=317, "EXP_AVGAIN_SETPOINT"=318, "EXP_AVGAIN"=319, "EXP_AVGAIN_CALIB_TEMP"=320, "EXP_AVGAIN_CALIB_COEFF1"=321, "EXP_AVGAIN_CALIB_COEFF2"=322, "EXP_AVGAIN_CALIB_COEFF3"=323, "EXP_AVGAIN_CALIB_COEFF4"=324, "EXP_AVGAIN_CALIB_COEFF5"=325, "EXP_FORCE_READOUT_MODE"=326, "EXP_RESET_DATACOLLECTION"=327, "EXP_ACTIVE_SUBFRAME"=328, "EXP_PV_READOUT_PORT"=514, "EXP_CLASSNAME"=775, "EXP_FLATFLDNAME"=776, "EXP_DARKNAME"=777, "EXP_SETUPNAME"=778, "EXP_ACCESSNAME"=779, "EXP_DATFILENAME"=780, "EXP_ABSORBFILENAME"=781, "EXP_BLEMISHFILENAME"=782, "EXP_COSMICFILENAME"=783, "EXP_FILEINCBASENAME"=784, "EXP_YTNAME"=785, "EXP_DEVNAME"=786, "EXP_USEROI"=787, "EXP_DOBLEMISH"=788, "EXP_DOABSORB"=789, "EXP_DOCOSMIC"=790, "EXP_COSMICSENS"=791, "EXP_ABSORBSTRIP"=792, "EXP_DATATYPE"=793, "EXP_OVERWRITECONFIRM"=794, "EXP_FILEINCENABLE"=795, "EXP_FILEINCCOUNT"=796, "EXP_RUNNING"=797, "EXP_SAVEROPT"=798, "EXP_TIME_UNITS"=799, "EXP_FILEACCESS"=800, "EXP_AUTOSAVE"=801, "EXP_NEWWINDOW"=802, "EXP_XDIM"=803, "EXP_YDIM"=804, "EXP_XDIMDET"=805, "EXP_YDIMDET"=806, "EXP_ROIMODE"=807, "EXP_NUMREPEATSEXP"=808, "EXP_NUMACCUMSEXP"=809, "EXP_THREADSTATE"=810, "EXP_USEMINTHRESHOLDING"=811, "EXP_MINTHRESHOLDVALUE"=812, "EXP_USEMAXTHRESHOLDING"=813, "EXP_MAXTHRESHOLDVALUE"=814, "EXP_RUNNING_EXPERIMENT"=815, "EXP_THRESHOLD_DEMAND_UPDATE"=816, "EXP_ROICOUNT"=817, "EXP_ACCUMS"=818, "EXP_CACCUMS"=819, "EXP_CSEQUENTS"=820, "EXP_PHOTON_ESTIMATION_ENABLE"=821, "EXP_PHOTON_MAXTIME"=822, "EXP_PHOTON_MAXTIMEUNIT"=823, "EXP_CUSTOMFILTER_ENABLE"=824, "EXP_CUSTOMFILTER_SIZE"=825, "EXP_LOOKUPTABLE_ENABLE"=826, "EXP_BSHOWWINDOW"=827, "EXP_BBACKSUBTRACT"=828, "EXP_BDOFLATFIELD"=829, "EXP_ASCIIOUTPUTFILE"=830, "EXP_ASCIIOUTPUT_DELIMITER"=831, "EXP_ASCIIOUTPUT_TERMINATOR"=832, "EXP_FFTYPE"=833, "EXP_BGTYPE"=834, "EXP_COSGRASS"=835, "EXP_RUNASCONFIRM"=836, "EXP_RUNASRUNACCESS"=837, "EXP_DATAFILETYPE"=838, "EXP_ROTATE"=839, "EXP_FLIP"=840, "EXP_REVERSE"=841, "EXP_SWBINNING"=842, "EXP_AUTOSTORE"=843, "EXP_XBINNED"=844, "EXP_YBINNED"=845, "EXP_NUMPATTERNS"=846, "EXP_EXPERIMENTTIME"=847, "EXP_ASYNCSEQUENTIALS"=848, "EXP_SEQUENTIALS"=849, "EXP_CSEQUENTIALS"=850, "EXP_AUTOD"=851, "EXP_EXPOSURETIME"=852, "EXP_EXPOSURETIME_UNITS"=853, "EXP_ACQMODE"=854, "EXP_DMASIZE_PVCAM"=855, "EXP_INITIALIZE"=856, "EXP_CELL_X_SIZE"=857, "EXP_CELL_Y_SIZE"=858, "EXP_X_GAP_SIZE"=859, "EXP_Y_GAP_SIZE"=860] ("Param")
                w282 = 777 items=["EXP_ETACTUAL"=1, "EXP_SEQUENTS"=2, "EXP_ERROR"=3, "EXP_GETCAPS"=4, "EXP_GETPLSR"=5, "EXP_DETECTOR_BIT"=16, "EXP_RUNNING_APP"=23, "EXP_VIDEO_TYPE"=24, "EXP_CUSTOM_VIDEO_X"=25, "EXP_CUSTOM_VIDEO_Y"=26, "EXP_CUSTOM_VIDEO_FSTWIDTH"=27, "EXP_CUSTOM_VIDEO_LSTWIDTH"=28, "EXP_VIDEO_XDIM"=29, "EXP_VIDEO_YDIM"=30, "EXP_VIDEO_MAX_ZOOM"=31, "EXP_VIDEO_HORZ_PAN"=32, "EXP_VIDEO_VERT_PAN"=33, "EXP_WORD_MULTIPLIER"=34, "EXP_TARGET_ID"=35, "EXP_ADAPTER_ID"=36, "EXP_NUMADAPTORS"=37, "EXP_FORCE_PP_INIT"=38, "EXP_NOP_ADC"=39, "EXP_ACTUAL_TEMP"=40, "EXP_FORCE_AUTOSTOP"=41, "EXP_DEFAULT_VTCLK"=42, "EXP_MIN_VTCLK"=43, "EXP_MAX_VTCLK"=44, "EXP_DEFAULT_HTCLK"=45, "EXP_MIN_HTCLK"=46, "EXP_MAX_HTCLK"=47, "EXP_TIMING_STYLE"=48, "EXP_HEADSELECT"=49, "EXP_HORZPHASE"=50, "EXP_VERTPHASE"=51, "EXP_SPECIAL_SPEED"=52, "EXP_PRE_STRIPS"=53, "EXP_POST_STRIPS"=54, "EXP_PRE_LINES"=55, "EXP_POST_LINES"=56, "EXP_ACTIVE_LINES"=57, "EXP_ACTIVE_STRIPS"=58, "EXP_XFER_EXTRA"=59, "EXP_MIN_BLOCK"=60, "EXP_NUM_MIN_BLOCK"=61, "EXP_LOGIC_OUTPUT"=66, "EXP_VIDEO_BLANK"=67, "EXP_ZOOM_MODE_VIDEO"=68, "EXP_LEVEL_SYNC"=69, "EXP_DISABLE_LASER"=70, "EXP_ACQBACK_SHUTTER"=71, "EXP_ACQFLAT_SHUTTER"=72, "EXP_SMALL_CCD_MINEXP"=73, "EXP_LARGE_CCD_MINEXP"=74, "EXP_GATING_MODE"=75, "EXP_ILME_B1X"=76, "EXP_ILME_B2X"=77, "EXP_ILME_D1X"=78, "EXP_ILME_D2X"=79, "EXP_ILME_D4X"=80, "EXP_INIT_HW_ACCUM"=81, "EXP_5X_GAIN_ENABLE"=82, "EXP_RET_SRCCMP"=83, "EXP_EVENT_HANDLE"=84, "EXP_READOUT_MODE"=85, "EXP_SHUTTER_TYPE"=86, "EXP_USER_DEFINED_CHIP"=87, "EXP_USER_DEFINED_TIMING"=88, "EXP_CONTROLLER_VERSION"=89, "EXP_GET_CONTROLLER_VER"=90, "EXP_TTL_LINES"=91, "EXP_BIT_ADJUST"=92, "EXP_RESOLUTION"=93, "EXP_GAIN"=94, "EXP_ADC_RATE"=95, "EXP_ADC_TYPE"=96, "EXP_NUMBER_OF_CLEANS"=97, "EXP_NUM_OF_STRIPS_PER_CLN"=98, "EXP_INTERFACE_CARD"=99, "EXP_INTERRUPT"=100, "EXP_IO_ADDRESS1"=101, "EXP_IO_ADDRESS2"=102, "EXP_IO_ADDRESS3"=103, "EXP_HW_ROI"=104, "EXP_HW_BINNING"=105, "EXP_EDGE_TRIGGER"=106, "EXP_SHUTTER_CONTROL"=107, "EXP_RS170"=108, "EXP_RS170_COMPLEX"=109, "EXP_HW_RS170_LUT"=110, "EXP_RS170_INTENSITY_SCALING"=111, "EXP_RS170_OFFSET"=112, "EXP_RS170_PAN"=113, "EXP_RS170_ZOOM2X"=114, "EXP_RS170_ZOOM4X"=115, "EXP_RS170_BINNING"=116, "EXP_RS170_DECIMATION"=117, "EXP_HW_ACCUM"=118, "EXP_SHT_PREOPEN"=119, "EXP_STORE_STROBE"=120, "EXP_CONT_CLNS"=121, "EXP_TIMING_MODE"=122, "EXP_EXT_TRIGGER"=123, "EXP_EVENT_COUNTER"=124, "EXP_SW_TRIGGER"=125, "EXP_KINETICS_WINDOWSIZE"=126, "EXP_EXPOSURE"=127, "EXP_CONTROLLER_NAME"=128, "EXP_CCD_CHIP_NAME"=129, "EXP_BSWBINNING"=297, "EXP_EDGEENHANCE"=130, "EXP_BOXVIDEOGAIN"=131, "EXP_HSHADING_VALUE"=132, "EXP_VSHADING_VALUE"=133, "EXP_EDGEENHANCE_FLAG"=134, "EXP_SHADING_FLAG"=135, "EXP_GRAYSCALE"=136, "EXP_OFFSET"=137, "EXP_CCDGAIN"=138, "EXP_TEMPERATURE"=139, "EXP_MCPVOLTAGE"=140, "EXP_BOXEXPOSURE"=141, "EXP_ABC_FLAG"=142, "EXP_GAMMA_FLAG"=143, "EXP_AUTOBLACK_FLAG"=144, "EXP_AGC_FLAG"=145, "EXP_ODD_FIELD"=146, "EXP_FIELD_SELECT"=147, "EXP_RESET"=148, "EXP_EXTERN_ENABLE"=149, "EXP_CONTROLLERS_SUPPORTED"=150, "EXP_VTCLK"=151, "EXP_HTCLK"=152, "EXP_GATE_VS_CW"=153, "EXP_COM_PORT"=154, "EXP_US_UNITS"=156, "EXP_MS_UNITS"=157, "EXP_SEC_UNITS"=158, "EXP_MIN_UNITS"=159, "EXP_HRS_UNITS"=160, "EXP_FRAME_UNITS"=161, "EXP_SYNC_ASYNC"=162, "EXP_FOCUS_NFRAME"=163, "EXP_TIMEOUT"=164, "EXP_TIMEOUT_DEFAULT"=165, "EXP_HW_AUTOSTOP"=166, "EXP_RS170_INTEN_OFFSET"=167, "EXP_CONTROLLER_ALIVE"=168, "EXP_FOCUS_TYPE"=169, "EXP_FOCUS_ZOOM"=170, "EXP_FOCUS_PAN"=171, "EXP_MULTI_TAP_ROI"=172, "EXP_USE_INTERUPTS"=173, "EXP_DATA_ACQ_STATE"=174, "EXP_VERIFY_GOOD_VALUES"=175, "EXP_WHITE_CLAMP"=176, "EXP_BLACK_CLAMP"=177, "EXP_DELAY_TIME"=178, "EXP_READOUT_TIME"=179, "EXP_SW_DIAG"=180, "EXP_DIAG1"=181, "EXP_DIAG2"=182, "EXP_DIAG3"=183, "EXP_DIAG4"=184, "EXP_DIAG5"=185, "EXP_AorB_GROUP"=186, "EXP_ABSORBANCE_FLAG"=187, "EXP_ABSORBANCE_METHOD"=188, "EXP_ABSORBANCE_STRIPNUM"=189, "EXP_DMASIZE_VIA_DRIVER"=190, "EXP_DRIVERVERSION"=191, "EXP_NUM_DEVICES"=192, "EXP_ECPDMA_CHANNEL"=193, "EXP_CUSTOM_SHUTTER"=194, "EXP_ADC_OFFSET"=195, "EXP_CURRENT_READOUT_MODE"=196, "EXP_BANK_ADD"=197, "EXP_LUT_BANK"=198, "EXP_SETUP_STATUS"=201, "EXP_XY_GROUPING"=239, "EXP_MESSAGES_FLAG"=240, "EXP_TTL_LINE_TO_WAIT"=253, "EXP_DATA_COLLECTION_MODE"=258, "EXP_DATA_COLLECTION_TYPE"=262, "EXP_SKIPFRAMES"=274, "EXP_CLR_INT_CNTR"=276, "EXP_ENABLE_INT_CNTR"=277, "EXP_INT_CNTR"=278, "EXP_INTERNAL_SYNC_SRC"=279, "EXP_SW_EXTSYNC"=280, "EXP_PTG_PRESENT"=281, "EXP_ELEC_SHT"=282, "EXP_BOARDS_WITH_NVRAM"=283, "EXP_ANLGMASTER_ST143"=284, "EXP_ANLGSLAVE_ST143"=285, "EXP_DISPLAY_ST143"=286, "EXP_INTRFACE_ST143"=287, "EXP_SCANCONTROL_ST143"=288, "EXP_NUMBERFRAMES_IRQ"=204, "EXP_COOL_TYPE"=214, "EXP_HD_TYPE"=215, "EXP_INTENSIFER_GAIN"=216, "EXP_SHT_GATE_MODE"=217, "EXP_HD_CHECK"=218, "EXP_AMP_MODE"=219, "EXP_AMP_DIALOG"=247, "EXP_ANALOG_GAIN"=220, "EXP_HW_FIXES"=221, "EXP_PCI_CARDS"=222, "EXP_NOT_REVERSE"=223, "EXP_LOAD_NVRAM_DEFAULTS"=234, "EXP_CNTR_BRD"=235, "EXP_XDIMHW"=237, "EXP_YDIMHW"=238, "EXP_SPECIAL_FAST_RDOUT"=254, "EXP_SPCL_FAST_Y_DIM"=255, "EXP_SPCL_FAST_X_DIM"=256, "EXP_SPCL_FAST_Y_INDEX"=257, "EXP_SHUTTER_COMP_TIME_MS"=266, "EXP_NVRAM_AVAIL"=267, "EXP_NUMBER_AGAIN_AVAIL"=269, "EXP_SENSOR_TYPE"=270, "EXP_EVENT_TYPE"=292, "EXP_ANTI_BLOOMING"=293, "EXP_FAST_PULSE_ENABLE"=233, "EXP_USE_HEADCALIB"=296, "EXP_TEMP_STATUS"=301, "EXP_MULTIPLE_READMODES_LIVE"=302, "EXP_FIRST_ACQUIRE_FLAG"=303, "EXP_ANTI_BLOOMING_CONTROL"=304, "EXP_PRE_HORZ_DELAY"=305, "EXP_NVRAM_TRIES"=306, "EXP_XASCEND"=307, "EXP_YASCEND"=308, "EXP_ALT_TIMING"=309, "EXP_SHUTTER_PRE_COMP"=310, "EXP_PVCAM_POSSIBLE"=311, "EXP_ADC_IN_NVRAM"=312, "EXP_PASSTHRU_MODE"=313, "EXP_FIRMWAREVERSION"=314, "EXP_IMMEDIATE_SHUTTER"=315, "EXP_STAGE2_TEMP"=316, "EXP_AVGAIN_ENABLED"=317, "EXP_AVGAIN_SETPOINT"=318, "EXP_AVGAIN"=319, "EXP_AVGAIN_CALIB_TEMP"=320, "EXP_AVGAIN_CALIB_COEFF1"=321, "EXP_AVGAIN_CALIB_COEFF2"=322, "EXP_AVGAIN_CALIB_COEFF3"=323, "EXP_AVGAIN_CALIB_COEFF4"=324, "EXP_AVGAIN_CALIB_COEFF5"=325, "EXP_FORCE_READOUT_MODE"=326, "EXP_RESET_DATACOLLECTION"=327, "EXP_ACTIVE_SUBFRAME"=328, "EXP_PV_READOUT_PORT"=514, "EXP_CLASSNAME"=775, "EXP_FLATFLDNAME"=776, "EXP_DARKNAME"=777, "EXP_SETUPNAME"=778, "EXP_ACCESSNAME"=779, "EXP_DATFILENAME"=780, "EXP_ABSORBFILENAME"=781, "EXP_BLEMISHFILENAME"=782, "EXP_COSMICFILENAME"=783, "EXP_FILEINCBASENAME"=784, "EXP_YTNAME"=785, "EXP_DEVNAME"=786, "EXP_USEROI"=787, "EXP_DOBLEMISH"=788, "EXP_DOABSORB"=789, "EXP_DOCOSMIC"=790, "EXP_COSMICSENS"=791, "EXP_ABSORBSTRIP"=792, "EXP_DATATYPE"=793, "EXP_OVERWRITECONFIRM"=794, "EXP_FILEINCENABLE"=795, "EXP_FILEINCCOUNT"=796, "EXP_RUNNING"=797, "EXP_SAVEROPT"=798, "EXP_TIME_UNITS"=799, "EXP_FILEACCESS"=800, "EXP_AUTOSAVE"=801, "EXP_NEWWINDOW"=802, "EXP_XDIM"=803, "EXP_YDIM"=804, "EXP_XDIMDET"=805, "EXP_YDIMDET"=806, "EXP_ROIMODE"=807, "EXP_NUMREPEATSEXP"=808, "EXP_NUMACCUMSEXP"=809, "EXP_THREADSTATE"=810, "EXP_USEMINTHRESHOLDING"=811, "EXP_MINTHRESHOLDVALUE"=812, "EXP_USEMAXTHRESHOLDING"=813, "EXP_MAXTHRESHOLDVALUE"=814, "EXP_RUNNING_EXPERIMENT"=815, "EXP_THRESHOLD_DEMAND_UPDATE"=816, "EXP_ROICOUNT"=817, "EXP_ACCUMS"=818, "EXP_CACCUMS"=819, "EXP_CSEQUENTS"=820, "EXP_PHOTON_ESTIMATION_ENABLE"=821, "EXP_PHOTON_MAXTIME"=822, "EXP_PHOTON_MAXTIMEUNIT"=823, "EXP_CUSTOMFILTER_ENABLE"=824, "EXP_CUSTOMFILTER_SIZE"=825, "EXP_LOOKUPTABLE_ENABLE"=826, "EXP_BSHOWWINDOW"=827, "EXP_BBACKSUBTRACT"=828, "EXP_BDOFLATFIELD"=829, "EXP_ASCIIOUTPUTFILE"=830, "EXP_ASCIIOUTPUT_DELIMITER"=831, "EXP_ASCIIOUTPUT_TERMINATOR"=832, "EXP_FFTYPE"=833, "EXP_BGTYPE"=834, "EXP_COSGRASS"=835, "EXP_RUNASCONFIRM"=836, "EXP_RUNASRUNACCESS"=837, "EXP_DATAFILETYPE"=838, "EXP_ROTATE"=839, "EXP_FLIP"=840, "EXP_REVERSE"=841, "EXP_SWBINNING"=842, "EXP_AUTOSTORE"=843, "EXP_XBINNED"=844, "EXP_YBINNED"=845, "EXP_NUMPATTERNS"=846, "EXP_EXPERIMENTTIME"=847, "EXP_ASYNCSEQUENTIALS"=848, "EXP_SEQUENTIALS"=849, "EXP_CSEQUENTIALS"=850, "EXP_AUTOD"=851, "EXP_EXPOSURETIME"=852, "EXP_EXPOSURETIME_UNITS"=853, "EXP_ACQMODE"=854, "EXP_DMASIZE_PVCAM"=855, "EXP_INITIALIZE"=856, "EXP_CELL_X_SIZE"=857, "EXP_CELL_Y_SIZE"=858, "EXP_X_GAP_SIZE"=859, "EXP_Y_GAP_SIZE"=860] ("Param")
                n202 = local read "OMA V exposure time"() -> (w277:dbl)
                n203 = local read "experiment reference"() -> (w274:refnum<k7>)
                n204 = invoke class="IExpSetup2" method="SetParam"(reference=w274, "Param"=w276, "pSetVal"=w277) -> (reference out=w275:refnum<k7>)  [unwired: 2 in, 4 out]
                n205 = invoke class="IExpSetup2" method="SetParam"(reference=w275, "Param"=w282, "pSetVal"=path "C:/Users/Yuriy/bkgOMAV" ("Full File Name\nfor Acqure")) -> (reference out=w281:refnum<k7>)  [unwired: 2 in, 4 out]
                n206 = invoke class="IExpSetup2" method="AcquireBackground"(reference=w281) -> (reference out=w278:refnum<k7>)  [unwired: 2 in, 2 out]
                n207 = while {
                  tunnel: w278 -> [w285]
                  tunnel: [w284] -> w279
                  tunnel: [w283] -> w273
                  stop <- w291 stop-if-true
                  w287 = 797 items=["EXP_ETACTUAL"=1, "EXP_SEQUENTS"=2, "EXP_ERROR"=3, "EXP_GETCAPS"=4, "EXP_GETPLSR"=5, "EXP_DETECTOR_BIT"=16, "EXP_RUNNING_APP"=23, "EXP_VIDEO_TYPE"=24, "EXP_CUSTOM_VIDEO_X"=25, "EXP_CUSTOM_VIDEO_Y"=26, "EXP_CUSTOM_VIDEO_FSTWIDTH"=27, "EXP_CUSTOM_VIDEO_LSTWIDTH"=28, "EXP_VIDEO_XDIM"=29, "EXP_VIDEO_YDIM"=30, "EXP_VIDEO_MAX_ZOOM"=31, "EXP_VIDEO_HORZ_PAN"=32, "EXP_VIDEO_VERT_PAN"=33, "EXP_WORD_MULTIPLIER"=34, "EXP_TARGET_ID"=35, "EXP_ADAPTER_ID"=36, "EXP_NUMADAPTORS"=37, "EXP_FORCE_PP_INIT"=38, "EXP_NOP_ADC"=39, "EXP_ACTUAL_TEMP"=40, "EXP_FORCE_AUTOSTOP"=41, "EXP_DEFAULT_VTCLK"=42, "EXP_MIN_VTCLK"=43, "EXP_MAX_VTCLK"=44, "EXP_DEFAULT_HTCLK"=45, "EXP_MIN_HTCLK"=46, "EXP_MAX_HTCLK"=47, "EXP_TIMING_STYLE"=48, "EXP_HEADSELECT"=49, "EXP_HORZPHASE"=50, "EXP_VERTPHASE"=51, "EXP_SPECIAL_SPEED"=52, "EXP_PRE_STRIPS"=53, "EXP_POST_STRIPS"=54, "EXP_PRE_LINES"=55, "EXP_POST_LINES"=56, "EXP_ACTIVE_LINES"=57, "EXP_ACTIVE_STRIPS"=58, "EXP_XFER_EXTRA"=59, "EXP_MIN_BLOCK"=60, "EXP_NUM_MIN_BLOCK"=61, "EXP_LOGIC_OUTPUT"=66, "EXP_VIDEO_BLANK"=67, "EXP_ZOOM_MODE_VIDEO"=68, "EXP_LEVEL_SYNC"=69, "EXP_DISABLE_LASER"=70, "EXP_ACQBACK_SHUTTER"=71, "EXP_ACQFLAT_SHUTTER"=72, "EXP_SMALL_CCD_MINEXP"=73, "EXP_LARGE_CCD_MINEXP"=74, "EXP_GATING_MODE"=75, "EXP_ILME_B1X"=76, "EXP_ILME_B2X"=77, "EXP_ILME_D1X"=78, "EXP_ILME_D2X"=79, "EXP_ILME_D4X"=80, "EXP_INIT_HW_ACCUM"=81, "EXP_5X_GAIN_ENABLE"=82, "EXP_RET_SRCCMP"=83, "EXP_EVENT_HANDLE"=84, "EXP_READOUT_MODE"=85, "EXP_SHUTTER_TYPE"=86, "EXP_USER_DEFINED_CHIP"=87, "EXP_USER_DEFINED_TIMING"=88, "EXP_CONTROLLER_VERSION"=89, "EXP_GET_CONTROLLER_VER"=90, "EXP_TTL_LINES"=91, "EXP_BIT_ADJUST"=92, "EXP_RESOLUTION"=93, "EXP_GAIN"=94, "EXP_ADC_RATE"=95, "EXP_ADC_TYPE"=96, "EXP_NUMBER_OF_CLEANS"=97, "EXP_NUM_OF_STRIPS_PER_CLN"=98, "EXP_INTERFACE_CARD"=99, "EXP_INTERRUPT"=100, "EXP_IO_ADDRESS1"=101, "EXP_IO_ADDRESS2"=102, "EXP_IO_ADDRESS3"=103, "EXP_HW_ROI"=104, "EXP_HW_BINNING"=105, "EXP_EDGE_TRIGGER"=106, "EXP_SHUTTER_CONTROL"=107, "EXP_RS170"=108, "EXP_RS170_COMPLEX"=109, "EXP_HW_RS170_LUT"=110, "EXP_RS170_INTENSITY_SCALING"=111, "EXP_RS170_OFFSET"=112, "EXP_RS170_PAN"=113, "EXP_RS170_ZOOM2X"=114, "EXP_RS170_ZOOM4X"=115, "EXP_RS170_BINNING"=116, "EXP_RS170_DECIMATION"=117, "EXP_HW_ACCUM"=118, "EXP_SHT_PREOPEN"=119, "EXP_STORE_STROBE"=120, "EXP_CONT_CLNS"=121, "EXP_TIMING_MODE"=122, "EXP_EXT_TRIGGER"=123, "EXP_EVENT_COUNTER"=124, "EXP_SW_TRIGGER"=125, "EXP_KINETICS_WINDOWSIZE"=126, "EXP_EXPOSURE"=127, "EXP_CONTROLLER_NAME"=128, "EXP_CCD_CHIP_NAME"=129, "EXP_BSWBINNING"=297, "EXP_EDGEENHANCE"=130, "EXP_BOXVIDEOGAIN"=131, "EXP_HSHADING_VALUE"=132, "EXP_VSHADING_VALUE"=133, "EXP_EDGEENHANCE_FLAG"=134, "EXP_SHADING_FLAG"=135, "EXP_GRAYSCALE"=136, "EXP_OFFSET"=137, "EXP_CCDGAIN"=138, "EXP_TEMPERATURE"=139, "EXP_MCPVOLTAGE"=140, "EXP_BOXEXPOSURE"=141, "EXP_ABC_FLAG"=142, "EXP_GAMMA_FLAG"=143, "EXP_AUTOBLACK_FLAG"=144, "EXP_AGC_FLAG"=145, "EXP_ODD_FIELD"=146, "EXP_FIELD_SELECT"=147, "EXP_RESET"=148, "EXP_EXTERN_ENABLE"=149, "EXP_CONTROLLERS_SUPPORTED"=150, "EXP_VTCLK"=151, "EXP_HTCLK"=152, "EXP_GATE_VS_CW"=153, "EXP_COM_PORT"=154, "EXP_US_UNITS"=156, "EXP_MS_UNITS"=157, "EXP_SEC_UNITS"=158, "EXP_MIN_UNITS"=159, "EXP_HRS_UNITS"=160, "EXP_FRAME_UNITS"=161, "EXP_SYNC_ASYNC"=162, "EXP_FOCUS_NFRAME"=163, "EXP_TIMEOUT"=164, "EXP_TIMEOUT_DEFAULT"=165, "EXP_HW_AUTOSTOP"=166, "EXP_RS170_INTEN_OFFSET"=167, "EXP_CONTROLLER_ALIVE"=168, "EXP_FOCUS_TYPE"=169, "EXP_FOCUS_ZOOM"=170, "EXP_FOCUS_PAN"=171, "EXP_MULTI_TAP_ROI"=172, "EXP_USE_INTERUPTS"=173, "EXP_DATA_ACQ_STATE"=174, "EXP_VERIFY_GOOD_VALUES"=175, "EXP_WHITE_CLAMP"=176, "EXP_BLACK_CLAMP"=177, "EXP_DELAY_TIME"=178, "EXP_READOUT_TIME"=179, "EXP_SW_DIAG"=180, "EXP_DIAG1"=181, "EXP_DIAG2"=182, "EXP_DIAG3"=183, "EXP_DIAG4"=184, "EXP_DIAG5"=185, "EXP_AorB_GROUP"=186, "EXP_ABSORBANCE_FLAG"=187, "EXP_ABSORBANCE_METHOD"=188, "EXP_ABSORBANCE_STRIPNUM"=189, "EXP_DMASIZE_VIA_DRIVER"=190, "EXP_DRIVERVERSION"=191, "EXP_NUM_DEVICES"=192, "EXP_ECPDMA_CHANNEL"=193, "EXP_CUSTOM_SHUTTER"=194, "EXP_ADC_OFFSET"=195, "EXP_CURRENT_READOUT_MODE"=196, "EXP_BANK_ADD"=197, "EXP_LUT_BANK"=198, "EXP_SETUP_STATUS"=201, "EXP_XY_GROUPING"=239, "EXP_MESSAGES_FLAG"=240, "EXP_TTL_LINE_TO_WAIT"=253, "EXP_DATA_COLLECTION_MODE"=258, "EXP_DATA_COLLECTION_TYPE"=262, "EXP_SKIPFRAMES"=274, "EXP_CLR_INT_CNTR"=276, "EXP_ENABLE_INT_CNTR"=277, "EXP_INT_CNTR"=278, "EXP_INTERNAL_SYNC_SRC"=279, "EXP_SW_EXTSYNC"=280, "EXP_PTG_PRESENT"=281, "EXP_ELEC_SHT"=282, "EXP_BOARDS_WITH_NVRAM"=283, "EXP_ANLGMASTER_ST143"=284, "EXP_ANLGSLAVE_ST143"=285, "EXP_DISPLAY_ST143"=286, "EXP_INTRFACE_ST143"=287, "EXP_SCANCONTROL_ST143"=288, "EXP_NUMBERFRAMES_IRQ"=204, "EXP_COOL_TYPE"=214, "EXP_HD_TYPE"=215, "EXP_INTENSIFER_GAIN"=216, "EXP_SHT_GATE_MODE"=217, "EXP_HD_CHECK"=218, "EXP_AMP_MODE"=219, "EXP_AMP_DIALOG"=247, "EXP_ANALOG_GAIN"=220, "EXP_HW_FIXES"=221, "EXP_PCI_CARDS"=222, "EXP_NOT_REVERSE"=223, "EXP_LOAD_NVRAM_DEFAULTS"=234, "EXP_CNTR_BRD"=235, "EXP_XDIMHW"=237, "EXP_YDIMHW"=238, "EXP_SPECIAL_FAST_RDOUT"=254, "EXP_SPCL_FAST_Y_DIM"=255, "EXP_SPCL_FAST_X_DIM"=256, "EXP_SPCL_FAST_Y_INDEX"=257, "EXP_SHUTTER_COMP_TIME_MS"=266, "EXP_NVRAM_AVAIL"=267, "EXP_NUMBER_AGAIN_AVAIL"=269, "EXP_SENSOR_TYPE"=270, "EXP_EVENT_TYPE"=292, "EXP_ANTI_BLOOMING"=293, "EXP_FAST_PULSE_ENABLE"=233, "EXP_USE_HEADCALIB"=296, "EXP_TEMP_STATUS"=301, "EXP_MULTIPLE_READMODES_LIVE"=302, "EXP_FIRST_ACQUIRE_FLAG"=303, "EXP_ANTI_BLOOMING_CONTROL"=304, "EXP_PRE_HORZ_DELAY"=305, "EXP_NVRAM_TRIES"=306, "EXP_XASCEND"=307, "EXP_YASCEND"=308, "EXP_ALT_TIMING"=309, "EXP_SHUTTER_PRE_COMP"=310, "EXP_PVCAM_POSSIBLE"=311, "EXP_ADC_IN_NVRAM"=312, "EXP_PASSTHRU_MODE"=313, "EXP_FIRMWAREVERSION"=314, "EXP_IMMEDIATE_SHUTTER"=315, "EXP_STAGE2_TEMP"=316, "EXP_AVGAIN_ENABLED"=317, "EXP_AVGAIN_SETPOINT"=318, "EXP_AVGAIN"=319, "EXP_AVGAIN_CALIB_TEMP"=320, "EXP_AVGAIN_CALIB_COEFF1"=321, "EXP_AVGAIN_CALIB_COEFF2"=322, "EXP_AVGAIN_CALIB_COEFF3"=323, "EXP_AVGAIN_CALIB_COEFF4"=324, "EXP_AVGAIN_CALIB_COEFF5"=325, "EXP_FORCE_READOUT_MODE"=326, "EXP_RESET_DATACOLLECTION"=327, "EXP_ACTIVE_SUBFRAME"=328, "EXP_PV_READOUT_PORT"=514, "EXP_CLASSNAME"=775, "EXP_FLATFLDNAME"=776, "EXP_DARKNAME"=777, "EXP_SETUPNAME"=778, "EXP_ACCESSNAME"=779, "EXP_DATFILENAME"=780, "EXP_ABSORBFILENAME"=781, "EXP_BLEMISHFILENAME"=782, "EXP_COSMICFILENAME"=783, "EXP_FILEINCBASENAME"=784, "EXP_YTNAME"=785, "EXP_DEVNAME"=786, "EXP_USEROI"=787, "EXP_DOBLEMISH"=788, "EXP_DOABSORB"=789, "EXP_DOCOSMIC"=790, "EXP_COSMICSENS"=791, "EXP_ABSORBSTRIP"=792, "EXP_DATATYPE"=793, "EXP_OVERWRITECONFIRM"=794, "EXP_FILEINCENABLE"=795, "EXP_FILEINCCOUNT"=796, "EXP_RUNNING"=797, "EXP_SAVEROPT"=798, "EXP_TIME_UNITS"=799, "EXP_FILEACCESS"=800, "EXP_AUTOSAVE"=801, "EXP_NEWWINDOW"=802, "EXP_XDIM"=803, "EXP_YDIM"=804, "EXP_XDIMDET"=805, "EXP_YDIMDET"=806, "EXP_ROIMODE"=807, "EXP_NUMREPEATSEXP"=808, "EXP_NUMACCUMSEXP"=809, "EXP_THREADSTATE"=810, "EXP_USEMINTHRESHOLDING"=811, "EXP_MINTHRESHOLDVALUE"=812, "EXP_USEMAXTHRESHOLDING"=813, "EXP_MAXTHRESHOLDVALUE"=814, "EXP_RUNNING_EXPERIMENT"=815, "EXP_THRESHOLD_DEMAND_UPDATE"=816, "EXP_ROICOUNT"=817, "EXP_ACCUMS"=818, "EXP_CACCUMS"=819, "EXP_CSEQUENTS"=820, "EXP_PHOTON_ESTIMATION_ENABLE"=821, "EXP_PHOTON_MAXTIME"=822, "EXP_PHOTON_MAXTIMEUNIT"=823, "EXP_CUSTOMFILTER_ENABLE"=824, "EXP_CUSTOMFILTER_SIZE"=825, "EXP_LOOKUPTABLE_ENABLE"=826, "EXP_BSHOWWINDOW"=827, "EXP_BBACKSUBTRACT"=828, "EXP_BDOFLATFIELD"=829, "EXP_ASCIIOUTPUTFILE"=830, "EXP_ASCIIOUTPUT_DELIMITER"=831, "EXP_ASCIIOUTPUT_TERMINATOR"=832, "EXP_FFTYPE"=833, "EXP_BGTYPE"=834, "EXP_COSGRASS"=835, "EXP_RUNASCONFIRM"=836, "EXP_RUNASRUNACCESS"=837, "EXP_DATAFILETYPE"=838, "EXP_ROTATE"=839, "EXP_FLIP"=840, "EXP_REVERSE"=841, "EXP_SWBINNING"=842, "EXP_AUTOSTORE"=843, "EXP_XBINNED"=844, "EXP_YBINNED"=845, "EXP_NUMPATTERNS"=846, "EXP_EXPERIMENTTIME"=847, "EXP_ASYNCSEQUENTIALS"=848, "EXP_SEQUENTIALS"=849, "EXP_CSEQUENTIALS"=850, "EXP_AUTOD"=851, "EXP_EXPOSURETIME"=852, "EXP_EXPOSURETIME_UNITS"=853, "EXP_ACQMODE"=854, "EXP_DMASIZE_PVCAM"=855, "EXP_INITIALIZE"=856, "EXP_CELL_X_SIZE"=857, "EXP_CELL_Y_SIZE"=858, "EXP_X_GAP_SIZE"=859, "EXP_Y_GAP_SIZE"=860] ("Param")
                  # "acquire"
                  n208 = invoke class="IExpSetup2" method="GetParam"(reference=w285, "Param"=w287) -> (reference out=w283:refnum<k7>, "GetParam"=w288:variant)  [unwired: 3 in, 3 out]
                  n209 = Variant To Data(type=FALSE, Variant=w288) -> (data=w289:bool)  [unwired: 1 in, 1 out]
                  n210 = local read "Stop measurement"() -> (w290:bool)
                  n211 = Not(x=w289) -> (.not. x?=w284:bool)
                  n212 = Or(x=w284, y=w290) -> (x .or. y?=w291:bool)
                  n213 = Wait (ms)(milliseconds to wait=u32 5) -> ()  [unwired: 1 out]
                }
                n214 = case shown="True" w279 {
                  tunnel: w273 -> [_ w293]
                  frame False {
                  }
                  frame True {
                    w295 = 828 items=["EXP_ETACTUAL"=1, "EXP_SEQUENTS"=2, "EXP_ERROR"=3, "EXP_GETCAPS"=4, "EXP_GETPLSR"=5, "EXP_DETECTOR_BIT"=16, "EXP_RUNNING_APP"=23, "EXP_VIDEO_TYPE"=24, "EXP_CUSTOM_VIDEO_X"=25, "EXP_CUSTOM_VIDEO_Y"=26, "EXP_CUSTOM_VIDEO_FSTWIDTH"=27, "EXP_CUSTOM_VIDEO_LSTWIDTH"=28, "EXP_VIDEO_XDIM"=29, "EXP_VIDEO_YDIM"=30, "EXP_VIDEO_MAX_ZOOM"=31, "EXP_VIDEO_HORZ_PAN"=32, "EXP_VIDEO_VERT_PAN"=33, "EXP_WORD_MULTIPLIER"=34, "EXP_TARGET_ID"=35, "EXP_ADAPTER_ID"=36, "EXP_NUMADAPTORS"=37, "EXP_FORCE_PP_INIT"=38, "EXP_NOP_ADC"=39, "EXP_ACTUAL_TEMP"=40, "EXP_FORCE_AUTOSTOP"=41, "EXP_DEFAULT_VTCLK"=42, "EXP_MIN_VTCLK"=43, "EXP_MAX_VTCLK"=44, "EXP_DEFAULT_HTCLK"=45, "EXP_MIN_HTCLK"=46, "EXP_MAX_HTCLK"=47, "EXP_TIMING_STYLE"=48, "EXP_HEADSELECT"=49, "EXP_HORZPHASE"=50, "EXP_VERTPHASE"=51, "EXP_SPECIAL_SPEED"=52, "EXP_PRE_STRIPS"=53, "EXP_POST_STRIPS"=54, "EXP_PRE_LINES"=55, "EXP_POST_LINES"=56, "EXP_ACTIVE_LINES"=57, "EXP_ACTIVE_STRIPS"=58, "EXP_XFER_EXTRA"=59, "EXP_MIN_BLOCK"=60, "EXP_NUM_MIN_BLOCK"=61, "EXP_LOGIC_OUTPUT"=66, "EXP_VIDEO_BLANK"=67, "EXP_ZOOM_MODE_VIDEO"=68, "EXP_LEVEL_SYNC"=69, "EXP_DISABLE_LASER"=70, "EXP_ACQBACK_SHUTTER"=71, "EXP_ACQFLAT_SHUTTER"=72, "EXP_SMALL_CCD_MINEXP"=73, "EXP_LARGE_CCD_MINEXP"=74, "EXP_GATING_MODE"=75, "EXP_ILME_B1X"=76, "EXP_ILME_B2X"=77, "EXP_ILME_D1X"=78, "EXP_ILME_D2X"=79, "EXP_ILME_D4X"=80, "EXP_INIT_HW_ACCUM"=81, "EXP_5X_GAIN_ENABLE"=82, "EXP_RET_SRCCMP"=83, "EXP_EVENT_HANDLE"=84, "EXP_READOUT_MODE"=85, "EXP_SHUTTER_TYPE"=86, "EXP_USER_DEFINED_CHIP"=87, "EXP_USER_DEFINED_TIMING"=88, "EXP_CONTROLLER_VERSION"=89, "EXP_GET_CONTROLLER_VER"=90, "EXP_TTL_LINES"=91, "EXP_BIT_ADJUST"=92, "EXP_RESOLUTION"=93, "EXP_GAIN"=94, "EXP_ADC_RATE"=95, "EXP_ADC_TYPE"=96, "EXP_NUMBER_OF_CLEANS"=97, "EXP_NUM_OF_STRIPS_PER_CLN"=98, "EXP_INTERFACE_CARD"=99, "EXP_INTERRUPT"=100, "EXP_IO_ADDRESS1"=101, "EXP_IO_ADDRESS2"=102, "EXP_IO_ADDRESS3"=103, "EXP_HW_ROI"=104, "EXP_HW_BINNING"=105, "EXP_EDGE_TRIGGER"=106, "EXP_SHUTTER_CONTROL"=107, "EXP_RS170"=108, "EXP_RS170_COMPLEX"=109, "EXP_HW_RS170_LUT"=110, "EXP_RS170_INTENSITY_SCALING"=111, "EXP_RS170_OFFSET"=112, "EXP_RS170_PAN"=113, "EXP_RS170_ZOOM2X"=114, "EXP_RS170_ZOOM4X"=115, "EXP_RS170_BINNING"=116, "EXP_RS170_DECIMATION"=117, "EXP_HW_ACCUM"=118, "EXP_SHT_PREOPEN"=119, "EXP_STORE_STROBE"=120, "EXP_CONT_CLNS"=121, "EXP_TIMING_MODE"=122, "EXP_EXT_TRIGGER"=123, "EXP_EVENT_COUNTER"=124, "EXP_SW_TRIGGER"=125, "EXP_KINETICS_WINDOWSIZE"=126, "EXP_EXPOSURE"=127, "EXP_CONTROLLER_NAME"=128, "EXP_CCD_CHIP_NAME"=129, "EXP_BSWBINNING"=297, "EXP_EDGEENHANCE"=130, "EXP_BOXVIDEOGAIN"=131, "EXP_HSHADING_VALUE"=132, "EXP_VSHADING_VALUE"=133, "EXP_EDGEENHANCE_FLAG"=134, "EXP_SHADING_FLAG"=135, "EXP_GRAYSCALE"=136, "EXP_OFFSET"=137, "EXP_CCDGAIN"=138, "EXP_TEMPERATURE"=139, "EXP_MCPVOLTAGE"=140, "EXP_BOXEXPOSURE"=141, "EXP_ABC_FLAG"=142, "EXP_GAMMA_FLAG"=143, "EXP_AUTOBLACK_FLAG"=144, "EXP_AGC_FLAG"=145, "EXP_ODD_FIELD"=146, "EXP_FIELD_SELECT"=147, "EXP_RESET"=148, "EXP_EXTERN_ENABLE"=149, "EXP_CONTROLLERS_SUPPORTED"=150, "EXP_VTCLK"=151, "EXP_HTCLK"=152, "EXP_GATE_VS_CW"=153, "EXP_COM_PORT"=154, "EXP_US_UNITS"=156, "EXP_MS_UNITS"=157, "EXP_SEC_UNITS"=158, "EXP_MIN_UNITS"=159, "EXP_HRS_UNITS"=160, "EXP_FRAME_UNITS"=161, "EXP_SYNC_ASYNC"=162, "EXP_FOCUS_NFRAME"=163, "EXP_TIMEOUT"=164, "EXP_TIMEOUT_DEFAULT"=165, "EXP_HW_AUTOSTOP"=166, "EXP_RS170_INTEN_OFFSET"=167, "EXP_CONTROLLER_ALIVE"=168, "EXP_FOCUS_TYPE"=169, "EXP_FOCUS_ZOOM"=170, "EXP_FOCUS_PAN"=171, "EXP_MULTI_TAP_ROI"=172, "EXP_USE_INTERUPTS"=173, "EXP_DATA_ACQ_STATE"=174, "EXP_VERIFY_GOOD_VALUES"=175, "EXP_WHITE_CLAMP"=176, "EXP_BLACK_CLAMP"=177, "EXP_DELAY_TIME"=178, "EXP_READOUT_TIME"=179, "EXP_SW_DIAG"=180, "EXP_DIAG1"=181, "EXP_DIAG2"=182, "EXP_DIAG3"=183, "EXP_DIAG4"=184, "EXP_DIAG5"=185, "EXP_AorB_GROUP"=186, "EXP_ABSORBANCE_FLAG"=187, "EXP_ABSORBANCE_METHOD"=188, "EXP_ABSORBANCE_STRIPNUM"=189, "EXP_DMASIZE_VIA_DRIVER"=190, "EXP_DRIVERVERSION"=191, "EXP_NUM_DEVICES"=192, "EXP_ECPDMA_CHANNEL"=193, "EXP_CUSTOM_SHUTTER"=194, "EXP_ADC_OFFSET"=195, "EXP_CURRENT_READOUT_MODE"=196, "EXP_BANK_ADD"=197, "EXP_LUT_BANK"=198, "EXP_SETUP_STATUS"=201, "EXP_XY_GROUPING"=239, "EXP_MESSAGES_FLAG"=240, "EXP_TTL_LINE_TO_WAIT"=253, "EXP_DATA_COLLECTION_MODE"=258, "EXP_DATA_COLLECTION_TYPE"=262, "EXP_SKIPFRAMES"=274, "EXP_CLR_INT_CNTR"=276, "EXP_ENABLE_INT_CNTR"=277, "EXP_INT_CNTR"=278, "EXP_INTERNAL_SYNC_SRC"=279, "EXP_SW_EXTSYNC"=280, "EXP_PTG_PRESENT"=281, "EXP_ELEC_SHT"=282, "EXP_BOARDS_WITH_NVRAM"=283, "EXP_ANLGMASTER_ST143"=284, "EXP_ANLGSLAVE_ST143"=285, "EXP_DISPLAY_ST143"=286, "EXP_INTRFACE_ST143"=287, "EXP_SCANCONTROL_ST143"=288, "EXP_NUMBERFRAMES_IRQ"=204, "EXP_COOL_TYPE"=214, "EXP_HD_TYPE"=215, "EXP_INTENSIFER_GAIN"=216, "EXP_SHT_GATE_MODE"=217, "EXP_HD_CHECK"=218, "EXP_AMP_MODE"=219, "EXP_AMP_DIALOG"=247, "EXP_ANALOG_GAIN"=220, "EXP_HW_FIXES"=221, "EXP_PCI_CARDS"=222, "EXP_NOT_REVERSE"=223, "EXP_LOAD_NVRAM_DEFAULTS"=234, "EXP_CNTR_BRD"=235, "EXP_XDIMHW"=237, "EXP_YDIMHW"=238, "EXP_SPECIAL_FAST_RDOUT"=254, "EXP_SPCL_FAST_Y_DIM"=255, "EXP_SPCL_FAST_X_DIM"=256, "EXP_SPCL_FAST_Y_INDEX"=257, "EXP_SHUTTER_COMP_TIME_MS"=266, "EXP_NVRAM_AVAIL"=267, "EXP_NUMBER_AGAIN_AVAIL"=269, "EXP_SENSOR_TYPE"=270, "EXP_EVENT_TYPE"=292, "EXP_ANTI_BLOOMING"=293, "EXP_FAST_PULSE_ENABLE"=233, "EXP_USE_HEADCALIB"=296, "EXP_TEMP_STATUS"=301, "EXP_MULTIPLE_READMODES_LIVE"=302, "EXP_FIRST_ACQUIRE_FLAG"=303, "EXP_ANTI_BLOOMING_CONTROL"=304, "EXP_PRE_HORZ_DELAY"=305, "EXP_NVRAM_TRIES"=306, "EXP_XASCEND"=307, "EXP_YASCEND"=308, "EXP_ALT_TIMING"=309, "EXP_SHUTTER_PRE_COMP"=310, "EXP_PVCAM_POSSIBLE"=311, "EXP_ADC_IN_NVRAM"=312, "EXP_PASSTHRU_MODE"=313, "EXP_FIRMWAREVERSION"=314, "EXP_IMMEDIATE_SHUTTER"=315, "EXP_STAGE2_TEMP"=316, "EXP_AVGAIN_ENABLED"=317, "EXP_AVGAIN_SETPOINT"=318, "EXP_AVGAIN"=319, "EXP_AVGAIN_CALIB_TEMP"=320, "EXP_AVGAIN_CALIB_COEFF1"=321, "EXP_AVGAIN_CALIB_COEFF2"=322, "EXP_AVGAIN_CALIB_COEFF3"=323, "EXP_AVGAIN_CALIB_COEFF4"=324, "EXP_AVGAIN_CALIB_COEFF5"=325, "EXP_FORCE_READOUT_MODE"=326, "EXP_RESET_DATACOLLECTION"=327, "EXP_ACTIVE_SUBFRAME"=328, "EXP_PV_READOUT_PORT"=514, "EXP_CLASSNAME"=775, "EXP_FLATFLDNAME"=776, "EXP_DARKNAME"=777, "EXP_SETUPNAME"=778, "EXP_ACCESSNAME"=779, "EXP_DATFILENAME"=780, "EXP_ABSORBFILENAME"=781, "EXP_BLEMISHFILENAME"=782, "EXP_COSMICFILENAME"=783, "EXP_FILEINCBASENAME"=784, "EXP_YTNAME"=785, "EXP_DEVNAME"=786, "EXP_USEROI"=787, "EXP_DOBLEMISH"=788, "EXP_DOABSORB"=789, "EXP_DOCOSMIC"=790, "EXP_COSMICSENS"=791, "EXP_ABSORBSTRIP"=792, "EXP_DATATYPE"=793, "EXP_OVERWRITECONFIRM"=794, "EXP_FILEINCENABLE"=795, "EXP_FILEINCCOUNT"=796, "EXP_RUNNING"=797, "EXP_SAVEROPT"=798, "EXP_TIME_UNITS"=799, "EXP_FILEACCESS"=800, "EXP_AUTOSAVE"=801, "EXP_NEWWINDOW"=802, "EXP_XDIM"=803, "EXP_YDIM"=804, "EXP_XDIMDET"=805, "EXP_YDIMDET"=806, "EXP_ROIMODE"=807, "EXP_NUMREPEATSEXP"=808, "EXP_NUMACCUMSEXP"=809, "EXP_THREADSTATE"=810, "EXP_USEMINTHRESHOLDING"=811, "EXP_MINTHRESHOLDVALUE"=812, "EXP_USEMAXTHRESHOLDING"=813, "EXP_MAXTHRESHOLDVALUE"=814, "EXP_RUNNING_EXPERIMENT"=815, "EXP_THRESHOLD_DEMAND_UPDATE"=816, "EXP_ROICOUNT"=817, "EXP_ACCUMS"=818, "EXP_CACCUMS"=819, "EXP_CSEQUENTS"=820, "EXP_PHOTON_ESTIMATION_ENABLE"=821, "EXP_PHOTON_MAXTIME"=822, "EXP_PHOTON_MAXTIMEUNIT"=823, "EXP_CUSTOMFILTER_ENABLE"=824, "EXP_CUSTOMFILTER_SIZE"=825, "EXP_LOOKUPTABLE_ENABLE"=826, "EXP_BSHOWWINDOW"=827, "EXP_BBACKSUBTRACT"=828, "EXP_BDOFLATFIELD"=829, "EXP_ASCIIOUTPUTFILE"=830, "EXP_ASCIIOUTPUT_DELIMITER"=831, "EXP_ASCIIOUTPUT_TERMINATOR"=832, "EXP_FFTYPE"=833, "EXP_BGTYPE"=834, "EXP_COSGRASS"=835, "EXP_RUNASCONFIRM"=836, "EXP_RUNASRUNACCESS"=837, "EXP_DATAFILETYPE"=838, "EXP_ROTATE"=839, "EXP_FLIP"=840, "EXP_REVERSE"=841, "EXP_SWBINNING"=842, "EXP_AUTOSTORE"=843, "EXP_XBINNED"=844, "EXP_YBINNED"=845, "EXP_NUMPATTERNS"=846, "EXP_EXPERIMENTTIME"=847, "EXP_ASYNCSEQUENTIALS"=848, "EXP_SEQUENTIALS"=849, "EXP_CSEQUENTIALS"=850, "EXP_AUTOD"=851, "EXP_EXPOSURETIME"=852, "EXP_EXPOSURETIME_UNITS"=853, "EXP_ACQMODE"=854, "EXP_DMASIZE_PVCAM"=855, "EXP_INITIALIZE"=856, "EXP_CELL_X_SIZE"=857, "EXP_CELL_Y_SIZE"=858, "EXP_X_GAP_SIZE"=859, "EXP_Y_GAP_SIZE"=860] ("Param")
                    n215 = invoke class="IExpSetup2" method="SetParam"(reference=w293, "Param"=w295, "pSetVal"=1) -> ()  [unwired: 2 in, 5 out]
                  }
                }
              }
              frame #1 {
              }
              frame #2 {
                n216 = local write "busy"(FALSE ("busy")) -> ()
                n217 = local write "Stop measurement"(FALSE ("Stop measurement")) -> ()
                n218 = local write "Spectro Correct background"(TRUE ("Spectro Correct background")) -> ()
                n219 = property on="Spectro Correct background" class="Bool (strict)"("DisabledEnum"=T2."Enabled" ("Disabled")) -> ()  [unwired: 2 in, 2 out]
              }
            }
          }
          frame 12 {
            # "start continuous spectra"
            n220 = flat-sequence {
              frame #0 {
                n221 = Tick Count (ms)() -> (millisecond timer value=w300:u32)
                n222 = local write "time start (ms)"(w300) -> ()
              }
              frame #1 {
                w304 = 127 items=["EXP_ETACTUAL"=1, "EXP_SEQUENTS"=2, "EXP_ERROR"=3, "EXP_GETCAPS"=4, "EXP_GETPLSR"=5, "EXP_DETECTOR_BIT"=16, "EXP_RUNNING_APP"=23, "EXP_VIDEO_TYPE"=24, "EXP_CUSTOM_VIDEO_X"=25, "EXP_CUSTOM_VIDEO_Y"=26, "EXP_CUSTOM_VIDEO_FSTWIDTH"=27, "EXP_CUSTOM_VIDEO_LSTWIDTH"=28, "EXP_VIDEO_XDIM"=29, "EXP_VIDEO_YDIM"=30, "EXP_VIDEO_MAX_ZOOM"=31, "EXP_VIDEO_HORZ_PAN"=32, "EXP_VIDEO_VERT_PAN"=33, "EXP_WORD_MULTIPLIER"=34, "EXP_TARGET_ID"=35, "EXP_ADAPTER_ID"=36, "EXP_NUMADAPTORS"=37, "EXP_FORCE_PP_INIT"=38, "EXP_NOP_ADC"=39, "EXP_ACTUAL_TEMP"=40, "EXP_FORCE_AUTOSTOP"=41, "EXP_DEFAULT_VTCLK"=42, "EXP_MIN_VTCLK"=43, "EXP_MAX_VTCLK"=44, "EXP_DEFAULT_HTCLK"=45, "EXP_MIN_HTCLK"=46, "EXP_MAX_HTCLK"=47, "EXP_TIMING_STYLE"=48, "EXP_HEADSELECT"=49, "EXP_HORZPHASE"=50, "EXP_VERTPHASE"=51, "EXP_SPECIAL_SPEED"=52, "EXP_PRE_STRIPS"=53, "EXP_POST_STRIPS"=54, "EXP_PRE_LINES"=55, "EXP_POST_LINES"=56, "EXP_ACTIVE_LINES"=57, "EXP_ACTIVE_STRIPS"=58, "EXP_XFER_EXTRA"=59, "EXP_MIN_BLOCK"=60, "EXP_NUM_MIN_BLOCK"=61, "EXP_LOGIC_OUTPUT"=66, "EXP_VIDEO_BLANK"=67, "EXP_ZOOM_MODE_VIDEO"=68, "EXP_LEVEL_SYNC"=69, "EXP_DISABLE_LASER"=70, "EXP_ACQBACK_SHUTTER"=71, "EXP_ACQFLAT_SHUTTER"=72, "EXP_SMALL_CCD_MINEXP"=73, "EXP_LARGE_CCD_MINEXP"=74, "EXP_GATING_MODE"=75, "EXP_ILME_B1X"=76, "EXP_ILME_B2X"=77, "EXP_ILME_D1X"=78, "EXP_ILME_D2X"=79, "EXP_ILME_D4X"=80, "EXP_INIT_HW_ACCUM"=81, "EXP_5X_GAIN_ENABLE"=82, "EXP_RET_SRCCMP"=83, "EXP_EVENT_HANDLE"=84, "EXP_READOUT_MODE"=85, "EXP_SHUTTER_TYPE"=86, "EXP_USER_DEFINED_CHIP"=87, "EXP_USER_DEFINED_TIMING"=88, "EXP_CONTROLLER_VERSION"=89, "EXP_GET_CONTROLLER_VER"=90, "EXP_TTL_LINES"=91, "EXP_BIT_ADJUST"=92, "EXP_RESOLUTION"=93, "EXP_GAIN"=94, "EXP_ADC_RATE"=95, "EXP_ADC_TYPE"=96, "EXP_NUMBER_OF_CLEANS"=97, "EXP_NUM_OF_STRIPS_PER_CLN"=98, "EXP_INTERFACE_CARD"=99, "EXP_INTERRUPT"=100, "EXP_IO_ADDRESS1"=101, "EXP_IO_ADDRESS2"=102, "EXP_IO_ADDRESS3"=103, "EXP_HW_ROI"=104, "EXP_HW_BINNING"=105, "EXP_EDGE_TRIGGER"=106, "EXP_SHUTTER_CONTROL"=107, "EXP_RS170"=108, "EXP_RS170_COMPLEX"=109, "EXP_HW_RS170_LUT"=110, "EXP_RS170_INTENSITY_SCALING"=111, "EXP_RS170_OFFSET"=112, "EXP_RS170_PAN"=113, "EXP_RS170_ZOOM2X"=114, "EXP_RS170_ZOOM4X"=115, "EXP_RS170_BINNING"=116, "EXP_RS170_DECIMATION"=117, "EXP_HW_ACCUM"=118, "EXP_SHT_PREOPEN"=119, "EXP_STORE_STROBE"=120, "EXP_CONT_CLNS"=121, "EXP_TIMING_MODE"=122, "EXP_EXT_TRIGGER"=123, "EXP_EVENT_COUNTER"=124, "EXP_SW_TRIGGER"=125, "EXP_KINETICS_WINDOWSIZE"=126, "EXP_EXPOSURE"=127, "EXP_CONTROLLER_NAME"=128, "EXP_CCD_CHIP_NAME"=129, "EXP_BSWBINNING"=297, "EXP_EDGEENHANCE"=130, "EXP_BOXVIDEOGAIN"=131, "EXP_HSHADING_VALUE"=132, "EXP_VSHADING_VALUE"=133, "EXP_EDGEENHANCE_FLAG"=134, "EXP_SHADING_FLAG"=135, "EXP_GRAYSCALE"=136, "EXP_OFFSET"=137, "EXP_CCDGAIN"=138, "EXP_TEMPERATURE"=139, "EXP_MCPVOLTAGE"=140, "EXP_BOXEXPOSURE"=141, "EXP_ABC_FLAG"=142, "EXP_GAMMA_FLAG"=143, "EXP_AUTOBLACK_FLAG"=144, "EXP_AGC_FLAG"=145, "EXP_ODD_FIELD"=146, "EXP_FIELD_SELECT"=147, "EXP_RESET"=148, "EXP_EXTERN_ENABLE"=149, "EXP_CONTROLLERS_SUPPORTED"=150, "EXP_VTCLK"=151, "EXP_HTCLK"=152, "EXP_GATE_VS_CW"=153, "EXP_COM_PORT"=154, "EXP_US_UNITS"=156, "EXP_MS_UNITS"=157, "EXP_SEC_UNITS"=158, "EXP_MIN_UNITS"=159, "EXP_HRS_UNITS"=160, "EXP_FRAME_UNITS"=161, "EXP_SYNC_ASYNC"=162, "EXP_FOCUS_NFRAME"=163, "EXP_TIMEOUT"=164, "EXP_TIMEOUT_DEFAULT"=165, "EXP_HW_AUTOSTOP"=166, "EXP_RS170_INTEN_OFFSET"=167, "EXP_CONTROLLER_ALIVE"=168, "EXP_FOCUS_TYPE"=169, "EXP_FOCUS_ZOOM"=170, "EXP_FOCUS_PAN"=171, "EXP_MULTI_TAP_ROI"=172, "EXP_USE_INTERUPTS"=173, "EXP_DATA_ACQ_STATE"=174, "EXP_VERIFY_GOOD_VALUES"=175, "EXP_WHITE_CLAMP"=176, "EXP_BLACK_CLAMP"=177, "EXP_DELAY_TIME"=178, "EXP_READOUT_TIME"=179, "EXP_SW_DIAG"=180, "EXP_DIAG1"=181, "EXP_DIAG2"=182, "EXP_DIAG3"=183, "EXP_DIAG4"=184, "EXP_DIAG5"=185, "EXP_AorB_GROUP"=186, "EXP_ABSORBANCE_FLAG"=187, "EXP_ABSORBANCE_METHOD"=188, "EXP_ABSORBANCE_STRIPNUM"=189, "EXP_DMASIZE_VIA_DRIVER"=190, "EXP_DRIVERVERSION"=191, "EXP_NUM_DEVICES"=192, "EXP_ECPDMA_CHANNEL"=193, "EXP_CUSTOM_SHUTTER"=194, "EXP_ADC_OFFSET"=195, "EXP_CURRENT_READOUT_MODE"=196, "EXP_BANK_ADD"=197, "EXP_LUT_BANK"=198, "EXP_SETUP_STATUS"=201, "EXP_XY_GROUPING"=239, "EXP_MESSAGES_FLAG"=240, "EXP_TTL_LINE_TO_WAIT"=253, "EXP_DATA_COLLECTION_MODE"=258, "EXP_DATA_COLLECTION_TYPE"=262, "EXP_SKIPFRAMES"=274, "EXP_CLR_INT_CNTR"=276, "EXP_ENABLE_INT_CNTR"=277, "EXP_INT_CNTR"=278, "EXP_INTERNAL_SYNC_SRC"=279, "EXP_SW_EXTSYNC"=280, "EXP_PTG_PRESENT"=281, "EXP_ELEC_SHT"=282, "EXP_BOARDS_WITH_NVRAM"=283, "EXP_ANLGMASTER_ST143"=284, "EXP_ANLGSLAVE_ST143"=285, "EXP_DISPLAY_ST143"=286, "EXP_INTRFACE_ST143"=287, "EXP_SCANCONTROL_ST143"=288, "EXP_NUMBERFRAMES_IRQ"=204, "EXP_COOL_TYPE"=214, "EXP_HD_TYPE"=215, "EXP_INTENSIFER_GAIN"=216, "EXP_SHT_GATE_MODE"=217, "EXP_HD_CHECK"=218, "EXP_AMP_MODE"=219, "EXP_AMP_DIALOG"=247, "EXP_ANALOG_GAIN"=220, "EXP_HW_FIXES"=221, "EXP_PCI_CARDS"=222, "EXP_NOT_REVERSE"=223, "EXP_LOAD_NVRAM_DEFAULTS"=234, "EXP_CNTR_BRD"=235, "EXP_XDIMHW"=237, "EXP_YDIMHW"=238, "EXP_SPECIAL_FAST_RDOUT"=254, "EXP_SPCL_FAST_Y_DIM"=255, "EXP_SPCL_FAST_X_DIM"=256, "EXP_SPCL_FAST_Y_INDEX"=257, "EXP_SHUTTER_COMP_TIME_MS"=266, "EXP_NVRAM_AVAIL"=267, "EXP_NUMBER_AGAIN_AVAIL"=269, "EXP_SENSOR_TYPE"=270, "EXP_EVENT_TYPE"=292, "EXP_ANTI_BLOOMING"=293, "EXP_FAST_PULSE_ENABLE"=233, "EXP_USE_HEADCALIB"=296, "EXP_TEMP_STATUS"=301, "EXP_MULTIPLE_READMODES_LIVE"=302, "EXP_FIRST_ACQUIRE_FLAG"=303, "EXP_ANTI_BLOOMING_CONTROL"=304, "EXP_PRE_HORZ_DELAY"=305, "EXP_NVRAM_TRIES"=306, "EXP_XASCEND"=307, "EXP_YASCEND"=308, "EXP_ALT_TIMING"=309, "EXP_SHUTTER_PRE_COMP"=310, "EXP_PVCAM_POSSIBLE"=311, "EXP_ADC_IN_NVRAM"=312, "EXP_PASSTHRU_MODE"=313, "EXP_FIRMWAREVERSION"=314, "EXP_IMMEDIATE_SHUTTER"=315, "EXP_STAGE2_TEMP"=316, "EXP_AVGAIN_ENABLED"=317, "EXP_AVGAIN_SETPOINT"=318, "EXP_AVGAIN"=319, "EXP_AVGAIN_CALIB_TEMP"=320, "EXP_AVGAIN_CALIB_COEFF1"=321, "EXP_AVGAIN_CALIB_COEFF2"=322, "EXP_AVGAIN_CALIB_COEFF3"=323, "EXP_AVGAIN_CALIB_COEFF4"=324, "EXP_AVGAIN_CALIB_COEFF5"=325, "EXP_FORCE_READOUT_MODE"=326, "EXP_RESET_DATACOLLECTION"=327, "EXP_ACTIVE_SUBFRAME"=328, "EXP_PV_READOUT_PORT"=514, "EXP_CLASSNAME"=775, "EXP_FLATFLDNAME"=776, "EXP_DARKNAME"=777, "EXP_SETUPNAME"=778, "EXP_ACCESSNAME"=779, "EXP_DATFILENAME"=780, "EXP_ABSORBFILENAME"=781, "EXP_BLEMISHFILENAME"=782, "EXP_COSMICFILENAME"=783, "EXP_FILEINCBASENAME"=784, "EXP_YTNAME"=785, "EXP_DEVNAME"=786, "EXP_USEROI"=787, "EXP_DOBLEMISH"=788, "EXP_DOABSORB"=789, "EXP_DOCOSMIC"=790, "EXP_COSMICSENS"=791, "EXP_ABSORBSTRIP"=792, "EXP_DATATYPE"=793, "EXP_OVERWRITECONFIRM"=794, "EXP_FILEINCENABLE"=795, "EXP_FILEINCCOUNT"=796, "EXP_RUNNING"=797, "EXP_SAVEROPT"=798, "EXP_TIME_UNITS"=799, "EXP_FILEACCESS"=800, "EXP_AUTOSAVE"=801, "EXP_NEWWINDOW"=802, "EXP_XDIM"=803, "EXP_YDIM"=804, "EXP_XDIMDET"=805, "EXP_YDIMDET"=806, "EXP_ROIMODE"=807, "EXP_NUMREPEATSEXP"=808, "EXP_NUMACCUMSEXP"=809, "EXP_THREADSTATE"=810, "EXP_USEMINTHRESHOLDING"=811, "EXP_MINTHRESHOLDVALUE"=812, "EXP_USEMAXTHRESHOLDING"=813, "EXP_MAXTHRESHOLDVALUE"=814, "EXP_RUNNING_EXPERIMENT"=815, "EXP_THRESHOLD_DEMAND_UPDATE"=816, "EXP_ROICOUNT"=817, "EXP_ACCUMS"=818, "EXP_CACCUMS"=819, "EXP_CSEQUENTS"=820, "EXP_PHOTON_ESTIMATION_ENABLE"=821, "EXP_PHOTON_MAXTIME"=822, "EXP_PHOTON_MAXTIMEUNIT"=823, "EXP_CUSTOMFILTER_ENABLE"=824, "EXP_CUSTOMFILTER_SIZE"=825, "EXP_LOOKUPTABLE_ENABLE"=826, "EXP_BSHOWWINDOW"=827, "EXP_BBACKSUBTRACT"=828, "EXP_BDOFLATFIELD"=829, "EXP_ASCIIOUTPUTFILE"=830, "EXP_ASCIIOUTPUT_DELIMITER"=831, "EXP_ASCIIOUTPUT_TERMINATOR"=832, "EXP_FFTYPE"=833, "EXP_BGTYPE"=834, "EXP_COSGRASS"=835, "EXP_RUNASCONFIRM"=836, "EXP_RUNASRUNACCESS"=837, "EXP_DATAFILETYPE"=838, "EXP_ROTATE"=839, "EXP_FLIP"=840, "EXP_REVERSE"=841, "EXP_SWBINNING"=842, "EXP_AUTOSTORE"=843, "EXP_XBINNED"=844, "EXP_YBINNED"=845, "EXP_NUMPATTERNS"=846, "EXP_EXPERIMENTTIME"=847, "EXP_ASYNCSEQUENTIALS"=848, "EXP_SEQUENTIALS"=849, "EXP_CSEQUENTIALS"=850, "EXP_AUTOD"=851, "EXP_EXPOSURETIME"=852, "EXP_EXPOSURETIME_UNITS"=853, "EXP_ACQMODE"=854, "EXP_DMASIZE_PVCAM"=855, "EXP_INITIALIZE"=856, "EXP_CELL_X_SIZE"=857, "EXP_CELL_Y_SIZE"=858, "EXP_X_GAP_SIZE"=859, "EXP_Y_GAP_SIZE"=860] ("Param")
                n223 = local read "OMA V exposure time"() -> (w305:dbl)
                n224 = local read "experiment reference"() -> (w303:refnum<k7>)
                n225 = invoke class="IExpSetup2" method="SetParam"(reference=w303, "Param"=w304, "pSetVal"=w305) -> (reference out=w302:refnum<k7>)  [unwired: 2 in, 4 out]
                n226 = local read "file reference"() -> (w301:refnum<k7>)
                n227 = while {
                  shift-right: [w314] -> _
                  shift-left: w301 -> [w311]
                  tunnel: w302 -> [w309]
                  i -> [w317]
                  stop <- w312 stop-if-true
                  n228 = flat-sequence {
                    tunnel: [w322] -> w313
                    tunnel: w311 -> [w321]
                    tunnel: [w320] -> w310
                    tunnel: w309 -> [w319]
                    tunnel: [w318] -> w306
                    tunnel: w313 -> [w328]
                    tunnel: [w327] -> w307
                    tunnel: w306 -> [w327]
                    tunnel: [w331] -> w312
                    tunnel: [w330] -> w308
                    tunnel: w307 -> [w329]
                    frame #0 {
                      n229 = invoke class="IExpSetup2" method="Start"(reference=w319, "pFile"=w321) -> (reference out=w318:refnum<k7>, "pFile"=w320:refnum<k7>)  [unwired: 2 in, 2 out]
                      n230 = local read "time start (ms)"() -> (w324:i32)
                      n231 = Tick Count (ms)() -> (millisecond timer value=w322:u32)
                      n232 = Subtract(x=w322, y=w324) -> (x-y=w325:u32)
                      n233 = Divide(x=w325, y=u32 1000) -> (x/y=w326:dbl)
                      n234 = local write "time elapsed (s)"(w326) -> ()
                    }
                    frame #1 {
                      n235 = local write "time start (ms)"(w328) -> ()
                    }
                    frame #2 {
                      n236 = while {
                        tunnel: [w339] -> w331
                        tunnel: [w332] -> _
                        tunnel: [w333] -> w330
                        tunnel: w329 -> [w332]
                        stop <- w338 stop-if-true
                        w337 = 797 items=["EXP_ETACTUAL"=1, "EXP_SEQUENTS"=2, "EXP_ERROR"=3, "EXP_GETCAPS"=4, "EXP_GETPLSR"=5, "EXP_DETECTOR_BIT"=16, "EXP_RUNNING_APP"=23, "EXP_VIDEO_TYPE"=24, "EXP_CUSTOM_VIDEO_X"=25, "EXP_CUSTOM_VIDEO_Y"=26, "EXP_CUSTOM_VIDEO_FSTWIDTH"=27, "EXP_CUSTOM_VIDEO_LSTWIDTH"=28, "EXP_VIDEO_XDIM"=29, "EXP_VIDEO_YDIM"=30, "EXP_VIDEO_MAX_ZOOM"=31, "EXP_VIDEO_HORZ_PAN"=32, "EXP_VIDEO_VERT_PAN"=33, "EXP_WORD_MULTIPLIER"=34, "EXP_TARGET_ID"=35, "EXP_ADAPTER_ID"=36, "EXP_NUMADAPTORS"=37, "EXP_FORCE_PP_INIT"=38, "EXP_NOP_ADC"=39, "EXP_ACTUAL_TEMP"=40, "EXP_FORCE_AUTOSTOP"=41, "EXP_DEFAULT_VTCLK"=42, "EXP_MIN_VTCLK"=43, "EXP_MAX_VTCLK"=44, "EXP_DEFAULT_HTCLK"=45, "EXP_MIN_HTCLK"=46, "EXP_MAX_HTCLK"=47, "EXP_TIMING_STYLE"=48, "EXP_HEADSELECT"=49, "EXP_HORZPHASE"=50, "EXP_VERTPHASE"=51, "EXP_SPECIAL_SPEED"=52, "EXP_PRE_STRIPS"=53, "EXP_POST_STRIPS"=54, "EXP_PRE_LINES"=55, "EXP_POST_LINES"=56, "EXP_ACTIVE_LINES"=57, "EXP_ACTIVE_STRIPS"=58, "EXP_XFER_EXTRA"=59, "EXP_MIN_BLOCK"=60, "EXP_NUM_MIN_BLOCK"=61, "EXP_LOGIC_OUTPUT"=66, "EXP_VIDEO_BLANK"=67, "EXP_ZOOM_MODE_VIDEO"=68, "EXP_LEVEL_SYNC"=69, "EXP_DISABLE_LASER"=70, "EXP_ACQBACK_SHUTTER"=71, "EXP_ACQFLAT_SHUTTER"=72, "EXP_SMALL_CCD_MINEXP"=73, "EXP_LARGE_CCD_MINEXP"=74, "EXP_GATING_MODE"=75, "EXP_ILME_B1X"=76, "EXP_ILME_B2X"=77, "EXP_ILME_D1X"=78, "EXP_ILME_D2X"=79, "EXP_ILME_D4X"=80, "EXP_INIT_HW_ACCUM"=81, "EXP_5X_GAIN_ENABLE"=82, "EXP_RET_SRCCMP"=83, "EXP_EVENT_HANDLE"=84, "EXP_READOUT_MODE"=85, "EXP_SHUTTER_TYPE"=86, "EXP_USER_DEFINED_CHIP"=87, "EXP_USER_DEFINED_TIMING"=88, "EXP_CONTROLLER_VERSION"=89, "EXP_GET_CONTROLLER_VER"=90, "EXP_TTL_LINES"=91, "EXP_BIT_ADJUST"=92, "EXP_RESOLUTION"=93, "EXP_GAIN"=94, "EXP_ADC_RATE"=95, "EXP_ADC_TYPE"=96, "EXP_NUMBER_OF_CLEANS"=97, "EXP_NUM_OF_STRIPS_PER_CLN"=98, "EXP_INTERFACE_CARD"=99, "EXP_INTERRUPT"=100, "EXP_IO_ADDRESS1"=101, "EXP_IO_ADDRESS2"=102, "EXP_IO_ADDRESS3"=103, "EXP_HW_ROI"=104, "EXP_HW_BINNING"=105, "EXP_EDGE_TRIGGER"=106, "EXP_SHUTTER_CONTROL"=107, "EXP_RS170"=108, "EXP_RS170_COMPLEX"=109, "EXP_HW_RS170_LUT"=110, "EXP_RS170_INTENSITY_SCALING"=111, "EXP_RS170_OFFSET"=112, "EXP_RS170_PAN"=113, "EXP_RS170_ZOOM2X"=114, "EXP_RS170_ZOOM4X"=115, "EXP_RS170_BINNING"=116, "EXP_RS170_DECIMATION"=117, "EXP_HW_ACCUM"=118, "EXP_SHT_PREOPEN"=119, "EXP_STORE_STROBE"=120, "EXP_CONT_CLNS"=121, "EXP_TIMING_MODE"=122, "EXP_EXT_TRIGGER"=123, "EXP_EVENT_COUNTER"=124, "EXP_SW_TRIGGER"=125, "EXP_KINETICS_WINDOWSIZE"=126, "EXP_EXPOSURE"=127, "EXP_CONTROLLER_NAME"=128, "EXP_CCD_CHIP_NAME"=129, "EXP_BSWBINNING"=297, "EXP_EDGEENHANCE"=130, "EXP_BOXVIDEOGAIN"=131, "EXP_HSHADING_VALUE"=132, "EXP_VSHADING_VALUE"=133, "EXP_EDGEENHANCE_FLAG"=134, "EXP_SHADING_FLAG"=135, "EXP_GRAYSCALE"=136, "EXP_OFFSET"=137, "EXP_CCDGAIN"=138, "EXP_TEMPERATURE"=139, "EXP_MCPVOLTAGE"=140, "EXP_BOXEXPOSURE"=141, "EXP_ABC_FLAG"=142, "EXP_GAMMA_FLAG"=143, "EXP_AUTOBLACK_FLAG"=144, "EXP_AGC_FLAG"=145, "EXP_ODD_FIELD"=146, "EXP_FIELD_SELECT"=147, "EXP_RESET"=148, "EXP_EXTERN_ENABLE"=149, "EXP_CONTROLLERS_SUPPORTED"=150, "EXP_VTCLK"=151, "EXP_HTCLK"=152, "EXP_GATE_VS_CW"=153, "EXP_COM_PORT"=154, "EXP_US_UNITS"=156, "EXP_MS_UNITS"=157, "EXP_SEC_UNITS"=158, "EXP_MIN_UNITS"=159, "EXP_HRS_UNITS"=160, "EXP_FRAME_UNITS"=161, "EXP_SYNC_ASYNC"=162, "EXP_FOCUS_NFRAME"=163, "EXP_TIMEOUT"=164, "EXP_TIMEOUT_DEFAULT"=165, "EXP_HW_AUTOSTOP"=166, "EXP_RS170_INTEN_OFFSET"=167, "EXP_CONTROLLER_ALIVE"=168, "EXP_FOCUS_TYPE"=169, "EXP_FOCUS_ZOOM"=170, "EXP_FOCUS_PAN"=171, "EXP_MULTI_TAP_ROI"=172, "EXP_USE_INTERUPTS"=173, "EXP_DATA_ACQ_STATE"=174, "EXP_VERIFY_GOOD_VALUES"=175, "EXP_WHITE_CLAMP"=176, "EXP_BLACK_CLAMP"=177, "EXP_DELAY_TIME"=178, "EXP_READOUT_TIME"=179, "EXP_SW_DIAG"=180, "EXP_DIAG1"=181, "EXP_DIAG2"=182, "EXP_DIAG3"=183, "EXP_DIAG4"=184, "EXP_DIAG5"=185, "EXP_AorB_GROUP"=186, "EXP_ABSORBANCE_FLAG"=187, "EXP_ABSORBANCE_METHOD"=188, "EXP_ABSORBANCE_STRIPNUM"=189, "EXP_DMASIZE_VIA_DRIVER"=190, "EXP_DRIVERVERSION"=191, "EXP_NUM_DEVICES"=192, "EXP_ECPDMA_CHANNEL"=193, "EXP_CUSTOM_SHUTTER"=194, "EXP_ADC_OFFSET"=195, "EXP_CURRENT_READOUT_MODE"=196, "EXP_BANK_ADD"=197, "EXP_LUT_BANK"=198, "EXP_SETUP_STATUS"=201, "EXP_XY_GROUPING"=239, "EXP_MESSAGES_FLAG"=240, "EXP_TTL_LINE_TO_WAIT"=253, "EXP_DATA_COLLECTION_MODE"=258, "EXP_DATA_COLLECTION_TYPE"=262, "EXP_SKIPFRAMES"=274, "EXP_CLR_INT_CNTR"=276, "EXP_ENABLE_INT_CNTR"=277, "EXP_INT_CNTR"=278, "EXP_INTERNAL_SYNC_SRC"=279, "EXP_SW_EXTSYNC"=280, "EXP_PTG_PRESENT"=281, "EXP_ELEC_SHT"=282, "EXP_BOARDS_WITH_NVRAM"=283, "EXP_ANLGMASTER_ST143"=284, "EXP_ANLGSLAVE_ST143"=285, "EXP_DISPLAY_ST143"=286, "EXP_INTRFACE_ST143"=287, "EXP_SCANCONTROL_ST143"=288, "EXP_NUMBERFRAMES_IRQ"=204, "EXP_COOL_TYPE"=214, "EXP_HD_TYPE"=215, "EXP_INTENSIFER_GAIN"=216, "EXP_SHT_GATE_MODE"=217, "EXP_HD_CHECK"=218, "EXP_AMP_MODE"=219, "EXP_AMP_DIALOG"=247, "EXP_ANALOG_GAIN"=220, "EXP_HW_FIXES"=221, "EXP_PCI_CARDS"=222, "EXP_NOT_REVERSE"=223, "EXP_LOAD_NVRAM_DEFAULTS"=234, "EXP_CNTR_BRD"=235, "EXP_XDIMHW"=237, "EXP_YDIMHW"=238, "EXP_SPECIAL_FAST_RDOUT"=254, "EXP_SPCL_FAST_Y_DIM"=255, "EXP_SPCL_FAST_X_DIM"=256, "EXP_SPCL_FAST_Y_INDEX"=257, "EXP_SHUTTER_COMP_TIME_MS"=266, "EXP_NVRAM_AVAIL"=267, "EXP_NUMBER_AGAIN_AVAIL"=269, "EXP_SENSOR_TYPE"=270, "EXP_EVENT_TYPE"=292, "EXP_ANTI_BLOOMING"=293, "EXP_FAST_PULSE_ENABLE"=233, "EXP_USE_HEADCALIB"=296, "EXP_TEMP_STATUS"=301, "EXP_MULTIPLE_READMODES_LIVE"=302, "EXP_FIRST_ACQUIRE_FLAG"=303, "EXP_ANTI_BLOOMING_CONTROL"=304, "EXP_PRE_HORZ_DELAY"=305, "EXP_NVRAM_TRIES"=306, "EXP_XASCEND"=307, "EXP_YASCEND"=308, "EXP_ALT_TIMING"=309, "EXP_SHUTTER_PRE_COMP"=310, "EXP_PVCAM_POSSIBLE"=311, "EXP_ADC_IN_NVRAM"=312, "EXP_PASSTHRU_MODE"=313, "EXP_FIRMWAREVERSION"=314, "EXP_IMMEDIATE_SHUTTER"=315, "EXP_STAGE2_TEMP"=316, "EXP_AVGAIN_ENABLED"=317, "EXP_AVGAIN_SETPOINT"=318, "EXP_AVGAIN"=319, "EXP_AVGAIN_CALIB_TEMP"=320, "EXP_AVGAIN_CALIB_COEFF1"=321, "EXP_AVGAIN_CALIB_COEFF2"=322, "EXP_AVGAIN_CALIB_COEFF3"=323, "EXP_AVGAIN_CALIB_COEFF4"=324, "EXP_AVGAIN_CALIB_COEFF5"=325, "EXP_FORCE_READOUT_MODE"=326, "EXP_RESET_DATACOLLECTION"=327, "EXP_ACTIVE_SUBFRAME"=328, "EXP_PV_READOUT_PORT"=514, "EXP_COOLING_FAN_CTRL"=339, "EXP_SHTR_RES"=343, "EXP_PBC"=351, "EXP_PREEXP_CLEANS"=354, "EXP_TTL_CTRL"=355, "EXP_PAR_SHIFT_INDEX"=547, "EXP_LOGIC_OUTPUT_INVERT"=548, "EXP_CLASSNAME"=775, "EXP_FLATFLDNAME"=776, "EXP_DARKNAME"=777, "EXP_SETUPNAME"=778, "EXP_ACCESSNAME"=779, "EXP_DATFILENAME"=780, "EXP_ABSORBFILENAME"=781, "EXP_BLEMISHFILENAME"=782, "EXP_COSMICFILENAME"=783, "EXP_FILEINCBASENAME"=784, "EXP_YTNAME"=785, "EXP_DEVNAME"=786, "EXP_USEROI"=787, "EXP_DOBLEMISH"=788, "EXP_DOABSORB"=789, "EXP_DOCOSMIC"=790, "EXP_COSMICSENS"=791, "EXP_ABSORBSTRIP"=792, "EXP_DATATYPE"=793, "EXP_OVERWRITECONFIRM"=794, "EXP_FILEINCENABLE"=795, "EXP_FILEINCCOUNT"=796, "EXP_RUNNING"=797, "EXP_SAVEROPT"=798, "EXP_TIME_UNITS"=799, "EXP_FILEACCESS"=800, "EXP_AUTOSAVE"=801, "EXP_NEWWINDOW"=802, "EXP_XDIM"=803, "EXP_YDIM"=804, "EXP_XDIMDET"=805, "EXP_YDIMDET"=806, "EXP_ROIMODE"=807, "EXP_NUMREPEATSEXP"=808, "EXP_NUMACCUMSEXP"=809, "EXP_THREADSTATE"=810, "EXP_USEMINTHRESHOLDING"=811, "EXP_MINTHRESHOLDVALUE"=812, "EXP_USEMAXTHRESHOLDING"=813, "EXP_MAXTHRESHOLDVALUE"=814, "EXP_RUNNING_EXPERIMENT"=815, "EXP_THRESHOLD_DEMAND_UPDATE"=816, "EXP_ROICOUNT"=817, "EXP_ACCUMS"=818, "EXP_CACCUMS"=819, "EXP_CSEQUENTS"=820, "EXP_PHOTON_ESTIMATION_ENABLE"=821, "EXP_PHOTON_MAXTIME"=822, "EXP_PHOTON_MAXTIMEUNIT"=823, "EXP_CUSTOMFILTER_ENABLE"=824, "EXP_CUSTOMFILTER_SIZE"=825, "EXP_LOOKUPTABLE_ENABLE"=826, "EXP_BSHOWWINDOW"=827, "EXP_BBACKSUBTRACT"=828, "EXP_BDOFLATFIELD"=829, "EXP_ASCIIOUTPUTFILE"=830, "EXP_ASCIIOUTPUT_DELIMITER"=831, "EXP_ASCIIOUTPUT_TERMINATOR"=832, "EXP_FFTYPE"=833, "EXP_BGTYPE"=834, "EXP_COSGRASS"=835, "EXP_RUNASCONFIRM"=836, "EXP_RUNASRUNACCESS"=837, "EXP_DATAFILETYPE"=838, "EXP_ROTATE"=839, "EXP_FLIP"=840, "EXP_REVERSE"=841, "EXP_SWBINNING"=842, "EXP_AUTOSTORE"=843, "EXP_XBINNED"=844, "EXP_YBINNED"=845, "EXP_NUMPATTERNS"=846, "EXP_EXPERIMENTTIME"=847, "EXP_ASYNCSEQUENTIALS"=848, "EXP_SEQUENTIALS"=849, "EXP_CSEQUENTIALS"=850, "EXP_AUTOD"=851, "EXP_EXPOSURETIME"=852, "EXP_EXPOSURETIME_UNITS"=853, "EXP_ACQMODE"=854, "EXP_DMASIZE_PVCAM"=855, "EXP_INITIALIZE"=856, "EXP_CELL_X_SIZE"=857, "EXP_CELL_Y_SIZE"=858, "EXP_X_GAP_SIZE"=859, "EXP_Y_GAP_SIZE"=860] ("Param")
                        n237 = invoke class="IExpSetup2" method="GetParam"(reference=w332, "Param"=w337) -> (reference out=w333:refnum<k7>, "GetParam"=w340:variant)  [unwired: 3 in, 3 out]
                        n238 = Variant To Data(type=TRUE, Variant=w340) -> (data=w335:bool)  [unwired: 1 in, 1 out]
                        n239 = local read "Stop measurement"() -> (w339:bool)
                        n240 = Not(x=w335) -> (.not. x?=w334:bool)
                        n241 = Or(x=w339, y=w334) -> (x .or. y?=w338:bool)
                      }
                    }
                    frame #3 {
                    }
                  }
                  n242 = Not(x=w312) -> (.not. x?=w315:bool)
                  n243 = Equal To 0?(x=w317) -> (x = 0?=w316:bool)
                  n244 = case shown="False" w315 {
                    tunnel: [w342 w343] -> w314
                    tunnel: w316 -> [_ w353]
                    tunnel: w310 -> [w342 w348]
                    tunnel: w308 -> [w341 _]
                    frame False {
                      n245 = invoke class="IExpSetup2" method="Stop"(reference=w341) -> ()  [unwired: 2 in, 3 out]
                    }
                    frame True {
                      n246 = local read "FrameVariant"() -> (w351:variant)
                      n247 = local read "frame array"() -> (w352:i32[][])
                      n248 = invoke class="IDocFile" method="GetFrame"(reference=w348, "frame"=i16 1, "FrameVariant"=w351) -> (reference out=w343:refnum<k7>, "FrameVariant"=w349:variant)  [unwired: 2 in, 3 out]
                      n249 = Variant To Data(type=w352, Variant=w349) -> (data=w356:i32[][])  [unwired: 1 in, 1 out]
                      n250 = Index Array(array=w356, index (col)=0 ("disabled index (col)")) -> (element=w354:i32[])  [unwired: 1 in]
                      n251 = case shown="True" w353 {
                        tunnel: w343 -> [_ w362]
                        tunnel: w354 -> [w357 w358]
                        tunnel: [w357 w358] -> w345
                        frame False {
                        }
                        frame True {
                          n252 = invoke class="IDocFile" method="GetCalibration"(reference=w362) -> ("GetCalibration"=w364:refnum<k7>)  [unwired: 2 in, 2 out]
                          n253 = Array Size(array=w358) -> (size(s)=w359:i32)
                          n254 = property class="ICalibObj"(reference=w364) -> (reference out=w360:refnum<k7>, "PairCount"=w365:u8)  [unwired: 1 in, 1 out]
                          n255 = for {
                            N: w365 -> [_]
                            tunnel: w360 -> [w382]
                            tunnel: [w383] -> w367 mode=indexing
                            tunnel: [w380] -> w366 mode=indexing
                            i -> [w381]
                            n256 = invoke class="ICalibObj" method="CalibVal"(reference=w382, "index"=w381) -> ("CalibVal"=w383:dbl)  [unwired: 2 in, 3 out]
                            n257 = invoke class="ICalibObj" method="PixelLoc"(reference=w382, "index"=w381) -> ("PixelLoc"=w380:dbl)  [unwired: 2 in, 3 out]
                          }
                          n258 = for {
                            N: w359 -> [_]
                            tunnel: w367 -> [w379]
                            tunnel: [w378] -> w361 mode=indexing
                            tunnel: [w377] -> _ mode=indexing
                            tunnel: w366 -> [w376]
                            tunnel: 1 ("index") -> [w368]
                            i -> [w375]
                            n259 = Divide(x=w368, y=2) -> (x/y=w372:dbl)
                            n260 = Round To Nearest(number=w372) -> (nearest integer value=w370:dbl)
                            n261 = Multiply(x=w375, y=w368) -> (x*y=w371:i32)
                            n262 = Increment(x=w370) -> (x+1=w369:dbl)
                            n263 = Add(x=w371, y=w369) -> (x+y=w374:dbl)
                            n264 = call <vilib>:"Polynomial Interpolation.vi"("x value"=w374, "X"=w376, "Y"=w379) -> ("interpolation error"=w377:dbl, "interpolation value"=w378:dbl)  [unwired: 1 out]
                          }
                          n265 = local write "Wavelength Scale"(w361) -> ()
                        }
                      }
                      n266 = local read "Wavelength Scale"() -> (w344:dbl[])
                      n267 = Add Array Elements(numeric array=w345) -> (sum=w347:i32)
                      n268 = Bundle("Wavelength Scale"=w344, "frame array"=w345) -> (w346:T3)  [unwired: 1 in]
                      n269 = local write "Time Trace"(w347) -> ()
                      n270 = local write "Intensity Sum"(w347) -> ()
                      n271 = local write "XY Graph Spectrum"(w346) -> ()
                    }
                  }
                }
              }
              frame #2 {
                w384 = FALSE ("Stop measurement")
                n272 = local write "busy"(FALSE ("busy")) -> ()
                n273 = local write "Stop measurement"(w384) -> ()
                n274 = local write "Start Continuous"(w384) -> ()
              }
            }
          }
          frame 13 {
            w388 = 127 items=["EXP_ETACTUAL"=1, "EXP_SEQUENTS"=2, "EXP_ERROR"=3, "EXP_GETCAPS"=4, "EXP_GETPLSR"=5, "EXP_DETECTOR_BIT"=16, "EXP_RUNNING_APP"=23, "EXP_VIDEO_TYPE"=24, "EXP_CUSTOM_VIDEO_X"=25, "EXP_CUSTOM_VIDEO_Y"=26, "EXP_CUSTOM_VIDEO_FSTWIDTH"=27, "EXP_CUSTOM_VIDEO_LSTWIDTH"=28, "EXP_VIDEO_XDIM"=29, "EXP_VIDEO_YDIM"=30, "EXP_VIDEO_MAX_ZOOM"=31, "EXP_VIDEO_HORZ_PAN"=32, "EXP_VIDEO_VERT_PAN"=33, "EXP_WORD_MULTIPLIER"=34, "EXP_TARGET_ID"=35, "EXP_ADAPTER_ID"=36, "EXP_NUMADAPTORS"=37, "EXP_FORCE_PP_INIT"=38, "EXP_NOP_ADC"=39, "EXP_ACTUAL_TEMP"=40, "EXP_FORCE_AUTOSTOP"=41, "EXP_DEFAULT_VTCLK"=42, "EXP_MIN_VTCLK"=43, "EXP_MAX_VTCLK"=44, "EXP_DEFAULT_HTCLK"=45, "EXP_MIN_HTCLK"=46, "EXP_MAX_HTCLK"=47, "EXP_TIMING_STYLE"=48, "EXP_HEADSELECT"=49, "EXP_HORZPHASE"=50, "EXP_VERTPHASE"=51, "EXP_SPECIAL_SPEED"=52, "EXP_PRE_STRIPS"=53, "EXP_POST_STRIPS"=54, "EXP_PRE_LINES"=55, "EXP_POST_LINES"=56, "EXP_ACTIVE_LINES"=57, "EXP_ACTIVE_STRIPS"=58, "EXP_XFER_EXTRA"=59, "EXP_MIN_BLOCK"=60, "EXP_NUM_MIN_BLOCK"=61, "EXP_LOGIC_OUTPUT"=66, "EXP_VIDEO_BLANK"=67, "EXP_ZOOM_MODE_VIDEO"=68, "EXP_LEVEL_SYNC"=69, "EXP_DISABLE_LASER"=70, "EXP_ACQBACK_SHUTTER"=71, "EXP_ACQFLAT_SHUTTER"=72, "EXP_SMALL_CCD_MINEXP"=73, "EXP_LARGE_CCD_MINEXP"=74, "EXP_GATING_MODE"=75, "EXP_ILME_B1X"=76, "EXP_ILME_B2X"=77, "EXP_ILME_D1X"=78, "EXP_ILME_D2X"=79, "EXP_ILME_D4X"=80, "EXP_INIT_HW_ACCUM"=81, "EXP_5X_GAIN_ENABLE"=82, "EXP_RET_SRCCMP"=83, "EXP_EVENT_HANDLE"=84, "EXP_READOUT_MODE"=85, "EXP_SHUTTER_TYPE"=86, "EXP_USER_DEFINED_CHIP"=87, "EXP_USER_DEFINED_TIMING"=88, "EXP_CONTROLLER_VERSION"=89, "EXP_GET_CONTROLLER_VER"=90, "EXP_TTL_LINES"=91, "EXP_BIT_ADJUST"=92, "EXP_RESOLUTION"=93, "EXP_GAIN"=94, "EXP_ADC_RATE"=95, "EXP_ADC_TYPE"=96, "EXP_NUMBER_OF_CLEANS"=97, "EXP_NUM_OF_STRIPS_PER_CLN"=98, "EXP_INTERFACE_CARD"=99, "EXP_INTERRUPT"=100, "EXP_IO_ADDRESS1"=101, "EXP_IO_ADDRESS2"=102, "EXP_IO_ADDRESS3"=103, "EXP_HW_ROI"=104, "EXP_HW_BINNING"=105, "EXP_EDGE_TRIGGER"=106, "EXP_SHUTTER_CONTROL"=107, "EXP_RS170"=108, "EXP_RS170_COMPLEX"=109, "EXP_HW_RS170_LUT"=110, "EXP_RS170_INTENSITY_SCALING"=111, "EXP_RS170_OFFSET"=112, "EXP_RS170_PAN"=113, "EXP_RS170_ZOOM2X"=114, "EXP_RS170_ZOOM4X"=115, "EXP_RS170_BINNING"=116, "EXP_RS170_DECIMATION"=117, "EXP_HW_ACCUM"=118, "EXP_SHT_PREOPEN"=119, "EXP_STORE_STROBE"=120, "EXP_CONT_CLNS"=121, "EXP_TIMING_MODE"=122, "EXP_EXT_TRIGGER"=123, "EXP_EVENT_COUNTER"=124, "EXP_SW_TRIGGER"=125, "EXP_KINETICS_WINDOWSIZE"=126, "EXP_EXPOSURE"=127, "EXP_CONTROLLER_NAME"=128, "EXP_CCD_CHIP_NAME"=129, "EXP_BSWBINNING"=297, "EXP_EDGEENHANCE"=130, "EXP_BOXVIDEOGAIN"=131, "EXP_HSHADING_VALUE"=132, "EXP_VSHADING_VALUE"=133, "EXP_EDGEENHANCE_FLAG"=134, "EXP_SHADING_FLAG"=135, "EXP_GRAYSCALE"=136, "EXP_OFFSET"=137, "EXP_CCDGAIN"=138, "EXP_TEMPERATURE"=139, "EXP_MCPVOLTAGE"=140, "EXP_BOXEXPOSURE"=141, "EXP_ABC_FLAG"=142, "EXP_GAMMA_FLAG"=143, "EXP_AUTOBLACK_FLAG"=144, "EXP_AGC_FLAG"=145, "EXP_ODD_FIELD"=146, "EXP_FIELD_SELECT"=147, "EXP_RESET"=148, "EXP_EXTERN_ENABLE"=149, "EXP_CONTROLLERS_SUPPORTED"=150, "EXP_VTCLK"=151, "EXP_HTCLK"=152, "EXP_GATE_VS_CW"=153, "EXP_COM_PORT"=154, "EXP_US_UNITS"=156, "EXP_MS_UNITS"=157, "EXP_SEC_UNITS"=158, "EXP_MIN_UNITS"=159, "EXP_HRS_UNITS"=160, "EXP_FRAME_UNITS"=161, "EXP_SYNC_ASYNC"=162, "EXP_FOCUS_NFRAME"=163, "EXP_TIMEOUT"=164, "EXP_TIMEOUT_DEFAULT"=165, "EXP_HW_AUTOSTOP"=166, "EXP_RS170_INTEN_OFFSET"=167, "EXP_CONTROLLER_ALIVE"=168, "EXP_FOCUS_TYPE"=169, "EXP_FOCUS_ZOOM"=170, "EXP_FOCUS_PAN"=171, "EXP_MULTI_TAP_ROI"=172, "EXP_USE_INTERUPTS"=173, "EXP_DATA_ACQ_STATE"=174, "EXP_VERIFY_GOOD_VALUES"=175, "EXP_WHITE_CLAMP"=176, "EXP_BLACK_CLAMP"=177, "EXP_DELAY_TIME"=178, "EXP_READOUT_TIME"=179, "EXP_SW_DIAG"=180, "EXP_DIAG1"=181, "EXP_DIAG2"=182, "EXP_DIAG3"=183, "EXP_DIAG4"=184, "EXP_DIAG5"=185, "EXP_AorB_GROUP"=186, "EXP_ABSORBANCE_FLAG"=187, "EXP_ABSORBANCE_METHOD"=188, "EXP_ABSORBANCE_STRIPNUM"=189, "EXP_DMASIZE_VIA_DRIVER"=190, "EXP_DRIVERVERSION"=191, "EXP_NUM_DEVICES"=192, "EXP_ECPDMA_CHANNEL"=193, "EXP_CUSTOM_SHUTTER"=194, "EXP_ADC_OFFSET"=195, "EXP_CURRENT_READOUT_MODE"=196, "EXP_BANK_ADD"=197, "EXP_LUT_BANK"=198, "EXP_SETUP_STATUS"=201, "EXP_XY_GROUPING"=239, "EXP_MESSAGES_FLAG"=240, "EXP_TTL_LINE_TO_WAIT"=253, "EXP_DATA_COLLECTION_MODE"=258, "EXP_DATA_COLLECTION_TYPE"=262, "EXP_SKIPFRAMES"=274, "EXP_CLR_INT_CNTR"=276, "EXP_ENABLE_INT_CNTR"=277, "EXP_INT_CNTR"=278, "EXP_INTERNAL_SYNC_SRC"=279, "EXP_SW_EXTSYNC"=280, "EXP_PTG_PRESENT"=281, "EXP_ELEC_SHT"=282, "EXP_BOARDS_WITH_NVRAM"=283, "EXP_ANLGMASTER_ST143"=284, "EXP_ANLGSLAVE_ST143"=285, "EXP_DISPLAY_ST143"=286, "EXP_INTRFACE_ST143"=287, "EXP_SCANCONTROL_ST143"=288, "EXP_NUMBERFRAMES_IRQ"=204, "EXP_COOL_TYPE"=214, "EXP_HD_TYPE"=215, "EXP_INTENSIFER_GAIN"=216, "EXP_SHT_GATE_MODE"=217, "EXP_HD_CHECK"=218, "EXP_AMP_MODE"=219, "EXP_AMP_DIALOG"=247, "EXP_ANALOG_GAIN"=220, "EXP_HW_FIXES"=221, "EXP_PCI_CARDS"=222, "EXP_NOT_REVERSE"=223, "EXP_LOAD_NVRAM_DEFAULTS"=234, "EXP_CNTR_BRD"=235, "EXP_XDIMHW"=237, "EXP_YDIMHW"=238, "EXP_SPECIAL_FAST_RDOUT"=254, "EXP_SPCL_FAST_Y_DIM"=255, "EXP_SPCL_FAST_X_DIM"=256, "EXP_SPCL_FAST_Y_INDEX"=257, "EXP_SHUTTER_COMP_TIME_MS"=266, "EXP_NVRAM_AVAIL"=267, "EXP_NUMBER_AGAIN_AVAIL"=269, "EXP_SENSOR_TYPE"=270, "EXP_EVENT_TYPE"=292, "EXP_ANTI_BLOOMING"=293, "EXP_FAST_PULSE_ENABLE"=233, "EXP_USE_HEADCALIB"=296, "EXP_TEMP_STATUS"=301, "EXP_MULTIPLE_READMODES_LIVE"=302, "EXP_FIRST_ACQUIRE_FLAG"=303, "EXP_ANTI_BLOOMING_CONTROL"=304, "EXP_PRE_HORZ_DELAY"=305, "EXP_NVRAM_TRIES"=306, "EXP_XASCEND"=307, "EXP_YASCEND"=308, "EXP_ALT_TIMING"=309, "EXP_SHUTTER_PRE_COMP"=310, "EXP_PVCAM_POSSIBLE"=311, "EXP_ADC_IN_NVRAM"=312, "EXP_PASSTHRU_MODE"=313, "EXP_FIRMWAREVERSION"=314, "EXP_IMMEDIATE_SHUTTER"=315, "EXP_STAGE2_TEMP"=316, "EXP_AVGAIN_ENABLED"=317, "EXP_AVGAIN_SETPOINT"=318, "EXP_AVGAIN"=319, "EXP_AVGAIN_CALIB_TEMP"=320, "EXP_AVGAIN_CALIB_COEFF1"=321, "EXP_AVGAIN_CALIB_COEFF2"=322, "EXP_AVGAIN_CALIB_COEFF3"=323, "EXP_AVGAIN_CALIB_COEFF4"=324, "EXP_AVGAIN_CALIB_COEFF5"=325, "EXP_FORCE_READOUT_MODE"=326, "EXP_RESET_DATACOLLECTION"=327, "EXP_ACTIVE_SUBFRAME"=328, "EXP_PV_READOUT_PORT"=514, "EXP_CLASSNAME"=775, "EXP_FLATFLDNAME"=776, "EXP_DARKNAME"=777, "EXP_SETUPNAME"=778, "EXP_ACCESSNAME"=779, "EXP_DATFILENAME"=780, "EXP_ABSORBFILENAME"=781, "EXP_BLEMISHFILENAME"=782, "EXP_COSMICFILENAME"=783, "EXP_FILEINCBASENAME"=784, "EXP_YTNAME"=785, "EXP_DEVNAME"=786, "EXP_USEROI"=787, "EXP_DOBLEMISH"=788, "EXP_DOABSORB"=789, "EXP_DOCOSMIC"=790, "EXP_COSMICSENS"=791, "EXP_ABSORBSTRIP"=792, "EXP_DATATYPE"=793, "EXP_OVERWRITECONFIRM"=794, "EXP_FILEINCENABLE"=795, "EXP_FILEINCCOUNT"=796, "EXP_RUNNING"=797, "EXP_SAVEROPT"=798, "EXP_TIME_UNITS"=799, "EXP_FILEACCESS"=800, "EXP_AUTOSAVE"=801, "EXP_NEWWINDOW"=802, "EXP_XDIM"=803, "EXP_YDIM"=804, "EXP_XDIMDET"=805, "EXP_YDIMDET"=806, "EXP_ROIMODE"=807, "EXP_NUMREPEATSEXP"=808, "EXP_NUMACCUMSEXP"=809, "EXP_THREADSTATE"=810, "EXP_USEMINTHRESHOLDING"=811, "EXP_MINTHRESHOLDVALUE"=812, "EXP_USEMAXTHRESHOLDING"=813, "EXP_MAXTHRESHOLDVALUE"=814, "EXP_RUNNING_EXPERIMENT"=815, "EXP_THRESHOLD_DEMAND_UPDATE"=816, "EXP_ROICOUNT"=817, "EXP_ACCUMS"=818, "EXP_CACCUMS"=819, "EXP_CSEQUENTS"=820, "EXP_PHOTON_ESTIMATION_ENABLE"=821, "EXP_PHOTON_MAXTIME"=822, "EXP_PHOTON_MAXTIMEUNIT"=823, "EXP_CUSTOMFILTER_ENABLE"=824, "EXP_CUSTOMFILTER_SIZE"=825, "EXP_LOOKUPTABLE_ENABLE"=826, "EXP_BSHOWWINDOW"=827, "EXP_BBACKSUBTRACT"=828, "EXP_BDOFLATFIELD"=829, "EXP_ASCIIOUTPUTFILE"=830, "EXP_ASCIIOUTPUT_DELIMITER"=831, "EXP_ASCIIOUTPUT_TERMINATOR"=832, "EXP_FFTYPE"=833, "EXP_BGTYPE"=834, "EXP_COSGRASS"=835, "EXP_RUNASCONFIRM"=836, "EXP_RUNASRUNACCESS"=837, "EXP_DATAFILETYPE"=838, "EXP_ROTATE"=839, "EXP_FLIP"=840, "EXP_REVERSE"=841, "EXP_SWBINNING"=842, "EXP_AUTOSTORE"=843, "EXP_XBINNED"=844, "EXP_YBINNED"=845, "EXP_NUMPATTERNS"=846, "EXP_EXPERIMENTTIME"=847, "EXP_ASYNCSEQUENTIALS"=848, "EXP_SEQUENTIALS"=849, "EXP_CSEQUENTIALS"=850, "EXP_AUTOD"=851, "EXP_EXPOSURETIME"=852, "EXP_EXPOSURETIME_UNITS"=853, "EXP_ACQMODE"=854, "EXP_DMASIZE_PVCAM"=855, "EXP_INITIALIZE"=856, "EXP_CELL_X_SIZE"=857, "EXP_CELL_Y_SIZE"=858, "EXP_X_GAP_SIZE"=859, "EXP_Y_GAP_SIZE"=860] ("Param")
            # "start streaming data"
            n275 = local read "error reader"() -> (w395:errorcluster)
            n276 = local read "OMA V exposure time"() -> (w390:dbl)
            n277 = local read "experiment reference"() -> (w389:refnum<k7>)
            n278 = local read "reader endpoint"() -> (w396:refnum<k21>)
            n279 = local read "writer endpoint"() -> (w398:refnum<k21>)
            n280 = invoke class="IExpSetup2" method="SetParam"(reference=w389, "Param"=w388, "pSetVal"=w390) -> (reference out=w386:refnum<k7>)  [unwired: 2 in, 4 out]
            n281 = local read "file reference"() -> (w387:refnum<k7>)
            n282 = local read "error writer"() -> (w397:errorcluster)
            n283 = while {
              shift-right: [w417] -> w394
              shift-left: w398 -> [w423]
              shift-right: [w416] -> w393
              shift-left: w397 -> [w422]
              shift-right: [w419] -> w392
              shift-left: w396 -> [w421]
              shift-right: [w418] -> w391
              shift-left: w395 -> [w420]
              tunnel: w386 -> [w414]
              shift-right: [w413] -> _
              shift-left: w387 -> [w415]
              i -> [w412]
              stop <- w424 stop-if-true
              n284 = flat-sequence {
                tunnel: w420 -> [w429]
                tunnel: w421 -> [w430]
                tunnel: w422 -> [w431]
                tunnel: w423 -> [w432]
                tunnel: [w432] -> w411
                tunnel: [w431] -> w410
                tunnel: [w430] -> w409
                tunnel: [w429] -> w408
                tunnel: [w442] -> w427
                tunnel: [w441] -> w426
                tunnel: [w433] -> w425
                tunnel: [w438] -> w419
                tunnel: [w437] -> w418
                tunnel: w411 -> [w442]
                tunnel: w410 -> [w441]
                tunnel: w409 -> [w440]
                tunnel: w408 -> [w439]
                tunnel: w427 -> [w459]
                tunnel: w426 -> [w458]
                tunnel: w425 -> [w455]
                tunnel: w415 -> [w454]
                tunnel: w414 -> [w453]
                tunnel: w412 -> [w451]
                tunnel: [w455] -> w407
                tunnel: [w457] -> w406
                tunnel: [w456] -> w405
                tunnel: [w452] -> w404
                tunnel: [w543] -> w413
                tunnel: [w544] -> w416
                tunnel: [w545] -> w417
                tunnel: [w546] -> w424
                tunnel: w407 -> [w546]
                tunnel: w406 -> [w545]
                tunnel: w405 -> [w544]
                tunnel: w404 -> [w543]
                frame #0 {
                  n285 = Tick Count (ms)() -> (millisecond timer value=w428:u32)
                  n286 = local write "time start (ms)"(w428) -> ()
                }
                frame #1 {
                  # "experiment ready to acquire?"
                  n287 = while {
                    tunnel: [w444] -> w436
                    tunnel: [w445] -> w435
                    shift-right: [w447] -> w438
                    shift-left: w440 -> [w449]
                    shift-right: [w446] -> w437
                    shift-left: w439 -> [w448]
                    stop <- w443 continue-if-true
                    n288 = local read "standby stream"() -> (w444:bool)
                    n289 = shared-variable-read(w449, w448, 1000 ("timeout ms (-1)")) -> (w447:refnum<k21>, w446:errorcluster, w445:bool)  [unwired: 1 out]
                    n290 = And(x=w445, y=w444) -> (x .and. y?=w443:bool)
                  }
                  n291 = Not(x=w436) -> (.not. x?=w434:bool)
                  n292 = And(x=w435, y=w434) -> (x .and. y?=w433:bool)
                }
                frame #2 {
                  n293 = case shown="False" w455 {
                    tunnel: [w470 w536] -> w456
                    tunnel: [w469 w537] -> w457
                    tunnel: w458 -> [w468 w536]
                    tunnel: w459 -> [w467 w537]
                    tunnel: w454 -> [w464 w535]
                    tunnel: w453 -> [w463 w534]
                    tunnel: [w462 w535] -> w452
                    tunnel: w451 -> [w460 _]
                    frame False {
                      # "acquire"
                      n294 = flat-sequence {
                        tunnel: w467 -> [w490]
                        tunnel: w468 -> [w491]
                        tunnel: [w491] -> w466
                        tunnel: [w490] -> w465
                        tunnel: w464 -> [w489]
                        tunnel: w463 -> [w488]
                        tunnel: [w472] -> _
                        tunnel: [w477] -> w462
                        tunnel: [w476] -> w461
                        tunnel: w460 -> [w475]
                        tunnel: [w531] -> w470
                        tunnel: [w530] -> w469
                        tunnel: w466 -> [w529]
                        tunnel: w465 -> [w528]
                        tunnel: w461 -> [w527]
                        frame #0 {
                          n295 = invoke class="IExpSetup2" method="Start"(reference=w488, "pFile"=w489) -> (reference out=w487:refnum<k7>, "pFile"=w472:refnum<k7>)  [unwired: 2 in, 2 out]
                          n296 = while {
                            tunnel: w487 -> [w521]
                            tunnel: w472 -> [w519]
                            tunnel: [w519] -> w471
                            stop <- w520 stop-if-true
                            w524 = 797 items=["EXP_ETACTUAL"=1, "EXP_SEQUENTS"=2, "EXP_ERROR"=3, "EXP_GETCAPS"=4, "EXP_GETPLSR"=5, "EXP_DETECTOR_BIT"=16, "EXP_RUNNING_APP"=23, "EXP_VIDEO_TYPE"=24, "EXP_CUSTOM_VIDEO_X"=25, "EXP_CUSTOM_VIDEO_Y"=26, "EXP_CUSTOM_VIDEO_FSTWIDTH"=27, "EXP_CUSTOM_VIDEO_LSTWIDTH"=28, "EXP_VIDEO_XDIM"=29, "EXP_VIDEO_YDIM"=30, "EXP_VIDEO_MAX_ZOOM"=31, "EXP_VIDEO_HORZ_PAN"=32, "EXP_VIDEO_VERT_PAN"=33, "EXP_WORD_MULTIPLIER"=34, "EXP_TARGET_ID"=35, "EXP_ADAPTER_ID"=36, "EXP_NUMADAPTORS"=37, "EXP_FORCE_PP_INIT"=38, "EXP_NOP_ADC"=39, "EXP_ACTUAL_TEMP"=40, "EXP_FORCE_AUTOSTOP"=41, "EXP_DEFAULT_VTCLK"=42, "EXP_MIN_VTCLK"=43, "EXP_MAX_VTCLK"=44, "EXP_DEFAULT_HTCLK"=45, "EXP_MIN_HTCLK"=46, "EXP_MAX_HTCLK"=47, "EXP_TIMING_STYLE"=48, "EXP_HEADSELECT"=49, "EXP_HORZPHASE"=50, "EXP_VERTPHASE"=51, "EXP_SPECIAL_SPEED"=52, "EXP_PRE_STRIPS"=53, "EXP_POST_STRIPS"=54, "EXP_PRE_LINES"=55, "EXP_POST_LINES"=56, "EXP_ACTIVE_LINES"=57, "EXP_ACTIVE_STRIPS"=58, "EXP_XFER_EXTRA"=59, "EXP_MIN_BLOCK"=60, "EXP_NUM_MIN_BLOCK"=61, "EXP_LOGIC_OUTPUT"=66, "EXP_VIDEO_BLANK"=67, "EXP_ZOOM_MODE_VIDEO"=68, "EXP_LEVEL_SYNC"=69, "EXP_DISABLE_LASER"=70, "EXP_ACQBACK_SHUTTER"=71, "EXP_ACQFLAT_SHUTTER"=72, "EXP_SMALL_CCD_MINEXP"=73, "EXP_LARGE_CCD_MINEXP"=74, "EXP_GATING_MODE"=75, "EXP_ILME_B1X"=76, "EXP_ILME_B2X"=77, "EXP_ILME_D1X"=78, "EXP_ILME_D2X"=79, "EXP_ILME_D4X"=80, "EXP_INIT_HW_ACCUM"=81, "EXP_5X_GAIN_ENABLE"=82, "EXP_RET_SRCCMP"=83, "EXP_EVENT_HANDLE"=84, "EXP_READOUT_MODE"=85, "EXP_SHUTTER_TYPE"=86, "EXP_USER_DEFINED_CHIP"=87, "EXP_USER_DEFINED_TIMING"=88, "EXP_CONTROLLER_VERSION"=89, "EXP_GET_CONTROLLER_VER"=90, "EXP_TTL_LINES"=91, "EXP_BIT_ADJUST"=92, "EXP_RESOLUTION"=93, "EXP_GAIN"=94, "EXP_ADC_RATE"=95, "EXP_ADC_TYPE"=96, "EXP_NUMBER_OF_CLEANS"=97, "EXP_NUM_OF_STRIPS_PER_CLN"=98, "EXP_INTERFACE_CARD"=99, "EXP_INTERRUPT"=100, "EXP_IO_ADDRESS1"=101, "EXP_IO_ADDRESS2"=102, "EXP_IO_ADDRESS3"=103, "EXP_HW_ROI"=104, "EXP_HW_BINNING"=105, "EXP_EDGE_TRIGGER"=106, "EXP_SHUTTER_CONTROL"=107, "EXP_RS170"=108, "EXP_RS170_COMPLEX"=109, "EXP_HW_RS170_LUT"=110, "EXP_RS170_INTENSITY_SCALING"=111, "EXP_RS170_OFFSET"=112, "EXP_RS170_PAN"=113, "EXP_RS170_ZOOM2X"=114, "EXP_RS170_ZOOM4X"=115, "EXP_RS170_BINNING"=116, "EXP_RS170_DECIMATION"=117, "EXP_HW_ACCUM"=118, "EXP_SHT_PREOPEN"=119, "EXP_STORE_STROBE"=120, "EXP_CONT_CLNS"=121, "EXP_TIMING_MODE"=122, "EXP_EXT_TRIGGER"=123, "EXP_EVENT_COUNTER"=124, "EXP_SW_TRIGGER"=125, "EXP_KINETICS_WINDOWSIZE"=126, "EXP_EXPOSURE"=127, "EXP_CONTROLLER_NAME"=128, "EXP_CCD_CHIP_NAME"=129, "EXP_BSWBINNING"=297, "EXP_EDGEENHANCE"=130, "EXP_BOXVIDEOGAIN"=131, "EXP_HSHADING_VALUE"=132, "EXP_VSHADING_VALUE"=133, "EXP_EDGEENHANCE_FLAG"=134, "EXP_SHADING_FLAG"=135, "EXP_GRAYSCALE"=136, "EXP_OFFSET"=137, "EXP_CCDGAIN"=138, "EXP_TEMPERATURE"=139, "EXP_MCPVOLTAGE"=140, "EXP_BOXEXPOSURE"=141, "EXP_ABC_FLAG"=142, "EXP_GAMMA_FLAG"=143, "EXP_AUTOBLACK_FLAG"=144, "EXP_AGC_FLAG"=145, "EXP_ODD_FIELD"=146, "EXP_FIELD_SELECT"=147, "EXP_RESET"=148, "EXP_EXTERN_ENABLE"=149, "EXP_CONTROLLERS_SUPPORTED"=150, "EXP_VTCLK"=151, "EXP_HTCLK"=152, "EXP_GATE_VS_CW"=153, "EXP_COM_PORT"=154, "EXP_US_UNITS"=156, "EXP_MS_UNITS"=157, "EXP_SEC_UNITS"=158, "EXP_MIN_UNITS"=159, "EXP_HRS_UNITS"=160, "EXP_FRAME_UNITS"=161, "EXP_SYNC_ASYNC"=162, "EXP_FOCUS_NFRAME"=163, "EXP_TIMEOUT"=164, "EXP_TIMEOUT_DEFAULT"=165, "EXP_HW_AUTOSTOP"=166, "EXP_RS170_INTEN_OFFSET"=167, "EXP_CONTROLLER_ALIVE"=168, "EXP_FOCUS_TYPE"=169, "EXP_FOCUS_ZOOM"=170, "EXP_FOCUS_PAN"=171, "EXP_MULTI_TAP_ROI"=172, "EXP_USE_INTERUPTS"=173, "EXP_DATA_ACQ_STATE"=174, "EXP_VERIFY_GOOD_VALUES"=175, "EXP_WHITE_CLAMP"=176, "EXP_BLACK_CLAMP"=177, "EXP_DELAY_TIME"=178, "EXP_READOUT_TIME"=179, "EXP_SW_DIAG"=180, "EXP_DIAG1"=181, "EXP_DIAG2"=182, "EXP_DIAG3"=183, "EXP_DIAG4"=184, "EXP_DIAG5"=185, "EXP_AorB_GROUP"=186, "EXP_ABSORBANCE_FLAG"=187, "EXP_ABSORBANCE_METHOD"=188, "EXP_ABSORBANCE_STRIPNUM"=189, "EXP_DMASIZE_VIA_DRIVER"=190, "EXP_DRIVERVERSION"=191, "EXP_NUM_DEVICES"=192, "EXP_ECPDMA_CHANNEL"=193, "EXP_CUSTOM_SHUTTER"=194, "EXP_ADC_OFFSET"=195, "EXP_CURRENT_READOUT_MODE"=196, "EXP_BANK_ADD"=197, "EXP_LUT_BANK"=198, "EXP_SETUP_STATUS"=201, "EXP_XY_GROUPING"=239, "EXP_MESSAGES_FLAG"=240, "EXP_TTL_LINE_TO_WAIT"=253, "EXP_DATA_COLLECTION_MODE"=258, "EXP_DATA_COLLECTION_TYPE"=262, "EXP_SKIPFRAMES"=274, "EXP_CLR_INT_CNTR"=276, "EXP_ENABLE_INT_CNTR"=277, "EXP_INT_CNTR"=278, "EXP_INTERNAL_SYNC_SRC"=279, "EXP_SW_EXTSYNC"=280, "EXP_PTG_PRESENT"=281, "EXP_ELEC_SHT"=282, "EXP_BOARDS_WITH_NVRAM"=283, "EXP_ANLGMASTER_ST143"=284, "EXP_ANLGSLAVE_ST143"=285, "EXP_DISPLAY_ST143"=286, "EXP_INTRFACE_ST143"=287, "EXP_SCANCONTROL_ST143"=288, "EXP_NUMBERFRAMES_IRQ"=204, "EXP_COOL_TYPE"=214, "EXP_HD_TYPE"=215, "EXP_INTENSIFER_GAIN"=216, "EXP_SHT_GATE_MODE"=217, "EXP_HD_CHECK"=218, "EXP_AMP_MODE"=219, "EXP_AMP_DIALOG"=247, "EXP_ANALOG_GAIN"=220, "EXP_HW_FIXES"=221, "EXP_PCI_CARDS"=222, "EXP_NOT_REVERSE"=223, "EXP_LOAD_NVRAM_DEFAULTS"=234, "EXP_CNTR_BRD"=235, "EXP_XDIMHW"=237, "EXP_YDIMHW"=238, "EXP_SPECIAL_FAST_RDOUT"=254, "EXP_SPCL_FAST_Y_DIM"=255, "EXP_SPCL_FAST_X_DIM"=256, "EXP_SPCL_FAST_Y_INDEX"=257, "EXP_SHUTTER_COMP_TIME_MS"=266, "EXP_NVRAM_AVAIL"=267, "EXP_NUMBER_AGAIN_AVAIL"=269, "EXP_SENSOR_TYPE"=270, "EXP_EVENT_TYPE"=292, "EXP_ANTI_BLOOMING"=293, "EXP_FAST_PULSE_ENABLE"=233, "EXP_USE_HEADCALIB"=296, "EXP_TEMP_STATUS"=301, "EXP_MULTIPLE_READMODES_LIVE"=302, "EXP_FIRST_ACQUIRE_FLAG"=303, "EXP_ANTI_BLOOMING_CONTROL"=304, "EXP_PRE_HORZ_DELAY"=305, "EXP_NVRAM_TRIES"=306, "EXP_XASCEND"=307, "EXP_YASCEND"=308, "EXP_ALT_TIMING"=309, "EXP_SHUTTER_PRE_COMP"=310, "EXP_PVCAM_POSSIBLE"=311, "EXP_ADC_IN_NVRAM"=312, "EXP_PASSTHRU_MODE"=313, "EXP_FIRMWAREVERSION"=314, "EXP_IMMEDIATE_SHUTTER"=315, "EXP_STAGE2_TEMP"=316, "EXP_AVGAIN_ENABLED"=317, "EXP_AVGAIN_SETPOINT"=318, "EXP_AVGAIN"=319, "EXP_AVGAIN_CALIB_TEMP"=320, "EXP_AVGAIN_CALIB_COEFF1"=321, "EXP_AVGAIN_CALIB_COEFF2"=322, "EXP_AVGAIN_CALIB_COEFF3"=323, "EXP_AVGAIN_CALIB_COEFF4"=324, "EXP_AVGAIN_CALIB_COEFF5"=325, "EXP_FORCE_READOUT_MODE"=326, "EXP_RESET_DATACOLLECTION"=327, "EXP_ACTIVE_SUBFRAME"=328, "EXP_PV_READOUT_PORT"=514, "EXP_CLASSNAME"=775, "EXP_FLATFLDNAME"=776, "EXP_DARKNAME"=777, "EXP_SETUPNAME"=778, "EXP_ACCESSNAME"=779, "EXP_DATFILENAME"=780, "EXP_ABSORBFILENAME"=781, "EXP_BLEMISHFILENAME"=782, "EXP_COSMICFILENAME"=783, "EXP_FILEINCBASENAME"=784, "EXP_YTNAME"=785, "EXP_DEVNAME"=786, "EXP_USEROI"=787, "EXP_DOBLEMISH"=788, "EXP_DOABSORB"=789, "EXP_DOCOSMIC"=790, "EXP_COSMICSENS"=791, "EXP_ABSORBSTRIP"=792, "EXP_DATATYPE"=793, "EXP_OVERWRITECONFIRM"=794, "EXP_FILEINCENABLE"=795, "EXP_FILEINCCOUNT"=796, "EXP_RUNNING"=797, "EXP_SAVEROPT"=798, "EXP_TIME_UNITS"=799, "EXP_FILEACCESS"=800, "EXP_AUTOSAVE"=801, "EXP_NEWWINDOW"=802, "EXP_XDIM"=803, "EXP_YDIM"=804, "EXP_XDIMDET"=805, "EXP_YDIMDET"=806, "EXP_ROIMODE"=807, "EXP_NUMREPEATSEXP"=808, "EXP_NUMACCUMSEXP"=809, "EXP_THREADSTATE"=810, "EXP_USEMINTHRESHOLDING"=811, "EXP_MINTHRESHOLDVALUE"=812, "EXP_USEMAXTHRESHOLDING"=813, "EXP_MAXTHRESHOLDVALUE"=814, "EXP_RUNNING_EXPERIMENT"=815, "EXP_THRESHOLD_DEMAND_UPDATE"=816, "EXP_ROICOUNT"=817, "EXP_ACCUMS"=818, "EXP_CACCUMS"=819, "EXP_CSEQUENTS"=820, "EXP_PHOTON_ESTIMATION_ENABLE"=821, "EXP_PHOTON_MAXTIME"=822, "EXP_PHOTON_MAXTIMEUNIT"=823, "EXP_CUSTOMFILTER_ENABLE"=824, "EXP_CUSTOMFILTER_SIZE"=825, "EXP_LOOKUPTABLE_ENABLE"=826, "EXP_BSHOWWINDOW"=827, "EXP_BBACKSUBTRACT"=828, "EXP_BDOFLATFIELD"=829, "EXP_ASCIIOUTPUTFILE"=830, "EXP_ASCIIOUTPUT_DELIMITER"=831, "EXP_ASCIIOUTPUT_TERMINATOR"=832, "EXP_FFTYPE"=833, "EXP_BGTYPE"=834, "EXP_COSGRASS"=835, "EXP_RUNASCONFIRM"=836, "EXP_RUNASRUNACCESS"=837, "EXP_DATAFILETYPE"=838, "EXP_ROTATE"=839, "EXP_FLIP"=840, "EXP_REVERSE"=841, "EXP_SWBINNING"=842, "EXP_AUTOSTORE"=843, "EXP_XBINNED"=844, "EXP_YBINNED"=845, "EXP_NUMPATTERNS"=846, "EXP_EXPERIMENTTIME"=847, "EXP_ASYNCSEQUENTIALS"=848, "EXP_SEQUENTIALS"=849, "EXP_CSEQUENTIALS"=850, "EXP_AUTOD"=851, "EXP_EXPOSURETIME"=852, "EXP_EXPOSURETIME_UNITS"=853, "EXP_ACQMODE"=854, "EXP_DMASIZE_PVCAM"=855, "EXP_INITIALIZE"=856, "EXP_CELL_X_SIZE"=857, "EXP_CELL_Y_SIZE"=858, "EXP_X_GAP_SIZE"=859, "EXP_Y_GAP_SIZE"=860] ("Param")
                            # "acquire"
                            n297 = invoke class="IExpSetup2" method="GetParam"(reference=w521, "Param"=w524) -> ("GetParam"=w523:variant)  [unwired: 3 in, 4 out]
                            n298 = Variant To Data(type=FALSE, Variant=w523) -> (data=w522:bool)  [unwired: 1 in, 1 out]
                            n299 = Not(x=w522) -> (.not. x?=w520:bool)
                            n300 = Wait (ms)(milliseconds to wait=u32 5) -> ()  [unwired: 1 out]
                          }
                          n301 = Equal To 0?(x=w475) -> (x = 0?=w474:bool)
                          n302 = local read "FrameVariant"() -> (w482:variant)
                          n303 = invoke class="IDocFile" method="GetFrame"(reference=w471, "frame"=i16 1, "FrameVariant"=w482) -> (reference out=w477:refnum<k7>, "FrameVariant"=w480:variant)  [unwired: 2 in, 3 out]
                          n304 = local read "frame array"() -> (w473:i32[][])
                          n305 = Variant To Data(type=w473, Variant=w480) -> (data=w481:i32[][])  [unwired: 1 in, 1 out]
                          n306 = Index Array(array=w481, index (col)=0 ("disabled index (col)")) -> (element=w484:i32[])  [unwired: 1 in]
                          n307 = case shown="True" w474 {
                            tunnel: w477 -> [_ w497]
                            tunnel: w484 -> [w492 w493]
                            tunnel: [w492 w493] -> w485
                            frame False {
                            }
                            frame True {
                              n308 = invoke class="IDocFile" method="GetCalibration"(reference=w497) -> ("GetCalibration"=w499:refnum<k7>)  [unwired: 2 in, 2 out]
                              n309 = Array Size(array=w493) -> (size(s)=w494:i32)
                              n310 = property class="ICalibObj"(reference=w499) -> (reference out=w495:refnum<k7>, "PairCount"=w500:u8)  [unwired: 1 in, 1 out]
                              n311 = for {
                                N: w500 -> [_]
                                tunnel: w495 -> [w517]
                                tunnel: [w518] -> w502 mode=indexing
                                tunnel: [w515] -> w501 mode=indexing
                                i -> [w516]
                                n312 = invoke class="ICalibObj" method="CalibVal"(reference=w517, "index"=w516) -> ("CalibVal"=w518:dbl)  [unwired: 2 in, 3 out]
                                n313 = invoke class="ICalibObj" method="PixelLoc"(reference=w517, "index"=w516) -> ("PixelLoc"=w515:dbl)  [unwired: 2 in, 3 out]
                              }
                              n314 = for {
                                N: w494 -> [_]
                                tunnel: w502 -> [w514]
                                tunnel: [w513] -> w496 mode=indexing
                                tunnel: [w512] -> _ mode=indexing
                                tunnel: w501 -> [w511]
                                tunnel: 1 ("index") -> [w503]
                                i -> [w510]
                                n315 = Divide(x=w503, y=2) -> (x/y=w507:dbl)
                                n316 = Round To Nearest(number=w507) -> (nearest integer value=w505:dbl)
                                n317 = Multiply(x=w510, y=w503) -> (x*y=w506:i32)
                                n318 = Increment(x=w505) -> (x+1=w504:dbl)
                                n319 = Add(x=w506, y=w504) -> (x+y=w509:dbl)
                                n320 = call <vilib>:"Polynomial Interpolation.vi"("x value"=w509, "X"=w511, "Y"=w514) -> ("interpolation error"=w512:dbl, "interpolation value"=w513:dbl)  [unwired: 1 out]
                              }
                              n321 = local write "Wavelength Scale"(w496) -> ()
                            }
                          }
                          n322 = local read "Wavelength Scale"() -> (w483:dbl[])
                          n323 = Add Array Elements(numeric array=w485) -> (sum=w486:i32)
                          n324 = Bundle("Wavelength Scale"=w483, "frame array"=w485) -> (w476:T3)  [unwired: 1 in]
                          n325 = local write "XY Graph Spectrum"(w476) -> ()
                          n326 = local write "Time Trace"(w486) -> ()
                          n327 = local write "Intensity Sum"(w486) -> ()
                        }
                        frame #1 {
                          # "send data"
                          n328 = shared-variable-write(w528, w529, w527) -> (w532:refnum<k21>, w533:errorcluster)  [unwired: 1 in, 1 out]
                          n329 = Flush Stream(8:w533, 11:w532) -> (0:w531:errorcluster, 3:w530:refnum<k21>)  [unwired: 2 in, 1 out]
                        }
                      }
                    }
                    frame True {
                      n330 = invoke class="IExpSetup2" method="Stop"(reference=w534) -> ()  [unwired: 2 in, 3 out]
                    }
                  }
                }
                frame #3 {
                  n331 = local read "time start (ms)"() -> (w541:i32)
                  n332 = Tick Count (ms)() -> (millisecond timer value=w542:u32)
                  n333 = Subtract(x=w542, y=w541) -> (x-y=w540:u32)
                  n334 = Divide(x=w540, y=u32 1000) -> (x/y=w539:dbl)
                  n335 = local write "time elapsed (s)"(w539) -> ()
                }
              }
            }
            n336 = flat-sequence {
              tunnel: w394 -> [w402]
              tunnel: w393 -> [w401]
              tunnel: w392 -> [w400]
              tunnel: w391 -> [w399]
              frame #0 {
                n337 = local write "writer endpoint"(w402) -> ()
                n338 = local write "error writer"(w401) -> ()
                n339 = local write "error reader"(w399) -> ()
                n340 = local write "reader endpoint"(w400) -> ()
              }
              frame #1 {
                w403 = FALSE ("busy")
                n341 = local write "busy"(w403) -> ()
                n342 = local write "Start Stream"(w403) -> ()
              }
            }
          }
          frame 14 {
            # "start continuous spectra fast"
            n343 = flat-sequence {
              frame #0 {
                n344 = Tick Count (ms)() -> (millisecond timer value=w547:u32)
                n345 = local write "time start (ms)"(w547) -> ()
              }
              frame #1 {
                w553 = 127 items=["EXP_ETACTUAL"=1, "EXP_SEQUENTS"=2, "EXP_ERROR"=3, "EXP_GETCAPS"=4, "EXP_GETPLSR"=5, "EXP_DETECTOR_BIT"=16, "EXP_RUNNING_APP"=23, "EXP_VIDEO_TYPE"=24, "EXP_CUSTOM_VIDEO_X"=25, "EXP_CUSTOM_VIDEO_Y"=26, "EXP_CUSTOM_VIDEO_FSTWIDTH"=27, "EXP_CUSTOM_VIDEO_LSTWIDTH"=28, "EXP_VIDEO_XDIM"=29, "EXP_VIDEO_YDIM"=30, "EXP_VIDEO_MAX_ZOOM"=31, "EXP_VIDEO_HORZ_PAN"=32, "EXP_VIDEO_VERT_PAN"=33, "EXP_WORD_MULTIPLIER"=34, "EXP_TARGET_ID"=35, "EXP_ADAPTER_ID"=36, "EXP_NUMADAPTORS"=37, "EXP_FORCE_PP_INIT"=38, "EXP_NOP_ADC"=39, "EXP_ACTUAL_TEMP"=40, "EXP_FORCE_AUTOSTOP"=41, "EXP_DEFAULT_VTCLK"=42, "EXP_MIN_VTCLK"=43, "EXP_MAX_VTCLK"=44, "EXP_DEFAULT_HTCLK"=45, "EXP_MIN_HTCLK"=46, "EXP_MAX_HTCLK"=47, "EXP_TIMING_STYLE"=48, "EXP_HEADSELECT"=49, "EXP_HORZPHASE"=50, "EXP_VERTPHASE"=51, "EXP_SPECIAL_SPEED"=52, "EXP_PRE_STRIPS"=53, "EXP_POST_STRIPS"=54, "EXP_PRE_LINES"=55, "EXP_POST_LINES"=56, "EXP_ACTIVE_LINES"=57, "EXP_ACTIVE_STRIPS"=58, "EXP_XFER_EXTRA"=59, "EXP_MIN_BLOCK"=60, "EXP_NUM_MIN_BLOCK"=61, "EXP_LOGIC_OUTPUT"=66, "EXP_VIDEO_BLANK"=67, "EXP_ZOOM_MODE_VIDEO"=68, "EXP_LEVEL_SYNC"=69, "EXP_DISABLE_LASER"=70, "EXP_ACQBACK_SHUTTER"=71, "EXP_ACQFLAT_SHUTTER"=72, "EXP_SMALL_CCD_MINEXP"=73, "EXP_LARGE_CCD_MINEXP"=74, "EXP_GATING_MODE"=75, "EXP_ILME_B1X"=76, "EXP_ILME_B2X"=77, "EXP_ILME_D1X"=78, "EXP_ILME_D2X"=79, "EXP_ILME_D4X"=80, "EXP_INIT_HW_ACCUM"=81, "EXP_5X_GAIN_ENABLE"=82, "EXP_RET_SRCCMP"=83, "EXP_EVENT_HANDLE"=84, "EXP_READOUT_MODE"=85, "EXP_SHUTTER_TYPE"=86, "EXP_USER_DEFINED_CHIP"=87, "EXP_USER_DEFINED_TIMING"=88, "EXP_CONTROLLER_VERSION"=89, "EXP_GET_CONTROLLER_VER"=90, "EXP_TTL_LINES"=91, "EXP_BIT_ADJUST"=92, "EXP_RESOLUTION"=93, "EXP_GAIN"=94, "EXP_ADC_RATE"=95, "EXP_ADC_TYPE"=96, "EXP_NUMBER_OF_CLEANS"=97, "EXP_NUM_OF_STRIPS_PER_CLN"=98, "EXP_INTERFACE_CARD"=99, "EXP_INTERRUPT"=100, "EXP_IO_ADDRESS1"=101, "EXP_IO_ADDRESS2"=102, "EXP_IO_ADDRESS3"=103, "EXP_HW_ROI"=104, "EXP_HW_BINNING"=105, "EXP_EDGE_TRIGGER"=106, "EXP_SHUTTER_CONTROL"=107, "EXP_RS170"=108, "EXP_RS170_COMPLEX"=109, "EXP_HW_RS170_LUT"=110, "EXP_RS170_INTENSITY_SCALING"=111, "EXP_RS170_OFFSET"=112, "EXP_RS170_PAN"=113, "EXP_RS170_ZOOM2X"=114, "EXP_RS170_ZOOM4X"=115, "EXP_RS170_BINNING"=116, "EXP_RS170_DECIMATION"=117, "EXP_HW_ACCUM"=118, "EXP_SHT_PREOPEN"=119, "EXP_STORE_STROBE"=120, "EXP_CONT_CLNS"=121, "EXP_TIMING_MODE"=122, "EXP_EXT_TRIGGER"=123, "EXP_EVENT_COUNTER"=124, "EXP_SW_TRIGGER"=125, "EXP_KINETICS_WINDOWSIZE"=126, "EXP_EXPOSURE"=127, "EXP_CONTROLLER_NAME"=128, "EXP_CCD_CHIP_NAME"=129, "EXP_BSWBINNING"=297, "EXP_EDGEENHANCE"=130, "EXP_BOXVIDEOGAIN"=131, "EXP_HSHADING_VALUE"=132, "EXP_VSHADING_VALUE"=133, "EXP_EDGEENHANCE_FLAG"=134, "EXP_SHADING_FLAG"=135, "EXP_GRAYSCALE"=136, "EXP_OFFSET"=137, "EXP_CCDGAIN"=138, "EXP_TEMPERATURE"=139, "EXP_MCPVOLTAGE"=140, "EXP_BOXEXPOSURE"=141, "EXP_ABC_FLAG"=142, "EXP_GAMMA_FLAG"=143, "EXP_AUTOBLACK_FLAG"=144, "EXP_AGC_FLAG"=145, "EXP_ODD_FIELD"=146, "EXP_FIELD_SELECT"=147, "EXP_RESET"=148, "EXP_EXTERN_ENABLE"=149, "EXP_CONTROLLERS_SUPPORTED"=150, "EXP_VTCLK"=151, "EXP_HTCLK"=152, "EXP_GATE_VS_CW"=153, "EXP_COM_PORT"=154, "EXP_US_UNITS"=156, "EXP_MS_UNITS"=157, "EXP_SEC_UNITS"=158, "EXP_MIN_UNITS"=159, "EXP_HRS_UNITS"=160, "EXP_FRAME_UNITS"=161, "EXP_SYNC_ASYNC"=162, "EXP_FOCUS_NFRAME"=163, "EXP_TIMEOUT"=164, "EXP_TIMEOUT_DEFAULT"=165, "EXP_HW_AUTOSTOP"=166, "EXP_RS170_INTEN_OFFSET"=167, "EXP_CONTROLLER_ALIVE"=168, "EXP_FOCUS_TYPE"=169, "EXP_FOCUS_ZOOM"=170, "EXP_FOCUS_PAN"=171, "EXP_MULTI_TAP_ROI"=172, "EXP_USE_INTERUPTS"=173, "EXP_DATA_ACQ_STATE"=174, "EXP_VERIFY_GOOD_VALUES"=175, "EXP_WHITE_CLAMP"=176, "EXP_BLACK_CLAMP"=177, "EXP_DELAY_TIME"=178, "EXP_READOUT_TIME"=179, "EXP_SW_DIAG"=180, "EXP_DIAG1"=181, "EXP_DIAG2"=182, "EXP_DIAG3"=183, "EXP_DIAG4"=184, "EXP_DIAG5"=185, "EXP_AorB_GROUP"=186, "EXP_ABSORBANCE_FLAG"=187, "EXP_ABSORBANCE_METHOD"=188, "EXP_ABSORBANCE_STRIPNUM"=189, "EXP_DMASIZE_VIA_DRIVER"=190, "EXP_DRIVERVERSION"=191, "EXP_NUM_DEVICES"=192, "EXP_ECPDMA_CHANNEL"=193, "EXP_CUSTOM_SHUTTER"=194, "EXP_ADC_OFFSET"=195, "EXP_CURRENT_READOUT_MODE"=196, "EXP_BANK_ADD"=197, "EXP_LUT_BANK"=198, "EXP_SETUP_STATUS"=201, "EXP_XY_GROUPING"=239, "EXP_MESSAGES_FLAG"=240, "EXP_TTL_LINE_TO_WAIT"=253, "EXP_DATA_COLLECTION_MODE"=258, "EXP_DATA_COLLECTION_TYPE"=262, "EXP_SKIPFRAMES"=274, "EXP_CLR_INT_CNTR"=276, "EXP_ENABLE_INT_CNTR"=277, "EXP_INT_CNTR"=278, "EXP_INTERNAL_SYNC_SRC"=279, "EXP_SW_EXTSYNC"=280, "EXP_PTG_PRESENT"=281, "EXP_ELEC_SHT"=282, "EXP_BOARDS_WITH_NVRAM"=283, "EXP_ANLGMASTER_ST143"=284, "EXP_ANLGSLAVE_ST143"=285, "EXP_DISPLAY_ST143"=286, "EXP_INTRFACE_ST143"=287, "EXP_SCANCONTROL_ST143"=288, "EXP_NUMBERFRAMES_IRQ"=204, "EXP_COOL_TYPE"=214, "EXP_HD_TYPE"=215, "EXP_INTENSIFER_GAIN"=216, "EXP_SHT_GATE_MODE"=217, "EXP_HD_CHECK"=218, "EXP_AMP_MODE"=219, "EXP_AMP_DIALOG"=247, "EXP_ANALOG_GAIN"=220, "EXP_HW_FIXES"=221, "EXP_PCI_CARDS"=222, "EXP_NOT_REVERSE"=223, "EXP_LOAD_NVRAM_DEFAULTS"=234, "EXP_CNTR_BRD"=235, "EXP_XDIMHW"=237, "EXP_YDIMHW"=238, "EXP_SPECIAL_FAST_RDOUT"=254, "EXP_SPCL_FAST_Y_DIM"=255, "EXP_SPCL_FAST_X_DIM"=256, "EXP_SPCL_FAST_Y_INDEX"=257, "EXP_SHUTTER_COMP_TIME_MS"=266, "EXP_NVRAM_AVAIL"=267, "EXP_NUMBER_AGAIN_AVAIL"=269, "EXP_SENSOR_TYPE"=270, "EXP_EVENT_TYPE"=292, "EXP_ANTI_BLOOMING"=293, "EXP_FAST_PULSE_ENABLE"=233, "EXP_USE_HEADCALIB"=296, "EXP_TEMP_STATUS"=301, "EXP_MULTIPLE_READMODES_LIVE"=302, "EXP_FIRST_ACQUIRE_FLAG"=303, "EXP_ANTI_BLOOMING_CONTROL"=304, "EXP_PRE_HORZ_DELAY"=305, "EXP_NVRAM_TRIES"=306, "EXP_XASCEND"=307, "EXP_YASCEND"=308, "EXP_ALT_TIMING"=309, "EXP_SHUTTER_PRE_COMP"=310, "EXP_PVCAM_POSSIBLE"=311, "EXP_ADC_IN_NVRAM"=312, "EXP_PASSTHRU_MODE"=313, "EXP_FIRMWAREVERSION"=314, "EXP_IMMEDIATE_SHUTTER"=315, "EXP_STAGE2_TEMP"=316, "EXP_AVGAIN_ENABLED"=317, "EXP_AVGAIN_SETPOINT"=318, "EXP_AVGAIN"=319, "EXP_AVGAIN_CALIB_TEMP"=320, "EXP_AVGAIN_CALIB_COEFF1"=321, "EXP_AVGAIN_CALIB_COEFF2"=322, "EXP_AVGAIN_CALIB_COEFF3"=323, "EXP_AVGAIN_CALIB_COEFF4"=324, "EXP_AVGAIN_CALIB_COEFF5"=325, "EXP_FORCE_READOUT_MODE"=326, "EXP_RESET_DATACOLLECTION"=327, "EXP_ACTIVE_SUBFRAME"=328, "EXP_PV_READOUT_PORT"=514, "EXP_CLASSNAME"=775, "EXP_FLATFLDNAME"=776, "EXP_DARKNAME"=777, "EXP_SETUPNAME"=778, "EXP_ACCESSNAME"=779, "EXP_DATFILENAME"=780, "EXP_ABSORBFILENAME"=781, "EXP_BLEMISHFILENAME"=782, "EXP_COSMICFILENAME"=783, "EXP_FILEINCBASENAME"=784, "EXP_YTNAME"=785, "EXP_DEVNAME"=786, "EXP_USEROI"=787, "EXP_DOBLEMISH"=788, "EXP_DOABSORB"=789, "EXP_DOCOSMIC"=790, "EXP_COSMICSENS"=791, "EXP_ABSORBSTRIP"=792, "EXP_DATATYPE"=793, "EXP_OVERWRITECONFIRM"=794, "EXP_FILEINCENABLE"=795, "EXP_FILEINCCOUNT"=796, "EXP_RUNNING"=797, "EXP_SAVEROPT"=798, "EXP_TIME_UNITS"=799, "EXP_FILEACCESS"=800, "EXP_AUTOSAVE"=801, "EXP_NEWWINDOW"=802, "EXP_XDIM"=803, "EXP_YDIM"=804, "EXP_XDIMDET"=805, "EXP_YDIMDET"=806, "EXP_ROIMODE"=807, "EXP_NUMREPEATSEXP"=808, "EXP_NUMACCUMSEXP"=809, "EXP_THREADSTATE"=810, "EXP_USEMINTHRESHOLDING"=811, "EXP_MINTHRESHOLDVALUE"=812, "EXP_USEMAXTHRESHOLDING"=813, "EXP_MAXTHRESHOLDVALUE"=814, "EXP_RUNNING_EXPERIMENT"=815, "EXP_THRESHOLD_DEMAND_UPDATE"=816, "EXP_ROICOUNT"=817, "EXP_ACCUMS"=818, "EXP_CACCUMS"=819, "EXP_CSEQUENTS"=820, "EXP_PHOTON_ESTIMATION_ENABLE"=821, "EXP_PHOTON_MAXTIME"=822, "EXP_PHOTON_MAXTIMEUNIT"=823, "EXP_CUSTOMFILTER_ENABLE"=824, "EXP_CUSTOMFILTER_SIZE"=825, "EXP_LOOKUPTABLE_ENABLE"=826, "EXP_BSHOWWINDOW"=827, "EXP_BBACKSUBTRACT"=828, "EXP_BDOFLATFIELD"=829, "EXP_ASCIIOUTPUTFILE"=830, "EXP_ASCIIOUTPUT_DELIMITER"=831, "EXP_ASCIIOUTPUT_TERMINATOR"=832, "EXP_FFTYPE"=833, "EXP_BGTYPE"=834, "EXP_COSGRASS"=835, "EXP_RUNASCONFIRM"=836, "EXP_RUNASRUNACCESS"=837, "EXP_DATAFILETYPE"=838, "EXP_ROTATE"=839, "EXP_FLIP"=840, "EXP_REVERSE"=841, "EXP_SWBINNING"=842, "EXP_AUTOSTORE"=843, "EXP_XBINNED"=844, "EXP_YBINNED"=845, "EXP_NUMPATTERNS"=846, "EXP_EXPERIMENTTIME"=847, "EXP_ASYNCSEQUENTIALS"=848, "EXP_SEQUENTIALS"=849, "EXP_CSEQUENTIALS"=850, "EXP_AUTOD"=851, "EXP_EXPOSURETIME"=852, "EXP_EXPOSURETIME_UNITS"=853, "EXP_ACQMODE"=854, "EXP_DMASIZE_PVCAM"=855, "EXP_INITIALIZE"=856, "EXP_CELL_X_SIZE"=857, "EXP_CELL_Y_SIZE"=858, "EXP_X_GAP_SIZE"=859, "EXP_Y_GAP_SIZE"=860] ("Param")
                n346 = local read "OMA V exposure time"() -> (w554:dbl)
                n347 = local read "experiment reference"() -> (w552:refnum<k7>)
                n348 = invoke class="IExpSetup2" method="SetParam"(reference=w552, "Param"=w553, "pSetVal"=w554) -> (reference out=w549:refnum<k7>)  [unwired: 2 in, 4 out]
                n349 = local read "file reference"() -> (w551:refnum<k7>)
                n350 = invoke class="IExpSetup2" method="StartFocus"(reference=w549, "pFile"=w551) -> (reference out=w548:refnum<k7>, "pFile"=w550:refnum<k7>)  [unwired: 2 in, 2 out]
                n351 = while {
                  shift-right: [w563] -> _
                  shift-left: w550 -> [w560]
                  tunnel: w548 -> [w558]
                  i -> [w566]
                  stop <- w561 stop-if-true
                  n352 = flat-sequence {
                    tunnel: [w569] -> w562
                    tunnel: w560 -> [w568]
                    tunnel: [w568] -> w559
                    tunnel: w558 -> [w567]
                    tunnel: [w567] -> w555
                    tunnel: w562 -> [w575]
                    tunnel: [w574] -> w556
                    tunnel: w555 -> [w574]
                    tunnel: [w577] -> w561
                    tunnel: [w576] -> w557
                    tunnel: w556 -> [w576]
                    frame #0 {
                      n353 = local read "time start (ms)"() -> (w571:i32)
                      n354 = Tick Count (ms)() -> (millisecond timer value=w569:u32)
                      n355 = Subtract(x=w569, y=w571) -> (x-y=w572:u32)
                      n356 = Divide(x=w572, y=u32 1000) -> (x/y=w573:dbl)
                      n357 = local write "time elapsed (s)"(w573) -> ()
                    }
                    frame #1 {
                      n358 = local write "time start (ms)"(w575) -> ()
                    }
                    frame #2 {
                      n359 = local read "OMA V exposure time"() -> (w580:dbl)
                      n360 = Multiply(x=w580, y=1000) -> (x*y=w579:dbl)
                      n361 = local read "Stop measurement"() -> (w577:bool)
                      n362 = Wait (ms)(milliseconds to wait=w579) -> ()  [unwired: 1 out]
                    }
                  }
                  n363 = Not(x=w561) -> (.not. x?=w564:bool)
                  n364 = Equal To 0?(x=w566) -> (x = 0?=w565:bool)
                  n365 = case shown="True" w564 {
                    tunnel: [w582 w583] -> w563
                    tunnel: w565 -> [_ w593]
                    tunnel: w559 -> [w582 w588]
                    tunnel: w557 -> [w581 _]
                    frame False {
                      n366 = invoke class="IExpSetup2" method="Stop"(reference=w581) -> ()  [unwired: 2 in, 3 out]
                    }
                    frame True {
                      n367 = local read "FrameVariant"() -> (w591:variant)
                      n368 = invoke class="IDocFile" method="GetFrame"(reference=w588, "frame"=i16 1, "FrameVariant"=w591) -> (reference out=w583:refnum<k7>, "FrameVariant"=w589:variant)  [unwired: 2 in, 3 out]
                      n369 = local read "frame array"() -> (w592:i32[][])
                      n370 = Variant To Data(type=w592, Variant=w589) -> (data=w596:i32[][])  [unwired: 1 in, 1 out]
                      n371 = Index Array(array=w596, index (col)=0 ("disabled index (col)")) -> (element=w594:i32[])  [unwired: 1 in]
                      n372 = case shown="True" w593 {
                        tunnel: w583 -> [_ w602]
                        tunnel: w594 -> [w597 w598]
                        tunnel: [w597 w598] -> w585
                        frame False {
                        }
                        frame True {
                          n373 = invoke class="IDocFile" method="GetCalibration"(reference=w602) -> ("GetCalibration"=w604:refnum<k7>)  [unwired: 2 in, 2 out]
                          n374 = Array Size(array=w598) -> (size(s)=w599:i32)
                          n375 = property class="ICalibObj"(reference=w604) -> (reference out=w600:refnum<k7>, "PairCount"=w605:u8)  [unwired: 1 in, 1 out]
                          n376 = for {
                            N: w605 -> [_]
                            tunnel: w600 -> [w622]
                            tunnel: [w623] -> w607 mode=indexing
                            tunnel: [w620] -> w606 mode=indexing
                            i -> [w621]
                            n377 = invoke class="ICalibObj" method="CalibVal"(reference=w622, "index"=w621) -> ("CalibVal"=w623:dbl)  [unwired: 2 in, 3 out]
                            n378 = invoke class="ICalibObj" method="PixelLoc"(reference=w622, "index"=w621) -> ("PixelLoc"=w620:dbl)  [unwired: 2 in, 3 out]
                          }
                          n379 = for {
                            N: w599 -> [_]
                            tunnel: w607 -> [w619]
                            tunnel: [w618] -> w601 mode=indexing
                            tunnel: [w617] -> _ mode=indexing
                            tunnel: w606 -> [w616]
                            tunnel: 1 ("index") -> [w608]
                            i -> [w615]
                            n380 = Divide(x=w608, y=2) -> (x/y=w612:dbl)
                            n381 = Round To Nearest(number=w612) -> (nearest integer value=w610:dbl)
                            n382 = Multiply(x=w615, y=w608) -> (x*y=w611:i32)
                            n383 = Increment(x=w610) -> (x+1=w609:dbl)
                            n384 = Add(x=w611, y=w609) -> (x+y=w614:dbl)
                            n385 = call <vilib>:"Polynomial Interpolation.vi"("x value"=w614, "X"=w616, "Y"=w619) -> ("interpolation error"=w617:dbl, "interpolation value"=w618:dbl)  [unwired: 1 out]
                          }
                          n386 = local write "Wavelength Scale"(w601) -> ()
                        }
                      }
                      n387 = local read "Wavelength Scale"() -> (w584:dbl[])
                      n388 = Add Array Elements(numeric array=w585) -> (sum=w587:i32)
                      n389 = Bundle("Wavelength Scale"=w584, "frame array"=w585) -> (w586:T3)  [unwired: 1 in]
                      n390 = local write "Time Trace"(w587) -> ()
                      n391 = local write "Intensity Sum"(w587) -> ()
                      n392 = local write "XY Graph Spectrum"(w586) -> ()
                    }
                  }
                }
              }
              frame #2 {
                w624 = FALSE ("Stop measurement")
                n393 = local write "busy"(FALSE ("busy")) -> ()
                n394 = local write "Stop measurement"(w624) -> ()
                n395 = local write "Start Continuous"(w624) -> ()
              }
            }
          }
          frame 15 {
            w630 = 127 items=["EXP_ETACTUAL"=1, "EXP_SEQUENTS"=2, "EXP_ERROR"=3, "EXP_GETCAPS"=4, "EXP_GETPLSR"=5, "EXP_DETECTOR_BIT"=16, "EXP_RUNNING_APP"=23, "EXP_VIDEO_TYPE"=24, "EXP_CUSTOM_VIDEO_X"=25, "EXP_CUSTOM_VIDEO_Y"=26, "EXP_CUSTOM_VIDEO_FSTWIDTH"=27, "EXP_CUSTOM_VIDEO_LSTWIDTH"=28, "EXP_VIDEO_XDIM"=29, "EXP_VIDEO_YDIM"=30, "EXP_VIDEO_MAX_ZOOM"=31, "EXP_VIDEO_HORZ_PAN"=32, "EXP_VIDEO_VERT_PAN"=33, "EXP_WORD_MULTIPLIER"=34, "EXP_TARGET_ID"=35, "EXP_ADAPTER_ID"=36, "EXP_NUMADAPTORS"=37, "EXP_FORCE_PP_INIT"=38, "EXP_NOP_ADC"=39, "EXP_ACTUAL_TEMP"=40, "EXP_FORCE_AUTOSTOP"=41, "EXP_DEFAULT_VTCLK"=42, "EXP_MIN_VTCLK"=43, "EXP_MAX_VTCLK"=44, "EXP_DEFAULT_HTCLK"=45, "EXP_MIN_HTCLK"=46, "EXP_MAX_HTCLK"=47, "EXP_TIMING_STYLE"=48, "EXP_HEADSELECT"=49, "EXP_HORZPHASE"=50, "EXP_VERTPHASE"=51, "EXP_SPECIAL_SPEED"=52, "EXP_PRE_STRIPS"=53, "EXP_POST_STRIPS"=54, "EXP_PRE_LINES"=55, "EXP_POST_LINES"=56, "EXP_ACTIVE_LINES"=57, "EXP_ACTIVE_STRIPS"=58, "EXP_XFER_EXTRA"=59, "EXP_MIN_BLOCK"=60, "EXP_NUM_MIN_BLOCK"=61, "EXP_LOGIC_OUTPUT"=66, "EXP_VIDEO_BLANK"=67, "EXP_ZOOM_MODE_VIDEO"=68, "EXP_LEVEL_SYNC"=69, "EXP_DISABLE_LASER"=70, "EXP_ACQBACK_SHUTTER"=71, "EXP_ACQFLAT_SHUTTER"=72, "EXP_SMALL_CCD_MINEXP"=73, "EXP_LARGE_CCD_MINEXP"=74, "EXP_GATING_MODE"=75, "EXP_ILME_B1X"=76, "EXP_ILME_B2X"=77, "EXP_ILME_D1X"=78, "EXP_ILME_D2X"=79, "EXP_ILME_D4X"=80, "EXP_INIT_HW_ACCUM"=81, "EXP_5X_GAIN_ENABLE"=82, "EXP_RET_SRCCMP"=83, "EXP_EVENT_HANDLE"=84, "EXP_READOUT_MODE"=85, "EXP_SHUTTER_TYPE"=86, "EXP_USER_DEFINED_CHIP"=87, "EXP_USER_DEFINED_TIMING"=88, "EXP_CONTROLLER_VERSION"=89, "EXP_GET_CONTROLLER_VER"=90, "EXP_TTL_LINES"=91, "EXP_BIT_ADJUST"=92, "EXP_RESOLUTION"=93, "EXP_GAIN"=94, "EXP_ADC_RATE"=95, "EXP_ADC_TYPE"=96, "EXP_NUMBER_OF_CLEANS"=97, "EXP_NUM_OF_STRIPS_PER_CLN"=98, "EXP_INTERFACE_CARD"=99, "EXP_INTERRUPT"=100, "EXP_IO_ADDRESS1"=101, "EXP_IO_ADDRESS2"=102, "EXP_IO_ADDRESS3"=103, "EXP_HW_ROI"=104, "EXP_HW_BINNING"=105, "EXP_EDGE_TRIGGER"=106, "EXP_SHUTTER_CONTROL"=107, "EXP_RS170"=108, "EXP_RS170_COMPLEX"=109, "EXP_HW_RS170_LUT"=110, "EXP_RS170_INTENSITY_SCALING"=111, "EXP_RS170_OFFSET"=112, "EXP_RS170_PAN"=113, "EXP_RS170_ZOOM2X"=114, "EXP_RS170_ZOOM4X"=115, "EXP_RS170_BINNING"=116, "EXP_RS170_DECIMATION"=117, "EXP_HW_ACCUM"=118, "EXP_SHT_PREOPEN"=119, "EXP_STORE_STROBE"=120, "EXP_CONT_CLNS"=121, "EXP_TIMING_MODE"=122, "EXP_EXT_TRIGGER"=123, "EXP_EVENT_COUNTER"=124, "EXP_SW_TRIGGER"=125, "EXP_KINETICS_WINDOWSIZE"=126, "EXP_EXPOSURE"=127, "EXP_CONTROLLER_NAME"=128, "EXP_CCD_CHIP_NAME"=129, "EXP_BSWBINNING"=297, "EXP_EDGEENHANCE"=130, "EXP_BOXVIDEOGAIN"=131, "EXP_HSHADING_VALUE"=132, "EXP_VSHADING_VALUE"=133, "EXP_EDGEENHANCE_FLAG"=134, "EXP_SHADING_FLAG"=135, "EXP_GRAYSCALE"=136, "EXP_OFFSET"=137, "EXP_CCDGAIN"=138, "EXP_TEMPERATURE"=139, "EXP_MCPVOLTAGE"=140, "EXP_BOXEXPOSURE"=141, "EXP_ABC_FLAG"=142, "EXP_GAMMA_FLAG"=143, "EXP_AUTOBLACK_FLAG"=144, "EXP_AGC_FLAG"=145, "EXP_ODD_FIELD"=146, "EXP_FIELD_SELECT"=147, "EXP_RESET"=148, "EXP_EXTERN_ENABLE"=149, "EXP_CONTROLLERS_SUPPORTED"=150, "EXP_VTCLK"=151, "EXP_HTCLK"=152, "EXP_GATE_VS_CW"=153, "EXP_COM_PORT"=154, "EXP_US_UNITS"=156, "EXP_MS_UNITS"=157, "EXP_SEC_UNITS"=158, "EXP_MIN_UNITS"=159, "EXP_HRS_UNITS"=160, "EXP_FRAME_UNITS"=161, "EXP_SYNC_ASYNC"=162, "EXP_FOCUS_NFRAME"=163, "EXP_TIMEOUT"=164, "EXP_TIMEOUT_DEFAULT"=165, "EXP_HW_AUTOSTOP"=166, "EXP_RS170_INTEN_OFFSET"=167, "EXP_CONTROLLER_ALIVE"=168, "EXP_FOCUS_TYPE"=169, "EXP_FOCUS_ZOOM"=170, "EXP_FOCUS_PAN"=171, "EXP_MULTI_TAP_ROI"=172, "EXP_USE_INTERUPTS"=173, "EXP_DATA_ACQ_STATE"=174, "EXP_VERIFY_GOOD_VALUES"=175, "EXP_WHITE_CLAMP"=176, "EXP_BLACK_CLAMP"=177, "EXP_DELAY_TIME"=178, "EXP_READOUT_TIME"=179, "EXP_SW_DIAG"=180, "EXP_DIAG1"=181, "EXP_DIAG2"=182, "EXP_DIAG3"=183, "EXP_DIAG4"=184, "EXP_DIAG5"=185, "EXP_AorB_GROUP"=186, "EXP_ABSORBANCE_FLAG"=187, "EXP_ABSORBANCE_METHOD"=188, "EXP_ABSORBANCE_STRIPNUM"=189, "EXP_DMASIZE_VIA_DRIVER"=190, "EXP_DRIVERVERSION"=191, "EXP_NUM_DEVICES"=192, "EXP_ECPDMA_CHANNEL"=193, "EXP_CUSTOM_SHUTTER"=194, "EXP_ADC_OFFSET"=195, "EXP_CURRENT_READOUT_MODE"=196, "EXP_BANK_ADD"=197, "EXP_LUT_BANK"=198, "EXP_SETUP_STATUS"=201, "EXP_XY_GROUPING"=239, "EXP_MESSAGES_FLAG"=240, "EXP_TTL_LINE_TO_WAIT"=253, "EXP_DATA_COLLECTION_MODE"=258, "EXP_DATA_COLLECTION_TYPE"=262, "EXP_SKIPFRAMES"=274, "EXP_CLR_INT_CNTR"=276, "EXP_ENABLE_INT_CNTR"=277, "EXP_INT_CNTR"=278, "EXP_INTERNAL_SYNC_SRC"=279, "EXP_SW_EXTSYNC"=280, "EXP_PTG_PRESENT"=281, "EXP_ELEC_SHT"=282, "EXP_BOARDS_WITH_NVRAM"=283, "EXP_ANLGMASTER_ST143"=284, "EXP_ANLGSLAVE_ST143"=285, "EXP_DISPLAY_ST143"=286, "EXP_INTRFACE_ST143"=287, "EXP_SCANCONTROL_ST143"=288, "EXP_NUMBERFRAMES_IRQ"=204, "EXP_COOL_TYPE"=214, "EXP_HD_TYPE"=215, "EXP_INTENSIFER_GAIN"=216, "EXP_SHT_GATE_MODE"=217, "EXP_HD_CHECK"=218, "EXP_AMP_MODE"=219, "EXP_AMP_DIALOG"=247, "EXP_ANALOG_GAIN"=220, "EXP_HW_FIXES"=221, "EXP_PCI_CARDS"=222, "EXP_NOT_REVERSE"=223, "EXP_LOAD_NVRAM_DEFAULTS"=234, "EXP_CNTR_BRD"=235, "EXP_XDIMHW"=237, "EXP_YDIMHW"=238, "EXP_SPECIAL_FAST_RDOUT"=254, "EXP_SPCL_FAST_Y_DIM"=255, "EXP_SPCL_FAST_X_DIM"=256, "EXP_SPCL_FAST_Y_INDEX"=257, "EXP_SHUTTER_COMP_TIME_MS"=266, "EXP_NVRAM_AVAIL"=267, "EXP_NUMBER_AGAIN_AVAIL"=269, "EXP_SENSOR_TYPE"=270, "EXP_EVENT_TYPE"=292, "EXP_ANTI_BLOOMING"=293, "EXP_FAST_PULSE_ENABLE"=233, "EXP_USE_HEADCALIB"=296, "EXP_TEMP_STATUS"=301, "EXP_MULTIPLE_READMODES_LIVE"=302, "EXP_FIRST_ACQUIRE_FLAG"=303, "EXP_ANTI_BLOOMING_CONTROL"=304, "EXP_PRE_HORZ_DELAY"=305, "EXP_NVRAM_TRIES"=306, "EXP_XASCEND"=307, "EXP_YASCEND"=308, "EXP_ALT_TIMING"=309, "EXP_SHUTTER_PRE_COMP"=310, "EXP_PVCAM_POSSIBLE"=311, "EXP_ADC_IN_NVRAM"=312, "EXP_PASSTHRU_MODE"=313, "EXP_FIRMWAREVERSION"=314, "EXP_IMMEDIATE_SHUTTER"=315, "EXP_STAGE2_TEMP"=316, "EXP_AVGAIN_ENABLED"=317, "EXP_AVGAIN_SETPOINT"=318, "EXP_AVGAIN"=319, "EXP_AVGAIN_CALIB_TEMP"=320, "EXP_AVGAIN_CALIB_COEFF1"=321, "EXP_AVGAIN_CALIB_COEFF2"=322, "EXP_AVGAIN_CALIB_COEFF3"=323, "EXP_AVGAIN_CALIB_COEFF4"=324, "EXP_AVGAIN_CALIB_COEFF5"=325, "EXP_FORCE_READOUT_MODE"=326, "EXP_RESET_DATACOLLECTION"=327, "EXP_ACTIVE_SUBFRAME"=328, "EXP_PV_READOUT_PORT"=514, "EXP_CLASSNAME"=775, "EXP_FLATFLDNAME"=776, "EXP_DARKNAME"=777, "EXP_SETUPNAME"=778, "EXP_ACCESSNAME"=779, "EXP_DATFILENAME"=780, "EXP_ABSORBFILENAME"=781, "EXP_BLEMISHFILENAME"=782, "EXP_COSMICFILENAME"=783, "EXP_FILEINCBASENAME"=784, "EXP_YTNAME"=785, "EXP_DEVNAME"=786, "EXP_USEROI"=787, "EXP_DOBLEMISH"=788, "EXP_DOABSORB"=789, "EXP_DOCOSMIC"=790, "EXP_COSMICSENS"=791, "EXP_ABSORBSTRIP"=792, "EXP_DATATYPE"=793, "EXP_OVERWRITECONFIRM"=794, "EXP_FILEINCENABLE"=795, "EXP_FILEINCCOUNT"=796, "EXP_RUNNING"=797, "EXP_SAVEROPT"=798, "EXP_TIME_UNITS"=799, "EXP_FILEACCESS"=800, "EXP_AUTOSAVE"=801, "EXP_NEWWINDOW"=802, "EXP_XDIM"=803, "EXP_YDIM"=804, "EXP_XDIMDET"=805, "EXP_YDIMDET"=806, "EXP_ROIMODE"=807, "EXP_NUMREPEATSEXP"=808, "EXP_NUMACCUMSEXP"=809, "EXP_THREADSTATE"=810, "EXP_USEMINTHRESHOLDING"=811, "EXP_MINTHRESHOLDVALUE"=812, "EXP_USEMAXTHRESHOLDING"=813, "EXP_MAXTHRESHOLDVALUE"=814, "EXP_RUNNING_EXPERIMENT"=815, "EXP_THRESHOLD_DEMAND_UPDATE"=816, "EXP_ROICOUNT"=817, "EXP_ACCUMS"=818, "EXP_CACCUMS"=819, "EXP_CSEQUENTS"=820, "EXP_PHOTON_ESTIMATION_ENABLE"=821, "EXP_PHOTON_MAXTIME"=822, "EXP_PHOTON_MAXTIMEUNIT"=823, "EXP_CUSTOMFILTER_ENABLE"=824, "EXP_CUSTOMFILTER_SIZE"=825, "EXP_LOOKUPTABLE_ENABLE"=826, "EXP_BSHOWWINDOW"=827, "EXP_BBACKSUBTRACT"=828, "EXP_BDOFLATFIELD"=829, "EXP_ASCIIOUTPUTFILE"=830, "EXP_ASCIIOUTPUT_DELIMITER"=831, "EXP_ASCIIOUTPUT_TERMINATOR"=832, "EXP_FFTYPE"=833, "EXP_BGTYPE"=834, "EXP_COSGRASS"=835, "EXP_RUNASCONFIRM"=836, "EXP_RUNASRUNACCESS"=837, "EXP_DATAFILETYPE"=838, "EXP_ROTATE"=839, "EXP_FLIP"=840, "EXP_REVERSE"=841, "EXP_SWBINNING"=842, "EXP_AUTOSTORE"=843, "EXP_XBINNED"=844, "EXP_YBINNED"=845, "EXP_NUMPATTERNS"=846, "EXP_EXPERIMENTTIME"=847, "EXP_ASYNCSEQUENTIALS"=848, "EXP_SEQUENTIALS"=849, "EXP_CSEQUENTIALS"=850, "EXP_AUTOD"=851, "EXP_EXPOSURETIME"=852, "EXP_EXPOSURETIME_UNITS"=853, "EXP_ACQMODE"=854, "EXP_DMASIZE_PVCAM"=855, "EXP_INITIALIZE"=856, "EXP_CELL_X_SIZE"=857, "EXP_CELL_Y_SIZE"=858, "EXP_X_GAP_SIZE"=859, "EXP_Y_GAP_SIZE"=860] ("Param")
            # "start streaming data fast"
            n396 = local read "error reader"() -> (w637:errorcluster)
            n397 = local read "OMA V exposure time"() -> (w632:dbl)
            n398 = local read "experiment reference"() -> (w631:refnum<k7>)
            n399 = invoke class="IExpSetup2" method="SetParam"(reference=w631, "Param"=w630, "pSetVal"=w632) -> (reference out=w628:refnum<k7>)  [unwired: 2 in, 4 out]
            n400 = local read "file reference"() -> (w629:refnum<k7>)
            n401 = local read "reader endpoint"() -> (w638:refnum<k21>)
            n402 = local read "writer endpoint"() -> (w640:refnum<k21>)
            n403 = invoke class="IExpSetup2" method="StartFocus"(reference=w628, "pFile"=w629) -> (reference out=w627:refnum<k7>, "pFile"=w626:refnum<k7>)  [unwired: 2 in, 2 out]
            n404 = local read "error writer"() -> (w639:errorcluster)
            n405 = while {
              shift-right: [w659] -> w636
              shift-left: w640 -> [w665]
              shift-right: [w658] -> w635
              shift-left: w639 -> [w664]
              shift-right: [w661] -> w634
              shift-left: w638 -> [w663]
              shift-right: [w660] -> w633
              shift-left: w637 -> [w662]
              tunnel: w627 -> [w656]
              shift-right: [w655] -> _
              shift-left: w626 -> [w657]
              i -> [w654]
              stop <- w666 stop-if-true
              n406 = flat-sequence {
                tunnel: w662 -> [w671]
                tunnel: w663 -> [w672]
                tunnel: w664 -> [w673]
                tunnel: w665 -> [w674]
                tunnel: [w674] -> w653
                tunnel: [w673] -> w652
                tunnel: [w672] -> w651
                tunnel: [w671] -> w650
                tunnel: [w684] -> w669
                tunnel: [w683] -> w668
                tunnel: [w675] -> w667
                tunnel: [w680] -> w661
                tunnel: [w679] -> w660
                tunnel: w653 -> [w684]
                tunnel: w652 -> [w683]
                tunnel: w651 -> [w682]
                tunnel: w650 -> [w681]
                tunnel: w669 -> [w701]
                tunnel: w668 -> [w700]
                tunnel: w667 -> [w697]
                tunnel: w657 -> [w696]
                tunnel: w656 -> [w695]
                tunnel: w654 -> [w693]
                tunnel: [w697] -> w649
                tunnel: [w699] -> w648
                tunnel: [w698] -> w647
                tunnel: [w694] -> w646
                tunnel: [w786] -> w655
                tunnel: [w787] -> w658
                tunnel: [w788] -> w659
                tunnel: [w789] -> w666
                tunnel: w649 -> [w789]
                tunnel: w648 -> [w788]
                tunnel: w647 -> [w787]
                tunnel: w646 -> [w786]
                frame #0 {
                  n407 = Tick Count (ms)() -> (millisecond timer value=w670:u32)
                  n408 = local write "time start (ms)"(w670) -> ()
                }
                frame #1 {
                  # "experiment ready to acquire?"
                  n409 = while {
                    tunnel: [w686] -> w678
                    tunnel: [w687] -> w677
                    shift-right: [w689] -> w680
                    shift-left: w682 -> [w691]
                    shift-right: [w688] -> w679
                    shift-left: w681 -> [w690]
                    stop <- w685 continue-if-true
                    n410 = local read "standby stream"() -> (w686:bool)
                    n411 = shared-variable-read(w691, w690, 1000 ("timeout ms (-1)")) -> (w689:refnum<k21>, w688:errorcluster, w687:bool)  [unwired: 1 out]
                    n412 = And(x=w687, y=w686) -> (x .and. y?=w685:bool)
                  }
                  n413 = Not(x=w678) -> (.not. x?=w676:bool)
                  n414 = And(x=w677, y=w676) -> (x .and. y?=w675:bool)
                }
                frame #2 {
                  n415 = case shown="False" w697 {
                    tunnel: [w717 w779] -> w698
                    tunnel: [w716 w780] -> w699
                    tunnel: w700 -> [w715 w779]
                    tunnel: w701 -> [w714 w780]
                    tunnel: w696 -> [w711 w778]
                    tunnel: w695 -> [w710 w777]
                    tunnel: [w709 w778] -> w694
                    tunnel: w693 -> [w707 _]
                    frame False {
                      # "acquire"
                      n416 = flat-sequence {
                        tunnel: w707 -> [w721]
                        tunnel: w710 -> [w722]
                        tunnel: w711 -> [w723]
                        tunnel: w714 -> [w724]
                        tunnel: w715 -> [w725]
                        tunnel: [w725] -> w706
                        tunnel: [w724] -> w705
                        tunnel: [w723] -> w704
                        tunnel: [w722] -> w703
                        tunnel: [w721] -> w702
                        tunnel: [w742] -> w713
                        tunnel: [w741] -> w712
                        tunnel: [w731] -> w709
                        tunnel: [w730] -> w708
                        tunnel: w706 -> [w742]
                        tunnel: w705 -> [w741]
                        tunnel: w704 -> [w726]
                        tunnel: w703 -> [_]
                        tunnel: w702 -> [w729]
                        tunnel: [w774] -> w717
                        tunnel: [w773] -> w716
                        tunnel: w713 -> [w772]
                        tunnel: w712 -> [w771]
                        tunnel: w708 -> [w770]
                        frame #0 {
                          n417 = local read "OMA V exposure time"() -> (w720:dbl)
                          n418 = Multiply(x=w720, y=1000) -> (x*y=w719:dbl)
                          n419 = Wait (ms)(milliseconds to wait=w719) -> ()  [unwired: 1 out]
                        }
                        frame #1 {
                          n420 = Equal To 0?(x=w729) -> (x = 0?=w728:bool)
                          n421 = local read "FrameVariant"() -> (w736:variant)
                          n422 = local read "frame array"() -> (w727:i32[][])
                          n423 = invoke class="IDocFile" method="GetFrame"(reference=w726, "frame"=i16 1, "FrameVariant"=w736) -> (reference out=w731:refnum<k7>, "FrameVariant"=w734:variant)  [unwired: 2 in, 3 out]
                          n424 = Variant To Data(type=w727, Variant=w734) -> (data=w735:i32[][])  [unwired: 1 in, 1 out]
                          n425 = Index Array(array=w735, index (col)=0 ("disabled index (col)")) -> (element=w738:i32[])  [unwired: 1 in]
                          n426 = case shown="True" w728 {
                            tunnel: w731 -> [_ w748]
                            tunnel: w738 -> [w743 w744]
                            tunnel: [w743 w744] -> w739
                            frame False {
                            }
                            frame True {
                              n427 = invoke class="IDocFile" method="GetCalibration"(reference=w748) -> ("GetCalibration"=w750:refnum<k7>)  [unwired: 2 in, 2 out]
                              n428 = Array Size(array=w744) -> (size(s)=w745:i32)
                              n429 = property class="ICalibObj"(reference=w750) -> (reference out=w746:refnum<k7>, "PairCount"=w751:u8)  [unwired: 1 in, 1 out]
                              n430 = for {
                                N: w751 -> [_]
                                tunnel: w746 -> [w768]
                                tunnel: [w769] -> w753 mode=indexing
                                tunnel: [w766] -> w752 mode=indexing
                                i -> [w767]
                                n431 = invoke class="ICalibObj" method="CalibVal"(reference=w768, "index"=w767) -> ("CalibVal"=w769:dbl)  [unwired: 2 in, 3 out]
                                n432 = invoke class="ICalibObj" method="PixelLoc"(reference=w768, "index"=w767) -> ("PixelLoc"=w766:dbl)  [unwired: 2 in, 3 out]
                              }
                              n433 = for {
                                N: w745 -> [_]
                                tunnel: w753 -> [w765]
                                tunnel: [w764] -> w747 mode=indexing
                                tunnel: [w763] -> _ mode=indexing
                                tunnel: w752 -> [w762]
                                tunnel: 1 ("index") -> [w754]
                                i -> [w761]
                                n434 = Divide(x=w754, y=2) -> (x/y=w758:dbl)
                                n435 = Round To Nearest(number=w758) -> (nearest integer value=w756:dbl)
                                n436 = Multiply(x=w761, y=w754) -> (x*y=w757:i32)
                                n437 = Increment(x=w756) -> (x+1=w755:dbl)
                                n438 = Add(x=w757, y=w755) -> (x+y=w760:dbl)
                                n439 = call <vilib>:"Polynomial Interpolation.vi"("x value"=w760, "X"=w762, "Y"=w765) -> ("interpolation error"=w763:dbl, "interpolation value"=w764:dbl)  [unwired: 1 out]
                              }
                              n440 = local write "Wavelength Scale"(w747) -> ()
                            }
                          }
                          n441 = local read "Wavelength Scale"() -> (w737:dbl[])
                          n442 = Add Array Elements(numeric array=w739) -> (sum=w740:i32)
                          n443 = Bundle("Wavelength Scale"=w737, "frame array"=w739) -> (w730:T3)  [unwired: 1 in]
                          n444 = local write "XY Graph Spectrum"(w730) -> ()
                          n445 = local write "Time Trace"(w740) -> ()
                          n446 = local write "Intensity Sum"(w740) -> ()
                        }
                        frame #2 {
                          # "send data"
                          n447 = shared-variable-write(w771, w772, w770) -> (w775:refnum<k21>, w776:errorcluster)  [unwired: 1 in, 1 out]
                          n448 = Flush Stream(8:w776, 11:w775) -> (0:w774:errorcluster, 3:w773:refnum<k21>)  [unwired: 2 in, 1 out]
                        }
                      }
                    }
                    frame True {
                      n449 = invoke class="IExpSetup2" method="Stop"(reference=w777) -> ()  [unwired: 2 in, 3 out]
                    }
                  }
                }
                frame #3 {
                  n450 = local read "time start (ms)"() -> (w784:i32)
                  n451 = Tick Count (ms)() -> (millisecond timer value=w785:u32)
                  n452 = Subtract(x=w785, y=w784) -> (x-y=w783:u32)
                  n453 = Divide(x=w783, y=u32 1000) -> (x/y=w782:dbl)
                  n454 = local write "time elapsed (s)"(w782) -> ()
                }
              }
            }
            n455 = flat-sequence {
              tunnel: w636 -> [w644]
              tunnel: w635 -> [w643]
              tunnel: w634 -> [w642]
              tunnel: w633 -> [w641]
              frame #0 {
                n456 = local write "writer endpoint"(w644) -> ()
                n457 = local write "error writer"(w643) -> ()
                n458 = local write "error reader"(w641) -> ()
                n459 = local write "reader endpoint"(w642) -> ()
              }
              frame #1 {
                w645 = FALSE ("busy")
                n460 = local write "busy"(w645) -> ()
                n461 = local write "Start Stream"(w645) -> ()
              }
            }
          }
          frame 16 {
            n462 = local read "Wavelength Step (nm)"() -> (w808:dbl)
            n463 = local read "Wavelength End (nm)"() -> (w811:dbl)
            n464 = local read "Wavelength Start (nm)"() -> (w812:dbl)
            n465 = Subtract(x=w812, y=w811) -> (x-y=w809:dbl)
            n466 = Divide(x=w809, y=w808) -> (x/y=w810:dbl)
            n467 = Absolute Value(x=w810) -> (abs(x)=w806:dbl)
            n468 = Round To Nearest(number=w806) -> (nearest integer value=w807:dbl)
            n469 = Increment(x=w807) -> (x+1=w805:dbl)
            n470 = call "subVI_RampGenerator.vi"("Number of Positions"=w805, "End  (um)"=w811, "Start  (um)"=w812) -> ("Array"=w802:dbl[])  [unwired: 1 in]
            n471 = flat-sequence {
              tunnel: w805 -> [w821]
              tunnel: [w821] -> w804
              tunnel: [w816] -> w800
              tunnel: [w815] -> w798
              tunnel: [w814] -> w792
              tunnel: [w813] -> w790
              tunnel: w804 -> [w827]
              tunnel: [w827] -> w803
              tunnel: [w825] -> w801
              tunnel: w800 -> [w825]
              tunnel: [w824] -> w799
              tunnel: w798 -> [w824]
              tunnel: [w823] -> w793
              tunnel: w792 -> [w823]
              tunnel: [w822] -> w791
              tunnel: w790 -> [w822]
              tunnel: w803 -> [w828]
              tunnel: w802 -> [w837]
              tunnel: w801 -> [w836]
              tunnel: w799 -> [w835]
              tunnel: [w834] -> w797
              tunnel: [w833] -> w796
              tunnel: [w832] -> w795
              tunnel: [w831] -> w794
              tunnel: w793 -> [w830]
              tunnel: w791 -> [w829]
              tunnel: w797 -> [w921]
              tunnel: w796 -> [w920]
              tunnel: w795 -> [w919]
              tunnel: w794 -> [w918]
              frame #0 {
                w817 = 87 items=["SPT_NOCMD", "SPT_SPECTS_SUPPORTED", "SPT_TYPE", "SPT_CALIBUPDATE", "SPT_GRATINGWARNING", "SPT_LASERWARNING", "SPT_FORCEMOVE", "SPT_INSTNAME", "SPT_USERNAME", "SPT_INSTUSERNAME", "SPT_INSTCOMMNAME", "SPT_WAVE_ORIENTED", "SPT_NUMSTAGES", "SPT_GRATINGSPERTURRET", "SPT_CURRGRATING", "SPT_GRAT_BACKLASH_REQ", "SPT_GRATINGBACKLASHSTEPS", "SPT_NEEDINIT", "SPT_NEED_HWINIT", "SPT_MOTOR", "SPT_ARRAYSIZE", "SPT_ROI_CENTER", "SPT_ORDER", "SPT_CUR_GRATING", "SPT_NEW_GRATING", "SPT_SEQUENCER_STATE", "SPT_NUMTURRETS", "SPT_CURRTURRET", "SPT_DO_RESET", "SPT_SLAVE_CNT", "SPT_NUM_STEPS", "SPT_PIXEL_WIDTH", "SPT_GRAT_USERNAME", "SPT_GRAT_GROOVES", "SPT_GRAT_CENTERADJ", "SPT_GRAT_LINEAR_ADJ", "SPT_GRAT_SLOPE_ADJ", "SPT_GRAT_FOCAL_LEN", "SPT_GRAT_INCL_ANGLE", "SPT_GRAT_DETECT_ANGLE", "SPT_GRAT_MAG", "SPT_ACCESS_ALL_GRAT_SPEEDS", "SPT_SPEED_FOR_EACH_GRATING", "SPT_NUM_SETABLE_GRAT_SPEEDS", "SPT_GRATING_SPEED", "SPT_GRATING_SPEED_MIN", "SPT_GRATING_SPEED_MAX", "SPT_GRAT_REF_GRATING", "SPT_GRAT_STEPSPUNIT", "SPT_GRAT_OFFSET", "SPT_GRAT_ADJUST", "SPT_GRAT_LO_CAL_WAVE", "SPT_GRAT_HI_CAL_WAVE", "SPT_GRAT_LO_POS_WAVE", "SPT_GRAT_HI_POS_WAVE", "SPT_GRAT_REF_WAVE", "SPT_NUM_SLITS", "SPT_SLIT_ENABLED", "SPT_SLIT_LOCATION", "SPT_SLIT_CURPOSITION", "SPT_SLIT_NEWPOSITION", "SPT_SPEED_FOR_EACH_SLIT", "SPT_NUM_SETABLE_SLIT_SPEEDS", "SPT_SLIT_SPEED", "SPT_SLIT_SPEED_MIN", "SPT_SLIT_SPEED_MAX", "SPT_SLIT_STEPSPUNIT", "SPT_SLIT_BACKLASH_REQ", "SPT_SLIT_BACKLASH", "SPT_NUMMIRRORS", "SPT_MIRROR_ENABLED", "SPT_MIRROR_LOCATION", "SPT_MIRROR_CURPOSITION", "SPT_MIRROR_NEWPOSITION", "SPT_OFFSET_AVAIL", "SPT_ADJUST_AVAIL", "SPT_COUNTERSUPPORTED", "SPT_POSITIONSUPPORTED", "SPT_AUTOCALIBSUPPORTED", "SPT_POSITIONMEMORY", "SPT_NUMCOEFFS", "SPT_COEFF", "SPT_SERIAL_IO_SUPPORTED", "SPT_GPIB_IO_SUPPORTED", "SPT_OFFSETADJUSTSUPPORTED", "SPT_LINEARADJUSTSUPPORTED", "SPT_WL_PRECISION", "SPT_NEW_POSITION", "SPT_CUR_POSITION", "SPT_ROI_OFFSET", "SPT_MARK_EXCITATION", "SPT_EXCITATION", "SPT_STEP_SIZE", "SPT_STARTING_WAVELENGTH", "SPT_ENDING_WAVELENGTH", "SPT_MIN_OVERLAP", "SPT_GLUE_BIN_SIZE", "SPT_STARTING_CENTER_WAVE", "SPT_DFLT_BIN_FLAG", "SPT_REPOSITION_FLAG", "SPT_PORT_TYPE", "SPT_PORT_NAME", "SPT_PORT_ADDRESS", "SPT_CUSTOM_NAME", "SPT_GLUE_FILE_NAME", "SPT_DEF_GRATINGSPERTURRET", "SPT_DEF_FOCALLENGTH", "SPT_DEF_INCLUSIONANGLE", "SPT_DEF_DETECTORANGLE", "SPT_DEF_MAGNIFICATION", "SPT_DEF_PIXELWIDTH", "SPT_DEF_REFGRATING", "SPT_DEF_GROOVES", "SPT_DEF_GRAT_USERNAME", "SPT_DEF_GRAT_STEPSPERUNIT", "SPT_DEF_GRAT_SPEED", "SPT_DEF_GRAT_MAX_SPEED", "SPT_DEF_GRAT_MIN_SPEED", "SPT_DEF_GRAT_BACKLASH_REQ", "SPT_DEF_GRAT_BACKLASHSTEPS", "SPT_DEF_SLIT_STEPSPERUNIT", "SPT_DEF_SLIT_SPEED", "SPT_DEF_SLIT_MAX_SPEED", "SPT_DEF_SLIT_MIN_SPEED", "SPT_DEF_SLIT_BACKLASH_REQ", "SPT_DEF_SLIT_BACKLASHSTEPS", "SPT_MIN_SLIT_POS", "SPT_MAX_SLIT_POS", "SPT_SLIT_POS_UNITS", "SPT_DEF_PORTADDRESS", "SPT_DEF_PORTNAME", "SPT_DEF_PORTTYPE", "SPT_SETTINGSLOADED", "SPT_BAUDRATE", "SPT_DATABITS", "SPT_STOPBITS", "SPT_PARITY", "SPT_CTSFLOW", "SPT_MODELNAME", "SPT_SERIALNUMBER", "SPT_VALIDITYFLAG", "SPT_EXISTS", "SPT_CHANGED", "SPT_MANUFACTURE_NAME", "SPT_TRIMTOPRECISION", "SPT_GRAT_TYPE", "SPT_COMM_PORT", "SPT_RESET_WAIT_FLAG", "SPT_DEMOPORT_FLAG", "SPT_INST_NUMTURRETS", "SPT_INST_CURR_TURRET", "SPT_INST_GRAT_GROOVES", "SPT_INST_CUR_GRAT_NUM", "SPT_INST_GRAT_USERNAME", "SPT_INST_CUR_GRAT_POS", "SPT_INST_GRAT_SPEED", "SPT_INST_MODELNAME", "SPT_INST_SERIALNUMBER", "SPT_INST_NUM_SLITS", "SPT_INST_SLIT_LOCATION", "SPT_INST_SLIT_POSITION", "SPT_INST_SLIT_SPEED", "SPT_INST_NUM_MIRRORS", "SPT_INST_MIRROR_LOCATION", "SPT_INST_MIRROR_POSITION", "SPT_ACTIVE_MIRROR_LOC", "SPT_ACTIVE_MIRROR_POS", "SPT_GRAT_MOVE_MODE", "SPT_ACTIVE_GRAT_POS", "SPT_ACTIVE_GRATING_NUM", "SPT_ACTIVE_SLIT_LOC", "SPT_ACTIVE_SLIT_POS", "SPT_STEP_ERROR_CODE", "SPT_ERROR_CODE", "SPT_ACTIVE_TURRET_NUM", "SPT_DLL_INDEX", "SPT_NMTOSTEPS_WL", "SPT_NMTOSTEPS_STEPS", "SPT_NUM_SPECT_DLLS", "SPT_NUM_SPECT_AVAIL", "SPT_MESSAGE_WND_HNDL", "SPT_MUTEX", "SPT_CALC_WL_INCENTERWL", "SPT_CALC_WL_INDIST", "SPT_CALC_WL_OUTWL", "SPT_ARRAY_CENTER", "SPT_CURR_CALIB_PTR", "SPT_DLL_TYPE", "SPT_NEW_SLIT_INDEX", "SPT_NEW_MIRROR_INDEX", "SPT_CALCSLOPEADJ_WL", "SPT_CALCSLOPEADJ_SLOPE", "SPT_MAX_GRATINGS_PER_TURRET", "SPT_MAX_NUM_TURRETS", "SPT_MAX_NUM_MIRRORS", "SPT_MAX_NUM_SLITS", "SPT_GRATING_SPEED_INDEX", "SPT_SLIT_SPEED_INDEX", "SPT_GRATING_SPEED_UNITS", "SPT_GRATING_SPEED_NAME", "SPT_SLIT_SPEED_UNITS", "SPT_SLIT_SPEED_NAME", "SPT_NEED_GRATING_SPEED_SET", "SPT_NEED_SLIT_SPEED_SET", "SPT_GRAT_STEPSUNIT_UNIT", "SPT_SLIT_STEPSUNIT_UNIT", "SPT_PROCESS_MOVE_STATUS", "SPT_RESET", "SPT_RESET_TIMEOUT_MS", "SPT_GENERIC_DLG_MAIN_TITLE", "SPT_GENERIC_DLG_INDEX", "SPT_GENERIC_EDITBOX_TXT", "SPT_GENERIC_EDITBOX", "SPT_GENERIC_SPINBUTTON", "SPT_GENERIC_CHECKBOX_TXT", "SPT_GENERIC_CHECKBOX", "SPT_GENERIC_COMBOBOX_TXT", "SPT_GENERIC_COMBOBOX", "SPT_GENERIC_RADIOBUTTON_GRP", "SPT_GENERIC_RADIOBUTTON_TXT", "SPT_GENERIC_RADIOBUTTON", "SPT_DLL_PRODUCT_VERSION", "SPT_DLL_FILE_VERSION", "SPT_END_OF_LIST"] ("Param")
                n472 = local read "Wavelength Start (nm)"() -> (w819:dbl)
                n473 = local read "writer endpoint"() -> (w814:refnum<k21>)
                n474 = local read "error writer"() -> (w813:errorcluster)
                n475 = local read "MonoRef"() -> (w820:refnum<k7>)
                n476 = invoke class="ISpectroObj" method="SetParam"(reference=w820, "Param"=w817, "pSetVal"=w819) -> (reference out=w818:refnum<k7>)  [unwired: 3 in, 5 out]
                n477 = local read "reader endpoint"() -> (w816:refnum<k21>)
                n478 = local read "error reader"() -> (w815:errorcluster)
                n479 = invoke class="ISpectroObj" method="Move"(reference=w818) -> ()  [unwired: 2 in, 3 out]
              }
              frame #1 {
                n480 = Wait (ms)(milliseconds to wait=u32 1000) -> ()  [unwired: 1 out]
              }
              frame #2 {
                n481 = for {
                  N: w828 -> [_]
                  tunnel: w837 -> [w858] mode=indexing
                  tunnel: w836 -> [w853]
                  tunnel: w835 -> [w852]
                  tunnel: [w851] -> w834
                  tunnel: [w850] -> w833
                  tunnel: [w848] -> w832
                  tunnel: [w847] -> w831
                  tunnel: w830 -> [w846]
                  tunnel: w829 -> [w845]
                  tunnel: w828 -> [w844]
                  i -> [w841]
                  stop <- w839 stop-if-true
                  n482 = flat-sequence {
                    tunnel: w858 -> [w860]
                    tunnel: [w860] -> w856
                    tunnel: [w861] -> w857
                    tunnel: w856 -> [w862]
                    tunnel: [w867] -> w855
                    tunnel: w857 -> [w867]
                    tunnel: [w866] -> w849
                    tunnel: w855 -> [w877]
                    tunnel: [w877] -> w854
                    tunnel: w853 -> [w876]
                    tunnel: w852 -> [w875]
                    tunnel: [w874] -> w851
                    tunnel: [w873] -> w850
                    tunnel: w849 -> [w872]
                    tunnel: [w871] -> w840
                    tunnel: w854 -> [w895]
                    tunnel: [w910] -> w848
                    tunnel: [w909] -> w847
                    tunnel: w846 -> [w908]
                    tunnel: w845 -> [w905]
                    tunnel: w843 -> [w901]
                    tunnel: w838 -> [w903]
                    frame #0 {
                      n483 = Tick Count (ms)() -> (millisecond timer value=w859:u32)
                      n484 = local write "time start (ms)"(w859) -> ()
                    }
                    frame #1 {
                      w865 = 87 items=["SPT_NOCMD", "SPT_SPECTS_SUPPORTED", "SPT_TYPE", "SPT_CALIBUPDATE", "SPT_GRATINGWARNING", "SPT_LASERWARNING", "SPT_FORCEMOVE", "SPT_INSTNAME", "SPT_USERNAME", "SPT_INSTUSERNAME", "SPT_INSTCOMMNAME", "SPT_WAVE_ORIENTED", "SPT_NUMSTAGES", "SPT_GRATINGSPERTURRET", "SPT_CURRGRATING", "SPT_GRAT_BACKLASH_REQ", "SPT_GRATINGBACKLASHSTEPS", "SPT_NEEDINIT", "SPT_NEED_HWINIT", "SPT_MOTOR", "SPT_ARRAYSIZE", "SPT_ROI_CENTER", "SPT_ORDER", "SPT_CUR_GRATING", "SPT_NEW_GRATING", "SPT_SEQUENCER_STATE", "SPT_NUMTURRETS", "SPT_CURRTURRET", "SPT_DO_RESET", "SPT_SLAVE_CNT", "SPT_NUM_STEPS", "SPT_PIXEL_WIDTH", "SPT_GRAT_USERNAME", "SPT_GRAT_GROOVES", "SPT_GRAT_CENTERADJ", "SPT_GRAT_LINEAR_ADJ", "SPT_GRAT_SLOPE_ADJ", "SPT_GRAT_FOCAL_LEN", "SPT_GRAT_INCL_ANGLE", "SPT_GRAT_DETECT_ANGLE", "SPT_GRAT_MAG", "SPT_ACCESS_ALL_GRAT_SPEEDS", "SPT_SPEED_FOR_EACH_GRATING", "SPT_NUM_SETABLE_GRAT_SPEEDS", "SPT_GRATING_SPEED", "SPT_GRATING_SPEED_MIN", "SPT_GRATING_SPEED_MAX", "SPT_GRAT_REF_GRATING", "SPT_GRAT_STEPSPUNIT", "SPT_GRAT_OFFSET", "SPT_GRAT_ADJUST", "SPT_GRAT_LO_CAL_WAVE", "SPT_GRAT_HI_CAL_WAVE", "SPT_GRAT_LO_POS_WAVE", "SPT_GRAT_HI_POS_WAVE", "SPT_GRAT_REF_WAVE", "SPT_NUM_SLITS", "SPT_SLIT_ENABLED", "SPT_SLIT_LOCATION", "SPT_SLIT_CURPOSITION", "SPT_SLIT_NEWPOSITION", "SPT_SPEED_FOR_EACH_SLIT", "SPT_NUM_SETABLE_SLIT_SPEEDS", "SPT_SLIT_SPEED", "SPT_SLIT_SPEED_MIN", "SPT_SLIT_SPEED_MAX", "SPT_SLIT_STEPSPUNIT", "SPT_SLIT_BACKLASH_REQ", "SPT_SLIT_BACKLASH", "SPT_NUMMIRRORS", "SPT_MIRROR_ENABLED", "SPT_MIRROR_LOCATION", "SPT_MIRROR_CURPOSITION", "SPT_MIRROR_NEWPOSITION", "SPT_OFFSET_AVAIL", "SPT_ADJUST_AVAIL", "SPT_COUNTERSUPPORTED", "SPT_POSITIONSUPPORTED", "SPT_AUTOCALIBSUPPORTED", "SPT_POSITIONMEMORY", "SPT_NUMCOEFFS", "SPT_COEFF", "SPT_SERIAL_IO_SUPPORTED", "SPT_GPIB_IO_SUPPORTED", "SPT_OFFSETADJUSTSUPPORTED", "SPT_LINEARADJUSTSUPPORTED", "SPT_WL_PRECISION", "SPT_NEW_POSITION", "SPT_CUR_POSITION", "SPT_ROI_OFFSET", "SPT_MARK_EXCITATION", "SPT_EXCITATION", "SPT_STEP_SIZE", "SPT_STARTING_WAVELENGTH", "SPT_ENDING_WAVELENGTH", "SPT_MIN_OVERLAP", "SPT_GLUE_BIN_SIZE", "SPT_STARTING_CENTER_WAVE", "SPT_DFLT_BIN_FLAG", "SPT_REPOSITION_FLAG", "SPT_PORT_TYPE", "SPT_PORT_NAME", "SPT_PORT_ADDRESS", "SPT_CUSTOM_NAME", "SPT_GLUE_FILE_NAME", "SPT_DEF_GRATINGSPERTURRET", "SPT_DEF_FOCALLENGTH", "SPT_DEF_INCLUSIONANGLE", "SPT_DEF_DETECTORANGLE", "SPT_DEF_MAGNIFICATION", "SPT_DEF_PIXELWIDTH", "SPT_DEF_REFGRATING", "SPT_DEF_GROOVES", "SPT_DEF_GRAT_USERNAME", "SPT_DEF_GRAT_STEPSPERUNIT", "SPT_DEF_GRAT_SPEED", "SPT_DEF_GRAT_MAX_SPEED", "SPT_DEF_GRAT_MIN_SPEED", "SPT_DEF_GRAT_BACKLASH_REQ", "SPT_DEF_GRAT_BACKLASHSTEPS", "SPT_DEF_SLIT_STEPSPERUNIT", "SPT_DEF_SLIT_SPEED", "SPT_DEF_SLIT_MAX_SPEED", "SPT_DEF_SLIT_MIN_SPEED", "SPT_DEF_SLIT_BACKLASH_REQ", "SPT_DEF_SLIT_BACKLASHSTEPS", "SPT_MIN_SLIT_POS", "SPT_MAX_SLIT_POS", "SPT_SLIT_POS_UNITS", "SPT_DEF_PORTADDRESS", "SPT_DEF_PORTNAME", "SPT_DEF_PORTTYPE", "SPT_SETTINGSLOADED", "SPT_BAUDRATE", "SPT_DATABITS", "SPT_STOPBITS", "SPT_PARITY", "SPT_CTSFLOW", "SPT_MODELNAME", "SPT_SERIALNUMBER", "SPT_VALIDITYFLAG", "SPT_EXISTS", "SPT_CHANGED", "SPT_MANUFACTURE_NAME", "SPT_TRIMTOPRECISION", "SPT_GRAT_TYPE", "SPT_COMM_PORT", "SPT_RESET_WAIT_FLAG", "SPT_DEMOPORT_FLAG", "SPT_INST_NUMTURRETS", "SPT_INST_CURR_TURRET", "SPT_INST_GRAT_GROOVES", "SPT_INST_CUR_GRAT_NUM", "SPT_INST_GRAT_USERNAME", "SPT_INST_CUR_GRAT_POS", "SPT_INST_GRAT_SPEED", "SPT_INST_MODELNAME", "SPT_INST_SERIALNUMBER", "SPT_INST_NUM_SLITS", "SPT_INST_SLIT_LOCATION", "SPT_INST_SLIT_POSITION", "SPT_INST_SLIT_SPEED", "SPT_INST_NUM_MIRRORS", "SPT_INST_MIRROR_LOCATION", "SPT_INST_MIRROR_POSITION", "SPT_ACTIVE_MIRROR_LOC", "SPT_ACTIVE_MIRROR_POS", "SPT_GRAT_MOVE_MODE", "SPT_ACTIVE_GRAT_POS", "SPT_ACTIVE_GRATING_NUM", "SPT_ACTIVE_SLIT_LOC", "SPT_ACTIVE_SLIT_POS", "SPT_STEP_ERROR_CODE", "SPT_ERROR_CODE", "SPT_ACTIVE_TURRET_NUM", "SPT_DLL_INDEX", "SPT_NMTOSTEPS_WL", "SPT_NMTOSTEPS_STEPS", "SPT_NUM_SPECT_DLLS", "SPT_NUM_SPECT_AVAIL", "SPT_MESSAGE_WND_HNDL", "SPT_MUTEX", "SPT_CALC_WL_INCENTERWL", "SPT_CALC_WL_INDIST", "SPT_CALC_WL_OUTWL", "SPT_ARRAY_CENTER", "SPT_CURR_CALIB_PTR", "SPT_DLL_TYPE", "SPT_NEW_SLIT_INDEX", "SPT_NEW_MIRROR_INDEX", "SPT_CALCSLOPEADJ_WL", "SPT_CALCSLOPEADJ_SLOPE", "SPT_MAX_GRATINGS_PER_TURRET", "SPT_MAX_NUM_TURRETS", "SPT_MAX_NUM_MIRRORS", "SPT_MAX_NUM_SLITS", "SPT_GRATING_SPEED_INDEX", "SPT_SLIT_SPEED_INDEX", "SPT_GRATING_SPEED_UNITS", "SPT_GRATING_SPEED_NAME", "SPT_SLIT_SPEED_UNITS", "SPT_SLIT_SPEED_NAME", "SPT_NEED_GRATING_SPEED_SET", "SPT_NEED_SLIT_SPEED_SET", "SPT_GRAT_STEPSUNIT_UNIT", "SPT_SLIT_STEPSUNIT_UNIT", "SPT_PROCESS_MOVE_STATUS", "SPT_RESET", "SPT_RESET_TIMEOUT_MS", "SPT_GENERIC_DLG_MAIN_TITLE", "SPT_GENERIC_DLG_INDEX", "SPT_GENERIC_EDITBOX_TXT", "SPT_GENERIC_EDITBOX", "SPT_GENERIC_SPINBUTTON", "SPT_GENERIC_CHECKBOX_TXT", "SPT_GENERIC_CHECKBOX", "SPT_GENERIC_COMBOBOX_TXT", "SPT_GENERIC_COMBOBOX", "SPT_GENERIC_RADIOBUTTON_GRP", "SPT_GENERIC_RADIOBUTTON_TXT", "SPT_GENERIC_RADIOBUTTON", "SPT_DLL_PRODUCT_VERSION", "SPT_DLL_FILE_VERSION", "SPT_END_OF_LIST"] ("Param")
                      n485 = local read "MonoRef"() -> (w863:refnum<k7>)
                      n486 = invoke class="ISpectroObj" method="SetParam"(reference=w863, "Param"=w865, "pSetVal"=w862) -> (reference out=w864:refnum<k7>)  [unwired: 3 in, 5 out]
                      n487 = invoke class="ISpectroObj" method="Move"(reference=w864) -> (reference out=w861:refnum<k7>)  [unwired: 2 in, 2 out]
                    }
                    frame #2 {
                      n488 = local read "OMA V exposure time"() -> (w869:dbl)
                      n489 = local read "Hosts Synchronized"() -> (w866:bool)
                      n490 = Multiply(x=w869, y=1.0) -> (x*y=w868:dbl)
                      n491 = Wait (ms)(milliseconds to wait=w868) -> ()  [unwired: 1 out]
                    }
                    frame #3 {
                      n492 = case shown="True" w872 {
                        tunnel: w876 -> [w879 w885]
                        tunnel: w875 -> [w880 w884]
                        tunnel: [w880 w883] -> w874
                        tunnel: [w879 w882] -> w873
                        tunnel: [FALSE w881] -> w871
                        frame False {
                        }
                        frame True {
                          n493 = while {
                            shift-right: [w891] -> w882
                            shift-left: w885 -> [w893]
                            shift-right: [w890] -> w883
                            shift-left: w884 -> [w892]
                            tunnel: [w886] -> w881
                            stop <- w887 continue-if-true
                            n494 = local read "standby stream"() -> (w888:bool)
                            n495 = shared-variable-read(w893, w892, 1000 ("timeout ms (-1)")) -> (w891:refnum<k21>, w890:errorcluster, w889:bool, w886:bool)
                            n496 = And(x=w889, y=w888) -> (x .and. y?=w887:bool)
                          }
                        }
                      }
                    }
                    frame #4 {
                      w896 = 88 items=["SPT_NOCMD", "SPT_SPECTS_SUPPORTED", "SPT_TYPE", "SPT_CALIBUPDATE", "SPT_GRATINGWARNING", "SPT_LASERWARNING", "SPT_FORCEMOVE", "SPT_INSTNAME", "SPT_USERNAME", "SPT_INSTUSERNAME", "SPT_INSTCOMMNAME", "SPT_WAVE_ORIENTED", "SPT_NUMSTAGES", "SPT_GRATINGSPERTURRET", "SPT_CURRGRATING", "SPT_GRAT_BACKLASH_REQ", "SPT_GRATINGBACKLASHSTEPS", "SPT_NEEDINIT", "SPT_NEED_HWINIT", "SPT_MOTOR", "SPT_ARRAYSIZE", "SPT_ROI_CENTER", "SPT_ORDER", "SPT_CUR_GRATING", "SPT_NEW_GRATING", "SPT_SEQUENCER_STATE", "SPT_NUMTURRETS", "SPT_CURRTURRET", "SPT_DO_RESET", "SPT_SLAVE_CNT", "SPT_NUM_STEPS", "SPT_PIXEL_WIDTH", "SPT_GRAT_USERNAME", "SPT_GRAT_GROOVES", "SPT_GRAT_CENTERADJ", "SPT_GRAT_LINEAR_ADJ", "SPT_GRAT_SLOPE_ADJ", "SPT_GRAT_FOCAL_LEN", "SPT_GRAT_INCL_ANGLE", "SPT_GRAT_DETECT_ANGLE", "SPT_GRAT_MAG", "SPT_ACCESS_ALL_GRAT_SPEEDS", "SPT_SPEED_FOR_EACH_GRATING", "SPT_NUM_SETABLE_GRAT_SPEEDS", "SPT_GRATING_SPEED", "SPT_GRATING_SPEED_MIN", "SPT_GRATING_SPEED_MAX", "SPT_GRAT_REF_GRATING", "SPT_GRAT_STEPSPUNIT", "SPT_GRAT_OFFSET", "SPT_GRAT_ADJUST", "SPT_GRAT_LO_CAL_WAVE", "SPT_GRAT_HI_CAL_WAVE", "SPT_GRAT_LO_POS_WAVE", "SPT_GRAT_HI_POS_WAVE", "SPT_GRAT_REF_WAVE", "SPT_NUM_SLITS", "SPT_SLIT_ENABLED", "SPT_SLIT_LOCATION", "SPT_SLIT_CURPOSITION", "SPT_SLIT_NEWPOSITION", "SPT_SPEED_FOR_EACH_SLIT", "SPT_NUM_SETABLE_SLIT_SPEEDS", "SPT_SLIT_SPEED", "SPT_SLIT_SPEED_MIN", "SPT_SLIT_SPEED_MAX", "SPT_SLIT_STEPSPUNIT", "SPT_SLIT_BACKLASH_REQ", "SPT_SLIT_BACKLASH", "SPT_NUMMIRRORS", "SPT_MIRROR_ENABLED", "SPT_MIRROR_LOCATION", "SPT_MIRROR_CURPOSITION", "SPT_MIRROR_NEWPOSITION", "SPT_OFFSET_AVAIL", "SPT_ADJUST_AVAIL", "SPT_COUNTERSUPPORTED", "SPT_POSITIONSUPPORTED", "SPT_AUTOCALIBSUPPORTED", "SPT_POSITIONMEMORY", "SPT_NUMCOEFFS", "SPT_COEFF", "SPT_SERIAL_IO_SUPPORTED", "SPT_GPIB_IO_SUPPORTED", "SPT_OFFSETADJUSTSUPPORTED", "SPT_LINEARADJUSTSUPPORTED", "SPT_WL_PRECISION", "SPT_NEW_POSITION", "SPT_CUR_POSITION", "SPT_ROI_OFFSET", "SPT_MARK_EXCITATION", "SPT_EXCITATION", "SPT_STEP_SIZE", "SPT_STARTING_WAVELENGTH", "SPT_ENDING_WAVELENGTH", "SPT_MIN_OVERLAP", "SPT_GLUE_BIN_SIZE", "SPT_STARTING_CENTER_WAVE", "SPT_DFLT_BIN_FLAG", "SPT_REPOSITION_FLAG", "SPT_PORT_TYPE", "SPT_PORT_NAME", "SPT_PORT_ADDRESS", "SPT_CUSTOM_NAME", "SPT_GLUE_FILE_NAME", "SPT_DEF_GRATINGSPERTURRET", "SPT_DEF_FOCALLENGTH", "SPT_DEF_INCLUSIONANGLE", "SPT_DEF_DETECTORANGLE", "SPT_DEF_MAGNIFICATION", "SPT_DEF_PIXELWIDTH", "SPT_DEF_REFGRATING", "SPT_DEF_GROOVES", "SPT_DEF_GRAT_USERNAME", "SPT_DEF_GRAT_STEPSPERUNIT", "SPT_DEF_GRAT_SPEED", "SPT_DEF_GRAT_MAX_SPEED", "SPT_DEF_GRAT_MIN_SPEED", "SPT_DEF_GRAT_BACKLASH_REQ", "SPT_DEF_GRAT_BACKLASHSTEPS", "SPT_DEF_SLIT_STEPSPERUNIT", "SPT_DEF_SLIT_SPEED", "SPT_DEF_SLIT_MAX_SPEED", "SPT_DEF_SLIT_MIN_SPEED", "SPT_DEF_SLIT_BACKLASH_REQ", "SPT_DEF_SLIT_BACKLASHSTEPS", "SPT_MIN_SLIT_POS", "SPT_MAX_SLIT_POS", "SPT_SLIT_POS_UNITS", "SPT_DEF_PORTADDRESS", "SPT_DEF_PORTNAME", "SPT_DEF_PORTTYPE", "SPT_SETTINGSLOADED", "SPT_BAUDRATE", "SPT_DATABITS", "SPT_STOPBITS", "SPT_PARITY", "SPT_CTSFLOW", "SPT_MODELNAME", "SPT_SERIALNUMBER", "SPT_VALIDITYFLAG", "SPT_EXISTS", "SPT_CHANGED", "SPT_MANUFACTURE_NAME", "SPT_TRIMTOPRECISION", "SPT_GRAT_TYPE", "SPT_COMM_PORT", "SPT_RESET_WAIT_FLAG", "SPT_DEMOPORT_FLAG", "SPT_INST_NUMTURRETS", "SPT_INST_CURR_TURRET", "SPT_INST_GRAT_GROOVES", "SPT_INST_CUR_GRAT_NUM", "SPT_INST_GRAT_USERNAME", "SPT_INST_CUR_GRAT_POS", "SPT_INST_GRAT_SPEED", "SPT_INST_MODELNAME", "SPT_INST_SERIALNUMBER", "SPT_INST_NUM_SLITS", "SPT_INST_SLIT_LOCATION", "SPT_INST_SLIT_POSITION", "SPT_INST_SLIT_SPEED", "SPT_INST_NUM_MIRRORS", "SPT_INST_MIRROR_LOCATION", "SPT_INST_MIRROR_POSITION", "SPT_ACTIVE_MIRROR_LOC", "SPT_ACTIVE_MIRROR_POS", "SPT_GRAT_MOVE_MODE", "SPT_ACTIVE_GRAT_POS", "SPT_ACTIVE_GRATING_NUM", "SPT_ACTIVE_SLIT_LOC", "SPT_ACTIVE_SLIT_POS", "SPT_STEP_ERROR_CODE", "SPT_ERROR_CODE", "SPT_ACTIVE_TURRET_NUM", "SPT_DLL_INDEX", "SPT_NMTOSTEPS_WL", "SPT_NMTOSTEPS_STEPS", "SPT_NUM_SPECT_DLLS", "SPT_NUM_SPECT_AVAIL", "SPT_MESSAGE_WND_HNDL", "SPT_MUTEX", "SPT_CALC_WL_INCENTERWL", "SPT_CALC_WL_INDIST", "SPT_CALC_WL_OUTWL", "SPT_ARRAY_CENTER", "SPT_CURR_CALIB_PTR", "SPT_DLL_TYPE", "SPT_NEW_SLIT_INDEX", "SPT_NEW_MIRROR_INDEX", "SPT_CALCSLOPEADJ_WL", "SPT_CALCSLOPEADJ_SLOPE", "SPT_MAX_GRATINGS_PER_TURRET", "SPT_MAX_NUM_TURRETS", "SPT_MAX_NUM_MIRRORS", "SPT_MAX_NUM_SLITS", "SPT_GRATING_SPEED_INDEX", "SPT_SLIT_SPEED_INDEX", "SPT_GRATING_SPEED_UNITS", "SPT_GRATING_SPEED_NAME", "SPT_SLIT_SPEED_UNITS", "SPT_SLIT_SPEED_NAME", "SPT_NEED_GRATING_SPEED_SET", "SPT_NEED_SLIT_SPEED_SET", "SPT_GRAT_STEPSUNIT_UNIT", "SPT_SLIT_STEPSUNIT_UNIT", "SPT_PROCESS_MOVE_STATUS", "SPT_RESET", "SPT_RESET_TIMEOUT_MS", "SPT_GENERIC_DLG_MAIN_TITLE", "SPT_GENERIC_DLG_INDEX", "SPT_GENERIC_EDITBOX_TXT", "SPT_GENERIC_EDITBOX", "SPT_GENERIC_SPINBUTTON", "SPT_GENERIC_CHECKBOX_TXT", "SPT_GENERIC_CHECKBOX", "SPT_GENERIC_COMBOBOX_TXT", "SPT_GENERIC_COMBOBOX", "SPT_GENERIC_RADIOBUTTON_GRP", "SPT_GENERIC_RADIOBUTTON_TXT", "SPT_GENERIC_RADIOBUTTON", "SPT_DLL_PRODUCT_VERSION", "SPT_DLL_FILE_VERSION", "SPT_END_OF_LIST"] ("Param")
                      n497 = invoke class="ISpectroObj" method="GetParam"(reference=w895, "Param"=w896) -> ("GetParam"=w899:variant)  [unwired: 4 in, 5 out]
                      n498 = Variant To Data(type=0.0, Variant=w899) -> (data=w898:dbl)  [unwired: 1 in, 1 out]
                      n499 = local write "Wavelength (nm)"(w898) -> ()
                    }
                    frame #5 {
                      # "send data"
                      n500 = Not(x=w903) -> (.not. x?=w902:bool)
                      n501 = And(x=w901, y=w902) -> (x .and. y?=w900:bool)
                      n502 = case shown="False" w900 {
                        tunnel: [cluster{dbl[], dbl[]} {[], []} ("data in") cluster{dbl[], dbl[]} {[1.0], [1.0]} ("data in")] -> w904
                        frame False {
                        }
                        frame True {
                        }
                      }
                      n503 = shared-variable-write(w908, w905, w904) -> (w907:refnum<k21>, w906:errorcluster)  [unwired: 1 in, 1 out]
                      n504 = Flush Stream(8:w906, 11:w907) -> (0:w910:errorcluster, 3:w909:refnum<k21>)  [unwired: 2 in, 1 out]
                    }
                    frame #6 {
                      n505 = local read "time start (ms)"() -> (w915:i32)
                      n506 = Tick Count (ms)() -> (millisecond timer value=w914:u32)
                      n507 = Subtract(x=w914, y=w915) -> (x-y=w916:u32)
                      n508 = Divide(x=w916, y=u32 1000) -> (x/y=w917:dbl)
                      n509 = local write "time elapsed (s)"(w917) -> ()
                    }
                  }
                  n510 = Increment(x=w841) -> (x+1=w842:i32)
                  n511 = Greater?(x=w844, y=w842) -> (0:w843:bool)
                  n512 = local read "Stop measurement"() -> (w838:bool)
                  n513 = Or(x=w838, y=w840) -> (x .or. y?=w839:bool)
                }
              }
              frame #3 {
                w922 = FALSE ("Stop measurement")
                n514 = local write "Stop measurement"(w922) -> ()
                n515 = local write "error reader"(w921) -> ()
                n516 = local write "reader endpoint"(w920) -> ()
                n517 = local write "Start Scan"(w922) -> ()
                n518 = local write "busy"(FALSE ("busy")) -> ()
                n519 = local write "writer endpoint"(w918) -> ()
                n520 = local write "error writer"(w919) -> ()
              }
            }
          }
        }
      }
      frame #2 {
        # "Fast post-updating"
      }
    }
  }
  n521 = Initialize Array(0, 1 ("dimension size"), 1 ("dimension size")) -> (→"frame array":i32[][])
  n522 = local write "standby stream"(FALSE ("standby stream")) -> ()
  n523 = local write "Spectro Correct background"(w7) -> ()
  n524 = property on="Intensity Sum" class="DigNum (strict)"("NumText.FontSize"=u32 40 ("Numeric Text.Size:Height")) -> ()  [unwired: 2 in, 2 out]
  n525 = local write "Set Temperature (°C)"(i8 -110 ("Set Temperature (°C)")) -> ()
  n526 = local write "OMA V gain"(w8) -> ()
  n527 = property on="Spectro Correct background" class="Bool (strict)"("DisabledEnum"=T2."Disabled" ("Disabled")) -> ()  [unwired: 2 in, 2 out]
  "Spectro ON" <- FALSE ("Spectro ON")
  "busy" <- FALSE ("busy")
  "Hosts Synchronized" <- w7
